vi "main4ChProspectiveStudyBK09172025.vi"() -> ()   [LabVIEW 2024]
doc: "Main VI for FLS imaging system."
uses:
  SubVI/DigitizerConfiguration/FLImDAQ.ctl
  <instrlib>/niScope/Controls/niScope trigger source.ctl
  SubVI/LabJack/LJ Pin Setting.ctl
  ConfigFiles/AimingBeamVideoConfig.ctl
  LaguerreDeconLib/DeconEngineClass/LaguerreDeconEngineClass.lvclass/LaguerreDeconEngineClass.ctl
  <vilib>/Utility/error.llb/DialogType.ctl
  LaguerreDeconLib/DeconEngineClass/LaguerreDeconEngineClass.lvclass
  <vilib>/event_ctls.llb/usereventprio.ctl
  <vilib>/Utility/miscctls.llb/LVMinMaxIncTypeDef.ctl
  SubVI/APD/APDClass.lvclass
  <vilib>/Analysis/baseanly.llb/Mean (DBL).vi
  SubVI/GlobalVariables.vi
  <vilib>/addons/control/pid/pid.llb/PID (DBL).vi
  <instrlib>/niScope/Acquire/Fetch/niScope Multi Fetch Binary 16.vi
  <vilib>/Instr/_visa.llb/VISA Configure Serial Port (Instr).vi
  <vilib>/Python/Open Anaconda Python Session.vi
  C:/Users/MarcuLab/Documents/GitHub/NetDeconForLV/Source/DotNETAssembly/output/build/LaguerreDeConNative.dll
  Documents/GitHub/NetDeconForLV/Source/DotNETAssembly/output/build/LaguerreDeConNative.dll
  <userlib>/_OpenG.lib/file/file.llb/openg_file.lvlib
  <userlib>/_OpenG.lib/time/time.llb/openg_time.lvlib
  <vilib>/Analysis/NI_AALBase.lvlib
  <vilib>/Utility/miscctls.llb/LVPointTypeDef.ctl
  <vilib>/addons/control/pid/NI_PID_pid.lvlib
panel:
  in  "CancerThreshold":dbl=0.15
  out "Decon Loop timing (ms)":dbl
  out "Ch3 Lifetime (ns)":dbl caption="Lifetime (ns)"
  out "Ch2 Lifetime (ns)":dbl caption="Lifetime (ns)"
  out "Ch1 Lifetime (ns)":dbl caption="Lifetime (ns)"
  out "Cancer Prob":dbl
  in  "Overlay selection":u16(ring)=2 items=["Gain", "Lifetime", "CancerProbability"]
  out "Record Backlog 2":i32
  in  "Auto gain ch4":bool=TRUE caption="Auto gain ch3"
  in  "V 4":dbl caption="Gain 3" min=0.0 max=4.67 step=0.1
  out "Gain4":dbl
  out "IntR4":dbl format="%#_2g"
  out "SNR4":dbl format="%#_3g"
  out "Channel 4":dbl[][](graph) caption="Channel 3"
  out "RunStartTime":u32
  out "Dig1 Temp":dbl
  out "Dig2 Temp":dbl
  out "Visualization PC video source":T1
  in  "V target(1.0)":dbl=1.0 caption="V target(1.5)" min=0.3 max=1.5 step=0.1 format="%#_4g"
  out "SNR3":dbl format="%#_3g"
  out "SNR2":dbl format="%#_3g"
  out "SNR1":dbl format="%#_3g"
  in  "Show BG removed?":bool=TRUE
  out "IntR3":dbl format="%#_2g"
  out "IntR2":dbl format="%#_2g"
  out "IntR1":dbl format="%#_2g"
  in  "Video Display":bool
  out "Gain3":dbl
  out "Gain2":dbl
  out "Gain1":dbl
  in  "Skip Data Save?":bool
  out "Aq Loop?":bool
  out "ML?":bool
  out "aquisition loop Error Out":errorcluster
  out "Laser f (Hz)":dbl
  out "Record Backlog":i32
  out "Fetch Record #":i32
  out "Sync Success?":bool
  out "Disclamer":picture
  out "Calibration #":i8
  out "BG #":i8
  in  "TCP Connect":bool
  out "Help":string
  in  "355nm Laser toggle":bool caption="355nm 460Hz"
  in  "Cali&iRF alignment":bool
  in  "Background":bool
  in  "Aiming beam toggle":bool caption="445nm 0Hz 30mA"
  in  "Auto gain ch3":bool=TRUE
  in  "Auto gain ch2":bool=TRUE
  in  "Auto gain ch1":bool=TRUE
  out "Run #":i8
  in  "StopButton":bool caption="Stop"
  out "Aquisition Status:":bool
  in  "StartButton":bool caption="Start"
  in  "V 3":dbl caption="Gain 3" min=0.0 max=4.65 step=0.1
  in  "V 2":dbl caption="Gain 2" min=0.0 max=4.59 step=0.1
  in  "V 1":dbl caption="Gain 1" min=0.0 max=4.63 step=0.1 format="%#_4g"
  in  "Video Source":enum32{"Camera", "FrameGrabber"}(radio)
  out "Case #":string
  out "System Hardware Connection Status":T2
  out "Channel 3":dbl[][](graph)
  out "Channel 2":dbl[][](graph)
  out "Channel 1":dbl[][](graph)
  in  "Tab Control":T3(tab)
  out "display loop timing(ms)":u32
  out "Aquisition loop timing(ms)":u32 format="%.2f"
  out "DisplayLoop":i32
  out "PID loop":i32 caption="processing loop"
  out "PID loop timing(ms)":u32 caption="processing loop timing(ms)"
  out "Communication loop(ms)":u32
  out "laser EM lamp V":dbl format="%0.6f"
  out "Auisition Loop idx":i32
  out "LJ process (ms)":u32
  out "LJ time(ms)":u32[](array[numeric])
  out "output variable":i32
  out "BG Graph":dbl[][](graph)
  out "Lifetime (ns)":cluster{dbl, dbl, dbl}(graph)
  out "DeCon Speed(ms)":dbl(graph)
  out "iRF Graph":dbl[][](graph)
  in  "Show BG":bool
  out "iRF length":i32
  out "BG length":i32
  out "data length":i32
  out "WarmupTime(ms)":u32
  out "BGAll":dbl[][](array[numeric])
  out "DeConOut":dbl[](array[numeric])
  in  "Ch1GainLim":dbl=350.0 format="%#_13g"
  in  "Ch2&3GainLim":dbl=1750.0 format="%#_13g"
  out "LJ Pinout":T4={"Ch1 Bias"="DAC0", "Ch2 Bias"="DAC1", "Ch3 Bias"="DAC2", "Ch4 Bias"="DAC0", "355 PWM"="FIO0", "AimingBeam PWM"="FIO2", "Laser Ready"="FIO3", "Interlock"="FIO1", "Laser Start/Stop"="FIO1", "Red LED"="FIO1", "Green LED"="DIO3", "Foot Pedal"="DIO15"}
  out "FLImDAQ":T5={"Digitizer 1"="", "Digitizer 2"="", "Channel"=enum."Channel 0", "trigger source"="VAL_EXTERNAL", "trigger level"=0.5, "trigger delay"=1.35e-07, "min sample rate"=12500000000.0, "min record length"=2500, "vertical range"=1.0, "vertical offset"=-0.25, "Waveform to Avg"=2000} caption="FLIm DAQ Configuration" {"trigger delay" format="%^#.4e"; "trigger level" min=0.0 max=3.5 step=0.5 format="%.2f"; "vertical offset" format="%.4f"; "vertical range" format="%.2f"; "min sample rate" format="%#.2p"}
  in  "Sys Reconfig":bool
  out "data out(communcation loop)":string
  out "PID loop error out":errorcluster caption="processing Error Out"
  out "decon error out":errorcluster
  out "Laser Rep Rate":dbl
  out "V4 Size":i32 caption="V3 Size"
  in  "Data Class":enum16{"Data", "BG", "Cali"}(ring)=enum."BG"
  out "V1 Size":i32
  out "V2 Size":i32
  out "V3 Size":i32
  out "data Size":i32[](array[numeric])
  out "State log":string
  out "SysConfigCluster":T7
  in  "Ch4 PID gains":T8={"proportional gain (Kc)"=30.0, "integral time (Ti, min)"=0.0003, "derivative time (Td, min)"=1e-05}
  in  "Ch3 PID gains":T8={"proportional gain (Kc)"=30.0, "integral time (Ti, min)"=0.0003, "derivative time (Td, min)"=1e-05}
  in  "Ch2 PID gains":T8={"proportional gain (Kc)"=30.0, "integral time (Ti, min)"=0.0003, "derivative time (Td, min)"=1e-05}
  in  "Ch1 PID gains":T8={"proportional gain (Kc)"=30.0, "integral time (Ti, min)"=0.0003, "derivative time (Td, min)"=1e-05}
  in  "module path":path=path "C:/Users/MarcuLab/Documents/GitHub/NetDeconForLV/Classifier/HNClassifier.py"
  in  "model path":path=path "C:/Users/MarcuLab/Documents/GitHub/NetDeconForLV/Classifier/20241127_dc/200.pkl"
  in  "Env name":string="HNClassifier"
  in  "Python version":string="3.10"
  out "Python session":refnum<k35>
  in  "Quit":bool
  in  "Radio Buttons":T9(radio)=enum."Ch2" caption="DeCon Chan"
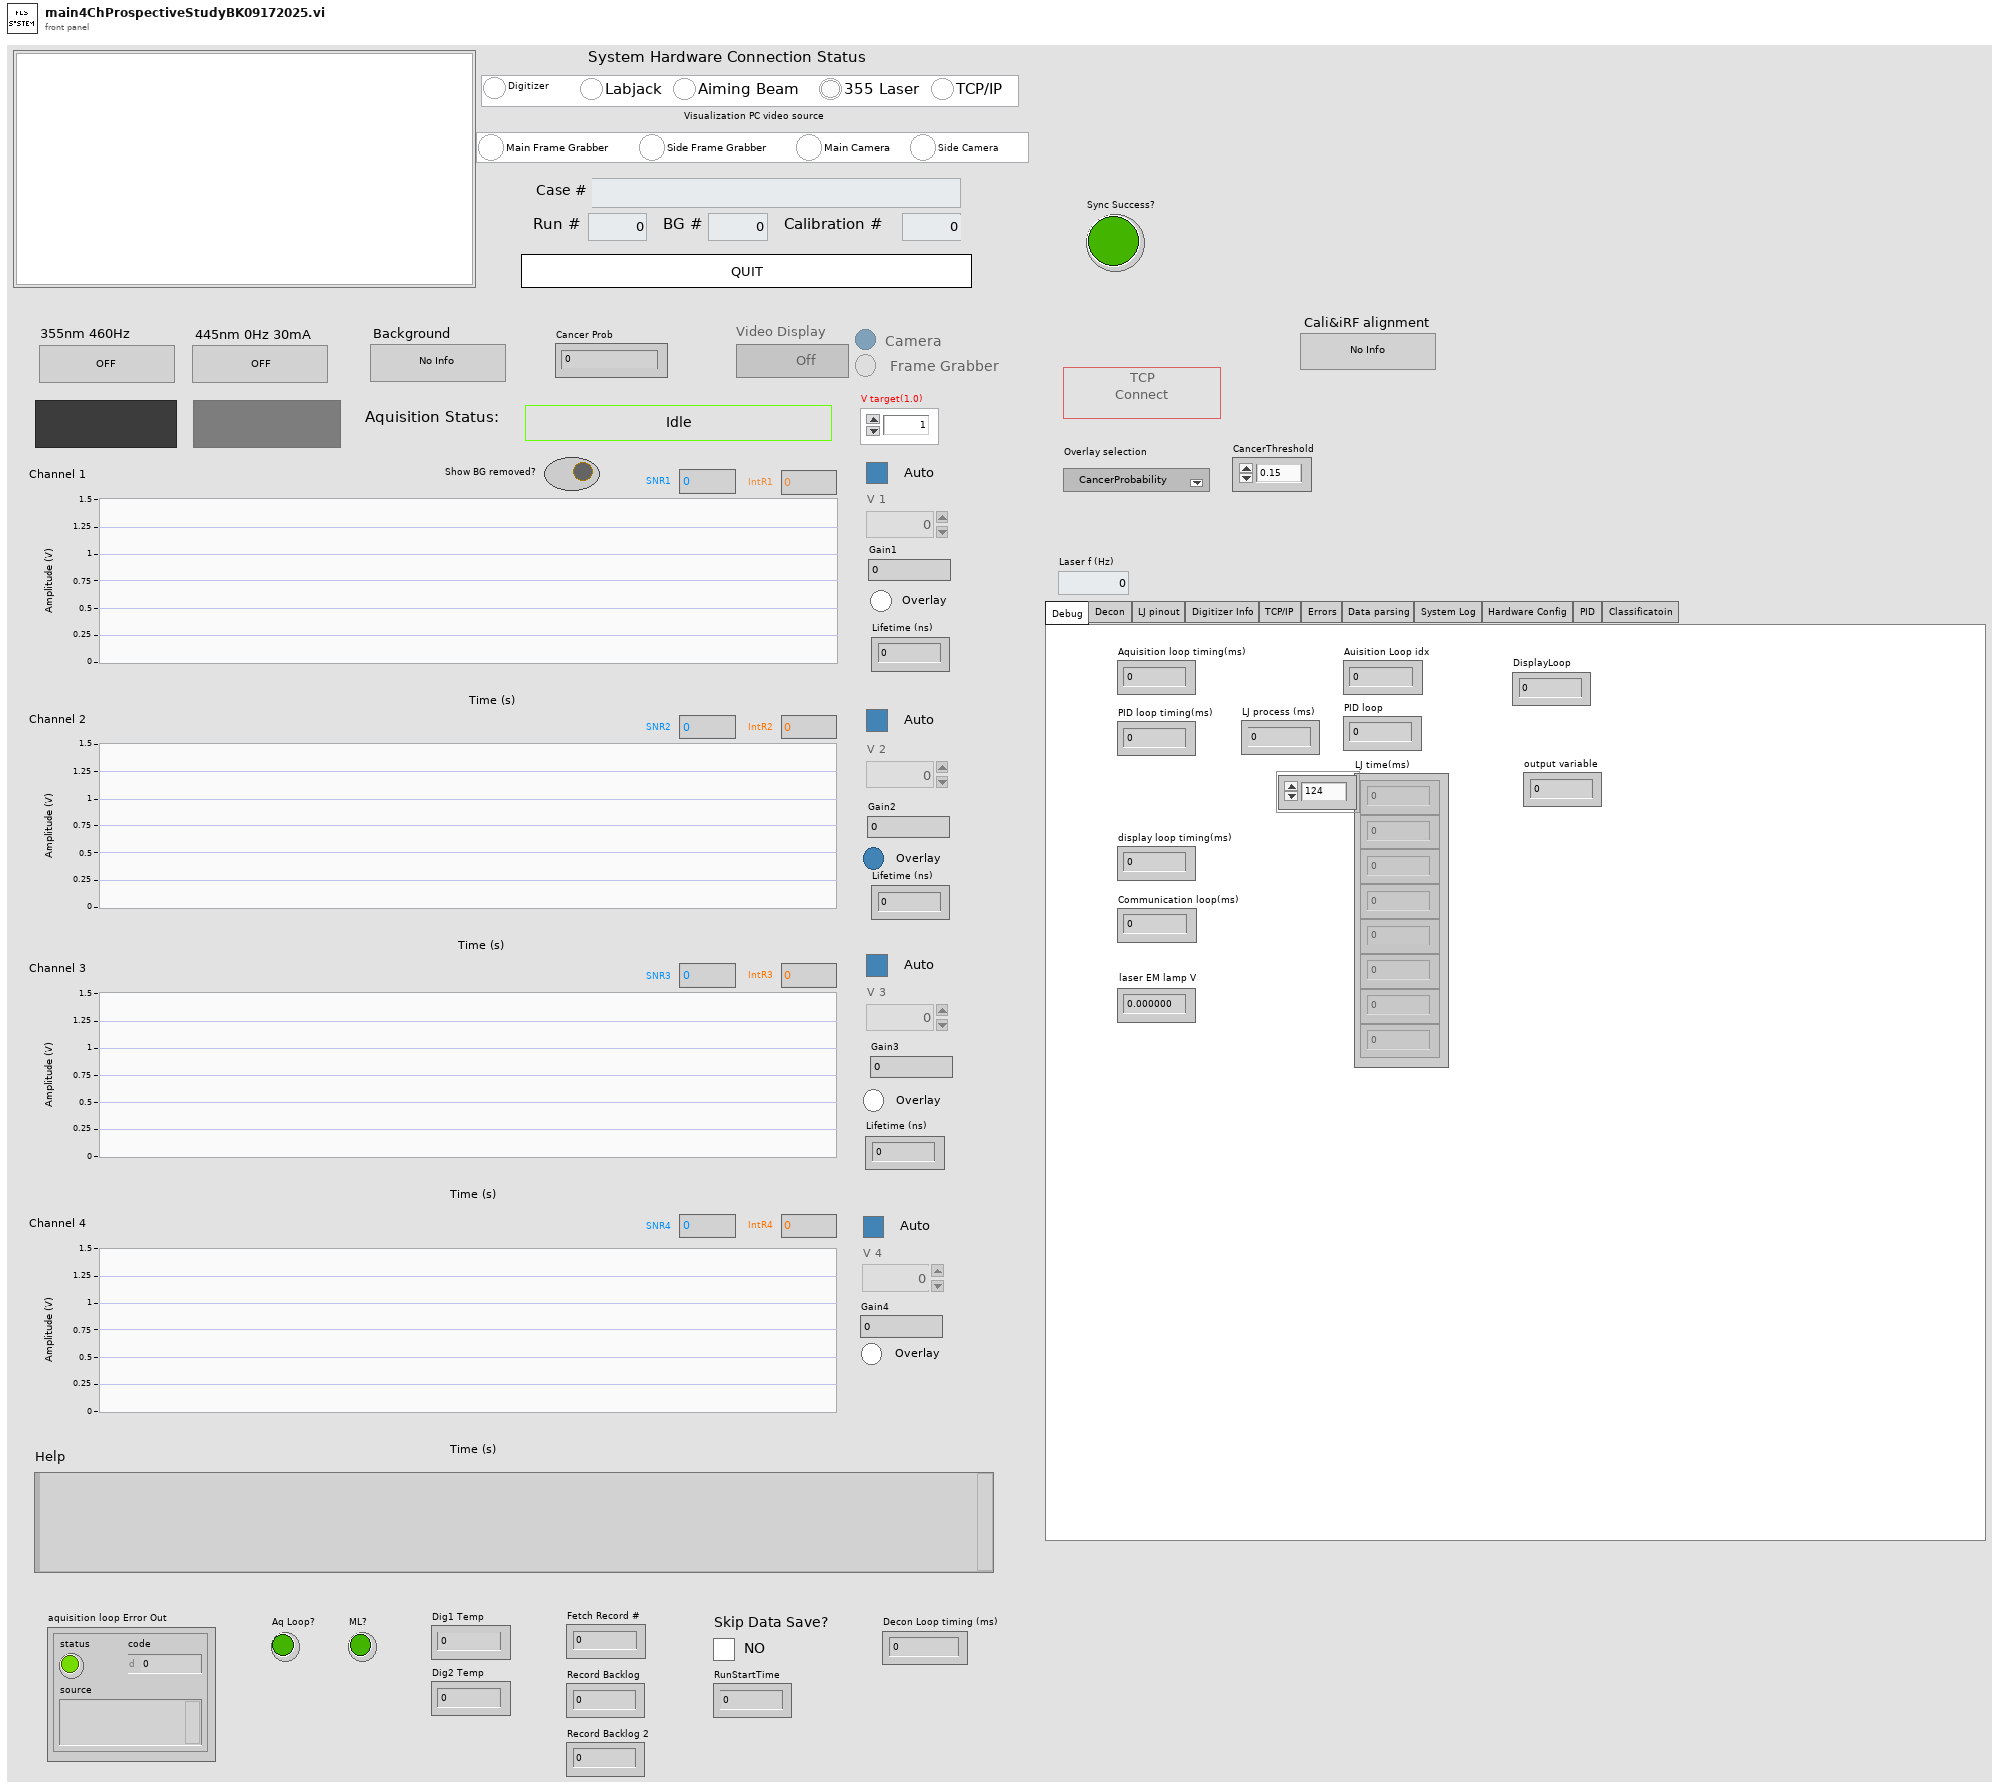
[diagram p1: front panel]
types:
  T1 = cluster{"Main Frame Grabber":bool, "Side Frame Grabber":bool, "Main Camera":bool, "Side Camera":bool}
  T2 = cluster{"Digitizer":bool, "Labjack":bool, "Aiming Beam":bool, "355 Laser":bool, "TCP/IP":bool}
  T3 = enum32{"Debug", "Decon", "LJ pinout", "Digitizer Info", "TCP/IP", "Errors", "Data parsing", "System Log", "Hardware Config", "PID", "Classificatoin"}
  T4 = typedef "LJ Pin Setting.ctl" = cluster{"Ch1 Bias":string, "Ch2 Bias":string, "Ch3 Bias":string, "Ch4 Bias":string, "355 PWM":string, "AimingBeam PWM":string, "Laser Ready":string, "Interlock":string, "Laser Start/Stop":string, "Red LED":string, "Green LED":string, "Foot Pedal":string}
  T5 = typedef "FLImDAQ.ctl" = cluster{"Digitizer 1":refnum<k15>, "Digitizer 2":refnum<k15>, "Channel":enum16{"Channel 0", "Channel 1", "Channel 0&1"}, "trigger source":T6, "trigger level":dbl, "trigger delay":dbl, "min sample rate":dbl, "min record length":i32, "vertical range":dbl, "vertical offset":dbl, "Waveform to Avg":i16}
  T6 = typedef "niScope trigger source.ctl" = string
  T7 = cluster{"Ch1Enable?":bool, "Ch2Enable?":bool, "Ch3Enable?":bool, "Ch1AutoGain?":bool, "Ch2AutoGain?":bool, "Ch3AutoGain?":bool, "AimingBeamEnable?":bool}
  T8 = cluster{"proportional gain (Kc)":dbl, "integral time (Ti, min)":dbl, "derivative time (Td, min)":dbl}
  T9 = enum32{"No Selection", "Ch1", "Ch2", "Ch3", "Ch4"}
  T10 = cluster{"remote start event":refnum<user-event>, "remote stop  event":refnum<user-event>}
  T11 = enum8{"Enabled", "Disabled", "Disabled and Grayed Out"}
  T12 = enum16{"open", "replace", "create", "open or create", "replace or create", "replace or create with confirmation"}
  T13 = cluster{"CH1":dbl[][], "CH2":dbl[][], "CH3":dbl[][], "CH4":dbl[][], "Gain cluster":cluster{"V1":dbl, "V2":dbl, "V3":dbl, "V4":dbl}}
  T14 = cluster{"idx":i32, "CH1&2":dbl[][], "CH3&4":dbl[][], "V cluster":cluster{"V1":dbl, "V2":dbl, "V3":dbl, "V4":dbl}}
  T15 = cluster{"Ch1 iRF":dbl[], "Ch2 iRF":dbl[], "Ch3 iRF":dbl[], "Ch4 iRF":dbl[]}
  T16 = enum16{"open", "open or create", "create or replace", "create", "open (read-only)"}
  T17 = enum32{"Invalid", "Standard", "Closed", "Hidden", "Minimized", "Maximized"}
  T18 = enum32{"invalid app kind", "Development System", "Run Time System", "Student Edition", "Embedded LabVIEW", "Evaluation", "Custom"}
  T19 = typedef "usereventprio.ctl" = enum32{"high priority", "normal priority"}
  T20 = enum32{"Bad", "Idle", "Run top level", "Running"}
  T21 = enum16{"Standard", "Buffered", "CRLF", "Immediate"}
  T22 = typedef "AimingBeamVideoConfig.ctl" = cluster{"DeCon Channel":enum16{"1", "2", "3"}, "Scale Bar":bool, "Scale Low":dbl, "Scale High":dbl, "ANSI":dbl, "Radius":dbl, "3D?":bool, "Firefly?":bool, "Pentero?":bool}
  T23 = cluster{"Core":cluster{"Current VI Reference":refnum<vi>, "Close Panel on Exit?":bool}, "SysConfigCluster":cluster{"Ch1Enable?":bool, "Ch2Enable?":bool, "Ch3Enable?":bool, "Ch1AutoGain?":bool, "Ch2AutoGain?":bool, "Ch3AutoGain?":bool, "AimingBeamEnable?":bool}, "System Status":cluster{"Digitizer":bool, "Labjack":bool, "Aiming Beam":bool, "355 Laser":bool, "TCP/IP":bool}, "IDs":cluster{"RunID":i8, "BG ID":i8, "Cali ID":i8}, "CaseID":string, "DefaultPath":path, "Pathes":cluster{"DataPath":path, "BG Path":path, "iRFPath":path, "CaliPath":path}, "FLImDAQ":cluster{"resource name":refnum<k15>, "resource name 2":refnum<k15>, "Channel":enum16{"Channel 0", "Channel 1", "Channel 0&1"}, "trigger source":T6, "trigger level":dbl, "trigger delay":dbl, "min sample rate":dbl, "min record length":i32, "vertical range":dbl, "vertical offset":dbl, "Waveform to Avg":i32}, "SysRunning?":bool, "AB Cluster":cluster{"Aiming Beam COM Port":refnum<visa-resource-name>, "Min Current":dbl, "Max Current":dbl, "Default Current":dbl, "Freq":i32}, "LJ Pinout":T4, "355 PWM setting":cluster{"DIO_EF_CLOCK1_DIVISOR":i16, "DIO_EF_CLOCK1_ROLL_VALUE":i32, "DIO#_EF_INDEX":i16, "DIO#_EF_OPTIONS":i16, "DIO#_EF_CONFIG_A":i32}, "AB PWM setting":cluster{"DIO_EF_CLOCK1_DIVISOR":i16, "DIO_EF_CLOCK1_ROLL_VALUE":i32, "DIO#_EF_INDEX":i16, "DIO#_EF_OPTIONS":i16, "DIO#_EF_CONFIG_A":i32}, "Last Trigger":u32, "niTClk sessions":refnum<k20>[], "Laser start tic":u32, "TCP attempt count":i32, "Ch1Data":dbl[][], "Ch2Data":dbl[][], "Ch3Data":dbl[][], "Ch4Data":dbl[][], "V1":dbl[], "V2":dbl[], "V3":dbl[], "V4":dbl[], "SlowTimer":u32, "FastTimer":u32, "listener ID":refnum<k5>, "TempPath":path, "CaliPath":path, "LED vi reference":refnum<vi>, "Aquisition Timer":u32, "APDSerialNum":cluster{"Ch1APDSerial#":string, "Ch2APDSerial#":string, "Ch3APDSerial#":string, "Ch4APDSerial#":string}, "VideoConfig":T22, "LED vi ref open?":bool, "video source":cluster{"Main Frame Grabber":bool, "Side Frame Grabber":bool, "Main Camera":bool, "Side Camera":bool}, "bothVidSourceAvail":bool}
  T24 = typedef "LVCursorListTypeDef.ctl" = cluster{"Name":string, "Color":u32, "Style":u8, "Point Style":u8, "Name Visible":bool, "Allow Drag":bool, "Cursor Mode":u32, "Plot":i32, "Index":i32, "Position":cluster{"X":dbl, "Y":dbl}, "X Scale":u32, "Y Scale":u32, "Watch Plots":i32[], "Watch All Plots":bool, "Plot Area":i32, "Label Offset":cluster{"X":dbl, "Y":dbl}}[]
  T25 = cluster{"Name":string, "Color":u32, "Style":u8, "Point Style":u8, "Name Visible":bool, "Allow Drag":bool, "Cursor Mode":u32, "Plot":i32, "Index":i32, "Position":cluster{"X":dbl, "Y":dbl}, "X Scale":u32, "Y Scale":u32, "Watch Plots":i32[], "Watch All Plots":bool, "Plot Area":i32, "Label Offset":cluster{"X":dbl, "Y":dbl}}
  T26 = cluster{"Ch1APDSerial#":string, "Ch2APDSerial#":string, "Ch3APDSerial#":string, "Ch4APDSerial#":string}
  T27 = cluster{"DataPath":path, "BG Path":path, "iRFPath":path, "CaliPath":path}
  T28 = cluster{"DIO_EF_CLOCK1_DIVISOR":i16, "DIO_EF_CLOCK1_ROLL_VALUE":i32, "DIO#_EF_INDEX":i16, "DIO#_EF_OPTIONS":i16, "DIO#_EF_CONFIG_A":i32}
  T29 = cluster{"Aiming Beam COM Port":refnum<visa-resource-name>, "Min Current":dbl, "Max Current":dbl, "Default Current":dbl, "Freq":i32}
  T30 = cluster{"resource name":refnum<k15>, "resource name 2":refnum<k15>, "Channel":enum16{"Channel 0", "Channel 1", "Channel 0&1"}, "trigger source":T6, "trigger level":dbl, "trigger delay":dbl, "min sample rate":dbl, "min record length":i32, "vertical range":dbl, "vertical offset":dbl, "Waveform to Avg":i32}
  T31 = cluster{"Current VI Reference":refnum<vi>, "Close Panel on Exit?":bool}
  T32 = cluster{"Channel 1":dbl[], "Channel 2":dbl[], "Channel 3":dbl[], "Channel 4":dbl[]}
  T33 = cluster{"V 1":dbl[], "V 2":dbl[], "V 3":dbl[], "V 4":dbl[]}
  T34 = cluster{"Ch1 WF":dbl[], "Ch2 WF":dbl[], "Ch3 WF":dbl[], "Ch4 WF":dbl[], "V1":dbl, "V2":dbl, "V3":dbl, "V4":dbl}
  T35 = typedef "iRFData.ctl" = cluster{"dt":dbl, "NumOfWFs":i32, "WFLength":i32, "iRFCtrlV":dbl[], "iRFWFsAvg":dbl[][], "iRFRaw":dbl[][]}
  T36 = cluster{"mean":dbl, "mean":dbl, "mean":dbl, "mean":dbl}
  T37 = cluster{"V1":dbl, "V2":dbl, "V3":dbl, "V4":dbl}[]
  T38 = cluster{"DataPath":path, "CaseID":string, "RunID":i16, "Ch1Data":dbl[][], "Ch2Data":dbl[][], "Ch3Data":dbl[][], "Ch4Data":dbl[][], "V1":dbl[], "V2":dbl[], "V3":dbl[], "V4":dbl[], "LaserRepRate":u16, "WFAverage":i16, "RunStartTime":u64}
  T39 = typedef "DialogType.ctl" = u16
  T40 = typedef "APD.ctl" = cluster{"gainV":dbl[], "gain":dbl[], "irfV":dbl[], "irfTNorm":dbl[][]}
  T41 = typedef "LJ PWM Setting.ctl" = cluster{"DIO_EF_CLOCK1_DIVISOR":i16, "DIO_EF_CLOCK1_ROLL_VALUE":i32, "DIO#_EF_INDEX":i16, "DIO#_EF_OPTIONS":i16, "DIO#_EF_CONFIG_A":i32}
  T42 = typedef "AimingBeam.ctl" = cluster{"Aiming Beam COM Port":refnum<visa-resource-name>, "Min Current":dbl, "Max Current":dbl, "Default Current":dbl, "Frequency(Hz)":u32}
  T43 = cluster{"DC1":i32, "DC2":i32, "BG1":i32, "BG2":i32}
  T44 = typedef "LVMinMaxIncTypeDef.ctl" = cluster{"Minimum":dbl, "Maximum":dbl, "Increment":dbl}
  T45 = typedef "LVBoundsTypeDef.ctl" = cluster{"Width":u32, "Height":u32}
  T46 = typedef "imagedata.ctl" = cluster{"image type":i32, "image depth":i32, "image":u8[], "mask":u8[], "colors":u32[], "Rectangle":cluster{"left":i16, "top":i16, "right":i16, "bottom":i16}}
  T47 = cluster{"DC Idx1":i32, "DC Idx2":i32, "BG Idx1":i32, "BG Idx2":i32}
  T48 = cluster{dbl[][], dbl[][], dbl[][], dbl[][], "V cluster":cluster{"V1":dbl, "V2":dbl, "V3":dbl, "V4":dbl}}
  T49 = cluster{"actualSamples":i32, "absoluteInitialX":dbl, "relativeInitialX":dbl, "xIncrement":dbl, "offset":dbl, "gain":dbl, "reserved1":dbl, "reserved2":dbl}[]
  T50 = cluster{"V1 out":dbl, "V2 out":dbl, "V3 out":dbl, "V3 out":dbl}
  T51 = cluster{i32, dbl[][], dbl[][], cluster{"V1 out":dbl, "V2 out":dbl, "V3 out":dbl, "V3 out":dbl}}
  T52 = typedef "LVPointTypeDef.ctl" = cluster{"Horizontal":i16, "Vertical":i16}
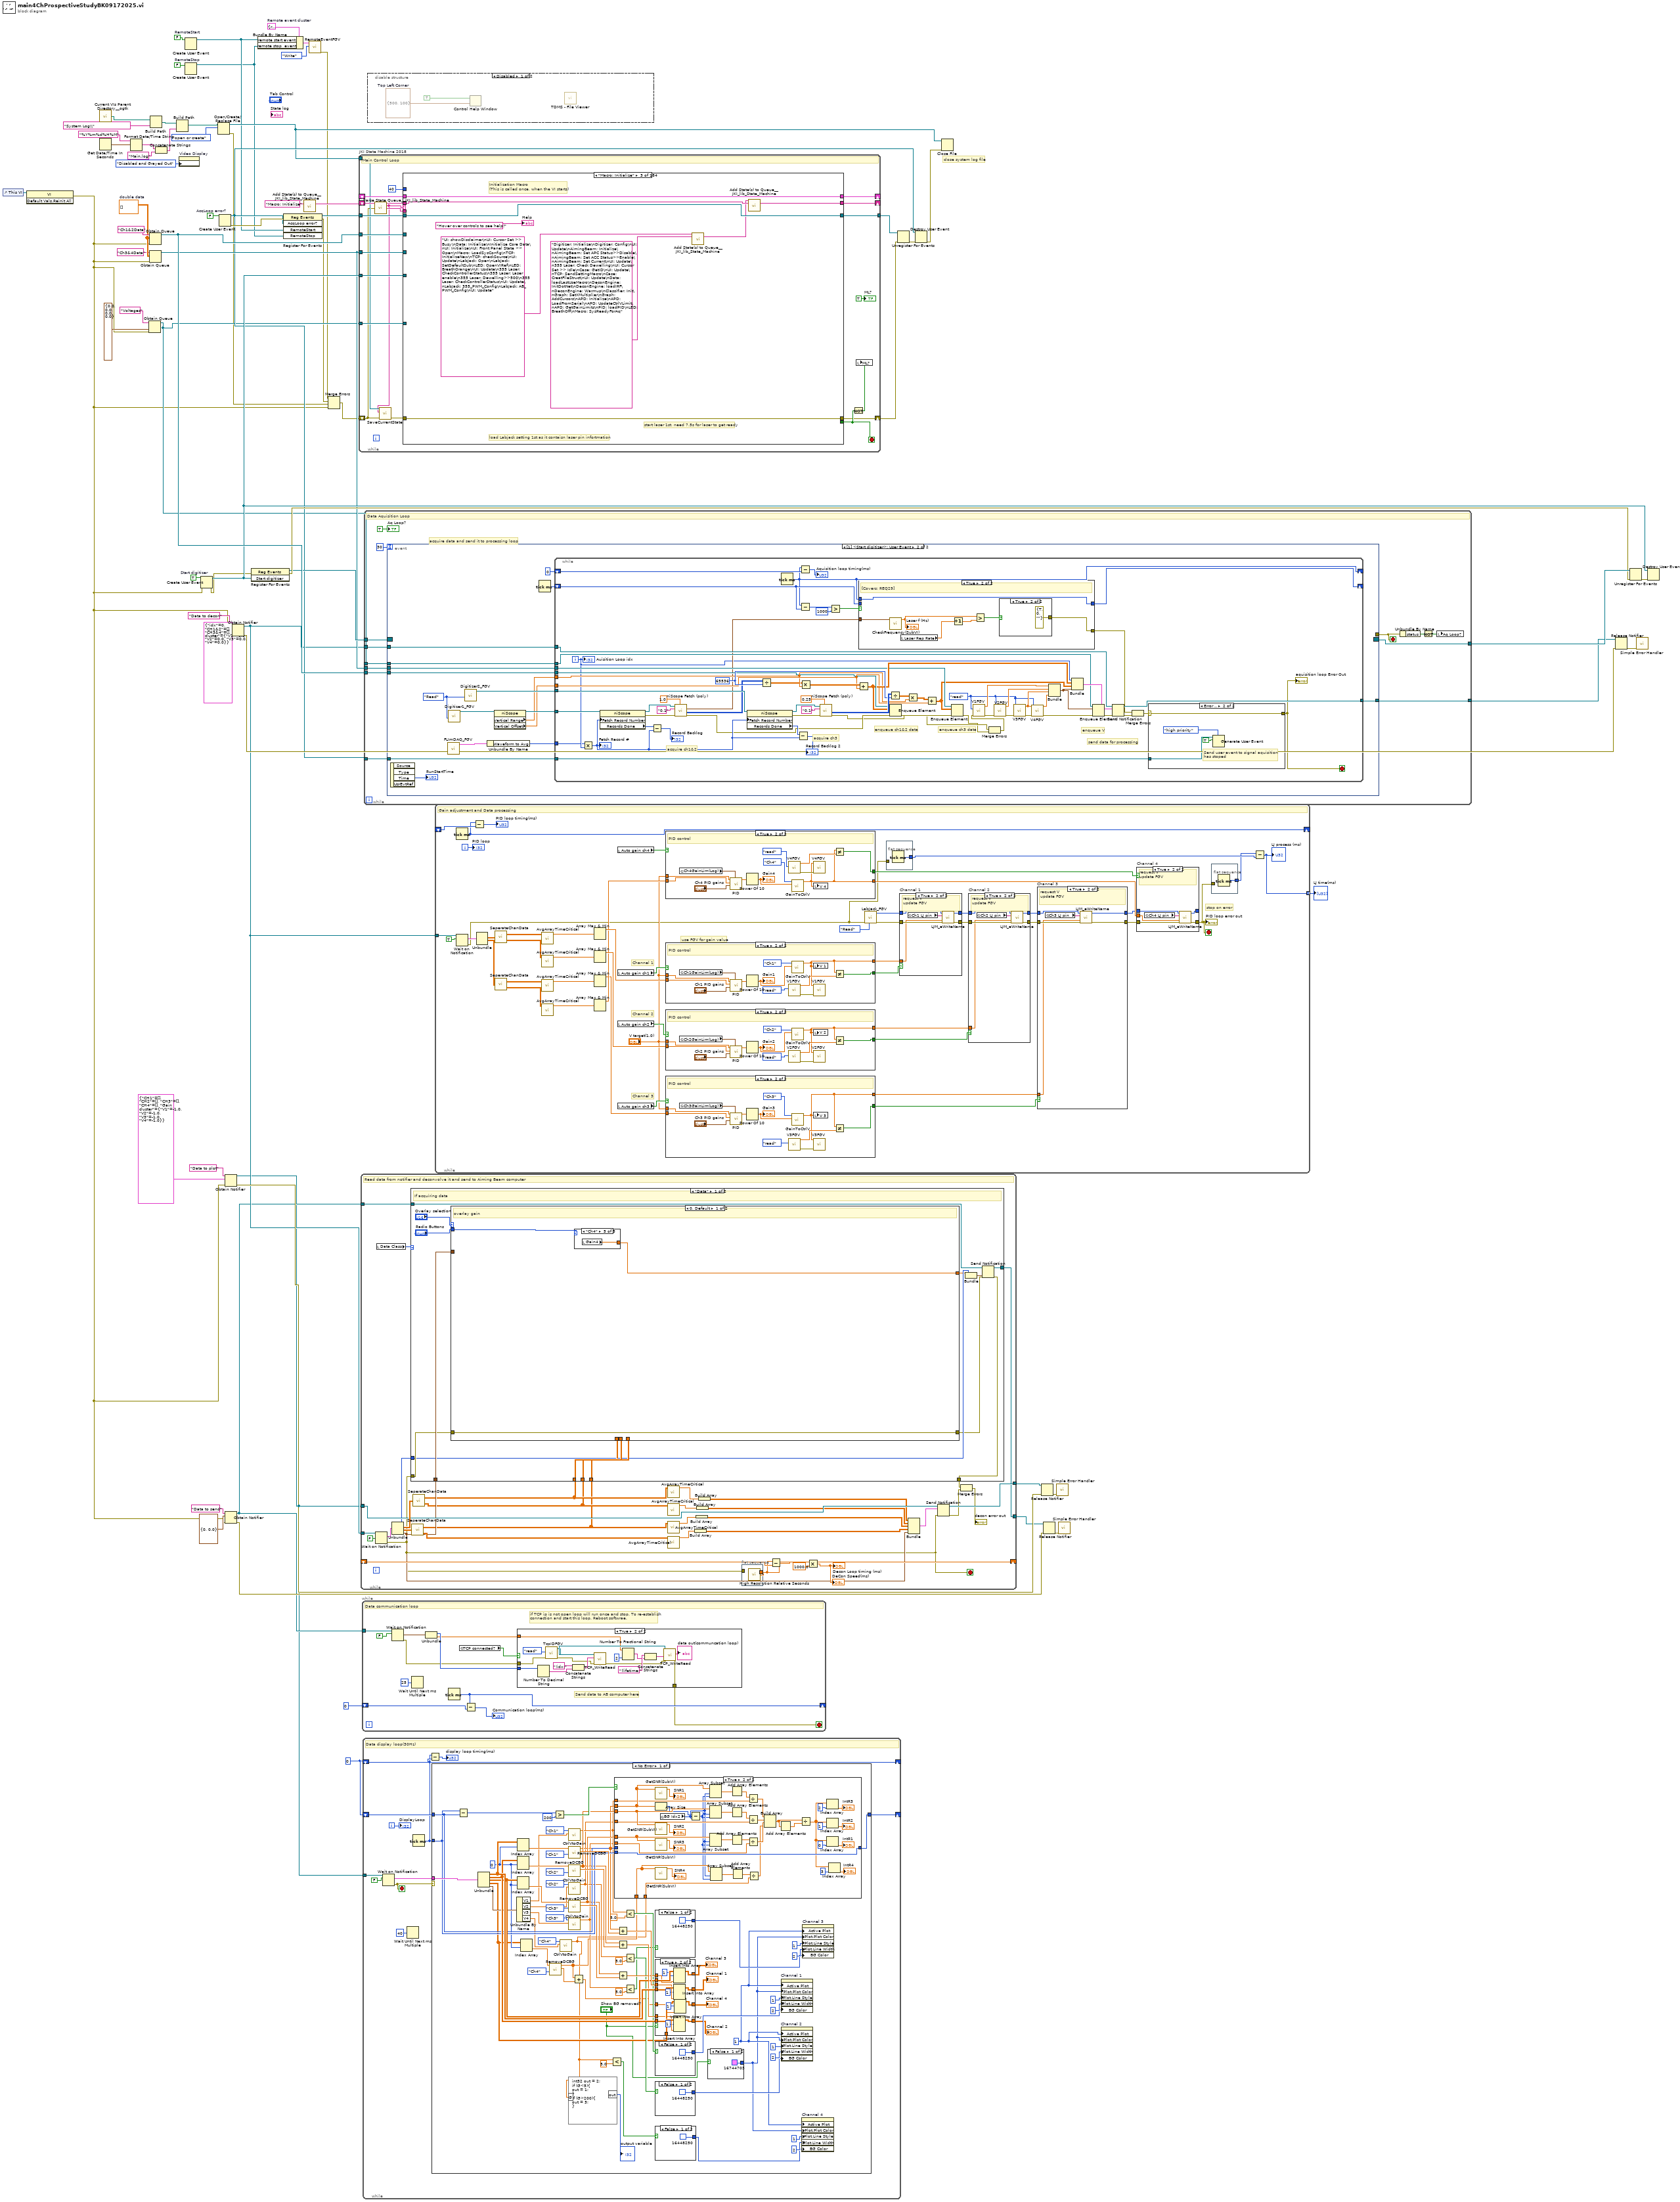
[diagram p0: block diagram]
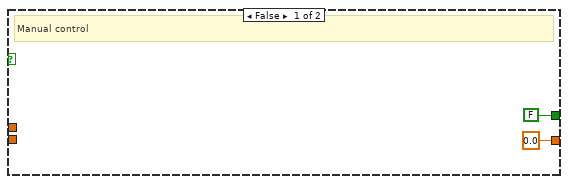
[diagram p6: hidden frame]
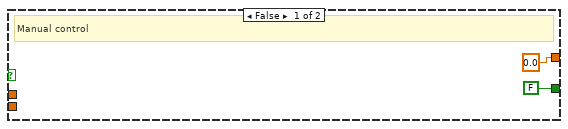
[diagram p7: hidden frame]
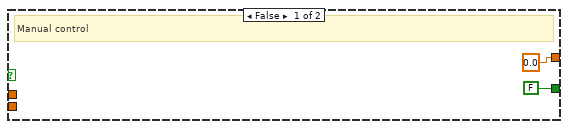
[diagram p8: hidden frame]
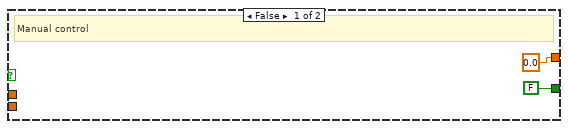
[diagram p9: hidden frame]
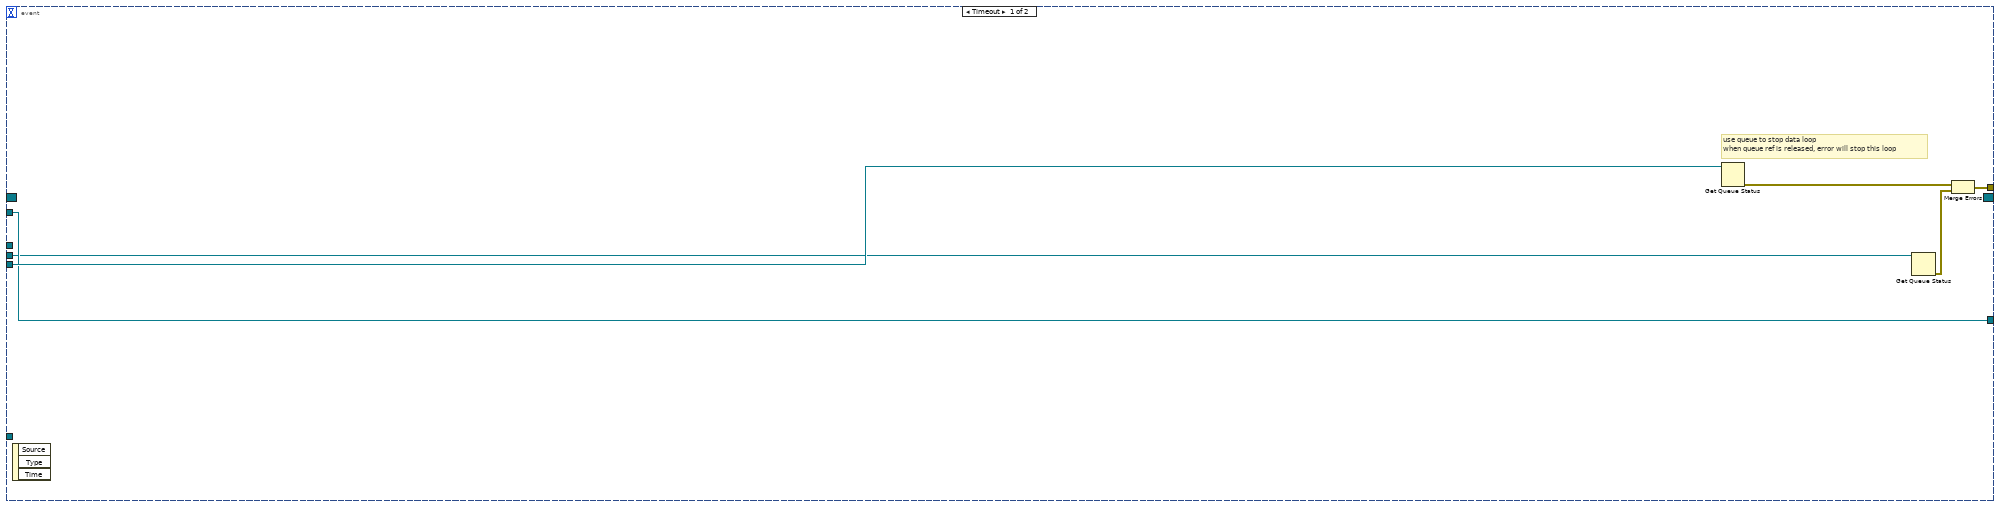
[diagram p10: hidden frame]
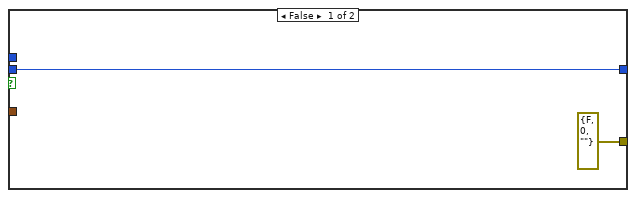
[diagram p11: hidden frame]
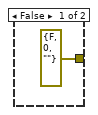
[diagram p12: hidden frame]
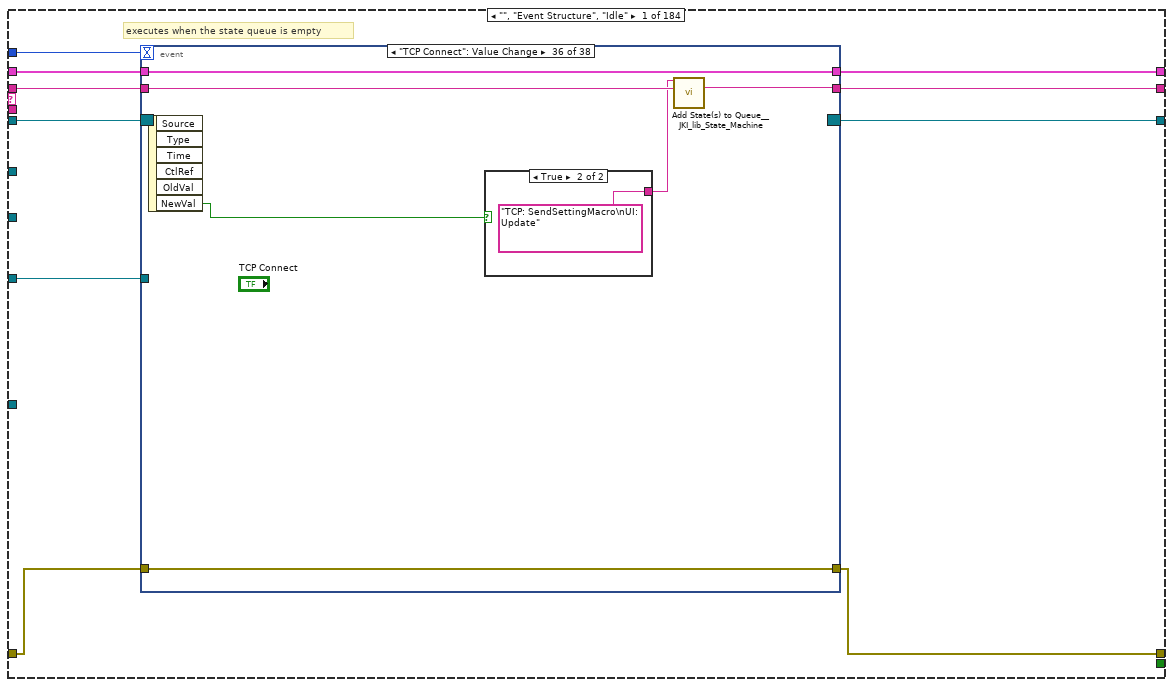
[diagram p14: hidden frame]
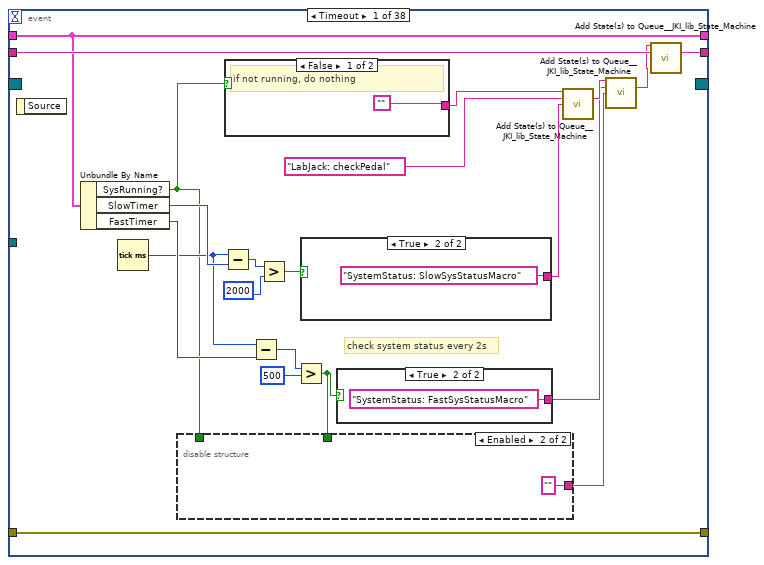
[diagram p15: hidden frame]
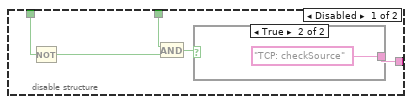
[diagram p16: hidden frame]
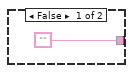
[diagram p17: hidden frame]
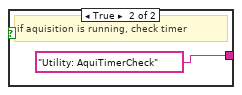
[diagram p18: hidden frame]
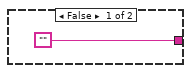
[diagram p19: hidden frame]
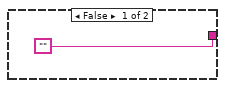
[diagram p20: hidden frame]
diagram:
  w8 = T10 {"remote start event"=refnum, "remote stop  event"=refnum}  # Remote event cluster
  w11 = FALSE  # RemoteStop
  w12 = FALSE  # RemoteStart
  w15 = u32 0 ("millisecond timer value")
  w54 = FALSE  # AcqLoop error?
  w64 = TRUE  # Start digitizer
  w67 = dbl[][] []  # double data
  # "close system log file"
  n1 = control-ref of="This VI"() -> (w69:refnum<vi>)
  n2 = invoke on="Invoke Node" class="VI" method="Default Vals.Reinit All"(reference=w69) -> (error out=w23:errorcluster)  [unwired: 2 in, 2 out]
  n3 = call <userlib>:"Current VIs Parent Directory__ogtk.vi"() -> ("Parent Directory (+ Relative)"=w34:path)  [unwired: 5 in]
  n4 = Get Date/Time In Seconds() -> (seconds since 1Jan1904=w32:timestamp)
  n5 = Format Date/Time String(time format string (%c)="%Y%m%d%H%M", seconds (now)=w32) -> (date/time string=w29:string)  [unwired: 1 in]
  n6 = Obtain Queue(name (unnamed)="Voltages", element data type=cluster{"V1":dbl, "V2":dbl, "V3":dbl, "V4":dbl} {"V1"=0.0, "V2"=0.0, "V3"=0.0, "V4"=0.0}, error in (no error)=w23) -> (queue out=w35:refnum<queue>)  [unwired: 2 in, 2 out]
  n7 = Obtain Queue(name (unnamed)="Ch3&4Data", element data type=w67, error in (no error)=w23) -> (queue out=w48:refnum<queue>)  [unwired: 2 in, 2 out]
  n8 = Obtain Queue(name (unnamed)="Ch1&2Data", element data type=w67, error in (no error)=w23) -> (queue out=w65:refnum<queue>)  [unwired: 2 in, 2 out]
  n9 = Build Path(base path=w34, name or relative path="System Log\\") -> (appended path=w25:path)
  n10 = Concatenate Strings(w29, "Main.log" ("string")) -> (w27:string)
  n11 = Build Path(base path=w25, name or relative path=w27) -> (appended path=w30:path)
  n12 = property on="Video Display" class="Bool (strict)"("DisabledEnum"=T11."Disabled and Grayed Out" ("Disabled")) -> ()  [unwired: 2 in, 2 out]
  n13 = Create User Event(user event datatype=w12) -> (user event=w10:refnum<user-event>)  [unwired: 1 in, 1 out]
  n14 = Create User Event(user event datatype=w11) -> (user event=w9:refnum<user-event>)  [unwired: 1 in, 1 out]
  n15 = Create User Event(user event datatype=w64, error in=w23) -> (user event=w53:refnum<user-event>, error out=w40:errorcluster)
  n16 = Open/Create/Replace File(file path (use dialog)=w30, operation (0:open)=T12."open or create") -> (refnum out=w21:refnum<file>, error out=w22:errorcluster)  [unwired: 4 in, 1 out]
  n17 = Create User Event(user event datatype=w54) -> (user event=w39:refnum<user-event>, error out=w41:errorcluster)  [unwired: 1 in]
  n18 = Obtain Notifier(name (unnamed)="Data to plot", notification data type=T13 {"CH1"=[], "CH2"=[], "CH3"=[], "CH4"=[], "Gain cluster"={"V1"=-1.0, "V2"=-1.0, "V3"=-1.0, "V4"=-1.0}}, error in (no error)=w23) -> (notifier out=w13:refnum<notifier>, error out=w49:errorcluster)  [unwired: 1 in, 1 out]
  n19 = Obtain Notifier(name (unnamed)="Data to send", notification data type=cluster{"idx":i32, "lifetime":dbl} {"idx"=0, "lifetime"=0.0}, error in (no error)=w23) -> (notifier out=w18:refnum<notifier>, error out=w38:errorcluster)  [unwired: 1 in, 1 out]
  n20 = Obtain Notifier(name (unnamed)="Data to decon", notification data type=T14 {"idx"=0, "CH1&2"=[], "CH3&4"=[], "V cluster"={"V1"=0.0, "V2"=0.0, "V3"=0.0, "V4"=0.0}}, error in (no error)=w23) -> (notifier out=w19:refnum<notifier>, error out=w58:errorcluster)  [unwired: 1 in, 1 out]
  n21 = register-events(error in=w40, w53) -> (reference out=w55:refnum<event-registration>, error out=w61:errorcluster)  [unwired: 1 in]
  n22 = Bundle By Name(cluster=w8, "remote start event"=w10, "remote stop  event"=w9) -> (w6:T10)
  n23 = register-events(error in=w41, w39, w10, w9) -> (reference out=w47:refnum<event-registration>, error out=w5:errorcluster)  [unwired: 1 in]
  n24 = call <vilib>:"Add State(s) to Queue__JKI_lib_State_Machine.vi"("State(s) in (\"\")"="Macro: Initialize") -> ("States Out"=w71:string)  [unwired: 14 in]
  n25 = call "RemoteEventFGV.vi"("Operation (Read)"=enum16{"Read", "Write"}."Write", "Remote Event in"=w6) -> ("Error Out"=w2:errorcluster)  [unwired: 8 in, 1 out]
  n26 = Merge Errors(w2, w5, w22, w23) -> (w24:errorcluster)
  n27 = while "JKI State Machine 2018" {
    shift-right: [w88] -> _
    shift-left: _ -> [w87]
    shift-right: [w72] -> w4
    shift-left: w24 -> [w74]
    shift-right: [w89] -> _
    shift-left: w71 -> [w90]
    tunnel: w65 -> [w85]
    tunnel: w48 -> [w84]
    tunnel: w53 -> [w83]
    tunnel: w47 -> [w82]
    tunnel: [w81] -> w46
    tunnel: w35 -> [w77]
    tunnel: w21 -> [w76]
    stop <- w80 stop-if-true
    # "Main Control Loop"
    n28 = call <vilib>:"Parse State Queue__JKI_lib_State_Machine.vi"("State Queue"=w90, "Error In (no error)"=w74) -> ("Remaining States"=w92:string, "Current State"=w75:string, "Arguments"=w91:string)  [unwired: 11 in]
    n29 = call "SaveCurrentState.vi"("error in (no error)"=w74, "Current State"=w75, "Byte Stream File in"=w76) -> ("error out"=w73:errorcluster)  [unwired: 8 in]
    n30 = case shown="\"Macro: Initialize\"" w75 {
      selector: w75 -> [_ _ _ _ _ _ _ _ _ _ _ _ _ _ _ _ _ _ _ _ _ _ _ _ w1091 _ _ _ _ _ _ _ _ _ _ _ _ _ _ _ _ _ _ _ _ _ _ _ _ _ _ _ _ _ _ _ _ _ _ _ _ _ _ _ _ _ _ _ _ _ _ _ _ _ _ _ _ _ _ _ _ _ _ _ _ _ _ _ _ _ _ _ _ _ _ _ _ _ _ _ _ _ _ _ _ _ _ _ _ _ _ _ _ _ _ _ _ _ _ _ _ _ _ _ _ _ _ _ _ _ _ _ _ _ _ _ _ _ _ _ _ _ _ _ _ _ _ _ _ _ _ _ _ _ _ _ _ _ _ _ _ _ _ _ _ _ _ _ _ _ _ _ _ _ _ _ _ _ _ _ _ _ _ _]
      tunnel: w92 -> [w102 w510 w519 w525 w531 w553 w566 w608 w614 w641 w660 w731 w746 w777 w804 w836 w867 w896 w910 w995 w1032 w1071 w1084 w1089 w1095 w1123 w1131 w1154 w1159 w1172 w1191 w1219 w1247 w1285 w1290 w1299 w1310 w1340 w1348 w1354 w1378 w1402 w1426 w1450 w1455 w1472 w1519 w1541 w1557 w1572 w1592 w1597 w1609 w1638 w1664 w1676 w1714 w1727 w1733 w1744 w1756 w1787 w1800 w1814 w1829 w1848 w1883 w1888 w1902 w1912 w1928 w1940 w1952 w1980 w1995 w2000 w2012 w2024 w2029 w2037 w2045 w2054 w2063 w2068 w2076 w2085 w2103 w2120 w2140 w2151 w2173 w2188 w2205 w2210 w2218 w2226 w2231 w2239 w2246 w2254 w2261 w2271 w2299 w2307 w2314 w2322 w2327 w2335 w2342 w2348 w2357 w2373 w2378 w2385 w2397 w2467 w2479 w2488 w2505 w2514 w2531 w2554 w2571 w2582 w2595 w2620 w2643 w2649 w2665 w2687 w2695 w2701 w2706 w2713 w2723 w2735 w2744 w2749 w2761 w2766 w2776 w2782 w2788 w2793 w2798 w2803 w2813 w2837 w2858 w2863 w2874 w2899 w2926 w2949 w2954 w2969 w3020 w3066 w3111 w3122 w3140 w3160 w3174 w3187 w3195 w3212 w3234 w3258 w3277 w3295 w3313 w3331 w3345 w3359 w3378 w3392 w3407 w3422 w3431 w3436 w3452 w3460 w3467 w3472]
      tunnel: w91 -> [_ _ _ _ _ _ _ _ _ _ _ _ _ _ _ _ _ _ _ _ _ _ _ _ _ _ _ _ _ _ _ _ _ _ _ _ _ _ _ _ _ _ _ _ _ _ _ _ _ _ _ _ _ _ _ _ _ _ _ _ w1754 _ _ _ _ _ _ _ _ _ _ _ _ _ _ _ _ _ _ _ _ _ _ _ _ _ _ _ _ _ _ _ _ _ _ _ _ _ _ _ _ w2262 _ _ _ _ _ _ _ _ _ _ _ w2380 w2391 _ _ _ _ w2511 w2528 _ _ _ _ _ w2639 _ _ _ _ _ _ w2708 _ _ _ _ _ _ w2772 _ _ _ _ _ _ _ _ _ _ _ _ _ _ _ _ _ _ _ _ _ _ _ _ _ _ _ _ _ _ _ _ _ _ _ _ _ _ _ _ _ _ _]
      tunnel: w87 -> [w100 w507 w515 w522 w528 w550 w563 _ w610 w637 w656 w728 w737 w774 w796 w827 w864 w893 w907 w956 w1024 w1059 w1079 w1086 w1093 w1116 w1128 w1152 w1156 w1160 w1181 w1211 w1239 w1281 w1287 w1297 w1308 w1338 w1346 w1351 w1359 w1383 w1408 w1432 w1452 w1465 w1509 w1538 w1542 w1569 w1589 w1594 w1598 w1627 w1654 w1669 w1697 w1725 w1730 w1737 w1752 w1770 w1795 w1806 w1824 w1841 w1866 w1885 w1898 w1906 w1925 w1937 w1949 w1968 w1984 w1997 w2010 w2022 w2026 w2031 w2038 w2050 w2059 w2065 w2072 w2082 w2090 w2107 w2135 w2141 w2170 w2181 w2203 w2207 w2211 w2219 w2228 w2237 w2243 w2251 w2258 w2268 w2296 w2304 w2311 w2319 w2324 w2329 w2340 w2345 w2351 w2370 w2375 w2383 w2393 w2464 w2469 w2482 w2503 w2512 w2529 w2544 w2568 w2579 w2589 w2613 w2640 w2646 w2658 w2683 w2692 w2698 w2703 w2710 w2717 w2731 w2741 w2746 w2758 w2763 w2769 w2779 w2785 w2790 w2795 w2800 w2810 w2835 w2856 w2860 w2872 w2897 w2924 w2947 w2951 w2962 w3014 w3062 w3108 w3118 w3135 w3155 w3169 w3183 w3189 w3207 w3229 w3253 w3272 w3290 w3308 w3326 w3340 w3354 w3373 w3387 w3402 w3419 w3429 w3433 w3450 w3458 w3464 w3469]
      tunnel: [w93 w508 w517 w523 w529 w551 w564 w606 w612 w633 w652 w705 w733 w775 w784 w816 w852 w884 w908 w932 w1021 w1058 w1080 w1087 w1097 w1120 errorcluster {"status"=FALSE, "code"=0, "source"=""} ("error out") w1151 w1157 w1170 w1189 w1203 w1226 w1283 w1288 w1292 w1303 w1313 w1342 w1352 w1360 w1384 w1409 w1433 w1453 w1456 w1501 w1532 w1546 w1570 w1580 w1595 w1601 w1625 w1653 w1668 w1684 w1719 w1731 w1742 w1746 w1761 w1790 w1802 w1820 w1840 w1857 w1886 w1890 w1908 w1923 w1935 w1947 w1970 w1985 w1998 w2002 w2019 w2027 w2035 w2043 w2047 w2056 w2066 w2069 w2078 w2093 w2115 w2134 w2145 w2163 w2185 w2201 w2208 w2216 w2224 w2229 w2236 w2244 w2252 w2259 w2269 w2297 w2305 w2312 w2320 w2325 w2333 w2339 w2346 w2354 w2371 w2376 w2381 w2394 w2465 w2473 w2485 w2495 w2508 w2525 w2545 w2569 w2578 w2591 w2615 w2641 w2647 w2655 w2677 w2693 w2699 w2704 w2711 w2721 w2733 w2742 w2747 w2759 w2764 w2774 w2780 w2786 w2791 w2796 w2801 w2811 w2825 w2849 w2861 w2865 w2884 w2916 w2941 w2952 w2956 w3015 w3063 w3109 w3117 w3137 w3157 w3171 w3185 w3191 w3209 w3231 w3255 w3274 w3292 w3310 w3328 w3342 w3356 w3375 w3389 w3403 w3420 w3427 w3434 w3440 w3453 w3465 w3470] -> w72
      tunnel: w73 -> [w99 w508 w517 w523 w529 w551 w564 w606 w612 w634 w650 w705 w732 w775 w785 w823 w853 w874 w908 w932 w1022 w1061 w1081 w1087 w1096 w1120 w1124 w1151 w1157 w1170 w1189 w1202 w1238 w1283 w1288 w1291 w1304 w1318 w1341 w1352 w1364 w1388 w1413 w1437 w1453 w1463 w1504 w1531 w1545 w1570 w1582 w1595 w1600 w1626 w1644 w1674 w1695 w1718 w1731 w1739 w1749 w1760 w1789 w1805 w1819 w1839 w1856 w1886 w1896 w1909 w1922 w1934 w1946 w1969 w1986 w1998 w2001 w2014 w2027 w2035 w2043 w2046 w2055 w2066 w2070 w2079 w2098 w2114 w2133 w2144 w2169 w2184 w2200 w2208 w2216 w2224 w2229 w2236 w2244 w2252 w2259 w2269 w2297 w2305 w2312 w2320 w2325 w2333 w2339 w2346 w2354 w2371 w2376 w2382 w2395 w2465 w2474 w2484 w2491 w2507 w2524 w2546 w2569 w2578 w2586 w2618 w2641 w2647 w2660 w2676 w2693 w2699 w2704 w2711 w2721 w2733 w2742 w2747 w2759 w2764 w2774 w2780 w2786 w2791 w2796 w2801 w2811 w2824 w2848 w2861 w2864 w2883 w2906 w2932 w2952 _ w3016 w3063 w3109 w3116 w3136 w3156 w3170 w3185 w3190 w3208 w3230 w3254 w3273 w3291 w3309 w3327 w3341 w3355 w3374 w3388 w3401 w3420 w3426 w3434 w3445 w3455 w3465 w3470]
      tunnel: [w101 w509 w518 w524 w530 w552 w565 w607 w613 w640 w659 w730 w745 w776 w803 w835 w866 w895 w909 w994 w1031 w1070 w1083 w1088 w1094 w1122 w1130 w1153 w1158 w1171 w1190 w1218 w1246 w1284 w1289 w1298 w1309 w1339 w1347 w1353 w1377 w1401 w1425 w1449 w1454 w1471 w1518 w1540 w1556 w1571 w1591 w1596 w1608 w1637 w1663 w1675 w1713 w1726 w1732 w1743 w1755 w1786 w1799 w1813 w1828 w1847 w1882 w1887 w1901 w1911 w1927 w1939 w1951 w1979 w1994 w1999 w2011 w2023 w2028 w2036 w2044 w2053 w2062 w2067 w2075 w2084 w2102 w2119 w2139 w2150 w2172 w2187 w2204 w2209 w2217 w2225 w2230 w2238 w2245 w2253 w2260 w2270 w2298 w2306 w2313 w2321 w2326 w2334 w2341 w2347 w2356 w2372 w2377 w2384 w2396 w2466 w2478 w2487 w2504 w2513 w2530 w2553 w2570 w2581 w2594 w2619 w2642 w2648 w2664 w2686 w2694 w2700 w2705 w2712 w2722 w2734 w2743 w2748 w2760 w2765 w2775 w2781 w2787 w2792 w2797 w2802 w2812 w2836 w2857 w2862 w2873 w2898 w2925 w2948 w2953 w2968 w3019 w3065 w3110 w3121 w3139 w3159 w3173 w3186 w3194 w3211 w3233 w3257 w3276 w3294 w3312 w3330 w3344 w3358 w3377 w3391 w3406 w3421 w3430 w3435 w3451 w3459 w3466 w3471] -> w89
      tunnel: [_ _ _ _ _ _ _ _ _ _ _ _ _ _ _ _ _ _ _ _ _ _ _ _ _ _ _ TRUE _ _ _ _ _ _ _ _ _ _ _ _ _ _ _ _ _ _ _ _ _ _ _ _ _ _ _ _ _ _ _ _ _ _ _ _ _ _ _ _ _ _ _ _ _ _ _ _ _ _ _ _ _ _ _ _ _ _ _ _ _ _ _ _ _ _ _ _ _ _ _ _ _ _ _ _ _ _ _ _ _ _ _ _ _ _ _ _ _ _ _ _ _ _ _ _ _ _ _ _ _ _ _ _ _ _ _ _ _ _ _ _ _ _ _ _ _ _ _ _ _ _ _ _ _ _ _ _ _ _ _ _ _ _ _ _ _ _ _ _ _ _ _ _ _ _ _ _ _ _ _ _ _ _ _ _] -> w80
      tunnel: [w98 w507 w515 w522 w528 w550 w563 w581 w610 w637 w656 w728 w737 w774 w796 w827 w864 w893 w907 w956 w1025 w1060 w1079 w1086 w1093 w1121 w1128 w1152 w1156 w1161 w1182 w1212 w1240 w1282 w1287 w1297 w1308 w1338 w1346 w1351 w1359 w1383 w1408 w1432 w1452 w1465 w1510 w1538 w1543 w1569 w1590 w1594 w1599 w1627 w1654 w1673 w1697 w1725 w1730 w1740 w1752 w1770 w1795 w1806 w1824 w1841 w1866 w1885 w1899 w1906 w1925 w1937 w1949 w1968 w1984 w1997 w2010 w2022 w2026 w2032 w2039 w2051 w2060 w2065 w2073 w2083 w2091 w2113 w2122 w2146 w2171 w2182 w2203 w2207 w2212 w2220 w2228 w2237 w2243 w2251 w2258 w2268 w2296 w2304 w2311 w2319 w2324 w2329 w2340 w2345 w2351 w2370 w2375 w2383 w2393 w2464 w2470 w2483 w2503 w2512 w2529 w2544 w2568 w2579 w2590 w2614 w2640 w2646 w2659 w2683 w2692 w2698 w2703 w2710 w2718 w2731 w2741 w2746 w2758 w2763 w2769 w2779 w2785 w2790 w2795 w2800 w2810 w2835 w2856 w2860 w2872 w2897 w2924 w2947 w2951 w2967 w3013 w3062 w3108 w3118 w3135 w3155 w3169 w3183 w3189 w3207 w3229 w3253 w3272 w3290 w3308 w3326 w3340 w3354 w3373 w3387 w3404 w3419 w3429 w3433 w3450 w3458 w3464 w3469] -> w88
      tunnel: 40 ("Timeout") -> [w97 _ _ _ _ _ _ _ _ _ _ _ _ _ _ _ _ _ _ _ _ _ _ _ _ _ _ _ _ _ _ _ _ _ _ _ _ _ _ _ _ _ _ _ _ _ _ _ _ _ _ _ _ _ _ _ _ _ _ _ _ _ _ _ _ _ _ _ _ _ _ _ _ _ _ _ _ _ _ _ _ _ _ _ _ _ _ _ _ _ _ _ _ _ _ _ _ _ _ _ _ _ _ _ _ _ _ _ _ _ _ _ _ _ _ _ _ _ _ _ _ _ _ _ _ _ _ _ _ _ _ _ _ _ _ _ _ _ _ _ _ _ _ _ _ _ _ _ _ _ _ _ _ _ _ _ _ _ _ _ _ _ _ _ _ _ _ _ _ _ _ _ _ _ _ _ _ _ _ _ _ _ _ _]
      tunnel: w85 -> [_ _ _ _ _ _ _ _ _ _ _ _ _ _ _ _ _ _ _ _ w1029 _ _ _ _ _ _ _ _ _ _ _ _ _ _ _ _ _ _ _ _ _ _ _ _ _ _ _ _ _ _ _ _ _ _ _ _ _ _ _ _ _ _ _ _ _ _ _ _ _ _ _ _ _ _ _ w2007 w2018 _ _ _ _ _ _ _ _ _ _ _ _ _ _ _ _ _ _ _ _ _ _ _ _ _ _ _ _ _ _ _ _ _ _ _ _ _ _ _ _ _ _ _ _ _ _ _ _ _ _ _ _ _ _ _ _ _ _ _ _ _ _ _ _ _ _ _ _ _ _ _ _ _ _ _ _ _ _ _ _ _ _ _ _ _ _ _ _ _ _ _ _ _ _ _ _ _ _ _ _ _ _ _ _ _ _]
      tunnel: w84 -> [_ _ _ _ _ _ _ _ _ _ _ _ _ _ _ _ _ _ _ _ w1028 _ _ _ _ _ _ _ _ _ _ _ _ _ _ _ _ _ _ _ _ _ _ _ _ _ _ _ _ _ _ _ _ _ _ _ _ _ _ _ _ _ _ _ _ _ _ _ _ _ _ _ _ _ _ _ w2008 w2017 _ _ _ _ _ _ _ _ _ _ _ _ _ _ _ _ _ _ _ _ _ _ _ _ _ _ _ _ _ _ _ _ _ _ _ _ _ _ _ _ _ _ _ _ _ _ _ _ _ _ _ _ _ _ _ _ _ _ _ _ _ _ _ _ _ _ _ _ _ _ _ _ _ _ _ _ _ _ _ _ _ _ _ _ _ _ _ _ _ _ _ _ _ _ _ _ _ _ _ _ _ _ _ _ _ _]
      tunnel: w83 -> [w96 _ _ _ _ _ _ _ _ _ _ _ _ _ _ _ _ _ _ _ _ _ _ _ _ _ _ _ _ _ _ _ _ _ _ _ _ _ _ _ _ _ _ _ _ _ _ w1534 _ _ _ _ _ _ _ _ _ _ _ _ _ _ _ _ _ _ _ _ _ _ _ _ _ _ _ _ _ _ _ _ _ _ _ _ _ _ _ _ _ _ _ _ _ _ _ _ _ _ _ _ _ _ _ _ _ _ _ _ _ _ _ _ _ _ _ _ _ _ _ _ _ _ _ _ _ _ _ _ _ _ _ _ _ _ _ _ _ _ _ _ _ _ _ _ _ _ _ _ _ _ _ _ _ _ _ _ _ _ _ _ _ _ _ _ _ _ _ _ _ _ _ _ _ _ _ _ _ _ _ _ _ _ _ _]
      tunnel: w82 -> [w95 w506 w516 w521 w527 w542 w562 w591 w611 w639 w658 w729 w744 w773 w802 w834 w865 w894 w906 w993 w1030 w1069 w1078 w1085 w1090 w1108 w1127 w1150 w1155 w1169 w1188 w1217 w1237 w1280 w1286 w1296 w1307 w1337 w1345 w1350 w1358 w1382 w1407 w1431 w1451 w1460 w1484 w1539 w1555 w1568 w1577 w1593 w1607 w1636 w1662 w1667 w1712 w1717 w1729 w1736 w1745 w1757 w1788 w1804 w1818 w1838 w1853 w1884 w1900 w1910 w1926 w1938 w1950 w1978 w1981 w1996 w2009 w2016 w2025 w2034 w2042 w2049 w2058 w2064 w2074 w2077 w2089 w2108 w2123 w2142 w2168 w2186 w2202 w2206 w2214 w2222 w2227 w2235 w2242 w2250 w2257 w2267 w2295 w2303 w2310 w2315 w2323 w2332 w2338 w2344 w2353 w2365 w2374 w2379 w2390 w2463 w2468 w2480 w2490 w2506 w2523 w2552 w2567 w2580 w2592 w2616 w2636 w2644 w2657 w2685 w2690 w2696 w2702 w2709 w2720 w2732 w2740 w2745 w2757 w2762 w2773 w2778 w2784 w2789 w2794 w2799 w2809 w2834 w2855 w2859 w2871 w2896 w2923 w2946 w2950 w2966 w3018 w3064 w3105 w3120 w3138 w3158 w3172 w3184 w3193 w3210 w3232 w3256 w3275 w3293 w3311 w3329 w3343 w3357 w3376 w3390 w3405 w3418 w3428 w3432 w3449 w3457 w3463 w3468]
      tunnel: [w94 w506 w516 w521 w527 w542 w562 w591 w611 w639 w658 w729 w744 w773 w802 w834 w865 w894 w906 w993 w1030 w1069 w1078 w1085 w1090 w1108 w1127 w1150 w1155 w1169 w1188 w1217 w1237 w1280 w1286 w1296 w1307 w1337 w1345 w1350 w1358 w1382 w1407 w1431 w1451 w1460 w1484 w1539 w1555 w1568 w1577 w1593 w1607 w1636 w1662 w1667 w1712 w1717 w1729 w1736 w1745 w1757 w1788 w1804 w1818 w1838 w1853 w1884 w1900 w1910 w1926 w1938 w1950 w1978 w1981 w1996 w2009 w2016 w2025 w2034 w2042 w2049 w2058 w2064 w2074 w2077 w2089 w2108 w2123 w2142 w2168 w2186 w2202 w2206 w2214 w2222 w2227 w2235 w2242 w2250 w2257 w2267 w2295 w2303 w2310 w2315 w2323 w2332 w2338 w2344 w2353 w2365 w2374 w2379 w2390 w2463 w2468 w2480 w2490 w2506 w2523 w2552 w2567 w2580 w2592 w2616 w2636 w2644 w2657 w2685 w2690 w2696 w2702 w2709 w2720 w2732 w2740 w2745 w2757 w2762 w2773 w2778 w2784 w2789 w2794 w2799 w2809 w2834 w2855 w2859 w2871 w2896 w2923 w2946 w2950 w2966 w3018 w3064 w3105 w3120 w3138 w3158 w3172 w3184 w3193 w3210 w3232 w3256 w3275 w3293 w3311 w3329 w3343 w3357 w3376 w3390 w3405 w3418 w3428 w3432 w3449 w3457 w3463 w3468] -> w81
      tunnel: w77 -> [_ _ _ _ _ _ _ _ _ _ _ _ _ _ _ _ _ _ _ _ w1023 _ _ _ _ _ _ _ _ _ _ _ _ _ _ _ _ _ _ _ _ _ _ _ _ _ _ _ _ _ _ _ _ _ _ _ _ _ _ _ _ _ _ _ _ _ _ _ _ _ _ _ _ _ _ _ w2006 w2015 _ _ _ _ _ _ _ _ _ _ _ _ _ _ _ _ _ _ _ _ _ _ _ _ _ _ _ _ _ _ _ _ _ _ _ _ _ _ _ _ _ _ _ _ _ _ _ _ _ _ _ _ _ _ _ _ _ _ _ _ _ _ _ _ _ _ _ _ _ _ _ _ _ _ _ _ _ _ _ _ _ _ _ _ _ _ _ _ _ _ _ _ _ _ _ _ _ _ _ _ _ _ _ _ _ _]
      frame "", "Event Structure", "Idle" {
        # "executes when the state queue is empty"
        n31 = event shown="[35] \"TCP Connect\": Value Change" {
          selector: w95 -> [_ _ _ _ _ _ _ _ _ _ _ _ _ _ _ _ _ _ _ _ _ _ _ _ _ _ _ _ _ _ _ _ _ _ _ _ _ _]
          dyn-events: [_ _ _ _ _ _ _ _ _ _ _ _ _ _ _ _ _ _ _ _ _ _ _ _ _ _ _ _ _ _ _ _ _ _ _ _ _ _] -> w94
          timeout: w97 -> [_ _ _ _ _ _ _ _ _ _ _ _ _ _ _ _ _ _ _ _ _ _ _ _ _ _ _ _ _ _ _ _ _ _ _ _ _ _]
          tunnel: w102 -> [w122 w141 w149 w153 w157 w165 w171 w179 w187 w197 w204 w233 w253 w273 w293 w297 w304 w327 w341 w355 w369 w374 w377 w383 w390 w397 w403 w409 w415 w422 w435 w446 w458 w465 w469 w473 w489 w505]
          tunnel: [w123 w141 w148 w153 w156 w165 w171 w179 w187 w197 w203 w233 w253 w273 w293 w297 w303 w327 w341 w355 w369 w373 w376 w383 w391 w398 w402 w408 w415 w423 w436 w446 w459 w465 w469 w472 w490 w504] -> w101
          tunnel: w100 -> [w106 w139 w143 w151 w158 w164 w172 w180 w188 w195 w199 w231 w251 w271 w291 w295 w299 w326 w340 w354 w368 w370 w378 w381 w386 w393 w405 w410 w413 w417 w430 w444 w454 w463 w467 w474 w487 w502]
          tunnel: [w121 w140 w144 w152 w159 w163 w170 w178 w186 w196 w205 w232 w252 w272 w292 w296 w305 w324 w328 w351 w366 w372 w379 w382 w387 w394 w406 w411 w414 w421 w434 w445 w455 w464 w468 w475 w491 w503] -> w93
          tunnel: w99 -> [w121 w140 w144 w152 w159 w163 w170 w178 w186 w196 w205 w232 w252 w272 w292 w296 w305 w321 w330 w342 w358 w372 w379 w382 w387 w394 w406 w411 w414 w421 w434 w445 w457 w464 w468 w475 w491 w503]
          tunnel: [w106 w139 w143 w151 w158 w164 w172 w180 w188 w195 w200 w231 w251 w271 w291 w295 w300 w326 w340 w354 w368 w370 w378 w381 w388 w395 w405 w410 w413 w418 w431 w444 w460 w463 w467 w474 w488 w502] -> w98
          tunnel: w96 -> [_ _ _ _ _ _ _ _ _ _ _ _ _ _ _ _ _ _ _ _ _ _ _ _ _ _ _ _ _ _ _ _ _ _ _ _ _ _]
          event Timeout {
            # "check system status every 2s"
            n32 = event-data() -> ()  [unwired: 1 in, 1 out]
            n33 = Unbundle By Name(w106) -> ("SysRunning?"=w104:bool, "SlowTimer"=w120:u32, "FastTimer"=w114:u32)
            n34 = Tick Count (ms)() -> (millisecond timer value=w107:u32)
            n35 = Subtract(x=w107, y=w120) -> (x-y=w117:u32)
            n36 = case shown="False" w104 {
              tunnel: ["" "Utility: AquiTimerCheck" ("State(s) in Front (\"\")")] -> w112
              frame False {
                # "if not running, do nothing"
              }
              frame True {
                # "if aquisition is running, check timer"
              }
            }
            n37 = Subtract(x=w107, y=w114) -> (x-y=w115:u32)
            n38 = Greater?(x=w117, y=u32 2000) -> (0:w118:bool)
            n39 = Greater?(x=w115, y=u32 500) -> (0:w105:bool)
            n40 = disable-structure shown="Enabled" {
              disable-tunnel: w105 -> [w128 _]
              disable-tunnel: w104 -> [w127 _]
              disable-tunnel: [w124 "" ("State(s) at Back (\"\")")] -> w103
              frame Disabled {
                n41 = Not(x=w127) -> (.not. x?=w126:bool)
                n42 = And(x=w128, y=w126) -> (x .and. y?=w125:bool)
                n43 = case shown="True" w125 {
                  tunnel: ["" ("Empty String Constant") "TCP: checkSource" ("State(s) in Front (\"\")")] -> w124
                  frame False {
                  }
                  frame True {
                  }
                }
              }
              frame Enabled {
              }
            }
            n44 = case shown="True" w118 {
              tunnel: ["" ("Empty String Constant") "SystemStatus: SlowSysStatusMacro" ("State(s) in Front (\"\")")] -> w110
              frame False {
              }
              frame True {
              }
            }
            n45 = case shown="True" w105 {
              tunnel: ["" ("Empty String Constant") "SystemStatus: FastSysStatusMacro" ("State(s) in Front (\"\")")] -> w108
              frame False {
              }
              frame True {
              }
            }
            n46 = call <vilib>:"Add State(s) to Queue__JKI_lib_State_Machine.vi"("State(s) in Front (\"\")"=w112, "State(s) in (\"\")"="LabJack: checkPedal" ("State(s) in Front (\"\")"), "State(s) at Back (\"\")"=w110) -> ("States Out"=w109:string)  [unwired: 12 in]
            n47 = call <vilib>:"Add State(s) to Queue__JKI_lib_State_Machine.vi"("State(s) in Front (\"\")"=w109, "State(s) in (\"\")"=w108, "State(s) at Back (\"\")"=w103) -> ("States Out"=w113:string)  [unwired: 12 in]
            n48 = call <vilib>:"Add State(s) to Queue__JKI_lib_State_Machine.vi"("State(s) in Front (\"\")"=w113, "State(s) in (\"\")"=w122) -> ("States Out"=w123:string)  [unwired: 13 in]
          }
          event "355nm Laser toggle": Mouse Enter {
            n49 = event-data() -> ()  [unwired: 1 in, 4 out]
            n50 = local write "Help"("Toggle 355nm laser." ("Help")) -> ()
          }
          event "355nm Laser toggle": Value Change {
            # "[Covers: REQ34]"
            n51 = event-data() -> ()  [unwired: 1 in, 6 out]
            n52 = Select(t="LabJack: 355_PWM_Start\nLabJack: AB_Start", s="355nm Laser toggle", f="LabJack: 355_PWM_Stop\nLabJack: AB_Stop") -> (s? t:f=w146:string)
            n53 = call <vilib>:"Add State(s) to Queue__JKI_lib_State_Machine.vi"("State(s) in Front (\"\")"=w146, "State(s) in (\"\")"=w149) -> ("States Out"=w148:string)  [unwired: 13 in]
          }
          event "Aiming beam toggle": Mouse Enter {
            n54 = event-data() -> ()  [unwired: 1 in, 4 out]
            n55 = local write "Help"("Toggle aiming beam laser." ("Help")) -> ()
          }
          event "Aiming beam toggle": Value Change {
            # "[Covers: REQ33]"
            n56 = event-data() -> ()  [unwired: 1 in, 6 out]
            n57 = case shown="True" "Aiming beam toggle" {
              tunnel: ["LabJack: AB_Stop" ("State(s) in Front (\"\")") "LabJack: AB_Start" ("State(s) in Front (\"\")")] -> w155
              frame False {
              }
              frame True {
              }
            }
            n58 = call <vilib>:"Add State(s) to Queue__JKI_lib_State_Machine.vi"("State(s) in Front (\"\")"=w155, "State(s) in (\"\")"=w157) -> ("States Out"=w156:string)  [unwired: 13 in]
          }
          event "Auto gain ch1": Value Change {
            n59 = event-data() -> ("NewVal"=w162:bool)  [unwired: 1 in, 5 out]
            n60 = case shown="True" w162 {
              frame False {
                n61 = local read "V 1"() -> (w166:dbl)
                n62 = call "V1FGV.vi"("action (write)"=enum16{"write", "read"}."write" ("action"), "V1 in"=w166) -> ()  [unwired: 8 in, 2 out]
                n63 = property on="V 1" class="DigNum (strict)"("DisabledEnum"=T11."Enabled" ("Disabled")) -> ()  [unwired: 2 in, 2 out]
              }
              frame True {
                n64 = property on="V 1" class="DigNum (strict)"("DisabledEnum"=T11."Disabled and Grayed Out" ("Disabled")) -> ()  [unwired: 2 in, 2 out]
              }
            }
          }
          event "Auto gain ch2": Value Change {
            n65 = event-data() -> ("NewVal"=w173:bool)  [unwired: 1 in, 5 out]
            n66 = case shown="False" w173 {
              frame False {
                n67 = local read "V 2"() -> (w174:dbl)
                n68 = property on="V 2" class="DigNum (strict)"("DisabledEnum"=T11."Enabled" ("Disabled")) -> ()  [unwired: 2 in, 2 out]
                n69 = call "V2FGV.vi"("action(write)"=enum16{"write", "read"}."write" ("action"), "V2 in"=w174) -> ()  [unwired: 8 in, 2 out]
              }
              frame True {
                n70 = property on="V 2" class="DigNum (strict)"("DisabledEnum"=T11."Disabled and Grayed Out" ("Disabled")) -> ()  [unwired: 2 in, 2 out]
              }
            }
          }
          event "Auto gain ch3": Value Change {
            n71 = event-data() -> ("NewVal"=w181:bool)  [unwired: 1 in, 5 out]
            n72 = case shown="False" w181 {
              frame False {
                n73 = local read "V 3"() -> (w182:dbl)
                n74 = property on="V 3" class="DigNum (strict)"("DisabledEnum"=T11."Enabled" ("Disabled")) -> ()  [unwired: 2 in, 2 out]
                n75 = call "V3FGV.vi"("action(write)"=enum16{"write", "read"}."write" ("action"), "V3 in"=w182) -> ()  [unwired: 8 in, 2 out]
              }
              frame True {
                n76 = property on="V 3" class="DigNum (strict)"("DisabledEnum"=T11."Disabled and Grayed Out" ("Disabled")) -> ()  [unwired: 2 in, 2 out]
              }
            }
          }
          event "Auto gain ch4": Value Change {
            n77 = event-data() -> ("NewVal"=w189:bool)  [unwired: 1 in, 5 out]
            n78 = case shown="False" w189 {
              frame False {
                n79 = local read "V 4"() -> (w190:dbl)
                n80 = property on="V 4" class="DigNum (strict)"("DisabledEnum"=T11."Enabled" ("Disabled")) -> ()  [unwired: 2 in, 2 out]
                n81 = call "V4FGV.vi"("action(write)"=enum16{"write", "read"}."write" ("action"), "V3 in"=w190) -> ()  [unwired: 8 in, 2 out]
              }
              frame True {
                n82 = property on="V 4" class="DigNum (strict)"("DisabledEnum"=T11."Disabled and Grayed Out" ("Disabled")) -> ()  [unwired: 2 in, 2 out]
              }
            }
          }
          event "Background": Mouse Enter {
            n83 = event-data() -> ()  [unwired: 1 in, 4 out]
            n84 = local write "Help"("Click to record a background." ("Help")) -> ()
          }
          event "Background": Value Change {
            n85 = event-data() -> ("NewVal"=w201:bool)  [unwired: 1 in, 5 out]
            n86 = case shown="True" w201 {
              tunnel: ["Utility: SetAllChanManualGain\nQueue: Flash\nUtility: Dewelling >> 2500\nLabJack: 355_PWM_Stop\nLabJack: AB_Stop" "Utility: SetDataClass >> Bg\nUI: Update\nLabJack: 355_PWM_Start\nLabJack: AB_Start\nUtility: SaveDeconChan\nUtility: Dewelling >> 50\nLabJack: SetV\nDigitizer: Start\nUtility: AquiTimerReset\nLED: BreathGreen\nUI: duringBGAcquire"] -> w202
              tunnel: [FALSE TRUE] -> w198
              frame False {
                n87 = local read "Skip Data Save?"() -> (w206:bool)
                n88 = case shown="False" w206 {
                  frame False {
                    n89 = property on="Background" class="Bool (strict)"("BoolText.Text"="Done!" ("Boolean Text.Text")) -> ()  [unwired: 2 in, 2 out]
                  }
                  frame True {
                  }
                }
              }
              frame True {
                # "[Covers: REQ6]"
                n90 = property on="Background" class="Bool (strict)"("BoolText.Text"="Running" ("Boolean Text.Text"), "Colors [4]"=cluster{u32, u32}[] [{6618880, 6618880}, {16711680, 16711680}]) -> ()  [unwired: 2 in, 2 out]
              }
            }
            n91 = Bundle By Name(cluster=w199, "SysRunning?"=w198) -> (w200:T23)
            n92 = call <vilib>:"Add State(s) to Queue__JKI_lib_State_Machine.vi"("State(s) in Front (\"\")"=w202, "State(s) in (\"\")"=w204) -> ("States Out"=w203:string)  [unwired: 13 in]
          }
          event "Channel 1": Cursor Move {
            n93 = event-data() -> ("CursIdx"=w217:i32, "CursLoc"=w229:cluster{"X":dbl, "Y":dbl})  [unwired: 1 in, 7 out]
            n94 = property on="Channel 3" class="WFGraph (strict)"() -> ("CrsrList"=w224:T24)  [unwired: 2 in, 2 out]
            n95 = property on="Channel 4" class="WFGraph (strict)"() -> ("CrsrList"=w216:T24)  [unwired: 2 in, 2 out]
            n96 = property on="Channel 2" class="WFGraph (strict)"() -> ("CrsrList"=w227:T24)  [unwired: 2 in, 2 out]
            n97 = Index Array(array=w224, index=w217) -> (element=w228:T25)
            n98 = Index Array(array=w216, index=w217) -> (element=w219:T25)
            n99 = Unbundle By Name(w229) -> ("X"=w218:dbl)
            n100 = Index Array(array=w227, index=w217) -> (element=w230:T25)
            n101 = Bundle By Name(cluster=w228, "Position.X"=w218) -> (w223:T25)
            n102 = Bundle By Name(cluster=w219, "Position.X"=w218) -> (w215:T25)
            n103 = Bundle By Name(cluster=w230, "Position.X"=w218) -> (w226:T25)
            n104 = control-ref of="Channel 1"() -> (w220:refnum<vi>)
            n105 = Replace Array Subset(array=w224, new element=w223, index=w217) -> (w222:T24)
            n106 = Replace Array Subset(array=w216, new element=w215, index=w217) -> (w214:T24)
            n107 = Replace Array Subset(array=w227, new element=w226, index=w217) -> (w225:T24)
            n108 = property on="Channel 3" class="WFGraph (strict)"("CrsrList"=w222) -> (error out=w221:errorcluster)  [unwired: 2 in, 1 out]
            n109 = property on="Channel 4" class="WFGraph (strict)"("CrsrList"=w214) -> ()  [unwired: 2 in, 2 out]
            n110 = property on="Channel 2" class="WFGraph (strict)"("CrsrList"=w225) -> ()  [unwired: 2 in, 2 out]
            n111 = call "UpdateCurserIdx(SubVI).vi"("error in (no error)"=w221, "WaveformGraph in"=w220) -> ()  [unwired: 9 in, 1 out]
          }
          event "Channel 2": Cursor Move {
            n112 = event-data() -> ("CursIdx"=w236:i32, "CursLoc"=w250:cluster{"X":dbl, "Y":dbl})  [unwired: 1 in, 7 out]
            n113 = Unbundle By Name(w250) -> ("X"=w238:dbl)
            n114 = property on="Channel 1" class="WFGraph (strict)"() -> ("CrsrList"=w244:T24)  [unwired: 2 in, 2 out]
            n115 = property on="Channel 3" class="WFGraph (strict)"() -> ("CrsrList"=w246:T24)  [unwired: 2 in, 2 out]
            n116 = property on="Channel 4" class="WFGraph (strict)"() -> ("CrsrList"=w237:T24)  [unwired: 2 in, 2 out]
            n117 = Index Array(array=w244, index=w236) -> (element=w249:T25)
            n118 = Index Array(array=w246, index=w236) -> (element=w248:T25)
            n119 = Index Array(array=w237, index=w236) -> (element=w239:T25)
            n120 = Bundle By Name(cluster=w239, "Position.X"=w238) -> (w235:T25)
            n121 = Bundle By Name(cluster=w249, "Position.X"=w238) -> (w247:T25)
            n122 = Bundle By Name(cluster=w248, "Position.X"=w238) -> (w245:T25)
            n123 = Replace Array Subset(array=w244, new element=w247, index=w236) -> (w243:T24)
            n124 = Replace Array Subset(array=w246, new element=w245, index=w236) -> (w242:T24)
            n125 = Replace Array Subset(array=w237, new element=w235, index=w236) -> (w234:T24)
            n126 = control-ref of="Channel 1"() -> (w241:refnum<vi>)
            n127 = property on="Channel 1" class="WFGraph (strict)"("CrsrList"=w243) -> ()  [unwired: 2 in, 2 out]
            n128 = property on="Channel 3" class="WFGraph (strict)"("CrsrList"=w242) -> (error out=w240:errorcluster)  [unwired: 2 in, 1 out]
            n129 = property on="Channel 4" class="WFGraph (strict)"("CrsrList"=w234) -> ()  [unwired: 2 in, 2 out]
            n130 = call "UpdateCurserIdx(SubVI).vi"("error in (no error)"=w240, "WaveformGraph in"=w241) -> ()  [unwired: 9 in, 1 out]
          }
          event "Channel 3": Cursor Move {
            n131 = event-data() -> ("CursIdx"=w256:i32, "CursLoc"=w270:cluster{"X":dbl, "Y":dbl})  [unwired: 1 in, 7 out]
            n132 = Unbundle By Name(w270) -> ("X"=w258:dbl)
            n133 = property on="Channel 4" class="WFGraph (strict)"() -> ("CrsrList"=w257:T24)  [unwired: 2 in, 2 out]
            n134 = property on="Channel 1" class="WFGraph (strict)"() -> ("CrsrList"=w267:T24)  [unwired: 2 in, 2 out]
            n135 = property on="Channel 2" class="WFGraph (strict)"() -> ("CrsrList"=w265:T24)  [unwired: 2 in, 2 out]
            n136 = Index Array(array=w257, index=w256) -> (element=w259:T25)
            n137 = Index Array(array=w267, index=w256) -> (element=w269:T25)
            n138 = Index Array(array=w265, index=w256) -> (element=w268:T25)
            n139 = Bundle By Name(cluster=w259, "Position.X"=w258) -> (w255:T25)
            n140 = Bundle By Name(cluster=w269, "Position.X"=w258) -> (w266:T25)
            n141 = Bundle By Name(cluster=w268, "Position.X"=w258) -> (w264:T25)
            n142 = Replace Array Subset(array=w257, new element=w255, index=w256) -> (w254:T24)
            n143 = Replace Array Subset(array=w267, new element=w266, index=w256) -> (w263:T24)
            n144 = Replace Array Subset(array=w265, new element=w264, index=w256) -> (w262:T24)
            n145 = control-ref of="Channel 1"() -> (w260:refnum<vi>)
            n146 = property on="Channel 4" class="WFGraph (strict)"("CrsrList"=w254) -> ()  [unwired: 2 in, 2 out]
            n147 = property on="Channel 1" class="WFGraph (strict)"("CrsrList"=w263) -> ()  [unwired: 2 in, 2 out]
            n148 = property on="Channel 2" class="WFGraph (strict)"("CrsrList"=w262) -> (error out=w261:errorcluster)  [unwired: 2 in, 1 out]
            n149 = call "UpdateCurserIdx(SubVI).vi"("error in (no error)"=w261, "WaveformGraph in"=w260) -> ()  [unwired: 9 in, 1 out]
          }
          event "Channel 4": Cursor Move {
            n150 = event-data() -> ("CursIdx"=w278:i32, "CursLoc"=w290:cluster{"X":dbl, "Y":dbl})  [unwired: 1 in, 7 out]
            n151 = Unbundle By Name(w290) -> ("X"=w276:dbl)
            n152 = property on="Channel 1" class="WFGraph (strict)"() -> ("CrsrList"=w288:T24)  [unwired: 2 in, 2 out]
            n153 = property on="Channel 2" class="WFGraph (strict)"() -> ("CrsrList"=w284:T24)  [unwired: 2 in, 2 out]
            n154 = property on="Channel 3" class="WFGraph (strict)"() -> ("CrsrList"=w279:T24)  [unwired: 2 in, 2 out]
            n155 = Index Array(array=w288, index=w278) -> (element=w289:T25)
            n156 = Index Array(array=w284, index=w278) -> (element=w285:T25)
            n157 = Index Array(array=w279, index=w278) -> (element=w281:T25)
            n158 = Bundle By Name(cluster=w289, "Position.X"=w276) -> (w287:T25)
            n159 = Bundle By Name(cluster=w285, "Position.X"=w276) -> (w283:T25)
            n160 = Bundle By Name(cluster=w281, "Position.X"=w276) -> (w280:T25)
            n161 = Replace Array Subset(array=w288, new element=w287, index=w278) -> (w286:T24)
            n162 = Replace Array Subset(array=w284, new element=w283, index=w278) -> (w282:T24)
            n163 = Replace Array Subset(array=w279, new element=w280, index=w278) -> (w277:T24)
            n164 = control-ref of="Channel 1"() -> (w274:refnum<vi>)
            n165 = call "UpdateCurserIdx(SubVI).vi"() -> ()  [unwired: 11 in, 1 out]
            n166 = call "UpdateCurserIdx(SubVI).vi"() -> ()  [unwired: 11 in, 1 out]
            n167 = property on="Channel 1" class="WFGraph (strict)"("CrsrList"=w286) -> ()  [unwired: 2 in, 2 out]
            n168 = property on="Channel 2" class="WFGraph (strict)"("CrsrList"=w282) -> ()  [unwired: 2 in, 2 out]
            n169 = property on="Channel 3" class="WFGraph (strict)"("CrsrList"=w277) -> (error out=w275:errorcluster)  [unwired: 2 in, 1 out]
            n170 = call "UpdateCurserIdx(SubVI).vi"("error in (no error)"=w275, "WaveformGraph in"=w274) -> ()  [unwired: 9 in, 1 out]
          }
          event "Cali&iRF alignment": Mouse Enter {
            n171 = event-data() -> ()  [unwired: 1 in, 4 out]
            n172 = local write "Help"("Click to run system intensity calibration and irf alignment" ("Help")) -> ()
          }
          event "Cali&iRF alignment": Value Change {
            n173 = event-data() -> ("NewVal"=w301:bool)  [unwired: 1 in, 5 out]
            n174 = case shown="False" w301 {
              tunnel: ["Utility: SetAllChanManualGain\nQueue: Flash\nUtility: Dewelling >> 2500\nLabJack: 355_PWM_Stop\nLabJack: AB_Stop" "Utility: SetDataClass >> Cali\nUI: Update\nUtility: SaveDeconChan\nLabJack: 355_PWM_Start\nLabJack: AB_Start\nLabJack: SetV\nDigitizer: Start\nUtility: AquiTimerReset\nLED: BreathGreen\nUI: duringIRFAlign"] -> w302
              tunnel: [FALSE TRUE] -> w298
              frame False {
                n175 = local read "Skip Data Save?"() -> (w306:bool)
                n176 = case shown="False" w306 {
                  frame False {
                    n177 = property on="Cali&iRF alignment" class="Bool (strict)"("BoolText.Text"="Done!" ("Boolean Text.Text")) -> ()  [unwired: 2 in, 2 out]
                  }
                  frame True {
                  }
                }
              }
              frame True {
                n178 = property on="Cali&iRF alignment" class="Bool (strict)"("BoolText.Text"="Running" ("Boolean Text.Text"), "Colors [4]"=cluster{u32, u32}[] [{6618880, 6618880}, {16711680, 16711680}]) -> ()  [unwired: 2 in, 2 out]
              }
            }
            n179 = Bundle By Name(cluster=w299, "SysRunning?"=w298) -> (w300:T23)
            n180 = call <vilib>:"Add State(s) to Queue__JKI_lib_State_Machine.vi"("State(s) in Front (\"\")"=w302, "State(s) in (\"\")"=w304) -> ("States Out"=w303:string)  [unwired: 13 in]
          }
          event "V 1": Value Change {
            n181 = event-data() -> ()  [unwired: 1 in, 6 out]
            n182 = call "LabJack_FGV.vi"("Operation(Read)"=enum16{"Write", "Read"}."Read" ("Operation"), "error in (no error)"=w321) -> ("error out"=w318:errorcluster, "Read data"=w319:i32)  [unwired: 8 in]
            n183 = global read "GlobalVariables.vi" "Ch1 LJ pin"() -> (w317:string)
            n184 = call "LJM_eWriteName.vi"("Handle In"=w319, "Name"=w317, "Value"="V 1", "error in"=w318) -> ("error out"=w315:errorcluster)  [unwired: 10 in, 1 out]
            n185 = call "V1FGV.vi"("Error In"=w315, "action (write)"=enum16{"write", "read"}."write" ("action"), "V1 in"="V 1") -> ("Error Out"=w314:errorcluster)  [unwired: 7 in, 1 out]
            n186 = call "CtrlVtoGain.vi"("error in (no error)"=w314, "CtrlV(V)"="V 1", "Channel"=enum16{"Ch1", "Ch2", "Ch3"}."Ch1" ("Enum")) -> ("error out"=w324:errorcluster, "Gain"=w323:dbl)  [unwired: 7 in]
            n187 = local write "Gain1"(w323) -> ()
          }
          event "V 2": Value Change {
            n188 = event-data() -> ()  [unwired: 1 in, 6 out]
            n189 = call "LabJack_FGV.vi"("Operation(Read)"=enum16{"Write", "Read"}."Read" ("Operation"), "error in (no error)"=w330) -> ("error out"=w335:errorcluster, "Read data"=w336:i32)  [unwired: 8 in]
            n190 = global read "GlobalVariables.vi" "Ch2 LJ pin"() -> (w334:string)
            n191 = call "LJM_eWriteName.vi"("Handle In"=w336, "Name"=w334, "Value"="V 2", "error in"=w335) -> ("error out"=w333:errorcluster)  [unwired: 10 in, 1 out]
            n192 = call "V2FGV.vi"("Error In"=w333, "action(write)"=enum16{"write", "read"}."write" ("action"), "V2 in"="V 2") -> ("Error Out"=w332:errorcluster)  [unwired: 7 in, 1 out]
            n193 = call "CtrlVtoGain.vi"("error in (no error)"=w332, "CtrlV(V)"="V 2", "Channel"=enum16{"Ch1", "Ch2", "Ch3"}."Ch2" ("Enum")) -> ("error out"=w328:errorcluster, "Gain"=w329:dbl)  [unwired: 7 in]
            n194 = local write "Gain2"(w329) -> ()
          }
          event "V 3": Value Change {
            n195 = event-data() -> ()  [unwired: 1 in, 6 out]
            n196 = call "LabJack_FGV.vi"("Operation(Read)"=enum16{"Write", "Read"}."Read" ("Operation"), "error in (no error)"=w342) -> ("error out"=w347:errorcluster, "Read data"=w348:i32)  [unwired: 8 in]
            n197 = global read "GlobalVariables.vi" "Ch3 LJ pin"() -> (w346:string)
            n198 = call "LJM_eWriteName.vi"("Handle In"=w348, "Name"=w346, "Value"="V 3", "error in"=w347) -> ("error out"=w344:errorcluster)  [unwired: 10 in, 1 out]
            n199 = call "V3FGV.vi"("Error In"=w344, "action(write)"=enum16{"write", "read"}."write" ("action"), "V3 in"="V 3") -> ("Error Out"=w343:errorcluster)  [unwired: 7 in, 1 out]
            n200 = call "CtrlVtoGain.vi"("error in (no error)"=w343, "CtrlV(V)"="V 3", "Channel"=enum16{"Ch1", "Ch2", "Ch3"}."Ch3" ("Enum")) -> ("error out"=w351:errorcluster, "Gain"=w350:dbl)  [unwired: 7 in]
            n201 = local write "Gain3"(w350) -> ()
          }
          event "V 4": Value Change {
            n202 = event-data() -> ()  [unwired: 1 in, 6 out]
            n203 = call "LabJack_FGV.vi"("Operation(Read)"=enum16{"Write", "Read"}."Read" ("Operation"), "error in (no error)"=w358) -> ("error out"=w362:errorcluster, "Read data"=w363:i32)  [unwired: 8 in]
            n204 = global read "GlobalVariables.vi" "Ch4 LJ pin"() -> (w361:string)
            n205 = call "LJM_eWriteName.vi"("Handle In"=w363, "Name"=w361, "Value"="V 4", "error in"=w362) -> ("error out"=w360:errorcluster)  [unwired: 10 in, 1 out]
            n206 = call "V4FGV.vi"("Error In"=w360, "action(write)"=enum16{"write", "read"}."write" ("action"), "V3 in"="V 4") -> ("Error Out"=w359:errorcluster)  [unwired: 7 in, 1 out]
            n207 = call "CtrlVtoGain.vi"("error in (no error)"=w359, "CtrlV(V)"="V 4", "Channel"=enum16{"Ch1", "Ch2", "Ch3", "Ch4"}."Ch4") -> ("error out"=w366:errorcluster, "Gain"=w365:dbl)  [unwired: 7 in]
            n208 = local write "Gain4"(w365) -> ()
          }
          event "Quit": Value Change {
            # "Exit Button Value Change (pressed) Event\n(when pressed.  quite)"
            n209 = event-data() -> ()  [unwired: 1 in, 1 out]
            n210 = call <vilib>:"Add State(s) to Queue__JKI_lib_State_Machine.vi"("State(s) in Front (\"\")"="LED: Off\nMacro: Exit", "State(s) in (\"\")"=w374) -> ("States Out"=w373:string)  [unwired: 13 in]
          }
          event "Show BG": Value Change {
            n211 = event-data() -> ()  [unwired: 1 in, 6 out]
            n212 = call <vilib>:"Add State(s) to Queue__JKI_lib_State_Machine.vi"("State(s) in Front (\"\")"="Data: showBG" ("State(s) in Front (\"\")"), "State(s) in (\"\")"=w377) -> ("States Out"=w376:string)  [unwired: 13 in]
          }
          event "StartButton": Mouse Enter {
            n213 = event-data() -> ()  [unwired: 1 in, 4 out]
            n214 = local write "Help"("Press to start aquisition." ("Help")) -> ()
          }
          event "StartButton": Value Change {
            # "[Covers: REQ32]"
            # "start PWM before acquisition"
            # "Initialize both digitizer aquisition and\n send user event to trigger aquisition loop"
            n215 = event-data() -> ()  [unwired: 1 in, 6 out]
            n216 = local write "StartButton"(FALSE ("StartButton")) -> ()
            n217 = Bundle By Name(cluster=w386, "SysRunning?"=TRUE) -> (w388:T23)
            n218 = call <vilib>:"Add State(s) to Queue__JKI_lib_State_Machine.vi"("State(s) in Front (\"\")"="TCP: stopCam\nUtility: SetDataClass >> Data\nQueue: Flash\nUI: Update\nUtility: StartBeep\nLabJack: 355_PWM_Start\nLabJack: AB_Start\nLabJack: SetV\nDigitizer: Start\nUtility: AquiTimerReset\nUI: DuringAquisition\nLED: BreathGreen\nTCP: sendRunNum\nTCP: sendVideoSource\nTCP: sendChannel\nTCP: startRun", "State(s) in (\"\")"=w390) -> ("States Out"=w391:string)  [unwired: 13 in]
          }
          event User Event {
            # "[Covers: REQ32]"
            # "start PWM before acquisition"
            # "Initialize both digitizer aquisition and\n send user event to trigger aquisition loop"
            n219 = event-data() -> ()  [unwired: 1 in, 5 out]
            n220 = Bundle By Name(cluster=w393, "SysRunning?"=TRUE) -> (w395:T23)
            n221 = call <vilib>:"Add State(s) to Queue__JKI_lib_State_Machine.vi"("State(s) in Front (\"\")"="TCP: stopCam\nUtility: SetDataClass >> Data\nQueue: Flash\nUI: Update\nUtility: StartBeep\nLabJack: 355_PWM_Start\nLabJack: AB_Start\nLabJack: SetV\nDigitizer: Start\nUtility: AquiTimerReset\nUI: DuringAquisition\nLED: BreathGreen\nTCP: sendRunNum\nTCP: sendVideoSource\nTCP: sendChannel\nTCP: startRun", "State(s) in (\"\")"=w397) -> ("States Out"=w398:string)  [unwired: 13 in]
          }
          event "Video Display": Value Change {
            n222 = event-data() -> ("NewVal"=w404:bool)  [unwired: 1 in, 5 out]
            n223 = Select(t="TCP: startCam", s=w404, f="TCP: stopCam") -> (s? t:f=w401:string)
            n224 = call <vilib>:"Add State(s) to Queue__JKI_lib_State_Machine.vi"("State(s) in (\"\")"=w403, "State(s) at Back (\"\")"=w401) -> ("States Out"=w402:string)  [unwired: 13 in]
          }
          event "Video Source": Value Change {
            n225 = event-data() -> ()  [unwired: 1 in, 6 out]
            n226 = call <vilib>:"Add State(s) to Queue__JKI_lib_State_Machine.vi"("State(s) in Front (\"\")"="TCP: sendVideoSource" ("State(s) in Front (\"\")"), "State(s) in (\"\")"=w409) -> ("States Out"=w408:string)  [unwired: 13 in]
          }
          event "StopButton": Mouse Enter {
            n227 = event-data() -> ()  [unwired: 1 in, 4 out]
            n228 = local write "Help"("Press to stop data aquisition." ("Help")) -> ()
          }
          event "StopButton": Value Change {
            # "if system is running, send stop command, if not do nothing."
            # "stop aquisition\nupdate UI"
            n229 = event-data() -> ()  [unwired: 1 in, 6 out]
            n230 = Unbundle By Name(w417) -> ("SysRunning?"=w419:bool)
            n231 = case shown="True" w419 {
              tunnel: ["" ("Empty String Constant") "LabJack: AB_Stop\nLabJack: 355_PWM_Stop\n/*Digitizer: Abort"] -> w420
              tunnel: w417 -> [w424 w428]
              tunnel: [w424 w427] -> w418
              frame False {
              }
              frame True {
                n232 = Bundle By Name(cluster=w428, "SysRunning?"=FALSE) -> (w427:T23)
              }
            }
            n233 = call <vilib>:"Add State(s) to Queue__JKI_lib_State_Machine.vi"("State(s) in Front (\"\")"=w420, "State(s) in (\"\")"=w422) -> ("States Out"=w423:string)  [unwired: 13 in]
            n234 = local write "StopButton"(FALSE ("StopButton")) -> ()
          }
          event User Event {
            # "if system is running, send stop command, if not do nothing."
            # "stop aquisition\nupdate UI"
            n235 = event-data() -> ()  [unwired: 1 in, 5 out]
            n236 = Unbundle By Name(w430) -> ("SysRunning?"=w432:bool)
            n237 = case shown="True" w432 {
              tunnel: ["" ("Empty String Constant") "LabJack: AB_Stop\nLabJack: 355_PWM_Stop\n/*Digitizer: Abort"] -> w433
              tunnel: w430 -> [w437 w441]
              tunnel: [w437 w440] -> w431
              frame False {
              }
              frame True {
                n238 = Bundle By Name(cluster=w441, "SysRunning?"=FALSE) -> (w440:T23)
              }
            }
            n239 = call <vilib>:"Add State(s) to Queue__JKI_lib_State_Machine.vi"("State(s) in Front (\"\")"=w433, "State(s) in (\"\")"=w435) -> ("States Out"=w436:string)  [unwired: 13 in]
          }
          event "Sys Reconfig": Mouse Enter {
            n240 = event-data() -> ()  [unwired: 1 in, 4 out]
            n241 = local write "Help"("Click to reconfig digitizer settings." ("Help")) -> ()
          }
          event "Sys Reconfig": Value Change {
            # "everytime the user change data aquisition setting, need to reinitilize decon engine and realign iRF.\ncheck whether data length has changed, if changed, reinitialize Decon engine\nreset BG ready, need a new BG"
            # "update DAQ FGV"
            n242 = event-data() -> ()  [unwired: 1 in, 6 out]
            n243 = call "SystemConfigEditorV6.vi"("error in"=w457) -> ("error out"=w456:errorcluster, "FLImDAQ out"=w451:T5)  [unwired: 1 in]
            n244 = Unbundle By Name(w454) -> ("FLImDAQ.min record length"=w453:i32)
            n245 = Unbundle By Name(w451) -> ("min record length"=w452:i32)
            n246 = call "FLImDAQ_FGV.vi"("error in (no error)"=w456, "Operation (Read)"=enum16{"Write", "Read"}."Write" ("Operation"), "Write data"=w451) -> ("error out"=w455:errorcluster, "Read data"=w450:T5)  [unwired: 7 in]
            n247 = Equal?(x=w453, y=w452) -> (x = y?=w449:bool)
            n248 = case shown="False" w449 {
              tunnel: ["UI: Cursor Set >> Busy\nDigitizer: Config\nDeconEngine: InitializeCh1\nDeconEngine: InitializeCh2\nDeconEngine: InitializeCh3\nUI: CaliAndiRFNotReady\n/*UI iRF not ready\nUI: Update\nUI: Cursor Set >> Idle" "UI: Cursor Set >> Busy\nDigitizer: Config\nUI: Update\nUI: Cursor Set >> Idle"] -> w448
              frame False {
              }
              frame True {
              }
            }
            n249 = Bundle By Name(cluster=w454, "FLImDAQ"=w450) -> (w460:T23)
            n250 = call <vilib>:"Add State(s) to Queue__JKI_lib_State_Machine.vi"("State(s) in Front (\"\")"=w448, "State(s) in (\"\")"=w458) -> ("States Out"=w459:string)  [unwired: 13 in]
          }
          event "System Hardware Connection Status", "StartButton", "StopButton", "355nm Laser toggle", "Aiming beam toggle", "Cali&iRF alignment", "Background", "Sys Reconfig": Mouse Leave {
            n251 = event-data() -> ()  [unwired: 1 in, 4 out]
            n252 = invoke on="Help" class="Str" method="Reinit To Default"() -> ()  [unwired: 3 in, 3 out]
          }
          event "System Hardware Connection Status.Digitizer": Mouse Enter {
            n253 = event-data() -> ()  [unwired: 1 in, 4 out]
            n254 = local write "Help"("Status of hardware connections. TCP/IP is optional." ("Help")) -> ()
          }
          event "TCP Connect": Value Change {
            n255 = event-data() -> ("NewVal"=w470:bool)  [unwired: 1 in, 5 out]
            n256 = case shown="True" w470 {
              tunnel: ["TCP: Close\nUI: Update" ("State(s) in Front (\"\")") "TCP: SendSettingMacro\nUI: Update" ("State(s) in Front (\"\")")] -> w471
              frame False {
              }
              frame True {
              }
            }
            n257 = call <vilib>:"Add State(s) to Queue__JKI_lib_State_Machine.vi"("State(s) in Front (\"\")"=w471, "State(s) in (\"\")"=w473) -> ("States Out"=w472:string)  [unwired: 13 in]
          }
          event User Event {
            # "if aquisition loop is error out. Stop digitizer, update front panel indicator, stop both laser and \nOption 1: parse and save data\nOption 2: Flash queue if scout run. [Covers: REQ23]"
            n258 = event-data() -> ()  [unwired: 1 in, 5 out]
            n259 = case shown="\"Data\", Default" "Data Class" {
              tunnel: [w495 "UI: Cursor Set >> Busy\nUtility: SetAllChanAutoGain\nUtility: RestoreDeConChan\nData: parseRunData\nData: irfAlignment\nUI: Cursor Set >> Idle" "UI: Cursor Set >> Busy\nUtility: SetAllChanAutoGain\nUtility: RestoreDeConChan\nData: parseRunData\nData: saveBGtoFGV\nData: saveBGtoFile\nUI: Cursor Set >> Idle\nData: showBG\nRun: BGIncrement"] -> w485
              frame "Data", Default {
                n260 = local read "Video Display"() -> (w497:bool)
                n261 = Select(t="TCP: startCam", s=w497, f="") -> (s? t:f=w493:string)
                n262 = call <vilib>:"Add State(s) to Queue__JKI_lib_State_Machine.vi"("State(s) in Front (\"\")"="UI: Cursor Set >> Busy\nData: parseRunData\nData: saveRunData\nUI: Cursor Set>>Idle" ("State(s) in Front (\"\")"), "State(s) in (\"\")"=w493) -> ("States Out"=w495:string)  [unwired: 13 in]
              }
              frame "Cali" {
              }
              frame "BG" {
              }
            }
            n263 = Bundle By Name(cluster=w487, "SysRunning?"=FALSE) -> (w488:T23)
            n264 = Select(t="" ("State(s) in Front (\"\")"), s="Skip Data Save?", f=w485) -> (s? t:f=w482:string)
            n265 = call <vilib>:"Add State(s) to Queue__JKI_lib_State_Machine.vi"("State(s) in Front (\"\")"="TCP: stopRun\nUI: Update\nLabJack: AB_Stop\nLabJack: 355_PWM_Stop\nDigitizer: Abort\nLabJack: ZeroV\nUtility: EndBeep\nLED: BreathOff" ("State(s) in Front (\"\")"), "State(s) in (\"\")"=w482, "State(s) at Back (\"\")"="Macro: SysReadyForAq\nUI: Update" ("State(s) in Front (\"\")")) -> ("States Out"=w480:string)  [unwired: 12 in]
            n266 = call <vilib>:"Add State(s) to Queue__JKI_lib_State_Machine.vi"("State(s) in Front (\"\")"=w480, "State(s) in (\"\")"=w489) -> ("States Out"=w490:string)  [unwired: 13 in]
          }
          event Panel Close? {
            # "Discard the event because we'll close the front panel ourselves in Macro: Exit"
            # "Close Panel button (pressed) Event\n(this executes Macro: Exit to terminate the VI)"
            n267 = event-data() -> ()  [unwired: 1 in, 1 out]
            n268 = event-data ("Event Filter Node")("Discard?"=TRUE) -> ()  [unwired: 1 in, 1 out]
            n269 = call <vilib>:"Add State(s) to Queue__JKI_lib_State_Machine.vi"("State(s) in Front (\"\")"="Macro: Exit", "State(s) in (\"\")"=w505) -> ("States Out"=w504:string)  [unwired: 13 in]
          }
        }
      }
      frame "---------- Macro ----------" {
        # "Do not put any code in this frame.\n(It is a separator no-op. You can make a copy of this frame to create a new Macro frame)"
        n270 = call <vilib>:"Add State(s) to Queue__JKI_lib_State_Machine.vi"("State(s) in (\"\")"=w510) -> ("States Out"=w509:string)  [unwired: 14 in]
      }
      frame "Macro: Initialize" {
        # "load Labjack setting 1st as it contaisn laser pin infortmation"
        # "start laser 1st, need 7.5s for laser to get ready"
        # "Initialization Macro\n(This is called once, when the VI starts)"
        n271 = call <vilib>:"Add State(s) to Queue__JKI_lib_State_Machine.vi"("State(s) in Front (\"\")"="UI: showDisclaimer\nUI: Cursor Set >> Busy\nData: Initialize\nInitialize Core Data\nUI: Initialize\nUI: Front Panel State >> Open\nMacro: LoadSysConfig\nTCP: InitializeNew\nTCP: checkSource\nUI: Update\nLabJack: Open\nLabJack: SetDefaultSub\nLED: OpenVIRef\nLED: BreathOrange\nUI: Update\n355 Laser: CheckControllerStatus\n355 Laser: Laser enable\n355 Laser: Dewelling>>500\n355 Laser: CheckControllerStatus\nUI: Update\nLabJack: 355_PWM_Config\nLabJack: AB_PWM_Config\nUI: Update", "State(s) in (\"\")"="Digitizer: Initialize\nDigitizer: Config\nUI: Update\nAimingBeam: Initialize\nAimingBeam: Set APC Status>>Disable\nAimingBeam: Set ACC Status>>Enable\nAimingBeam: Set Current\nUI: Update\n355 Laser: Check Dewelling\nUI: Cursor Set >> Idle\nCase: GetID\nUI: Update\nTCP: SendSettingMacro\nCase: CreatFileStruct\nUI: Update\nData: loadLastUseMacro\nDeconEngine: InitDotNet\nDeconEngine: loadIRF\nDeconEngine: Warmup\nClassifier: Init\nGraph: SetXMultiplier\nGraph: AddCursors\nAPD: Initialize\nAPD: LoadFromSerial\nAPD: UpdateCtrlVLimit\nAPD: GetGainLimits\nPID: loadPID\nLED: BreathOff\nMacro: SysReadyForAq") -> ("States Out"=w511:string)  [unwired: 13 in]
        n272 = call <vilib>:"Add State(s) to Queue__JKI_lib_State_Machine.vi"("State(s) in Front (\"\")"=w511, "State(s) in (\"\")"=w519) -> ("States Out"=w518:string)  [unwired: 13 in]
        "Help" <- "Hover over controls to see help!" ("Help")
      }
      frame "Macro: LoadSysConfig" {
        # "System configuration Macro. [Covers: REQ15]\n(Load configurations for different component of the system)"
        n273 = call <vilib>:"Add State(s) to Queue__JKI_lib_State_Machine.vi"("State(s) in Front (\"\")"="SysConfig: Load Sys Config\nSysConfig: Load Digitizer Setting\nSysConfig: Load AB setting\nSysConfig: Load LJ Pinout\nSysConfig: Load 355 PWM\nSysConfig: LoadAPDSerialNumber\nSysConfig: LoadABVideoSetting\nSysConfig: LoadCursorLocation", "State(s) in (\"\")"=w525) -> ("States Out"=w524:string)  [unwired: 13 in]
      }
      frame "Macro: SysReadyForAq" {
        # "Macro for system ready\n(It is a separator no-op. You can make a copy of this frame to create a new Macro frame)"
        n274 = call <vilib>:"Add State(s) to Queue__JKI_lib_State_Machine.vi"("State(s) in Front (\"\")"="UI: ReadyForAquisition\nLED: Green" ("State(s) in Front (\"\")"), "State(s) in (\"\")"=w531) -> ("States Out"=w530:string)  [unwired: 13 in]
      }
      frame "Macro: Exit" {
        # "close LJ last"
        # "check whether hardware is initilized, if so close, if not do nothing"
        # "Exit Macro, close all hardware\n(This is called once, when the VI exits)"
        n275 = Unbundle By Name(w550) -> ("System Status.Digitizer"=w546:bool, "System Status.Aiming Beam"=w545:bool, "System Status.355 Laser"=w544:bool, "System Status.Labjack"=w535:bool, "Core.Close Panel on Exit?"=w539:bool)
        n276 = case shown="True" w546 {
          tunnel: ["" ("Empty String Constant") "Digitizer: Close"] -> w541
          frame False {
          }
          frame True {
          }
        }
        n277 = case shown="True" w535 {
          tunnel: ["" ("Empty String Constant") "LabJack: SetDefaultAndClose"] -> w532
          frame False {
          }
          frame True {
          }
        }
        n278 = case shown="True" w545 {
          tunnel: ["" ("Empty String Constant") "AimingBeam: Set ACC Status >> Disable\nAimingBeam: Close"] -> w534
          frame False {
          }
          frame True {
          }
        }
        n279 = case shown="True" w544 {
          tunnel: ["" ("Empty String Constant") "355 Laser: Close\n355 Laser: CheckControllerStatus"] -> w533
          frame False {
          }
          frame True {
          }
        }
        n280 = Select(t="UI: Front Panel State >> Close", s=w539, f="" ("Empty String Constant")) -> (s? t:f=w536:string)
        n281 = call <vilib>:"Add State(s) to Queue__JKI_lib_State_Machine.vi"("State(s) in Front (\"\")"="TCP: Close\nDeconEngine: CloseNetRef\nClassifier: Close", "State(s) in (\"\")"=w541, "State(s) at Back (\"\")"=w534) -> ("States Out"=w543:string)  [unwired: 12 in]
        n282 = call <vilib>:"Add State(s) to Queue__JKI_lib_State_Machine.vi"("State(s) in Front (\"\")"=w543, "State(s) in (\"\")"=w533, "State(s) at Back (\"\")"=w532) -> ("States Out"=w538:string)  [unwired: 12 in]
        n283 = call <vilib>:"Add State(s) to Queue__JKI_lib_State_Machine.vi"("State(s) in Front (\"\")"=w538, "State(s) in (\"\")"="UI: Update\nUI: Reset\nGraph: SaveCursorLoc\nLED: CloseVIRef\nQueue: Destory\nData: Cleanup\nExit", "State(s) at Back (\"\")"=w536) -> ("States Out"=w547:string)  [unwired: 12 in]
        n284 = call <vilib>:"Add State(s) to Queue__JKI_lib_State_Machine.vi"("State(s) in Front (\"\")"=w547, "State(s) in (\"\")"=w553) -> ("States Out"=w552:string)  [unwired: 13 in]
      }
      frame "---------- Data ----------" {
        # "Do not put any code in this frame.\n(It is a separator no-op. You can make a copy of this frame to create a new Data frame)"
        n285 = call <vilib>:"Add State(s) to Queue__JKI_lib_State_Machine.vi"("State(s) in (\"\")"=w566) -> ("States Out"=w565:string)  [unwired: 14 in]
      }
      frame "Data: Initialize" {
        w567 = path ""  # CaliPath
        w568 = dbl[] []  # V4
        w569 = dbl[][] []  # Ch4Data
        w570 = FALSE  # bothVidSourceAvail
        w571 = T1 {"Main Frame Grabber"=FALSE, "Side Frame Grabber"=FALSE, "Main Camera"=FALSE, "Side Camera"=FALSE}  # video source
        w572 = FALSE  # LED vi ref open?
        w574 = T22 {"DeCon Channel"=enum."1", "Scale Bar"=FALSE, "Scale Low"=3.0, "Scale High"=8.0, "ANSI"=20.0, "Radius"=1.0, "3D?"=FALSE, "Firefly?"=FALSE, "Pentero?"=FALSE}  # VideoConfig
        w575 = T26 {"Ch1APDSerial#"="", "Ch2APDSerial#"="", "Ch3APDSerial#"="", "Ch4APDSerial#"=""}  # APDSerialNum
        w576 = u32 0  # Aquisition Timer
        w577 = cluster{"RunID":i8, "BG ID":i8, "Cali ID":i8} {"RunID"=1, "BG ID"=1, "Cali ID"=1}  # IDs
        w578 = refnum<vi> refnum  # LED vi reference
        w579 = path ""  # TempPath
        w580 = T27 {"DataPath"=path "", "BG Path"=path "", "iRFPath"=path "", "CaliPath"=path ""}  # Pathes
        w582 = dbl[] []  # V3
        w583 = dbl[] []  # V2
        w584 = dbl[] []  # V1
        w586 = u32 0  # FastTimer
        w587 = u32 0  # SlowTimer
        w588 = dbl[][] []  # Ch3Data
        w589 = dbl[][] []  # Ch2Data
        w573 = dbl[][] []  # Ch1Data
        w592 = T2 {"Digitizer"=FALSE, "Labjack"=FALSE, "Aiming Beam"=FALSE, "355 Laser"=FALSE, "TCP/IP"=FALSE}  # System Status
        w593 = T28 {"DIO_EF_CLOCK1_DIVISOR"=16, "DIO_EF_CLOCK1_ROLL_VALUE"=25000, "DIO#_EF_INDEX"=0, "DIO#_EF_OPTIONS"=1, "DIO#_EF_CONFIG_A"=6250}  # AB PWM setting
        w594 = T4 {"Ch1 Bias"="TDA11", "Ch2 Bias"="DAC10", "Ch3 Bias"="DAC0", "Ch4 Bias"="DAC0", "355 PWM"="FIO0", "AimingBeam PWM"="FIO2", "Laser Ready"="FIO3", "Interlock"="FIO1", "Laser Start/Stop"="FIO1", "Red LED"="FIO1", "Green LED"="FIO1", "Foot Pedal"="DIO15"}  # LJ Pinout
        w595 = 0  # TCP attempt count
        w596 = u32 0  # Laser start tic
        w597 = refnum<k20>[] []  # niTClk sessions
        w598 = u32 0  # Last Trigger
        w599 = T28 {"DIO_EF_CLOCK1_DIVISOR"=16, "DIO_EF_CLOCK1_ROLL_VALUE"=25000, "DIO#_EF_INDEX"=0, "DIO#_EF_OPTIONS"=1, "DIO#_EF_CONFIG_A"=6250}  # 355 PWM setting
        w600 = T29 {"Aiming Beam COM Port"="COM3", "Min Current"=0.0, "Max Current"=63.0, "Default Current"=20.0, "Freq"=0}  # AB Cluster
        w601 = T30 {"resource name"="", "resource name 2"="", "Channel"=enum."Channel 0", "trigger source"="VAL_EXTERNAL", "trigger level"=0.5, "trigger delay"=1.35e-07, "min sample rate"=12500000000.0, "min record length"=2500, "vertical range"=1.0, "vertical offset"=-0.25, "Waveform to Avg"=2000}  # FLImDAQ
        w602 = FALSE  # SysRunning?
        w590 = path ""  # DefaultPath
        w603 = ""  # CaseID
        w604 = T7 {"Ch1Enable?"=FALSE, "Ch2Enable?"=FALSE, "Ch3Enable?"=FALSE, "Ch1AutoGain?"=FALSE, "Ch2AutoGain?"=FALSE, "Ch3AutoGain?"=FALSE, "AimingBeamEnable?"=FALSE}  # SysConfigCluster
        w605 = T31 {"Current VI Reference"=refnum, "Close Panel on Exit?"=FALSE}  # Core
        # "Initialize the shift-register data, here.\n(data names are defined by what you wire into the bundle function)"
        n286 = Bundle("Core"=w605, "SysConfigCluster"=w604, "System Status"=w592, "IDs"=w577, "CaseID"=w603, "DefaultPath"=w590, "Pathes"=w580, "FLImDAQ"=w601, "SysRunning?"=w602, "AB Cluster"=w600, "LJ Pinout"=w594, "355 PWM setting"=w599, "AB PWM setting"=w593, "Last Trigger"=w598, "niTClk sessions"=w597, "Laser start tic"=w596, "TCP attempt count"=w595, "Ch1Data"=w573, "Ch2Data"=w589, "Ch3Data"=w588, "Ch4Data"=w569, "V1"=w584, "V2"=w583, "V3"=w582, "V4"=w568, "SlowTimer"=w587, "FastTimer"=w586, "listener ID"=refnum<k5> refnum, "TempPath"=w579, "CaliPath"=w567, "LED vi reference"=w578, "Aquisition Timer"=w576, "APDSerialNum"=w575, "VideoConfig"=w574, "LED vi ref open?"=w572, "video source"=w571, "bothVidSourceAvail"=w570) -> (w581:T23)  [unwired: 1 in]
        n287 = call <vilib>:"Add State(s) to Queue__JKI_lib_State_Machine.vi"("State(s) in (\"\")"=w608) -> ("States Out"=w607:string)  [unwired: 14 in]
      }
      frame "Data: loadLastUseMacro" {
        # "Load last use BG and Cali and iRF.\n(It is a separator no-op. You can make a copy of this frame to create a new Data frame)"
        n288 = call <vilib>:"Add State(s) to Queue__JKI_lib_State_Machine.vi"("State(s) in Front (\"\")"="Data: loadLastUseBG\nData: loadSystemCali\nData: loadLastUseiRF\n/*Data: LoadiRFFromAPDFile\nUI: CaliAndiRFLoaded\nData: ShowiRF" ("State(s) in Front (\"\")"), "State(s) in (\"\")"=w614) -> ("States Out"=w613:string)  [unwired: 13 in]
      }
      frame "Data: loadLastUseBG" {
        w618 = enum16{"write", "read"}."write" ("action")
        # "Load last use BG.\n()"
        n289 = Unbundle By Name(w637) -> ("TempPath"=w636:path)
        n290 = call "FLImDAQ_FGV.vi"() -> ("Read data"=w632:T5)  [unwired: 10 in, 1 out]
        n291 = Build Path(base path=w636, name or relative path="Background.tdms") -> (appended path=w635:path)
        n292 = call "ReadBGorCali (SubVI).vi"("DataType"=enum16{"BG", "Cali"}."BG", "error in (no error)"=w634, "file path in"=w635) -> ("error out"=w633:errorcluster, "AvgDataCluster"=w628:T32)  [unwired: 6 in, 1 out]
        n293 = Unbundle By Name(w628) -> ("Channel 1"=w615:dbl[], "Channel 2"=w627:dbl[], "Channel 3"=w620:dbl[], "Channel 4"=w617:dbl[])
        n294 = Unbundle By Name(w632) -> ("min record length"=w624:i32)
        n295 = Array Size(array=w615) -> (size(s)=w626:i32)
        "BG length" <- w626
        n296 = Equal?(x=w626, y=w624) -> (x = y?=w625:bool)
        n297 = Select(t="UI: BGLoaded" ("State(s) in Front (\"\")"), s=w625, f="UI: BGSizeError" ("State(s) in Front (\"\")")) -> (s? t:f=w629:string)
        n298 = case shown="True" w625 {
          tunnel: w615 -> [_ w648]
          tunnel: w627 -> [_ w647]
          tunnel: w620 -> [_ w646]
          tunnel: w624 -> [w643 _]
          tunnel: [w642 w648] -> w623
          tunnel: [w642 w647] -> w622
          tunnel: [w642 w646] -> w621
          tunnel: w617 -> [_ w645]
          tunnel: [w642 w645] -> w616
          frame False {
            # "If error set BG all 0, update UI"
            n299 = for {
              N: w643 -> [_]
              tunnel: [0.0] -> w642 mode=indexing
            }
          }
          frame True {
            # "If no error, check size match"
          }
        }
        n300 = call "BG4FGV.vi"("action"=w618, "BG4 in"=w616) -> ()  [unwired: 8 in, 2 out]
        n301 = call "BG3FGV.vi"("action"=w618, "BG3 in"=w621) -> ()  [unwired: 8 in, 2 out]
        n302 = call "BG1FGV.vi"("action"=w618, "BG1 in"=w623) -> ()  [unwired: 8 in, 2 out]
        n303 = call "BG2FGV.vi"("action"=w618, "BG2 in"=w622) -> ()  [unwired: 8 in, 2 out]
        n304 = call <vilib>:"Add State(s) to Queue__JKI_lib_State_Machine.vi"("State(s) in Front (\"\")"=w629, "State(s) in (\"\")"=w641) -> ("States Out"=w640:string)  [unwired: 13 in]
      }
      frame "Data: loadSystemCali" {
        # "Load last use calibration.\n()"
        n305 = Unbundle By Name(w656) -> ("CaliPath"=w655:path)
        n306 = Build Path(base path=w655, name or relative path="Calibration.tdms") -> (appended path=w651:path)
        n307 = call "ReadBGorCali (SubVI).vi"("DataType"=enum16{"BG", "Cali"}."Cali", "error in (no error)"=w650, "file path in"=w651) -> ("error out"=w652:errorcluster, "CtrlVCluster"=w654:T33, "AvgDataCluster"=w653:T32)  [unwired: 6 in]
        n308 = case shown="No Error" w652 {
          tunnel: w654 -> [w675 _]
          tunnel: w653 -> [w674 _]
          frame No Error {
            w665 = T34 {"Ch1 WF"=[], "Ch2 WF"=[], "Ch3 WF"=[], "Ch4 WF"=[], "V1"=0.0, "V2"=0.0, "V3"=0.0, "V4"=0.0}  # SysCaliData
            n309 = Unbundle By Name(w674) -> ("Channel 1"=w673:dbl[], "Channel 2"=w672:dbl[], "Channel 3"=w671:dbl[], "Channel 4"=w664:dbl[])
            n310 = Unbundle By Name(w675) -> ("V 1"=w670:dbl[], "V 2"=w669:dbl[], "V 3"=w663:dbl[], "V 4"=w661:dbl[])
            n311 = Index Array(array=w670) -> (element=w668:dbl)  [unwired: 1 in]
            n312 = Index Array(array=w669) -> (element=w667:dbl)  [unwired: 1 in]
            n313 = Index Array(array=w663) -> (element=w666:dbl)  [unwired: 1 in]
            n314 = Index Array(array=w661) -> (element=w662:dbl)  [unwired: 1 in]
            n315 = Bundle By Name(cluster=w665, "Ch1 WF"=w673, "Ch2 WF"=w672, "Ch3 WF"=w671, "Ch4 WF"=w664, "V1"=w668, "V2"=w667, "V3"=w666, "V4"=w662) -> (w676:T34)
            n316 = global write "GlobalVariables.vi" "SysCaliData"(w676) -> ()
          }
          frame Error {
          }
        }
        n317 = call <vilib>:"Add State(s) to Queue__JKI_lib_State_Machine.vi"("State(s) in (\"\")"=w660) -> ("States Out"=w659:string)  [unwired: 14 in]
      }
      frame "Data: LoadiRFFromAPDFile" {
        w706 = T15 {"Ch1 iRF"=[], "Ch2 iRF"=[], "Ch3 iRF"=[], "Ch4 iRF"=[]}  # LastUseiRF
        # "only load the last 5th  iRF for the moment"
        # "Load APD detector data\n(It is a separator no-op. You can make a copy of this frame to create a new Data frame)"
        n318 = Unbundle By Name(w728) -> ("APDSerialNum.Ch1APDSerial#"=w727:string, "APDSerialNum.Ch2APDSerial#"=w708:string, "APDSerialNum.Ch3APDSerial#"=w707:string, "APDSerialNum.Ch4APDSerial#"=w704:string)
        n319 = call "CreatFromSerialNumNoRaw.vi"("error in (no error)"=w705, "APD Serial #"=w727) -> ("error out"=w725:errorcluster, "APDClass out"=w726:refnum<class "APDClass.lvclass">)  [unwired: 8 in]
        n320 = call "CreatFromSerialNumNoRaw.vi"("error in (no error)"=w705, "APD Serial #"=w708) -> ("error out"=w716:errorcluster, "APDClass out"=w717:refnum<class "APDClass.lvclass">)  [unwired: 8 in]
        n321 = call "CreatFromSerialNumNoRaw.vi"("error in (no error)"=w705, "APD Serial #"=w707) -> ("error out"=w710:errorcluster, "APDClass out"=w711:refnum<class "APDClass.lvclass">)  [unwired: 8 in]
        n322 = call "CreatFromSerialNumNoRaw.vi"("error in (no error)"=w705, "APD Serial #"=w704) -> ("error out"=w702:errorcluster, "APDClass out"=w703:refnum<class "APDClass.lvclass">)  [unwired: 8 in]
        n323 = call-dynamic "Read iRFData.vi"("error in (no error)"=w725, "APDClass in"=w726) -> ("iRFData"=w724:T35)  [unwired: 7 in, 2 out]
        n324 = call-dynamic "Read iRFData.vi"("error in (no error)"=w716, "APDClass in"=w717) -> ("iRFData"=w720:T35)  [unwired: 7 in, 2 out]
        n325 = call-dynamic "Read iRFData.vi"("error in (no error)"=w710, "APDClass in"=w711) -> ("iRFData"=w714:T35)  [unwired: 7 in, 2 out]
        n326 = call-dynamic "Read iRFData.vi"("error in (no error)"=w702, "APDClass in"=w703) -> ("iRFData"=w701:T35)  [unwired: 7 in, 2 out]
        n327 = Unbundle By Name(w724) -> ("iRFWFsAvg"=w723:dbl[][])
        n328 = Unbundle By Name(w720) -> ("iRFWFsAvg"=w719:dbl[][])
        n329 = Unbundle By Name(w714) -> ("iRFWFsAvg"=w713:dbl[][])
        n330 = Unbundle By Name(w701) -> ("iRFWFsAvg"=w698:dbl[][])
        n331 = Array Size(array=w723) -> (size(s)=w722:i32[])
        n332 = Array Size(array=w719) -> (size(s)=w715:i32[])
        n333 = Array Size(array=w713) -> (size(s)=w709:i32[])
        n334 = Array Size(array=w698) -> (size(s)=w699:i32[])
        n335 = Index Array(array=w722, index=0) -> (element=w697:i32)
        n336 = Index Array(array=w715, index=0) -> (element=w693:i32)
        n337 = Index Array(array=w709, index=0) -> (element=w690:i32)
        n338 = Index Array(array=w699, index=0) -> (element=w687:i32)
        n339 = Subtract(x=w697, y=5) -> (x-y=w695:i32)
        n340 = Subtract(x=w693, y=5) -> (x-y=w692:i32)
        n341 = Subtract(x=w690, y=5) -> (x-y=w689:i32)
        n342 = Subtract(x=w687, y=5) -> (x-y=w686:i32)
        n343 = Index Array(array=w723, index (row)=w695) -> (element=w685:dbl[])  [unwired: 1 in]
        n344 = Index Array(array=w719, index (row)=w692) -> (element=w684:dbl[])  [unwired: 1 in]
        n345 = Index Array(array=w713, index (row)=w689) -> (element=w683:dbl[])  [unwired: 1 in]
        n346 = Index Array(array=w698, index (row)=w686) -> (element=w682:dbl[])  [unwired: 1 in]
        n347 = call "DownSampleAndShiftiRF (SubVI).vi"("ArrayIn"=w685) -> ("ArrayOut"=w681:dbl[])  [unwired: 10 in]
        n348 = call "DownSampleAndShiftiRF (SubVI).vi"("ArrayIn"=w684) -> ("ArrayOut"=w677:dbl[])  [unwired: 10 in]
        n349 = call "DownSampleAndShiftiRF (SubVI).vi"("ArrayIn"=w683) -> ("ArrayOut"=w678:dbl[])  [unwired: 10 in]
        n350 = call "DownSampleAndShiftiRF (SubVI).vi"("ArrayIn"=w682) -> ("ArrayOut"=w680:dbl[])  [unwired: 10 in]
        n351 = call <vilib>:"Add State(s) to Queue__JKI_lib_State_Machine.vi"("State(s) in (\"\")"=w731) -> ("States Out"=w730:string)  [unwired: 14 in]
        n352 = Bundle(cluster=w706, "Ch1 iRF"=w681, "Ch2 iRF"=w677, "Ch3 iRF"=w678, "Ch4 iRF"=w680) -> (w679:T15)
        n353 = global write "GlobalVariables.vi" "LastUseiRF"(w679) -> ()
      }
      frame "Data: loadLastUseiRF" {
        # "Load last use iRF.\n()"
        n354 = Unbundle By Name(w737) -> ("TempPath"=w736:path)
        n355 = Build Path(base path=w736, name or relative path="iRF.tdms") -> (appended path=w742:path)
        n356 = TDMS Open(8:w732, 11:w742) -> (0:w740:errorcluster, 3:w741:refnum<k34>)  [unwired: 5 in]
        n357 = TDMS Read(0:w741, 11:w740, 12:dbl[][] []) -> (4:w735:refnum<k34>, 10:w738:dbl[][], 15:w734:errorcluster)  [unwired: 5 in, 3 out]
        n358 = TDMS Close(8:w734, 11:w735) -> (0:w733:errorcluster)  [unwired: 1 out]
        n359 = case shown="No Error" w734 {
          tunnel: w738 -> [w752 _]
          frame No Error {
            w755 = T15 {"Ch1 iRF"=[], "Ch2 iRF"=[], "Ch3 iRF"=[], "Ch4 iRF"=[]}  # LastUseiRF
            n360 = Index Array(array=w752, index (row)=0) -> (element=w747:dbl[])  [unwired: 1 in]
            n361 = Index Array(array=w752, index (row)=1) -> (element=w748:dbl[])  [unwired: 1 in]
            n362 = Index Array(array=w752, index (row)=2) -> (element=w749:dbl[])  [unwired: 1 in]
            n363 = Index Array(array=w752, index (row)=3) -> (element=w750:dbl[])  [unwired: 1 in]
            n364 = Add Array Elements(numeric array=w747) -> (sum=w761:dbl)
            n365 = Add Array Elements(numeric array=w748) -> (sum=w759:dbl)
            n366 = Add Array Elements(numeric array=w749) -> (sum=w757:dbl)
            n367 = Add Array Elements(numeric array=w750) -> (sum=w753:dbl)
            n368 = Divide(x=w747, y=w761) -> (x/y=w760:dbl[])
            n369 = Divide(x=w748, y=w759) -> (x/y=w758:dbl[])
            n370 = Divide(x=w749, y=w757) -> (x/y=w756:dbl[])
            n371 = Divide(x=w750, y=w753) -> (x/y=w751:dbl[])
            n372 = Bundle(cluster=w755, "Ch1 iRF"=w760, "Ch2 iRF"=w758, "Ch3 iRF"=w756, "Ch4 iRF"=w751) -> (w763:T15)
            n373 = Array Size(array=w747) -> (size(s)=→"iRF length":i32)
            n374 = global write "GlobalVariables.vi" "LastUseiRF"(w763) -> ()
          }
          frame Error {
          }
        }
        n375 = call <vilib>:"Add State(s) to Queue__JKI_lib_State_Machine.vi"("State(s) in (\"\")"=w746) -> ("States Out"=w745:string)  [unwired: 14 in]
      }
      frame "Data: ShowiRF" {
        # "Show loaded iRF.\n(It is a separator no-op. You can make a copy of this frame to create a new Data frame)"
        n376 = global read "GlobalVariables.vi" "LastUseiRF"() -> (w772:T15)
        n377 = Unbundle By Name(w772) -> ("Ch1 iRF"=w771:dbl[], "Ch2 iRF"=w770:dbl[], "Ch3 iRF"=w769:dbl[], "Ch4 iRF"=w768:dbl[])
        n378 = Build Array(w771, w770, w769, w768) -> (→"iRF Graph":dbl[][])
        n379 = call <vilib>:"Add State(s) to Queue__JKI_lib_State_Machine.vi"("State(s) in (\"\")"=w777) -> ("States Out"=w776:string)  [unwired: 14 in]
      }
      frame "Data: saveCalibration" {
        # "Average data and save calibration file. [Covers: REQ11]\n(It is a separator no-op. You can make a copy of this frame to create a new Data frame)"
        n380 = Unbundle By Name(w796) -> ("Ch1Data"=w795:dbl[][], "V1"=w794:dbl[], "Ch2Data"=w793:dbl[][], "V2"=w792:dbl[], "Ch3Data"=w791:dbl[][], "V3"=w790:dbl[], "Ch4Data"=w781:dbl[][], "V4"=w780:dbl[], "Pathes.CaliPath"=w799:path, "IDs.Cali ID"=w798:i8)
        n381 = Increment(x=w798) -> (x+1=w782:i8)
        n382 = Bundle("Ch1Data"=w795, "V1"=w794) -> (w789:cluster{"Ch1Data":dbl[][], "V1":dbl[]})  [unwired: 1 in]
        n383 = Bundle("Ch4Data"=w781, "V4"=w780) -> (w779:cluster{"Ch4Data":dbl[][], "V4":dbl[]})  [unwired: 1 in]
        n384 = Bundle("Ch2Data"=w793, "V2"=w792) -> (w788:cluster{"Ch2Data":dbl[][], "V2":dbl[]})  [unwired: 1 in]
        n385 = Bundle("Ch3Data"=w791, "V3"=w790) -> (w787:cluster{"Ch3Data":dbl[][], "V3":dbl[]})  [unwired: 1 in]
        n386 = Format Value(string ("")="Calibration" ("default name"), format string="%02d", value (0)=w782) -> (output string=w801:string)
        n387 = Build Path(base path=w799, name or relative path=w801) -> (appended path=w786:path)
        n388 = call "SaveBGorCali(SubVI).vi"("Channel1"=w789, "BG path"=w786, "DataType"=enum16{"BG", "Cali"}."Cali", "Channel 2"=w788, "Channel 3"=w787, "Channel 4"=w779, "error in (no error)"=w785, "SytemID"="UCDVetMed") -> ("error out"=w784:errorcluster)  [unwired: 7 in]
        n389 = call <vilib>:"Add State(s) to Queue__JKI_lib_State_Machine.vi"("State(s) in (\"\")"=w804) -> ("States Out"=w803:string)  [unwired: 14 in]
      }
      frame "Data: saveiRF" {
        w810 = enum16{"write", "read"}."read" ("action")
        # "Get iRF from decon stracture and save it on disk.\n(It is a separator no-op. You can make a copy of this frame to create a new Data frame)"
        n390 = Unbundle By Name(w827) -> ("TempPath"=w826:path)
        n391 = call "Ch1DeconEngineFGV.vi"("action(read)"=w810) -> ("Error Out"=w832:errorcluster, "Ch1DeconEngine out"=w833:refnum<class "LaguerreDeconEngineClass.lvclass">)  [unwired: 9 in]
        n392 = call "Ch2DeconEngineFGV.vi"("action(read)"=w810) -> ("Error Out"=w830:errorcluster, "Ch2DeconEngine out"=w831:refnum<class "LaguerreDeconEngineClass.lvclass">)  [unwired: 9 in]
        n393 = call "Ch3DeconEngineFGV.vi"("action(read)"=w810) -> ("Error Out"=w828:errorcluster, "Ch3DeconEngine out"=w829:refnum<class "LaguerreDeconEngineClass.lvclass">)  [unwired: 9 in]
        n394 = call "Ch4DeconEngineFGV.vi"("action(read)"=w810) -> ("Error Out"=w809:errorcluster, "Ch3DeconEngine out"=w808:refnum<class "LaguerreDeconEngineClass.lvclass">)  [unwired: 9 in]
        n395 = Build Path(base path=w826, name or relative path="iRF" ("default name")) -> (appended path=w824:path)
        n396 = call "getIRF.vi"("error in (no error)"=w809, "LaguerreDeconEngineClass in"=w808) -> ("iRF"=w807:dbl[])  [unwired: 7 in, 2 out]
        n397 = call "getIRF.vi"("error in (no error)"=w832, "LaguerreDeconEngineClass in"=w833) -> ("iRF"=w815:dbl[])  [unwired: 7 in, 2 out]
        n398 = call "getIRF.vi"("error in (no error)"=w830, "LaguerreDeconEngineClass in"=w831) -> ("iRF"=w814:dbl[])  [unwired: 7 in, 2 out]
        n399 = call "getIRF.vi"("error in (no error)"=w828, "LaguerreDeconEngineClass in"=w829) -> ("iRF"=w813:dbl[])  [unwired: 7 in, 2 out]
        n400 = TDMS Open(8:w823, 10:T16."create or replace" ("operation (0:open)"), 11:w824) -> (0:w820:errorcluster, 3:w821:refnum<k34>)  [unwired: 4 in]
        n401 = Bundle(cluster=T15 {"Ch1 iRF"=[], "Ch2 iRF"=[], "Ch3 iRF"=[], "Ch4 iRF"=[]} ("LastUseiRF"), "Ch1 iRF"=w815, "Ch2 iRF"=w814, "Ch3 iRF"=w813, "Ch4 iRF"=w807) -> (w811:T15)
        n402 = Build Array(w815, w814, w813, w807) -> (w819:dbl[][])
        n403 = global write "GlobalVariables.vi" "LastUseiRF"(w811) -> ()
        n404 = TDMS Write(0:w821, 5:"iRF" ("group name in (Untitled)"), 7:string[] ["Ch1", "Ch2", "Ch3", "Ch4"] ("channel name(s) in (Untitled)"), 9:w819, 11:w820) -> (4:w818:refnum<k34>, 15:w817:errorcluster)  [unwired: 1 in, 2 out]
        n405 = TDMS Close(8:w817, 11:w818) -> (0:w816:errorcluster)  [unwired: 1 out]
        n406 = call <vilib>:"Add State(s) to Queue__JKI_lib_State_Machine.vi"("State(s) in (\"\")"=w836) -> ("States Out"=w835:string)  [unwired: 14 in]
      }
      frame "Data: saveBGtoFGV" {
        w863 = enum16{"write", "read"}."write" ("action")
        # "Save BG and pass it to FGV.\n(save BG to disk and set it to FGV)"
        n407 = call "DotNetFGV.vi"("Error In"=w853) -> ("Error Out"=w858:errorcluster, "reference out"=w859:refnum<k24>)  [unwired: 9 in]
        n408 = Unbundle By Name(w864) -> ("Ch1Data"=w848:dbl[][], "Ch2Data"=w846:dbl[][], "Ch3Data"=w844:dbl[][], "Ch4Data"=w842:dbl[][])
        n409 = Transpose 2D Array(2D array=w848) -> (transposed array=w862:dbl[][])
        n410 = Transpose 2D Array(2D array=w846) -> (transposed array=w861:dbl[][])
        n411 = Transpose 2D Array(2D array=w844) -> (transposed array=w860:dbl[][])
        n412 = call "AvgArrayTimeCritical.vi"("2D array"=w846) -> ("1D Avg"=w845:dbl[])  [unwired: 10 in]
        n413 = call "AvgArrayTimeCritical.vi"("2D array"=w844) -> ("1D Avg"=w843:dbl[])  [unwired: 10 in]
        n414 = call "WaveformTUA(SubVI).vi"("error in (no error)"=w858, "WF in"=w862, "new reference"=w859) -> ("error out"=w840:errorcluster, "WF out"=w849:dbl[])  [unwired: 6 in, 1 out]
        n415 = call "WaveformTUA(SubVI).vi"("error in (no error)"=w858, "WF in"=w861, "new reference"=w859) -> ("error out"=w839:errorcluster, "WF out"=w851:dbl[])  [unwired: 6 in, 1 out]
        n416 = call "WaveformTUA(SubVI).vi"("error in (no error)"=w858, "WF in"=w860, "new reference"=w859) -> ("error out"=w838:errorcluster, "WF out"=w850:dbl[])  [unwired: 6 in, 1 out]
        n417 = call "AvgArrayTimeCritical.vi"("2D array"=w848) -> ("1D Avg"=w847:dbl[])  [unwired: 10 in]
        n418 = call "AvgArrayTimeCritical.vi"("2D array"=w842) -> ("1D Avg"=w841:dbl[])  [unwired: 10 in]
        n419 = call "BG1FGV.vi"("Error In"=w840, "action"=w863, "BG1 in"=w847) -> ("Error Out"=w857:errorcluster)  [unwired: 7 in, 1 out]
        n420 = call "BG2FGV.vi"("Error In"=w839, "action"=w863, "BG2 in"=w845) -> ("Error Out"=w856:errorcluster)  [unwired: 7 in, 1 out]
        n421 = call "BG3FGV.vi"("Error In"=w838, "action"=w863, "BG3 in"=w843) -> ("Error Out"=w855:errorcluster)  [unwired: 7 in, 1 out]
        n422 = call "BG4FGV.vi"("action"=w863, "BG4 in"=w841) -> ("Error Out"=w854:errorcluster)  [unwired: 8 in, 1 out]
        n423 = Build Array(w849, w851, w850) -> (→"BGAll" →"BG Graph":dbl[][])
        n424 = Merge Errors(w857, w856, w855, w854) -> (w852:errorcluster)
        n425 = call <vilib>:"Add State(s) to Queue__JKI_lib_State_Machine.vi"("State(s) in (\"\")"=w867) -> ("States Out"=w866:string)  [unwired: 14 in]
      }
      frame "Data: saveBGtoFile" {
        w889 = "Background" ("name or relative path")
        # "Save BG to file.\n(save BG to disk both data folder and temp folder)"
        n426 = Unbundle By Name(w893) -> ("Pathes.BG Path"=w886:path, "IDs.BG ID"=w885:i8, "Ch1Data"=w883:dbl[][], "V1"=w882:dbl[], "Ch2Data"=w881:dbl[][], "V2"=w880:dbl[], "Ch3Data"=w879:dbl[][], "V3"=w878:dbl[], "Ch4Data"=w870:dbl[][], "V4"=w869:dbl[], "TempPath"=w891:path)
        n427 = Increment(x=w885) -> (x+1=w890:i8)
        n428 = Format Value(string ("")=w889, format string="%02d", value (0)=w890) -> (output string=w888:string)
        n429 = Build Path(base path=w891, name or relative path=w889) -> (appended path=w872:path)
        n430 = call "File Dialog2"("start path"=w886, "prompt"="Please select BG name, DO NOT CANCEL!", "default name"=w888) -> ("selected path"=w873:path)  [unwired: 9 in, 3 out]
        n431 = Bundle("Ch1Data"=w883, "V1"=w882) -> (w877:cluster{"Ch1Data":dbl[][], "V1":dbl[]})  [unwired: 1 in]
        n432 = Bundle("Ch4Data"=w870, "V4"=w869) -> (w868:cluster{"Ch4Data":dbl[][], "V4":dbl[]})  [unwired: 1 in]
        n433 = Bundle("Ch2Data"=w881, "V2"=w880) -> (w876:cluster{"Ch2Data":dbl[][], "V2":dbl[]})  [unwired: 1 in]
        n434 = Bundle("Ch3Data"=w879, "V3"=w878) -> (w875:cluster{"Ch3Data":dbl[][], "V3":dbl[]})  [unwired: 1 in]
        n435 = Build Array(w873, w872) -> (w871:path[])
        n436 = for {
          tunnel: w877 -> [w904]
          tunnel: w876 -> [w903]
          tunnel: w875 -> [w902]
          shift-right: [w905] -> w884
          shift-left: w874 -> [w901]
          tunnel: w871 -> [w900] mode=indexing
          tunnel: w868 -> [w898]
          n437 = call "SaveBGorCali(SubVI).vi"("Channel1"=w904, "BG path"=w900, "DataType"=enum16{"BG", "Cali"}."BG", "Channel 2"=w903, "Channel 3"=w902, "Channel 4"=w898, "error in (no error)"=w901, "SytemID"="UCDVetMed") -> ("error out"=w905:errorcluster)  [unwired: 7 in]
        }
        n438 = call <vilib>:"Add State(s) to Queue__JKI_lib_State_Machine.vi"("State(s) in (\"\")"=w896) -> ("States Out"=w895:string)  [unwired: 14 in]
      }
      frame "Data: showBG" {
        # "Show BG in seperate window.\n()"
        n439 = call "showBG.vi"() -> ()  [unwired: 12 in]
        n440 = call <vilib>:"Add State(s) to Queue__JKI_lib_State_Machine.vi"("State(s) in (\"\")"=w910) -> ("States Out"=w909:string)  [unwired: 14 in]
      }
      frame "Data: irfAlignment" {
        w911 = enum16{"write", "read"}."write" ("action")
        # "do iRF alignment in this state\n(It is a separator no-op. You can make a copy of this frame to create a new Data frame)"
        n441 = Unbundle By Name(w956) -> ("Ch1Data"=w992:dbl[][], "Ch2Data"=w991:dbl[][], "Ch3Data"=w990:dbl[][], "Ch4Data"=w933:dbl[][])
        n442 = call "Ch1DeconEngineFGV.vi"("Error In"=w932) -> ("Error Out"=w988:errorcluster, "Ch1DeconEngine out"=w989:refnum<class "LaguerreDeconEngineClass.lvclass">)  [unwired: 9 in]
        n443 = call "Ch2DeconEngineFGV.vi"("Error In"=w932) -> ("Error Out"=w986:errorcluster, "Ch2DeconEngine out"=w987:refnum<class "LaguerreDeconEngineClass.lvclass">)  [unwired: 9 in]
        n444 = call "Ch3DeconEngineFGV.vi"("Error In"=w932) -> ("Error Out"=w984:errorcluster, "Ch3DeconEngine out"=w985:refnum<class "LaguerreDeconEngineClass.lvclass">)  [unwired: 9 in]
        n445 = call "Ch4DeconEngineFGV.vi"("Error In"=w932) -> ("Error Out"=w923:errorcluster, "Ch3DeconEngine out"=w922:refnum<class "LaguerreDeconEngineClass.lvclass">)  [unwired: 9 in]
        n446 = call "AvgArray.vi"("2D array in"=w991) -> ("1D Avg out"=w938:dbl[])  [unwired: 10 in]
        n447 = call "AvgArray.vi"("2D array in"=w990) -> ("1D Avg out"=w937:dbl[])  [unwired: 10 in]
        n448 = call "AvgArray.vi"("2D array in"=w933) -> ("1D Avg out"=w912:dbl[])  [unwired: 10 in]
        n449 = call "AvgArray.vi"("2D array in"=w992) -> ("1D Avg out"=w939:dbl[])  [unwired: 10 in]
        n450 = call "RemoveDCBG.vi"("WF in"=w939) -> ("DC"=w946:dbl, "WF out"=w936:dbl[])  [unwired: 8 in, 1 out]
        n451 = call "RemoveDCBG.vi"("WF in"=w938) -> ("DC"=w943:dbl, "WF out"=w949:dbl[])  [unwired: 8 in, 1 out]
        n452 = call "RemoveDCBG.vi"("WF in"=w937) -> ("DC"=w941:dbl, "WF out"=w948:dbl[])  [unwired: 8 in, 1 out]
        n453 = call "RemoveDCBG.vi"("WF in"=w912) -> ("DC"=w916:dbl, "WF out"=w914:dbl[])  [unwired: 8 in, 1 out]
        n454 = call "computeIRFAlignment.vi"("error in (no error)"=w988, "fIRF temp"=w936, "LaguerreDeconEngineClass in"=w989) -> ("error out"=w980:errorcluster, "LaguerreDeconEngineClass out"=w981:refnum<class "LaguerreDeconEngineClass.lvclass">)  [unwired: 6 in, 1 out]
        n455 = call "computeIRFAlignment.vi"("error in (no error)"=w986, "fIRF temp"=w949, "LaguerreDeconEngineClass in"=w987) -> ("error out"=w978:errorcluster, "LaguerreDeconEngineClass out"=w979:refnum<class "LaguerreDeconEngineClass.lvclass">)  [unwired: 6 in, 1 out]
        n456 = call "computeIRFAlignment.vi"("error in (no error)"=w984, "fIRF temp"=w948, "LaguerreDeconEngineClass in"=w985) -> ("error out"=w982:errorcluster, "LaguerreDeconEngineClass out"=w983:refnum<class "LaguerreDeconEngineClass.lvclass">)  [unwired: 6 in, 1 out]
        n457 = call "computeIRFAlignment.vi"("error in (no error)"=w923, "fIRF temp"=w914, "LaguerreDeconEngineClass in"=w922) -> ("error out"=w930:errorcluster, "LaguerreDeconEngineClass out"=w931:refnum<class "LaguerreDeconEngineClass.lvclass">)  [unwired: 6 in, 1 out]
        n458 = call "Ch1DeconEngineFGV.vi"("Error In"=w980, "action(read)"=w911, "Ch1DeconEngine in"=w981) -> ("Error Out"=w976:errorcluster, "Ch1DeconEngine out"=w977:refnum<class "LaguerreDeconEngineClass.lvclass">)  [unwired: 7 in]
        n459 = call "Ch2DeconEngineFGV.vi"("Error In"=w978, "action(read)"=w911, "Ch2DeconEngine in"=w979) -> ("Error Out"=w966:errorcluster, "Ch2DeconEngine out"=w967:refnum<class "LaguerreDeconEngineClass.lvclass">)  [unwired: 7 in]
        n460 = call "Ch3DeconEngineFGV.vi"("Error In"=w982, "action(read)"=w911, "Ch3DeconEngine in"=w983) -> ("Error Out"=w960:errorcluster, "Ch3DeconEngine out"=w961:refnum<class "LaguerreDeconEngineClass.lvclass">)  [unwired: 7 in]
        n461 = call "Ch4DeconEngineFGV.vi"("Error In"=w930, "action(read)"=w911, "Ch3DeconEngine in"=w931) -> ("Error Out"=w924:errorcluster, "Ch3DeconEngine out"=w925:refnum<class "LaguerreDeconEngineClass.lvclass">)  [unwired: 7 in]
        n462 = call "setfIRF.vi"("error in (no error)"=w960, "fIRF"=w948, "LaguerreDeconEngineClass in"=w961) -> ("error out"=w964:errorcluster, "LaguerreDeconEngineClass out"=w965:refnum<class "LaguerreDeconEngineClass.lvclass">)  [unwired: 7 in]
        n463 = call "setfIRF.vi"("error in (no error)"=w924, "fIRF"=w914, "LaguerreDeconEngineClass in"=w925) -> ("error out"=w928:errorcluster, "LaguerreDeconEngineClass out"=w929:refnum<class "LaguerreDeconEngineClass.lvclass">)  [unwired: 7 in]
        n464 = call "setfIRF.vi"("error in (no error)"=w966, "fIRF"=w949, "LaguerreDeconEngineClass in"=w967) -> ("error out"=w970:errorcluster, "LaguerreDeconEngineClass out"=w971:refnum<class "LaguerreDeconEngineClass.lvclass">)  [unwired: 7 in]
        n465 = call "setfIRF.vi"("error in (no error)"=w976, "fIRF"=w936, "LaguerreDeconEngineClass in"=w977) -> ("error out"=w974:errorcluster, "LaguerreDeconEngineClass out"=w975:refnum<class "LaguerreDeconEngineClass.lvclass">)  [unwired: 7 in]
        n466 = Unbundle By Name(w956) -> ("V1"=w935:dbl[], "V2"=w955:dbl[], "V3"=w954:dbl[], "V4"=w921:dbl[])
        n467 = call "computeLCs.vi"("error in (no error)"=w974, "LaguerreDeconClass in"=w975) -> ("error out"=w972:errorcluster, "LaguerreDeconClass out"=w973:refnum<class "LaguerreDeconEngineClass.lvclass">)  [unwired: 8 in]
        n468 = call "computeLCs.vi"("error in (no error)"=w970, "LaguerreDeconClass in"=w971) -> ("error out"=w968:errorcluster, "LaguerreDeconClass out"=w969:refnum<class "LaguerreDeconEngineClass.lvclass">)  [unwired: 8 in]
        n469 = call "computeLCs.vi"("error in (no error)"=w964, "LaguerreDeconClass in"=w965) -> ("error out"=w962:errorcluster, "LaguerreDeconClass out"=w963:refnum<class "LaguerreDeconEngineClass.lvclass">)  [unwired: 8 in]
        n470 = call "computeLCs.vi"("error in (no error)"=w928, "LaguerreDeconClass in"=w929) -> ("error out"=w926:errorcluster, "LaguerreDeconClass out"=w927:refnum<class "LaguerreDeconEngineClass.lvclass">)  [unwired: 8 in]
        n471 = call-poly <vilib>:"Mean.vi"("X"=w935) -> ("mean"=w934:dbl)  [unwired: 1 out]
        n472 = call-poly <vilib>:"Mean.vi"("X"=w921) -> ("mean"=w920:dbl)  [unwired: 1 out]
        n473 = call-poly <vilib>:"Mean.vi"("X"=w955) -> ("mean"=w953:dbl)  [unwired: 1 out]
        n474 = call "getFitting.vi"("error in (no error)"=w972, "LaguerreDeconEngineClass in"=w973) -> ("Fitting"=w945:dbl[])  [unwired: 7 in, 2 out]
        n475 = call "getFitting.vi"("error in (no error)"=w968, "LaguerreDeconEngineClass in"=w969) -> ("Fitting"=w942:dbl[])  [unwired: 7 in, 2 out]
        n476 = call "getFitting.vi"("error in (no error)"=w962, "LaguerreDeconEngineClass in"=w963) -> ("Fitting"=w918:dbl[])  [unwired: 7 in, 2 out]
        n477 = call "getFitting.vi"("error in (no error)"=w926, "LaguerreDeconEngineClass in"=w927) -> ("Fitting"=w917:dbl[])  [unwired: 7 in, 2 out]
        n478 = Add(x=w946, y=w945) -> (x+y=w947:dbl[])
        n479 = Add(x=w943, y=w942) -> (x+y=w944:dbl[])
        n480 = call-poly <vilib>:"Mean.vi"("X"=w954) -> ("mean"=w952:dbl)  [unwired: 1 out]
        n481 = Add(x=w941, y=w918) -> (x+y=w940:dbl[])
        n482 = Build Array(w939, w947) -> (w959:dbl[][])
        n483 = Build Array(w938, w944) -> (w958:dbl[][])
        n484 = Build Array(w937, w940) -> (w957:dbl[][])
        n485 = Add(x=w916, y=w917) -> (x+y=w915:dbl[])
        n486 = Bundle("mean"=w934, "mean"=w953, "mean"=w952, "mean"=w920) -> (w919:T36)  [unwired: 1 in]
        n487 = Build Array(w912, w915) -> (w913:dbl[][])
        n488 = call "Calib_and_iRFAlign_confirm.vi"("Current V"=w919, "Ch4 Data"=w913, "Ch3 Data"=w957, "Ch2 Data"=w958, "Ch1 Data"=w959) -> ("Save?"=w951:bool)  [unwired: 6 in]
        n489 = case shown="True" w951 {
          tunnel: ["" ("Empty String Constant") "Data: saveCalibration\nData: saveiRF\nRun: CaliIncrement"] -> w950
          frame False {
          }
          frame True {
            # "[Covers: REQ2]"
          }
        }
        n490 = call <vilib>:"Add State(s) to Queue__JKI_lib_State_Machine.vi"("State(s) in Front (\"\")"=w950, "State(s) in (\"\")"=w995) -> ("States Out"=w994:string)  [unwired: 13 in]
      }
      frame "Data: parseRunData" {
        # "All APD bias"
        # "flash queue"
        # "Ch3&4"
        # "Ch1&2"
        # "Flash data from queue and save it in structure\n()"
        n491 = Flush Queue(queue=w1023, error in (no error)=w1022) -> (remaining elements=w1017:T37, error out=w1018:errorcluster)  [unwired: 1 out]
        n492 = Flush Queue(queue=w1028, error in (no error)=w1022) -> (remaining elements=w1026:cluster{"double data":dbl[][]}[], error out=w1019:errorcluster)  [unwired: 1 out]
        n493 = Flush Queue(queue=w1029, error in (no error)=w1022) -> (remaining elements=w1027:cluster{"double data":dbl[][]}[], error out=w1020:errorcluster)  [unwired: 1 out]
        n494 = for {
          tunnel: w1027 -> [w1045] mode=indexing
          tunnel: [w1043] -> w1012 mode=concatenating
          tunnel: [w1042] -> w1013 mode=concatenating
          n495 = Unbundle By Name(w1045) -> ("double data"=w1044:dbl[][])
          n496 = call "SeperateChanData.vi"("Input (Ch1&2)"=w1044) -> ("Ch1"=w1043:dbl[][], "Ch2"=w1042:dbl[][])
        }
        n497 = for {
          tunnel: w1026 -> [w1041] mode=indexing
          tunnel: [w1040] -> w1002 mode=concatenating
          tunnel: [w1038] -> w1003 mode=concatenating
          n498 = Unbundle By Name(w1041) -> ("double data"=w1039:dbl[][])
          n499 = call "SeperateChanData.vi"("Input (Ch1&2)"=w1039) -> ("Ch1"=w1040:dbl[][], "Ch2"=w1038:dbl[][])
        }
        n500 = call "FLImDAQ_FGV.vi"() -> ("Read data"=w1010:T5)  [unwired: 10 in, 1 out]
        n501 = Unbundle By Name(w1010) -> ("Waveform to Avg"=w1000:i16)
        n502 = for {
          tunnel: w1017 -> [w1037] mode=indexing
          tunnel: [w1036] -> w1009 mode=indexing
          tunnel: [w1035] -> w1007 mode=indexing
          tunnel: [w1034] -> w1005 mode=indexing
          tunnel: [w1033] -> w1001 mode=indexing
          n503 = Unbundle By Name(w1037) -> ("V1"=w1036:dbl, "V2"=w1035:dbl, "V3"=w1034:dbl, "V4"=w1033:dbl)
        }
        n504 = call "DuplicateV(SubVI).vi"("Averaging"=w1000, "V in"=w1009) -> ("V out"=w1008:dbl[])  [unwired: 9 in]
        n505 = Array Size(array=w1002) -> (size(s)=→"data Size":i32[])
        n506 = call "DuplicateV(SubVI).vi"("Averaging"=w1000, "V in"=w1007) -> ("V out"=w1006:dbl[])  [unwired: 9 in]
        n507 = call "DuplicateV(SubVI).vi"("Averaging"=w1000, "V in"=w1005) -> ("V out"=w1004:dbl[])  [unwired: 9 in]
        n508 = call "DuplicateV(SubVI).vi"("Averaging"=w1000, "V in"=w1001) -> ("V out"=w998:dbl[])  [unwired: 9 in]
        n509 = Bundle By Name(cluster=w1024, "Ch1Data"=w1012, "Ch2Data"=w1013, "Ch3Data"=w1002, "Ch4Data"=w1003, "V1"=w1008, "V2"=w1006, "V3"=w1004, "V4"=w998) -> (w1025:T23)
        n510 = Merge Errors(w1020, w1019, w1018) -> (w1021:errorcluster)
        n511 = Array Size(array=w1008) -> (size(s)=→"V1 Size":i32)
        n512 = Array Size(array=w1006) -> (size(s)=→"V2 Size":i32)
        n513 = Array Size(array=w1004) -> (size(s)=→"V3 Size":i32)
        n514 = Array Size(array=w998) -> (size(s)=→"V4 Size":i32)
        n515 = call <vilib>:"Add State(s) to Queue__JKI_lib_State_Machine.vi"("State(s) in (\"\")"=w1032) -> ("States Out"=w1031:string)  [unwired: 14 in]
      }
      frame "Data: saveRunData" {
        w1048 = T38 {"DataPath"=path "", "CaseID"="", "RunID"=0, "Ch1Data"=[], "Ch2Data"=[], "Ch3Data"=[], "Ch4Data"=[], "V1"=[], "V2"=[], "V3"=[], "V4"=[], "LaserRepRate"=0, "WFAverage"=0, "RunStartTime"=0}  # Data cluster
        # "Save FLIm data to disk.\n(Save to LV tdms file format)"
        n516 = Unbundle By Name(w1059) -> ("Pathes.DataPath"=w1055:path, "CaseID"=w1067:string, "IDs.RunID"=w1057:i8, "Ch1Data"=w1066:dbl[][], "Ch2Data"=w1065:dbl[][], "Ch3Data"=w1054:dbl[][], "Ch4Data"=w1047:dbl[][], "V1"=w1049:dbl[], "V2"=w1064:dbl[], "V3"=w1063:dbl[], "V4"=w1046:dbl[])
        n517 = call "FLImDAQ_FGV.vi"() -> ("Read data"=w1052:T5)  [unwired: 10 in, 1 out]
        n518 = Unbundle By Name(w1052) -> ("Waveform to Avg"=w1051:i16)
        n519 = local read "RunStartTime"() -> (w1050:u32)
        n520 = local read "Laser Rep Rate"() -> (w1053:dbl)
        n521 = Increment(x=w1057) -> (x+1=w1056:i8)
        n522 = Bundle By Name(cluster=w1048, "DataPath"=w1055, "CaseID"=w1067, "RunID"=w1056, "Ch1Data"=w1066, "Ch2Data"=w1065, "Ch3Data"=w1054, "Ch4Data"=w1047, "V1"=w1049, "V2"=w1064, "V3"=w1063, "V4"=w1046, "LaserRepRate"=w1053, "WFAverage"=w1051, "RunStartTime"=w1050) -> (w1062:T38)
        n523 = call "SaveRunData(SubVI).vi"("Data cluster"=w1062, "error in (no error)"=w1061) -> ("error out"=w1058:errorcluster)  [unwired: 13 in]
        n524 = flat-sequence {
          tunnel: w1059 -> [w1075]
          tunnel: [w1074] -> w1060
          tunnel: w1058 -> [_]
          frame #0 {
            w1072 = dbl[][] [] ("Ch1Data")
            w1073 = dbl[] [] ("V1")
            # "reset local data"
            n525 = Bundle By Name(cluster=w1075, "Ch1Data"=w1072, "Ch2Data"=w1072, "Ch3Data"=w1072, "Ch4Data"=w1072, "V1"=w1073, "V2"=w1073, "V3"=w1073, "V4"=w1073) -> (w1074:T23)
          }
        }
        n526 = case shown="No Error" w1058 {
          tunnel: ["Run: Increment" "" ("Empty String Constant")] -> w1068
          frame No Error {
          }
          frame Error {
          }
        }
        n527 = call <vilib>:"Add State(s) to Queue__JKI_lib_State_Machine.vi"("State(s) in Front (\"\")"=w1068, "State(s) in (\"\")"=w1071) -> ("States Out"=w1070:string)  [unwired: 13 in]
      }
      frame "Data: Cleanup" {
        # "Cleanup any data and references, here.\n(this is called automatically, by the Macro: Exit)"
        n528 = Unbundle By Name(w1079) -> ("Core.Current VI Reference"=w1082:refnum<vi>)
        n529 = Close Reference(reference=w1082, error in (no error)=w1081) -> (error out=w1080:errorcluster)
        n530 = call <vilib>:"Add State(s) to Queue__JKI_lib_State_Machine.vi"("State(s) in (\"\")"=w1084) -> ("States Out"=w1083:string)  [unwired: 14 in]
      }
      frame "---------- Core ----------" {
        # "Do not put any code in this frame.\n(it is a separator no-op)"
        n531 = call <vilib>:"Add State(s) to Queue__JKI_lib_State_Machine.vi"("State(s) in (\"\")"=w1089) -> ("States Out"=w1088:string)  [unwired: 14 in]
      }
      frame Default {
        w1100 = 42 items=["No error", "Argument error", "Memory is full", "Out of zone", "End of file", "File already open", "Generic file I/O error", "File not found", "File permission error", "Disk is full", "Duplicate path", "Too many files open", "System feature not enabled", "Resource file not found", "Cannot add resource", "Resource not found", "Image not found", "Image memory error", "Pen does not exist", "Config type invalid", "Config token not found", "Config parse error", "Config memory error", "Bad external code format", "Bad external code offset", "External code not present", "Null window", "Destroy window error", "Null menu", "Print aborted", "Bad print record", "Print driver error", "Windows error during printing", "Memory error during printing", "Print dialog error", "Generic print error", "Invalid device refnum", "Device not found", "Device parameter error", "Device unit error", "Cannot open device", "Device call aborted", "Generic error", "Cancelled by user", "Object ID too low", "Object ID too high", "Object not in heap", "Unknown heap", "Unknown object (invalid DefProc)", "Unknown object (DefProc not in table)", "Message out of range", "Invalid (null) method", "Unknown message", "Manager call not supported", "Bad address", "Network operation in progress", "Network operation timed out", "Connection is busy", "Network attribute not supported", "Network error", "Address in use", "System out of memory", "Connection aborted", "Connection refused", "Not connected", "Already connected", "Connection closed", "Initialization error (interapplication manager)", "Bad occurrence", "Wait on unbound occurrence handler", "Occurrence queue overflow", "Datalog type conflict", "Unused", "Unrecognized type (interapplication manager)", "Memory corrupt", "Failed to make temporary DLL", "Old CIN version", "Drag socket not found", "Failed to load drop-object", "Failed to register OLE object", "Failed to release OLE object", "Format specifier type mismatch", "Unknown format specifier", "Too few format specifiers", "Too many format specifiers", "Scan failed", "Newer CIN version", "Error converting to variant", "Runtime menu error", "Password tampered", "Variant attribute not found", "Incompatible variant data type", "Event data is not available", "Event Store is not present", "Occurrence is not found", "Event Queue is not created", "Event info is not available", "Refnum passed is NULL", "Error retrieving Class GUID", "Error retrieving CoClass GUID", "Error retrieving TypeLib GUID.", "Bad built application magic bytes.", "Specific driver is different from the specific driver associated with the Logical Name.", "There is no session opened to the class driver.", "Max Error", "MAX - Error with config objects", "MAX - Error loading configuration", "MAX - Group not supported"]
        # "Current State"
        # "Do not delete, rename, or modify this frame.\n(this is used to capture unhandled states and typos)"
        # "Handle mistyped state name (developer tool)"
        n532 = Format Into String(format string="Software Exception: Unhandled State \"%s\"." ("message"), error in=w1096, w1091) -> (resulting string=w1099:string, error out=w1098:errorcluster)  [unwired: 1 in]
        n533 = call <vilib>:"Error Cluster From Error Code.vi"("show call chain? (False)"=TRUE, "error in (no error)"=w1098, "error message (\"\")"=w1099, "error code (0)"=w1100) -> ("error out"=w1097:errorcluster)  [unwired: 5 in]
        n534 = call <vilib>:"Add State(s) to Queue__JKI_lib_State_Machine.vi"("State(s) in (\"\")"=w1095) -> ("States Out"=w1094:string)  [unwired: 14 in]
      }
      frame "Initialize Core Data" {
        # "Build default path based on the location of project"
        # "Do not delete, rename, or modify this frame.\n(this is used to determine panel behavior on exit)"
        # "originally closed?"
        # "exe?"
        # "If panel starts closed or is an EXE, then close it when we exit"
        n535 = call <vilib>:"Application Directory.vi"() -> ("Application Directory"=w1103:path)
        n536 = property on="Property Node" class="App"() -> ("App.Kind"=w1119:T18)  [unwired: 2 in, 2 out]
        n537 = property on="Property Node" class="VI"() -> ("FP.State"=w1113:T17)  [unwired: 2 in, 2 out]
        n538 = control-ref of="Current VI Reference"() -> (w1114:refnum<vi>)
        n539 = Equal?(x=w1113, y=T17."Closed" ("Front Panel Window:State")) -> (x = y?=w1111:bool)
        n540 = Strip Path(path=w1103) -> (stripped path=w1102:path)  [unwired: 1 out]
        n541 = Equal?(x=w1119, y=T18."Run Time System" ("Application:Kind")) -> (x = y?=w1117:bool)
        n542 = Build Path(base path=w1102, name or relative path="Data") -> (appended path=w1109:path)
        n543 = Build Path(base path=w1103, name or relative path="SystemTemp") -> (appended path=w1106:path)
        n544 = Build Path(base path=w1103, name or relative path="SystemCalibrationFile") -> (appended path=w1104:path)
        n545 = Or(x=w1111, y=w1117) -> (x .or. y?=w1115:bool)
        n546 = Bundle By Name(cluster=w1116, "Core.Current VI Reference"=w1114, "Core.Close Panel on Exit?"=w1115, "DefaultPath"=w1109, "TempPath"=w1106, "CaliPath"=w1104) -> (w1121:T23)
        n547 = call <vilib>:"Add State(s) to Queue__JKI_lib_State_Machine.vi"("State(s) in (\"\")"=w1123) -> ("States Out"=w1122:string)  [unwired: 14 in]
      }
      frame "Error Handler" {
        # "Unhandled Error -- Display it"
        # "Handle any errors here.\nYou can also output any states to clean-up after errors occur"
        # "Clear error"
        n548 = Unbundle By Name(w1124) -> ("code"=w1126:i32)
        n549 = case shown="Default" w1126 {
          tunnel: ["Macro: Exit" w1136 w1142] -> w1125
          tunnel: w1124 -> [w1132 _ _]
          frame Default {
            w1134 = T39 1 items=["no dialog", "OK message", "continue or stop message", "OK message + warnings", "continue/stop + warnings"] ("type of dialog (OK msg:1)")
            n550 = call <vilib>:"General Error Handler.vi"("type of dialog (OK msg:1)"=w1134, "error in (no error)"=w1132) -> ()  [unwired: 9 in, 5 out]
          }
          frame 5002 {
            n551 = Two Button Dialog(message="Laser interlock open! Please close interlock and try again! ", 1:"Safely Shutdown" ("F button name (\"Cancel\")"), 2:"OK" ("T button name (\"OK\")")) -> (T button?=w1137:bool)
            n552 = case shown="True" w1137 {
              tunnel: ["Macro: Exit" "355 Laser: CheckControllerStatus"] -> w1136
              frame False {
              }
              frame True {
              }
            }
          }
          frame 5001 {
            n553 = Two Button Dialog(message="Unable to connect to imaging computer, do you want to run data aquisiton alone? ", 1:"No" ("F button name (\"Cancel\")"), 2:"Yes" ("T button name (\"OK\")")) -> (T button?=w1143:bool)
            n554 = case shown="False" w1143 {
              tunnel: ["Macro: Exit" "" ("Empty String Constant")] -> w1142
              frame False {
              }
              frame True {
              }
            }
          }
        }
        n555 = call <vilib>:"Add State(s) to Queue__JKI_lib_State_Machine.vi"("State(s) in Front (\"\")"=w1125, "State(s) in (\"\")"=w1131) -> ("States Out"=w1130:string)  [unwired: 13 in]
      }
      frame "Exit" {
        # "Do not put any code in this frame.\n(No errors that occur here will be handled.)"
        n556 = call <vilib>:"Add State(s) to Queue__JKI_lib_State_Machine.vi"("State(s) in (\"\")"=w1154) -> ("States Out"=w1153:string)  [unwired: 14 in]
      }
      frame "---------- Case ----------" {
        # "Template Separator\n(You can make a copy of, or modify, this frame)"
        n557 = call <vilib>:"Add State(s) to Queue__JKI_lib_State_Machine.vi"("State(s) in (\"\")"=w1159) -> ("States Out"=w1158:string)  [unwired: 14 in]
      }
      frame "Case: getCaliID" {
        # "Get Calibration file #\n(You can make a copy of, or modify, this frame)"
        n558 = Unbundle By Name(w1160) -> ("Pathes.CaliPath"=w1163:path)
        n559 = call <vilib>:"Recursive File List.vi"("pattern"="*.tdms", "Treat LLBs as Folders?"=FALSE, "Folder Path"=w1163) -> ("All Files in Dir"=w1168:path[])  [unwired: 4 in, 4 out]
        n560 = for {
          tunnel: w1168 -> [w1178] mode=indexing
          tunnel: [w1177] -> w1167 mode=indexing
          tunnel: "Calibration" -> [w1174]
          n561 = Strip Path(path=w1178) -> (name=w1175:string)  [unwired: 1 out]
          n562 = Search and Replace String(input string=w1175, search string=w1174) -> (result string=w1173:string)  [unwired: 6 in, 3 out]
          n563 = Scan From String(format string="%d" ("string"), input string=w1173) -> (output 1=w1177:i32)  [unwired: 3 in, 3 out]
        }
        n564 = Array Max & Min(array=w1167) -> (max value=w1166:i32)  [unwired: 3 out]
        n565 = Bundle By Name(cluster=w1160, "IDs.Cali ID"=w1166) -> (w1161:T23)
        n566 = call <vilib>:"Add State(s) to Queue__JKI_lib_State_Machine.vi"("State(s) in (\"\")"=w1172) -> ("States Out"=w1171:string)  [unwired: 14 in]
      }
      frame "Case: getBGID" {
        # "Get background #\n(You can make a copy of, or modify, this frame)"
        n567 = Unbundle By Name(w1181) -> ("Pathes.BG Path"=w1186:path)
        n568 = call <vilib>:"Recursive File List.vi"("pattern"="*.tdms", "Treat LLBs as Folders?"=FALSE, "Folder Path"=w1186) -> ("All Files in Dir"=w1184:path[])  [unwired: 4 in, 4 out]
        n569 = for {
          tunnel: w1184 -> [w1201] mode=indexing
          tunnel: "Background" ("name or relative path") -> [w1199]
          shift-right: [w1192] -> w1179
          shift-left: 0 -> [w1196]
          n570 = Strip Path(path=w1201) -> (name=w1200:string)  [unwired: 1 out]
          n571 = Search and Replace String(input string=w1200, search string=w1199) -> (number of replacements=w1198:i32)  [unwired: 6 in, 3 out]
          n572 = Greater Than 0?(x=w1198) -> (x > 0?=w1197:bool)
          n573 = Select(t=1, s=w1197, f=0) -> (s? t:f=w1195:i32)
          n574 = Add(x=w1195, y=w1196) -> (x+y=w1192:i32)
        }
        n575 = Bundle By Name(cluster=w1181, "IDs.BG ID"=w1179) -> (w1182:T23)
        n576 = call <vilib>:"Add State(s) to Queue__JKI_lib_State_Machine.vi"("State(s) in (\"\")"=w1191) -> ("States Out"=w1190:string)  [unwired: 14 in]
      }
      frame "Case: getRunID" {
        # "Check folder for run ID\n(You can make a copy of, or modify, this frame)"
        n577 = Unbundle By Name(w1211) -> ("Pathes.DataPath"=w1210:path, "CaseID"=w1206:string)
        n578 = Build Array("Background" ("name or relative path"), "Calibration", "3DScanData" ("element")) -> (w1216:string[])
        n579 = call <vilib>:"Recursive File List.vi"("Folders to Exclude"=w1216, "pattern"="*.tdms", "Treat LLBs as Folders?"=FALSE, "Folder Path"=w1210) -> ("All Files in Dir"=w1207:path[])  [unwired: 3 in, 4 out]
        n580 = for {
          tunnel: w1207 -> [w1225] mode=indexing
          tunnel: [w1224] -> w1213 mode=indexing
          tunnel: w1206 -> [w1221]
          n581 = Strip Path(path=w1225) -> (name=w1222:string)  [unwired: 1 out]
          n582 = Search and Replace String(input string=w1222, search string=w1221) -> (result string=w1220:string)  [unwired: 6 in, 3 out]
          n583 = Scan From String(format string="_%d" ("string"), input string=w1220) -> (output 1=w1224:i32)  [unwired: 3 in, 3 out]
        }
        n584 = Array Max & Min(array=w1213) -> (max value=w1204:i32)  [unwired: 3 out]
        n585 = Bundle By Name(cluster=w1211, "IDs.RunID"=w1204) -> (w1212:T23)
        n586 = call "RunIDFGV.vi"("Error In"=w1202, "RunID in"=w1204) -> ("Error Out"=w1203:errorcluster)  [unwired: 8 in, 1 out]
        n587 = call <vilib>:"Add State(s) to Queue__JKI_lib_State_Machine.vi"("State(s) in (\"\")"=w1219) -> ("States Out"=w1218:string)  [unwired: 14 in]
      }
      frame "Case: CreatFileStruct" {
        # "Creat case file structure"
        n588 = Unbundle By Name(w1239) -> ("DefaultPath"=w1245:path, "CaseID"=w1232:string)
        n589 = Build Path(base path=w1245, name or relative path=w1232) -> (appended path=w1244:path)
        n590 = call <vilib>:"Check if File or Folder Exists.vi"("error in (no error)"=w1238, "path"=w1244) -> ("error out"=w1241:errorcluster, "file or folder exists?"=w1243:bool, "dup path"=w1242:path)  [unwired: 7 in]
        n591 = case shown="True" w1243 {
          tunnel: w1242 -> [w1262 w1270]
          tunnel: w1241 -> [w1260 w1265]
          tunnel: [w1254 w1270] -> w1230
          tunnel: [w1258 w1272] -> w1229
          tunnel: [u32 0 u32 0] -> w1228
          tunnel: [w1256 w1275] -> w1236
          tunnel: "Background" ("name or relative path") -> [w1255 w1267]
          tunnel: "Calibration" -> [w1253 w1266]
          tunnel: [w1249 w1268] -> w1233
          tunnel: w1232 -> [_ _]
          tunnel: ["" ("Empty String Constant") "Case: getRunID\nCase: getBGID\nCase: getCaliID\nUI: Update"] -> w1231
          frame False {
            # "Folder not exist. Creat folders."
            n592 = Create Folder(path (use dialog)=w1262, error in=w1260) -> (created path=w1254:path, error out=w1251:errorcluster)  [unwired: 1 in, 1 out]
            n593 = Build Path(base path=w1254, name or relative path=w1253) -> (appended path=w1252:path)
            n594 = Build Path(base path=w1254, name or relative path=w1255) -> (appended path=w1261:path)
            n595 = Create Folder(path (use dialog)=w1261, error in=w1251) -> (created path=w1256:path, error out=w1257:errorcluster)  [unwired: 1 in, 1 out]
            n596 = Create Folder(path (use dialog)=w1252, error in=w1251) -> (created path=w1249:path, error out=w1250:errorcluster)  [unwired: 1 in, 1 out]
            n597 = Merge Errors(w1257, w1250) -> (w1258:errorcluster)
          }
          frame True {
            # "Folder exsit, check file #"
            n598 = Build Path(base path=w1270, name or relative path=w1266) -> (appended path=w1271:path)
            n599 = Build Path(base path=w1270, name or relative path=w1267) -> (appended path=w1276:path)
            n600 = call <vilib>:"Check if File or Folder Exists.vi"("path"=w1271) -> ("file or folder exists?"=w1269:bool, "dup path"=w1268:path)  [unwired: 8 in, 1 out]
            n601 = call <vilib>:"Check if File or Folder Exists.vi"("path"=w1276) -> ("file or folder exists?"=w1274:bool, "dup path"=w1275:path)  [unwired: 8 in, 1 out]
            n602 = And(x=w1274, y=w1269) -> (x .and. y?=w1273:bool)
            n603 = case shown="False" w1273 {
              tunnel: w1265 -> [_ w1278]
              tunnel: [errorcluster {"status"=TRUE, "code"=5003, "source"="File structure error."} ("error out") w1278] -> w1272
              frame False {
              }
              frame True {
              }
            }
          }
        }
        n604 = Bundle By Name(cluster=w1239, "Pathes.DataPath"=w1230, "Pathes.BG Path"=w1236, "Pathes.CaliPath"=w1233, "IDs.RunID"=w1228, "IDs.BG ID"=w1228, "IDs.Cali ID"=w1228) -> (w1240:T23)
        n605 = call "DataRootPathFGV.vi"("Error In"=w1229, "PathIn"=w1230) -> ("Error Out"=w1227:errorcluster)  [unwired: 8 in, 1 out]
        n606 = call "RunIDFGV.vi"("Error In"=w1227, "RunID in"=w1228) -> ("Error Out"=w1226:errorcluster)  [unwired: 8 in, 1 out]
        n607 = call <vilib>:"Add State(s) to Queue__JKI_lib_State_Machine.vi"("State(s) in Front (\"\")"=w1231, "State(s) in (\"\")"=w1247) -> ("States Out"=w1246:string)  [unwired: 13 in]
      }
      frame "Case: GetID" {
        # "Template Separator\n(You can make a copy of, or modify, this frame)"
        n608 = call "set_subjectID.vi"() -> ("subject_id"=w1279:string)  [unwired: 10 in]
        n609 = Bundle By Name(cluster=w1281, "CaseID"=w1279) -> (w1282:T23)
        n610 = call <vilib>:"Add State(s) to Queue__JKI_lib_State_Machine.vi"("State(s) in (\"\")"=w1285) -> ("States Out"=w1284:string)  [unwired: 14 in]
      }
      frame "---------- DeconEngine ----------" {
        # "start data aquisition and then set irfAligh to ture and decon channel to 1,2 and 3."
        # "Template Separator\n(You can make a copy of, or modify, this frame)"
        n611 = call <vilib>:"Add State(s) to Queue__JKI_lib_State_Machine.vi"("State(s) in (\"\")"=w1290) -> ("States Out"=w1289:string)  [unwired: 14 in]
      }
      frame "DeconEngine: InitDotNet" {
        # "Initialize Dot Net Decon and save the FGV"
        # "Initilize Dot Net \n(You can make a copy of, or modify, this frame)"
        n612 = constructor on="Constructor Node" class="LaguerreDeCon"(error in=w1291) -> (reference out=w1294:refnum<k24>, error out=w1293:errorcluster)  [unwired: 2 in, 1 out]
        n613 = call "DotNetFGV.vi"("Error In"=w1293, "Operation (Read)"=enum16{"Read", "Write"}."Write", "reference in"=w1294) -> ("Error Out"=w1292:errorcluster)  [unwired: 7 in, 1 out]
        n614 = call <vilib>:"Add State(s) to Queue__JKI_lib_State_Machine.vi"("State(s) in (\"\")"=w1299) -> ("States Out"=w1298:string)  [unwired: 14 in]
      }
      frame "DeconEngine: Warmup" {
        # "Warm up parpool\n(You can make a copy of, or modify, this frame)"
        n615 = call "DotNetFGV.vi"("Error In"=w1304) -> ("Error Out"=w1305:errorcluster, "reference out"=w1306:refnum<k24>)  [unwired: 9 in]
        n616 = flat-sequence {
          tunnel: w1304 -> [_]
          tunnel: [w1312] -> w1301
          frame #0 {
            n617 = Tick Count (ms)() -> (millisecond timer value=w1312:u32)
          }
        }
        n618 = invoke class="LaguerreDeCon" method="init_parpool"(reference=w1306, error in=w1305) -> (error out=w1303:errorcluster)  [unwired: 1 in, 2 out]
        n619 = flat-sequence {
          tunnel: w1303 -> [_]
          tunnel: [w1311] -> w1302
          frame #0 {
            n620 = Tick Count (ms)() -> (millisecond timer value=w1311:u32)
          }
        }
        n621 = Subtract(x=w1302, y=w1301) -> (x-y=→"WarmupTime(ms)":u32)
        n622 = call <vilib>:"Add State(s) to Queue__JKI_lib_State_Machine.vi"("State(s) in (\"\")"=w1310) -> ("States Out"=w1309:string)  [unwired: 14 in]
      }
      frame "DeconEngine: loadIRF" {
        # "Load IRF for decon and save to FGV\n(You can make a copy of, or modify, this frame)"
        n623 = Current VI's Path() -> (path=w1330:path)
        n624 = Strip Path(path=w1330) -> (stripped path=w1329:path)  [unwired: 1 out]
        n625 = Build Path(base path=w1329, name or relative path="DotNetDecon") -> (appended path=w1317:path)
        n626 = Build Path(base path=w1317, name or relative path="Channel1.tdms") -> (appended path=w1334:path)
        n627 = Build Path(base path=w1317, name or relative path="Channel3.tdms") -> (appended path=w1319:path)
        n628 = Build Path(base path=w1317, name or relative path="Channel2.tdms") -> (appended path=w1320:path)
        n629 = call "LoadIRF.vi"("error in (no error)"=w1318, "file path"=w1334) -> ("error out"=w1332:errorcluster, "APD"=w1333:T40)  [unwired: 8 in]
        n630 = call "LoadIRF.vi"("error in (no error)"=w1318, "file path"=w1320) -> ("error out"=w1325:errorcluster, "APD"=w1326:T40)  [unwired: 8 in]
        n631 = call "LoadIRF.vi"("error in (no error)"=w1318, "file path"=w1319) -> ("error out"=w1322:errorcluster, "APD"=w1323:T40)  [unwired: 8 in]
        n632 = call "DeConAPD1FGV.vi"("Error In"=w1332, "Operation (Read)"=enum16{"Read", "Write"}."Write", "APDClass in"=w1333) -> ("Error Out"=w1316:errorcluster)  [unwired: 7 in, 1 out]
        n633 = call "DeConAPD2FGV.vi"("Error In"=w1325, "Operation (Read)"=enum16{"Read", "Write"}."Write", "APDClass in"=w1326) -> ("Error Out"=w1315:errorcluster)  [unwired: 7 in, 1 out]
        n634 = call "DeConAPD3FGV.vi"("Error In"=w1322, "Operation (Read)"=enum16{"Read", "Write"}."Write", "APDClass in"=w1323) -> ("Error Out"=w1314:errorcluster)  [unwired: 7 in, 1 out]
        n635 = Merge Errors(w1316, w1315, w1314) -> (w1313:errorcluster)
        n636 = call <vilib>:"Add State(s) to Queue__JKI_lib_State_Machine.vi"("State(s) in (\"\")"=w1340) -> ("States Out"=w1339:string)  [unwired: 14 in]
      }
      frame "DeconEngine: CloseNetRef" {
        # "Template Separator\n(You can make a copy of, or modify, this frame)"
        n637 = call "DotNetFGV.vi"("Error In"=w1341) -> ("Error Out"=w1343:errorcluster, "reference out"=w1344:refnum<k24>)  [unwired: 9 in]
        n638 = Close Reference(reference=w1344, error in (no error)=w1343) -> (error out=w1342:errorcluster)
        n639 = call <vilib>:"Add State(s) to Queue__JKI_lib_State_Machine.vi"("State(s) in (\"\")"=w1348) -> ("States Out"=w1347:string)  [unwired: 14 in]
      }
      frame "DeconEngine: InitilizeMacro" {
        # "start data aquisition and then set irfAligh to ture and decon channel to 1,2 and 3."
        # "Initilize Decon Engine for all channel\n(You can make a copy of, or modify, this frame)"
        n640 = call <vilib>:"Add State(s) to Queue__JKI_lib_State_Machine.vi"("State(s) in Front (\"\")"="DeconEngine: InitializeCh1\nDeconEngine: InitializeCh2\nDeconEngine: InitializeCh3\nDeconEngine: InitializeCh4" ("State(s) in Front (\"\")"), "State(s) in (\"\")"=w1354) -> ("States Out"=w1353:string)  [unwired: 13 in]
      }
      frame "DeconEngine: InitializeCh1" {
        w1376 = refnum<class "LaguerreDeconEngineClass.lvclass"> refnum  # Ch1DeconObj
        # "Initilize Laguerre Deconvolution engine Object\n(You can make a copy of, or modify, this frame)"
        n641 = global read "GlobalVariables.vi" "LastUseiRF"() -> (w1357:T15)
        n642 = call "setLaguerreOrder.vi"("error in (no error)"=w1364, "LaguerreOrder"=u32 12, "LaguerreDeconClass in"=w1376) -> ("error out"=w1373:errorcluster, "LaguerreDeconClass out"=w1374:refnum<class "LaguerreDeconEngineClass.lvclass">)  [unwired: 7 in]
        n643 = Unbundle By Name(w1357) -> ("Ch1 iRF"=w1356:dbl[])
        n644 = call "setDataLength.vi"("error in (no error)"=w1373, "dataLength"=u32 600, "LaguerreDeconClass in"=w1374) -> ("error out"=w1372:errorcluster, "LaguerreDeconClass out"=w1371:refnum<class "LaguerreDeconEngineClass.lvclass">)  [unwired: 7 in]
        n645 = call "setIRF.vi"("error in (no error)"=w1372, "iRF"=w1356, "LaguerreDeconClass in"=w1371) -> ("error out"=w1369:errorcluster, "LaguerreDeconClass out"=w1370:refnum<class "LaguerreDeconEngineClass.lvclass">)  [unwired: 7 in]
        n646 = call "computeAlpha.vi"("error in (no error)"=w1369, "LaguerreDeconClass in"=w1370) -> ("error out"=w1367:errorcluster, "LaguerreDeconClass out"=w1368:refnum<class "LaguerreDeconEngineClass.lvclass">)  [unwired: 8 in]
        n647 = call "dataInitilize.vi"("error in (no error)"=w1367, "LaguerreDeconClass in"=w1368) -> ("error out"=w1365:errorcluster, "LaguerreDeconClass out"=w1366:refnum<class "LaguerreDeconEngineClass.lvclass">)  [unwired: 8 in]
        n648 = call "computeDeconMatrix.vi"("error in (no error)"=w1365, "LaguerreDeconClass in"=w1366) -> ("error out"=w1361:errorcluster, "LaguerreDeconClass out"=w1363:refnum<class "LaguerreDeconEngineClass.lvclass">)  [unwired: 8 in]
        n649 = call "Ch1DeconEngineFGV.vi"("Error In"=w1361, "action(read)"=enum16{"write", "read"}."write" ("action"), "Ch1DeconEngine in"=w1363) -> ("Error Out"=w1360:errorcluster)  [unwired: 7 in, 1 out]
        n650 = call <vilib>:"Add State(s) to Queue__JKI_lib_State_Machine.vi"("State(s) in (\"\")"=w1378) -> ("States Out"=w1377:string)  [unwired: 14 in]
      }
      frame "DeconEngine: InitializeCh2" {
        w1400 = refnum<class "LaguerreDeconEngineClass.lvclass"> refnum  # Ch2DeconObj
        # "Initilize Laguerre Deconvolution engine Object\n(You can make a copy of, or modify, this frame)"
        n651 = global read "GlobalVariables.vi" "LastUseiRF"() -> (w1381:T15)
        n652 = call "setLaguerreOrder.vi"("error in (no error)"=w1388, "LaguerreOrder"=u32 12, "LaguerreDeconClass in"=w1400) -> ("error out"=w1397:errorcluster, "LaguerreDeconClass out"=w1398:refnum<class "LaguerreDeconEngineClass.lvclass">)  [unwired: 7 in]
        n653 = Unbundle By Name(w1381) -> ("Ch2 iRF"=w1380:dbl[])
        n654 = call "setDataLength.vi"("error in (no error)"=w1397, "dataLength"=u32 600, "LaguerreDeconClass in"=w1398) -> ("error out"=w1396:errorcluster, "LaguerreDeconClass out"=w1395:refnum<class "LaguerreDeconEngineClass.lvclass">)  [unwired: 7 in]
        n655 = call "setIRF.vi"("error in (no error)"=w1396, "iRF"=w1380, "LaguerreDeconClass in"=w1395) -> ("error out"=w1393:errorcluster, "LaguerreDeconClass out"=w1394:refnum<class "LaguerreDeconEngineClass.lvclass">)  [unwired: 7 in]
        n656 = call "computeAlpha.vi"("error in (no error)"=w1393, "LaguerreDeconClass in"=w1394) -> ("error out"=w1391:errorcluster, "LaguerreDeconClass out"=w1392:refnum<class "LaguerreDeconEngineClass.lvclass">)  [unwired: 8 in]
        n657 = call "dataInitilize.vi"("error in (no error)"=w1391, "LaguerreDeconClass in"=w1392) -> ("error out"=w1389:errorcluster, "LaguerreDeconClass out"=w1390:refnum<class "LaguerreDeconEngineClass.lvclass">)  [unwired: 8 in]
        n658 = call "computeDeconMatrix.vi"("error in (no error)"=w1389, "LaguerreDeconClass in"=w1390) -> ("error out"=w1385:errorcluster, "LaguerreDeconClass out"=w1387:refnum<class "LaguerreDeconEngineClass.lvclass">)  [unwired: 8 in]
        n659 = call "Ch2DeconEngineFGV.vi"("Error In"=w1385, "action(read)"=enum16{"write", "read"}."write" ("action"), "Ch2DeconEngine in"=w1387) -> ("Error Out"=w1384:errorcluster)  [unwired: 7 in, 1 out]
        n660 = call <vilib>:"Add State(s) to Queue__JKI_lib_State_Machine.vi"("State(s) in (\"\")"=w1402) -> ("States Out"=w1401:string)  [unwired: 14 in]
      }
      frame "DeconEngine: InitializeCh3" {
        w1404 = refnum<class "LaguerreDeconEngineClass.lvclass"> refnum  # Ch3DeconObj
        # "Initilize Laguerre Deconvolution engine Object\n(You can make a copy of, or modify, this frame)"
        n661 = global read "GlobalVariables.vi" "LastUseiRF"() -> (w1406:T15)
        n662 = call "setLaguerreOrder.vi"("error in (no error)"=w1413, "LaguerreOrder"=u32 12, "LaguerreDeconClass in"=w1404) -> ("error out"=w1422:errorcluster, "LaguerreDeconClass out"=w1423:refnum<class "LaguerreDeconEngineClass.lvclass">)  [unwired: 7 in]
        n663 = Unbundle By Name(w1406) -> ("Ch3 iRF"=w1405:dbl[])
        n664 = call "setDataLength.vi"("error in (no error)"=w1422, "dataLength"=600, "LaguerreDeconClass in"=w1423) -> ("error out"=w1421:errorcluster, "LaguerreDeconClass out"=w1420:refnum<class "LaguerreDeconEngineClass.lvclass">)  [unwired: 7 in]
        n665 = call "setIRF.vi"("error in (no error)"=w1421, "iRF"=w1405, "LaguerreDeconClass in"=w1420) -> ("error out"=w1418:errorcluster, "LaguerreDeconClass out"=w1419:refnum<class "LaguerreDeconEngineClass.lvclass">)  [unwired: 7 in]
        n666 = call "computeAlpha.vi"("error in (no error)"=w1418, "LaguerreDeconClass in"=w1419) -> ("error out"=w1416:errorcluster, "LaguerreDeconClass out"=w1417:refnum<class "LaguerreDeconEngineClass.lvclass">)  [unwired: 8 in]
        n667 = call "dataInitilize.vi"("error in (no error)"=w1416, "LaguerreDeconClass in"=w1417) -> ("error out"=w1414:errorcluster, "LaguerreDeconClass out"=w1415:refnum<class "LaguerreDeconEngineClass.lvclass">)  [unwired: 8 in]
        n668 = call "computeDeconMatrix.vi"("error in (no error)"=w1414, "LaguerreDeconClass in"=w1415) -> ("error out"=w1410:errorcluster, "LaguerreDeconClass out"=w1412:refnum<class "LaguerreDeconEngineClass.lvclass">)  [unwired: 8 in]
        n669 = call "Ch3DeconEngineFGV.vi"("Error In"=w1410, "action(read)"=enum16{"write", "read"}."write" ("action"), "Ch3DeconEngine in"=w1412) -> ("Error Out"=w1409:errorcluster)  [unwired: 7 in, 1 out]
        n670 = call <vilib>:"Add State(s) to Queue__JKI_lib_State_Machine.vi"("State(s) in (\"\")"=w1426) -> ("States Out"=w1425:string)  [unwired: 14 in]
      }
      frame "DeconEngine: InitializeCh4" {
        w1428 = refnum<class "LaguerreDeconEngineClass.lvclass"> refnum  # Ch3DeconObj
        # "Initilize Laguerre Deconvolution engine Object\n(You can make a copy of, or modify, this frame)"
        n671 = global read "GlobalVariables.vi" "LastUseiRF"() -> (w1430:T15)
        n672 = call "setLaguerreOrder.vi"("error in (no error)"=w1437, "LaguerreOrder"=u32 12, "LaguerreDeconClass in"=w1428) -> ("error out"=w1446:errorcluster, "LaguerreDeconClass out"=w1447:refnum<class "LaguerreDeconEngineClass.lvclass">)  [unwired: 7 in]
        n673 = Unbundle By Name(w1430) -> ("Ch4 iRF"=w1429:dbl[])
        n674 = call "setDataLength.vi"("error in (no error)"=w1446, "dataLength"=u32 600, "LaguerreDeconClass in"=w1447) -> ("error out"=w1445:errorcluster, "LaguerreDeconClass out"=w1444:refnum<class "LaguerreDeconEngineClass.lvclass">)  [unwired: 7 in]
        n675 = call "setIRF.vi"("error in (no error)"=w1445, "iRF"=w1429, "LaguerreDeconClass in"=w1444) -> ("error out"=w1442:errorcluster, "LaguerreDeconClass out"=w1443:refnum<class "LaguerreDeconEngineClass.lvclass">)  [unwired: 7 in]
        n676 = call "computeAlpha.vi"("error in (no error)"=w1442, "LaguerreDeconClass in"=w1443) -> ("error out"=w1440:errorcluster, "LaguerreDeconClass out"=w1441:refnum<class "LaguerreDeconEngineClass.lvclass">)  [unwired: 8 in]
        n677 = call "dataInitilize.vi"("error in (no error)"=w1440, "LaguerreDeconClass in"=w1441) -> ("error out"=w1438:errorcluster, "LaguerreDeconClass out"=w1439:refnum<class "LaguerreDeconEngineClass.lvclass">)  [unwired: 8 in]
        n678 = call "computeDeconMatrix.vi"("error in (no error)"=w1438, "LaguerreDeconClass in"=w1439) -> ("error out"=w1434:errorcluster, "LaguerreDeconClass out"=w1436:refnum<class "LaguerreDeconEngineClass.lvclass">)  [unwired: 8 in]
        n679 = call "Ch4DeconEngineFGV.vi"("Error In"=w1434, "action(read)"=enum16{"write", "read"}."write" ("action"), "Ch3DeconEngine in"=w1436) -> ("Error Out"=w1433:errorcluster)  [unwired: 7 in, 1 out]
        n680 = call <vilib>:"Add State(s) to Queue__JKI_lib_State_Machine.vi"("State(s) in (\"\")"=w1450) -> ("States Out"=w1449:string)  [unwired: 14 in]
      }
      frame "---------- Digitizer ----------" {
        # "Template Separator\n(You can make a copy of, or modify, this frame)"
        n681 = call <vilib>:"Add State(s) to Queue__JKI_lib_State_Machine.vi"("State(s) in (\"\")"=w1455) -> ("States Out"=w1454:string)  [unwired: 14 in]
      }
      frame "Digitizer: Initialize" {
        # "reset digitizer to everytime the system runs"
        # "reset digitizer to everytime the system runs"
        # "Initialize digitizer.\nInitialize both digitizer and update status."
        n682 = call "FLImDAQ_FGV.vi"("error in (no error)"=w1463) -> ("error out"=w1457:errorcluster, "Read data"=w1462:T5)  [unwired: 9 in]
        n683 = Unbundle By Name(w1465) -> ("SysConfigCluster.Ch1Enable?"=w1470:bool, "SysConfigCluster.Ch2Enable?"=w1469:bool, "SysConfigCluster.Ch3Enable?"=w1467:bool)
        n684 = Unbundle By Name(w1462) -> ("Digitizer 1"=w1458:refnum<k15>, "Digitizer 2"=w1461:refnum<k15>)
        n685 = property on="Digitizer" class="Bool (strict)"("Blinking"=TRUE) -> ()  [unwired: 2 in, 2 out]
        n686 = Or(x=w1470, y=w1469) -> (x .or. y?=w1468:bool)
        n687 = case shown="True" w1468 {
          tunnel: w1457 -> [w1478 w1481]
          tunnel: [w1478 w1480] -> w1459
          tunnel: w1458 -> [_ w1482]
          frame False {
          }
          frame True {
            n688 = call <instrlib>:"niScope Initialize.vi"("resource name"=w1482, "reset device"=TRUE, "error in"=w1481) -> ("error out"=w1480:errorcluster)  [unwired: 11 in, 1 out]
          }
        }
        n689 = case shown="True" w1467 {
          tunnel: w1457 -> [w1473 w1475]
          tunnel: [w1473 w1477] -> w1464
          tunnel: w1461 -> [_ w1476]
          frame False {
          }
          frame True {
            n690 = call <instrlib>:"niScope Initialize.vi"("resource name"=w1476, "reset device"=TRUE, "error in"=w1475) -> ("error out"=w1477:errorcluster)  [unwired: 11 in, 1 out]
          }
        }
        n691 = Merge Errors(w1459, w1464) -> (w1456:errorcluster)
        n692 = call <vilib>:"Add State(s) to Queue__JKI_lib_State_Machine.vi"("State(s) in (\"\")"=w1472) -> ("States Out"=w1471:string)  [unwired: 14 in]
      }
      frame "Digitizer: Config" {
        # "Synchronize is taking time ~3s."
        # "Config  digitizer\nCall subVi to config digitizer"
        n693 = call "FLImDAQ_FGV.vi"() -> ("Read data"=w1500:T5)  [unwired: 10 in, 1 out]
        n694 = Unbundle By Name(w1509) -> ("SysConfigCluster.Ch1Enable?"=w1517:bool, "SysConfigCluster.Ch2Enable?"=w1516:bool, "SysConfigCluster.Ch3Enable?"=w1514:bool, "FLImDAQ"=w1511:T30)
        n695 = Unbundle By Name(w1500) -> ("Digitizer 1"=w1503:refnum<k15>, "Digitizer 2"=w1502:refnum<k15>)
        n696 = property on="Digitizer" class="Bool (strict)"(error in=w1504, "Blinking"=TRUE) -> (error out=w1505:errorcluster)  [unwired: 1 in, 1 out]
        n697 = Or(x=w1517, y=w1516) -> (x .or. y?=w1515:bool)
        n698 = case shown="True" w1515 {
          tunnel: w1511 -> [_ w1530]
          tunnel: w1505 -> [w1526 w1529]
          tunnel: [w1526 w1528] -> w1512
          tunnel: w1503 -> [_ w1527]
          frame False {
          }
          frame True {
            n699 = call "DigitizerConfig.vi"("error in (no error)"=w1529, "FLImDAQ"=w1530, "IVI Refnum in"=w1527) -> ("error out"=w1528:errorcluster)  [unwired: 7 in, 1 out]
          }
        }
        n700 = case shown="True" w1514 {
          tunnel: w1511 -> [_ w1525]
          tunnel: w1512 -> [w1520 w1524]
          tunnel: [w1520 w1523] -> w1488
          tunnel: w1502 -> [_ w1521]
          frame False {
          }
          frame True {
            n701 = call "DigitizerConfig.vi"("Config Trigger? (T)"=FALSE ("Config Trigge(T)r:"), "error in (no error)"=w1524, "FLImDAQ"=w1525, "IVI Refnum in"=w1521) -> ("error out"=w1523:errorcluster)  [unwired: 6 in, 1 out]
          }
        }
        n702 = call "Digitizer1_FGV.vi"("error in (no error)"=w1488) -> ("error out"=w1498:errorcluster, "Read data"=w1499:refnum<k15>)  [unwired: 9 in]
        n703 = call <instrlib>:"niScope Get Session Reference.vi"("instrument handle"=w1499, "error in"=w1498) -> ("session reference"=w1492:refnum<k20>, "error out"=w1490:errorcluster)  [unwired: 11 in, 1 out]
        n704 = call "Digitizer2_FGV.vi"("error in (no error)"=w1490) -> ("error out"=w1496:errorcluster, "Read data"=w1497:refnum<k15>)  [unwired: 9 in]
        n705 = call <instrlib>:"niScope Get Session Reference.vi"("instrument handle"=w1497, "error in"=w1496) -> ("session reference"=w1491:refnum<k20>, "error out"=w1489:errorcluster)  [unwired: 11 in, 1 out]
        n706 = Build Array(w1492, w1491) -> (w1495:refnum<k20>[])
        n707 = call <instrlib>:"niTClk Configure For Homogeneous Triggers.vi"("error in (no error)"=w1489, "sessions"=w1495) -> ("error out"=w1494:errorcluster, "sessions out"=w1493:refnum<k20>[])  [unwired: 8 in]
        n708 = call <instrlib>:"niTClk Synchronize.vi"("error in (no error)"=w1494, "sessions"=w1493) -> ("error out"=w1487:errorcluster, "sessions out"=w1485:refnum<k20>[])  [unwired: 8 in]
        n709 = call <userlib>:"Wait (ms)__ogtk.vi"("error in (no error)"=w1487, "milliseconds to wait"=u32 1500) -> ("error out"=w1483:errorcluster)  [unwired: 8 in, 1 out]
        n710 = Unbundle By Name(w1483) -> ("status"=w1508:bool)
        n711 = Not(x=w1508) -> (.not. x?=w1507:bool)
        n712 = Bundle By Name(cluster=w1509, "System Status.Digitizer"=w1507, "niTClk sessions"=w1485) -> (w1510:T23)
        n713 = property on="Digitizer" class="Bool (strict)"(error in=w1483, "Blinking"=FALSE) -> (error out=w1501:errorcluster)  [unwired: 1 in, 1 out]
        n714 = call <vilib>:"Add State(s) to Queue__JKI_lib_State_Machine.vi"("State(s) in (\"\")"=w1519) -> ("States Out"=w1518:string)  [unwired: 14 in]
      }
      frame "Digitizer: Start" {
        # "send trigger to start acquisition loop"
        # "initilize aquisition"
        # "Start Digitizer\n(TClk start)"
        n715 = Unbundle By Name(w1538) -> ("niTClk sessions"=w1537:refnum<k20>[])
        n716 = call <instrlib>:"niTClk Initiate.vi"("error in (no error)"=w1531, "sessions"=w1537) -> ("error out"=w1533:errorcluster)  [unwired: 8 in, 1 out]
        n717 = Generate User Event(priority (normal)=usereventprio."high priority", user event=w1534, event data cluster=TRUE ("event data"), error in=w1533) -> (error out=w1532:errorcluster)  [unwired: 1 out]
        n718 = call <vilib>:"Add State(s) to Queue__JKI_lib_State_Machine.vi"("State(s) in (\"\")"=w1541) -> ("States Out"=w1540:string)  [unwired: 14 in]
      }
      frame "Digitizer: Abort" {
        # "Template Separator\n(You can make a copy of, or modify, this frame)"
        n719 = call "Digitizer1_FGV.vi"("error in (no error)"=w1545, "Operation (Read)"=enum16{"Write", "Read"}."Read" ("Operation")) -> ("error out"=w1552:errorcluster, "Read data"=w1549:refnum<k15>)  [unwired: 8 in]
        n720 = call "Digitizer2_FGV.vi"("error in (no error)"=w1545, "Operation (Read)"=enum16{"Write", "Read"}."Read" ("Operation")) -> ("error out"=w1548:errorcluster, "Read data"=w1550:refnum<k15>)  [unwired: 8 in]
        n721 = Bundle By Name(cluster=w1542, "SysRunning?"=FALSE ("System Status")) -> (w1543:T23)
        n722 = call <instrlib>:"niScope Abort.vi"("instrument handle"=w1549, "error in"=w1552) -> ("error out"=w1554:errorcluster)  [unwired: 12 in, 1 out]
        n723 = call <instrlib>:"niScope Abort.vi"("instrument handle"=w1550, "error in"=w1548) -> ("error out"=w1553:errorcluster)  [unwired: 12 in, 1 out]
        n724 = Merge Errors(w1554, w1553) -> (w1546:errorcluster)
        n725 = call <vilib>:"Add State(s) to Queue__JKI_lib_State_Machine.vi"("State(s) in (\"\")"=w1557) -> ("States Out"=w1556:string)  [unwired: 14 in]
      }
      frame "Digitizer: checkTemp" {
        w1560 = 65.0 ("y")
        w1565 = enum16{"Write", "Read"}."Read" ("Operation")
        # "Template Separator\n(You can make a copy of, or modify, this frame)"
        n726 = call "Digitizer1_FGV.vi"("Operation (Read)"=w1565) -> ("error out"=w1566:errorcluster, "Read data"=w1567:refnum<k15>)  [unwired: 9 in]
        n727 = call "Digitizer2_FGV.vi"("Operation (Read)"=w1565) -> ("error out"=w1563:errorcluster, "Read data"=w1564:refnum<k15>)  [unwired: 9 in]
        n728 = property on="Property Node" class="niScope"(reference=w1564, error in=w1563) -> ("Device Temperature"=w1561:dbl)  [unwired: 2 out]
        "Dig2 Temp" <- w1561
        n729 = property on="Property Node" class="niScope"(reference=w1567, error in=w1566) -> ("Device Temperature"=w1562:dbl)  [unwired: 2 out]
        "Dig1 Temp" <- w1562
        n730 = Greater?(x=w1562, y=w1560) -> (0:w1559:bool)
        n731 = Greater?(x=w1561, y=w1560) -> (0:w1558:bool)
        n732 = case shown="True" w1559 {
          frame False {
          }
          frame True {
            n733 = One Button Dialog(message="Digitizer 1 over heating!", button name ("OK")="OK") -> ()  [unwired: 1 out]
          }
        }
        n734 = case shown="True" w1558 {
          frame False {
          }
          frame True {
            n735 = One Button Dialog(message="Digitizer 2 over heating!", button name ("OK")="OK") -> ()  [unwired: 1 out]
          }
        }
        n736 = call <vilib>:"Add State(s) to Queue__JKI_lib_State_Machine.vi"("State(s) in (\"\")"=w1572) -> ("States Out"=w1571:string)  [unwired: 14 in]
      }
      frame "Digitizer: Close" {
        # "Close Digitizer"
        n737 = call "Digitizer1_FGV.vi"("error in (no error)"=w1582, "Operation (Read)"=enum16{"Write", "Read"}."Read" ("Operation")) -> ("error out"=w1584:errorcluster, "Read data"=w1588:refnum<k15>)  [unwired: 8 in]
        n738 = call "Digitizer2_FGV.vi"("error in (no error)"=w1582, "Operation (Read)"=enum16{"Write", "Read"}."Read" ("Operation")) -> ("error out"=w1583:errorcluster, "Read data"=w1586:refnum<k15>)  [unwired: 8 in]
        n739 = call <instrlib>:"niScope Close.vi"("instrument handle"=w1588, "error in"=w1584) -> ("error out"=w1581:errorcluster)  [unwired: 13 in]
        n740 = call <instrlib>:"niScope Close.vi"("instrument handle"=w1586, "error in"=w1583) -> ("error out"=w1580:errorcluster)  [unwired: 13 in]
        n741 = Merge Errors(w1581, w1580) -> (w1579:errorcluster)
        n742 = Unbundle By Name(w1579) -> ("status"=w1578:bool)
        n743 = Bundle By Name(cluster=w1589, "System Status.Digitizer"=w1578) -> (w1590:T23)
        n744 = call <vilib>:"Add State(s) to Queue__JKI_lib_State_Machine.vi"("State(s) in (\"\")"=w1592) -> ("States Out"=w1591:string)  [unwired: 14 in]
      }
      frame "---------- LabJack ----------" {
        # "Template Separator\n(You can make a copy of, or modify, this frame)"
        n745 = call <vilib>:"Add State(s) to Queue__JKI_lib_State_Machine.vi"("State(s) in (\"\")"=w1597) -> ("States Out"=w1596:string)  [unwired: 14 in]
      }
      frame "LabJack: checkPedal" {
        # "Template Separator\n(You can make a copy of, or modify, this frame)"
        n746 = Unbundle By Name(w1598) -> ("LJ Pinout.Foot Pedal"=w1602:string)
        n747 = call "LabJack_FGV.vi"("Operation(Read)"=enum16{"Write", "Read"}."Read" ("Operation"), "error in (no error)"=w1600) -> ("error out"=w1604:errorcluster, "Read data"=w1605:i32)  [unwired: 8 in]
        n748 = call "LJM_eReadName.vi"("Handle In"=w1605, "Name"=w1602, "error in"=w1604) -> ("Value"=w1603:dbl, "error out"=w1601:errorcluster)  [unwired: 10 in, 1 out]
        n749 = case shown="1" w1603 {
          tunnel: w1598 -> [w1610 w1613]
          tunnel: [w1610 w1611] -> w1599
          frame 0, Default {
          }
          frame 1 {
            # "If Pedal pressed"
            n750 = Tick Count (ms)() -> (millisecond timer value=w1617:u32)
            n751 = Unbundle By Name(w1613) -> ("Last Trigger"=w1612:u32)
            n752 = Subtract(x=w1617, y=w1612) -> (x-y=w1616:u32)
            n753 = Greater Or Equal?(x=w1616, y=u32 2000) -> (x >= y?=w1614:bool)
            n754 = case shown="True" w1614 {
              tunnel: w1613 -> [w1618 w1619]
              tunnel: w1612 -> [_ _]
              tunnel: [w1618 w1620] -> w1611
              frame False {
              }
              frame True {
                n755 = Tick Count (ms)() -> (millisecond timer value=w1621:u32)
                n756 = Unbundle By Name(w1619) -> ("SysRunning?"=w1622:bool)
                n757 = case shown="False" w1622 {
                  frame False {
                    n758 = property on="StartButton" class="Bool (strict)"("Val(Sgnl)"=TRUE ("Value (Signaling)")) -> ()  [unwired: 2 in, 2 out]
                  }
                  frame True {
                    n759 = property on="StopButton" class="Bool (strict)"("Val(Sgnl)"=TRUE ("Value (Signaling)")) -> ()  [unwired: 2 in, 2 out]
                  }
                }
                n760 = Bundle By Name(cluster=w1619, "Last Trigger"=w1621) -> (w1620:T23)
              }
            }
          }
        }
        n761 = call <vilib>:"Add State(s) to Queue__JKI_lib_State_Machine.vi"("State(s) in (\"\")"=w1609) -> ("States Out"=w1608:string)  [unwired: 14 in]
      }
      frame "LabJack: ZeroV" {
        # "Just Zero V\nDO not update FGV and front panel\nWIll resume from last V"
        # "set bias to 0"
        # "Zero APD bias\n(You can make a copy of, or modify, this frame)"
        n762 = Unbundle By Name(w1627) -> ("LJ Pinout.Ch1 Bias"=w1632:string, "LJ Pinout.Ch2 Bias"=w1631:string, "LJ Pinout.Ch3 Bias"=w1630:string)
        n763 = Build Array(w1632, w1631, w1630) -> (w1629:string[])
        n764 = call "LabJack_FGV.vi"("Operation(Read)"=enum16{"Write", "Read"}."Read" ("Operation"), "error in (no error)"=w1626) -> ("error out"=w1633:errorcluster, "Read data"=w1634:i32)  [unwired: 8 in]
        n765 = call "LJM_eWriteNames.vi"("Handle In"=w1634, "aNames"=w1629, "aValuesIn"=dbl[] [0.0, 0.0, 0.0], "error in"=w1633) -> ("error out"=w1625:errorcluster)  [unwired: 9 in, 2 out]
        n766 = call <vilib>:"Add State(s) to Queue__JKI_lib_State_Machine.vi"("State(s) in (\"\")"=w1638) -> ("States Out"=w1637:string)  [unwired: 14 in]
      }
      frame "LabJack: SetV" {
        w1645 = enum16{"write", "read"}."read" ("action (write)")
        # "set bias to user specifid"
        # "Set APD bias\n(You can make a copy of, or modify, this frame)"
        n767 = Unbundle By Name(w1654) -> ("LJ Pinout.Ch1 Bias"=w1658:string, "LJ Pinout.Ch2 Bias"=w1657:string, "LJ Pinout.Ch3 Bias"=w1656:string, "LJ Pinout.Ch4 Bias"=w1648:string)
        n768 = call "V2FGV.vi"("Error In"=w1644, "action(write)"=w1645) -> ("Error Out"=w1642:errorcluster, "V2 out"=w1650:dbl)  [unwired: 8 in]
        n769 = call "V4FGV.vi"("Error In"=w1644, "action(write)"=w1645) -> ("Error Out"=w1640:errorcluster, "V3 out"=w1646:dbl)  [unwired: 8 in]
        n770 = call "V1FGV.vi"("Error In"=w1644, "action (write)"=w1645) -> ("Error Out"=w1643:errorcluster, "V1 out"=w1647:dbl)  [unwired: 8 in]
        n771 = call "V3FGV.vi"("Error In"=w1644, "action(write)"=w1645) -> ("Error Out"=w1641:errorcluster, "V3 out"=w1649:dbl)  [unwired: 8 in]
        n772 = local write "V 3"(w1649) -> ()
        n773 = local write "V 2"(w1650) -> ()
        n774 = local write "V 4"(w1646) -> ()
        n775 = local write "V 1"(w1647) -> ()
        n776 = Build Array(w1658, w1657, w1656, w1648) -> (w1655:string[])
        n777 = call "LabJack_FGV.vi"("Operation(Read)"=enum16{"Write", "Read"}."Read" ("Operation"), "error in (no error)"=w1644) -> ("error out"=w1659:errorcluster, "Read data"=w1660:i32)  [unwired: 8 in]
        n778 = Build Array(w1647, w1650, w1649, w1646) -> (w1651:dbl[])
        n779 = call "LJM_eWriteNames.vi"("Handle In"=w1660, "aNames"=w1655, "aValuesIn"=w1651, "error in"=w1659) -> ("error out"=w1652:errorcluster)  [unwired: 9 in, 2 out]
        n780 = Merge Errors(w1643, w1642, w1641, w1640) -> (w1639:errorcluster)
        n781 = call <vilib>:"Add State(s) to Queue__JKI_lib_State_Machine.vi"("State(s) in (\"\")"=w1664) -> ("States Out"=w1663:string)  [unwired: 14 in]
        n782 = Merge Errors(w1639, w1652) -> (w1653:errorcluster)
      }
      frame "LabJack: Open" {
        # "Initialize LabJack T7\nEstablish connection and initialize pins"
        n783 = call "LJ_Open.vi"("error in"=w1674, "DeviceType"="LJM_dtT7") -> ("error out"=w1671:errorcluster, "Success?"=w1672:bool, "Handle Out"=w1666:i32)  [unwired: 7 in]
        n784 = call "LabJack_FGV.vi"("Operation(Read)"=enum16{"Write", "Read"}."Write" ("Operation"), "error in (no error)"=w1671, "Write data"=w1666) -> ("error out"=w1668:errorcluster)  [unwired: 7 in, 1 out]
        n785 = Bundle By Name(cluster=w1669, "System Status.Labjack"=w1672) -> (w1673:T23)
        n786 = call <vilib>:"Add State(s) to Queue__JKI_lib_State_Machine.vi"("State(s) in (\"\")"=w1676) -> ("States Out"=w1675:string)  [unwired: 14 in]
      }
      frame "LabJack: SetDefaultSub" {
        w1686 = enum16{"write", "read"}."write" ("action")
        w1687 = 0.0 ("V1 in")
        w1700 = "_EF_ENABLE" ("string")
        # "1. Disable PWM\n2. Set all V to 0\n3. Set 355 relay to open\n4. Set LED to off"
        # "read once to set DIO to input"
        # "set all initila V to 0. Set footpedal to input. Set PWM to low. Set laser relay to open. Set LEDs to yellow."
        # "Set Labjack to correct input and output state and initial values"
        n787 = disable-structure shown="Disabled" {
          frame Disabled {
            (unwired) dbl[] [0.0, 0.0, 0.0, 0.0, 0.0, 0.0, 0.0, 0.0, 0.0] ("aValuesIn")
          }
          frame Enabled {
          }
        }
        n788 = Unbundle By Name(w1697) -> ("LJ Pinout.355 PWM"=w1702:string, "LJ Pinout.AimingBeam PWM"=w1701:string, "LJ Pinout.Ch1 Bias"=w1707:string, "LJ Pinout.Ch2 Bias"=w1677:string, "LJ Pinout.Ch3 Bias"=w1711:string, "LJ Pinout.Ch4 Bias"=w1691:string, "LJ Pinout.Laser Start/Stop"=w1710:string, "LJ Pinout.Red LED"=w1709:string, "LJ Pinout.Green LED"=w1708:string)
        n789 = call "V1FGV.vi"("Error In"=w1695, "action (write)"=w1686, "V1 in"=w1687) -> ("Error Out"=w1690:errorcluster, "V1 out"=w1694:dbl)  [unwired: 7 in]
        n790 = local write "V 1"(w1694) -> ()
        n791 = call "V2FGV.vi"("Error In"=w1690, "action(write)"=w1686, "V2 in"=w1687) -> ("Error Out"=w1689:errorcluster, "V2 out"=w1693:dbl)  [unwired: 7 in]
        n792 = call "LabJack_FGV.vi"("Operation(Read)"=enum16{"Write", "Read"}."Read" ("Operation"), "error in (no error)"=w1695) -> ("error out"=w1683:errorcluster, "Read data"=w1705:i32)  [unwired: 8 in]
        n793 = Concatenate Strings(w1702, w1700) -> (w1699:string)
        n794 = Concatenate Strings(w1701, w1700) -> (w1698:string)
        n795 = local write "V 2"(w1693) -> ()
        n796 = call "V3FGV.vi"("Error In"=w1689, "action(write)"=w1686, "V3 in"=w1687) -> ("Error Out"=w1688:errorcluster, "V3 out"=w1692:dbl)  [unwired: 7 in]
        n797 = Build Array(w1699, w1698, w1707, w1677, w1711, w1691, w1710, w1709, w1708) -> (w1681:string[])
        n798 = local write "V 3"(w1692) -> ()
        n799 = call "V4FGV.vi"("Error In"=w1688, "action(write)"=w1686, "V3 in"=w1687) -> ("Error Out"=w1684:errorcluster, "V3 out"=w1685:dbl)  [unwired: 7 in]
        n800 = Array Size(array=w1681) -> (size(s)=w1680:i32)
        n801 = local write "V 4"(w1685) -> ()
        n802 = Initialize Array(0.0 ("element"), w1680) -> (w1678:dbl[])
        n803 = Unbundle By Name(w1697) -> ("LJ Pinout.Foot Pedal"=w1696:string)
        n804 = call "LJM_eWriteNames.vi"("Handle In"=w1705, "aNames"=w1681, "aValuesIn"=w1678, "error in"=w1683) -> ("Handle Out"=w1704:i32, "error out"=w1703:errorcluster)  [unwired: 9 in, 1 out]
        n805 = call "LJM_eReadName.vi"("Handle In"=w1704, "Name"=w1696, "error in"=w1703) -> ("error out"=w1682:errorcluster)  [unwired: 10 in, 2 out]
        n806 = case shown="Error .." w1682 {
          frame No Error {
            # "no error"
          }
          frame Error {
            # "handle error"
            n807 = One Button Dialog(message="Labjack error! The pin assignment is likely wrong. Please check pin setting of Labjack. Program will terminate.", button name ("OK")="OK") -> ()  [unwired: 1 out]
          }
        }
        n808 = call <vilib>:"Add State(s) to Queue__JKI_lib_State_Machine.vi"("State(s) in (\"\")"=w1714) -> ("States Out"=w1713:string)  [unwired: 14 in]
      }
      frame "LabJack: FootPedalConfig" {
        # "Setup footPedal\n(You can make a copy of, or modify, this frame)"
        n809 = call "LabJack_FGV.vi"("Operation(Read)"=enum16{"Write", "Read"}."Read" ("Operation"), "error in (no error)"=w1718) -> ("error out"=w1722:errorcluster, "Read data"=w1723:i32)  [unwired: 8 in]
        n810 = call "LJM_eWriteName.vi"("Handle In"=w1723, "Name"="DIO15", "Value"=1.0, "error in"=w1722) -> ("error out"=w1719:errorcluster)  [unwired: 10 in, 1 out]
        n811 = call <vilib>:"Add State(s) to Queue__JKI_lib_State_Machine.vi"("State(s) in (\"\")"=w1727) -> ("States Out"=w1726:string)  [unwired: 14 in]
      }
      frame "LabJack: SetDefaultAndClose" {
        # "Template Separator\n(You can make a copy of, or modify, this frame)"
        n812 = call <vilib>:"Add State(s) to Queue__JKI_lib_State_Machine.vi"("State(s) in Front (\"\")"="LabJack: SetDefaultSub\nLabJack: Close" ("State(s) in Front (\"\")"), "State(s) in (\"\")"=w1733) -> ("States Out"=w1732:string)  [unwired: 13 in]
      }
      frame "LabJack: Close" {
        # "Close LabJack Refnum"
        n813 = call "LabJack_FGV.vi"("Operation(Read)"=enum16{"Write", "Read"}."Read" ("Operation"), "error in (no error)"=w1739) -> ("error out"=w1734:errorcluster, "Read data"=w1735:i32)  [unwired: 8 in]
        n814 = Bundle By Name(cluster=w1737, "System Status.Labjack"=FALSE ("System Status.Gain Control")) -> (w1740:T23)
        n815 = call "LJM_Close.vi"("error in"=w1734, "Handle"=w1735) -> ("error out"=w1742:errorcluster)  [unwired: 9 in]
        n816 = call <vilib>:"Add State(s) to Queue__JKI_lib_State_Machine.vi"("State(s) in (\"\")"=w1744) -> ("States Out"=w1743:string)  [unwired: 14 in]
      }
      frame "LabJack: Interlock enable/disable" {
        w1753 = i8 0  # int8
        # "[Covers: REQ8]"
        # "Interlock enable/disable\n(Usage: \"LabJack: Interlock enable/disable >> 1|0\")"
        n817 = Fract/Exp String To Number(string=w1754, default (0 dbl)=w1753) -> (number=w1750:i8)  [unwired: 2 in, 1 out]
        n818 = Unbundle By Name(w1752) -> ("LJ Pinout.Interlock"=w1751:string)
        n819 = call "LabJack_FGV.vi"("Operation(Read)"=enum16{"Write", "Read"}."Read" ("Operation")) -> ("Read data"=w1748:i32)  [unwired: 9 in, 1 out]
        n820 = call "LJM_eWriteName.vi"("Handle In"=w1748, "Name"=w1751, "Value"=w1750, "error in"=w1749) -> ("error out"=w1746:errorcluster)  [unwired: 10 in, 1 out]
        n821 = call <vilib>:"Add State(s) to Queue__JKI_lib_State_Machine.vi"("State(s) in (\"\")"=w1756) -> ("States Out"=w1755:string)  [unwired: 14 in]
      }
      frame "LabJack: 355_PWM_Config" {
        w1758 = 0.0 ("element")
        w1778 = "DIO_EF_CLOCK1_ENABLE"
        # "Config PWM frequency"
        n822 = Unbundle By Name(w1770) -> ("LJ Pinout.355 PWM"=w1777:string)
        n823 = Unbundle By Name(w1770) -> ("355 PWM setting.DIO_EF_CLOCK1_DIVISOR"=w1769:i16, "355 PWM setting.DIO_EF_CLOCK1_ROLL_VALUE"=w1768:i32, "355 PWM setting.DIO#_EF_INDEX"=w1765:i16, "355 PWM setting.DIO#_EF_OPTIONS"=w1764:i16, "355 PWM setting.DIO#_EF_CONFIG_A"=w1763:i32)
        n824 = Concatenate Strings(w1777, "_EF_ENABLE" ("string")) -> (w1773:string)
        n825 = Concatenate Strings(w1777, "_EF_INDEX") -> (w1776:string)
        n826 = Concatenate Strings(w1777, "_EF_OPTIONS") -> (w1775:string)
        n827 = Concatenate Strings(w1777, "_EF_CONFIG_A") -> (w1774:string)
        n828 = call "LabJack_FGV.vi"("Operation(Read)"=enum16{"Write", "Read"}."Read" ("Operation")) -> ("Read data"=w1771:i32)  [unwired: 9 in, 1 out]
        n829 = Build Array(w1758, w1758, w1769, w1768, 1.0 ("element"), 0.0 ("element"), w1765, w1764, w1763) -> (w1762:dbl[])
        n830 = Build Array("DIO_EF_CLOCK0_ENABLE", w1778, "DIO_EF_CLOCK1_DIVISOR", "DIO_EF_CLOCK1_ROLL_VALUE", w1778, w1773, w1776, w1775, w1774) -> (w1772:string[])
        n831 = call "LJM_eWriteNames.vi"("Handle In"=w1771, "aNames"=w1772, "aValuesIn"=w1762, "error in"=w1760) -> ("error out"=w1761:errorcluster)  [unwired: 9 in, 2 out]
        n832 = call <vilib>:"Add State(s) to Queue__JKI_lib_State_Machine.vi"("State(s) in (\"\")"=w1787) -> ("States Out"=w1786:string)  [unwired: 14 in]
      }
      frame "LabJack: 355_PWM_Start" {
        # "Template Separator\n(You can make a copy of, or modify, this frame)"
        n833 = Unbundle By Name(w1795) -> ("LJ Pinout.355 PWM"=w1794:string)
        n834 = call "LabJack_FGV.vi"("Operation(Read)"=enum16{"Write", "Read"}."Read" ("Operation"), "error in (no error)"=w1789) -> ("error out"=w1796:errorcluster, "Read data"=w1797:i32)  [unwired: 8 in]
        n835 = Concatenate Strings(w1794, "_EF_ENABLE" ("string")) -> (w1792:string)
        n836 = call "LJM_eWriteName.vi"("Handle In"=w1797, "Name"=w1792, "Value"=1.0, "error in"=w1796) -> ("error out"=w1790:errorcluster)  [unwired: 10 in, 1 out]
        n837 = call <vilib>:"Add State(s) to Queue__JKI_lib_State_Machine.vi"("State(s) in (\"\")"=w1800) -> ("States Out"=w1799:string)  [unwired: 14 in]
      }
      frame "LabJack: 355_PWM_Stop" {
        # "Template Separator\n(You can make a copy of, or modify, this frame)"
        n838 = Unbundle By Name(w1806) -> ("LJ Pinout.355 PWM"=w1810:string)
        n839 = call "LabJack_FGV.vi"("Operation(Read)"=enum16{"Write", "Read"}."Read" ("Operation"), "error in (no error)"=w1805) -> ("error out"=w1811:errorcluster, "Read data"=w1803:i32)  [unwired: 8 in]
        n840 = Concatenate Strings(w1810, "_EF_ENABLE" ("string")) -> (w1808:string)
        n841 = call "LJM_eWriteName.vi"("Handle In"=w1803, "Name"=w1808, "Value"=0.0, "error in"=w1811) -> ("error out"=w1802:errorcluster)  [unwired: 10 in, 1 out]
        n842 = local write "355nm Laser toggle"(FALSE ("355nm Laser toggle")) -> ()
        n843 = call <vilib>:"Add State(s) to Queue__JKI_lib_State_Machine.vi"("State(s) in (\"\")"=w1814) -> ("States Out"=w1813:string)  [unwired: 14 in]
      }
      frame "LabJack: AB_Start" {
        # "Aiming Beam Start\n(Based on aimging beam frequency, set LabJack pin)"
        n844 = Unbundle By Name(w1824) -> ("AB Cluster.Freq"=w1816:i32, "LJ Pinout.AimingBeam PWM"=w1823:string)
        n845 = Greater Than 0?(x=w1816) -> (x > 0?=w1815:bool)
        n846 = case shown="False" w1815 {
          tunnel: w1823 -> [w1830 w1833]
          tunnel: [w1830 w1831] -> w1822
          frame False {
            # "if 0 freq, set PWM pin"
          }
          frame True {
            # "if non zero freq, set PWM enable"
            n847 = Concatenate Strings(w1833, "_EF_ENABLE" ("string")) -> (w1831:string)
          }
        }
        n848 = call "LabJack_FGV.vi"("Operation(Read)"=enum16{"Write", "Read"}."Read" ("Operation"), "error in (no error)"=w1819) -> ("error out"=w1825:errorcluster, "Read data"=w1826:i32)  [unwired: 8 in]
        n849 = call "LJM_eWriteName.vi"("Handle In"=w1826, "Name"=w1822, "Value"=1.0, "error in"=w1825) -> ("error out"=w1820:errorcluster)  [unwired: 10 in, 1 out]
        n850 = local write "Aiming beam toggle"(TRUE ("Aiming beam toggle")) -> ()
        n851 = call <vilib>:"Add State(s) to Queue__JKI_lib_State_Machine.vi"("State(s) in (\"\")"=w1829) -> ("States Out"=w1828:string)  [unwired: 14 in]
      }
      frame "LabJack: AB_Stop" {
        # "Aiming Beam Stop\n(Based on aiming beam frequency, set LabJack pin low)"
        n852 = Unbundle By Name(w1841) -> ("AB Cluster.Freq"=w1836:i32, "LJ Pinout.AimingBeam PWM"=w1843:string)
        n853 = Greater Than 0?(x=w1836) -> (x > 0?=w1835:bool)
        n854 = case shown="False" w1835 {
          tunnel: w1843 -> [w1849 w1852]
          tunnel: [w1849 w1850] -> w1834
          frame False {
          }
          frame True {
            n855 = Concatenate Strings(w1852, "_EF_ENABLE" ("string")) -> (w1850:string)
          }
        }
        n856 = call "LabJack_FGV.vi"("Operation(Read)"=enum16{"Write", "Read"}."Read" ("Operation"), "error in (no error)"=w1839) -> ("error out"=w1844:errorcluster, "Read data"=w1845:i32)  [unwired: 8 in]
        n857 = call "LJM_eWriteName.vi"("Handle In"=w1845, "Name"=w1834, "Value"=0.0, "error in"=w1844) -> ("error out"=w1840:errorcluster)  [unwired: 10 in, 1 out]
        n858 = local write "Aiming beam toggle"(FALSE ("Aiming beam toggle")) -> ()
        n859 = call <vilib>:"Add State(s) to Queue__JKI_lib_State_Machine.vi"("State(s) in (\"\")"=w1848) -> ("States Out"=w1847:string)  [unwired: 14 in]
      }
      frame "LabJack: AB_PWM_Config" {
        w1854 = 0.0 ("element")
        w1874 = "DIO_EF_CLOCK2_ENABLE"
        # "Config PWM frequency"
        n860 = Unbundle By Name(w1866) -> ("LJ Pinout.AimingBeam PWM"=w1873:string)
        n861 = Unbundle By Name(w1866) -> ("AB PWM setting.DIO_EF_CLOCK1_DIVISOR"=w1865:i16, "AB PWM setting.DIO_EF_CLOCK1_ROLL_VALUE"=w1864:i32, "AB PWM setting.DIO#_EF_INDEX"=w1861:i16, "AB PWM setting.DIO#_EF_OPTIONS"=w1860:i16, "AB PWM setting.DIO#_EF_CONFIG_A"=w1859:i32)
        n862 = Concatenate Strings(w1873, "_EF_ENABLE" ("string")) -> (w1869:string)
        n863 = Concatenate Strings(w1873, "_EF_INDEX") -> (w1872:string)
        n864 = Concatenate Strings(w1873, "_EF_OPTIONS") -> (w1871:string)
        n865 = Concatenate Strings(w1873, "_EF_CONFIG_A") -> (w1870:string)
        n866 = call "LabJack_FGV.vi"("Operation(Read)"=enum16{"Write", "Read"}."Read" ("Operation")) -> ("Read data"=w1867:i32)  [unwired: 9 in, 1 out]
        n867 = Build Array(w1854, w1854, w1865, w1864, 1.0 ("element"), 0.0 ("element"), w1861, w1860, w1859) -> (w1858:dbl[])
        n868 = Build Array("DIO_EF_CLOCK0_ENABLE", w1874, "DIO_EF_CLOCK2_DIVISOR", "DIO_EF_CLOCK2_ROLL_VALUE", w1874, w1869, w1872, w1871, w1870) -> (w1868:string[])
        n869 = call "LJM_eWriteNames.vi"("Handle In"=w1867, "aNames"=w1868, "aValuesIn"=w1858, "error in"=w1856) -> ("error out"=w1857:errorcluster)  [unwired: 9 in, 2 out]
        n870 = call <vilib>:"Add State(s) to Queue__JKI_lib_State_Machine.vi"("State(s) in (\"\")"=w1883) -> ("States Out"=w1882:string)  [unwired: 14 in]
      }
      frame "---------- LED ----------" {
        # "Template Separator\n(You can make a copy of, or modify, this frame)"
        n871 = call <vilib>:"Add State(s) to Queue__JKI_lib_State_Machine.vi"("State(s) in (\"\")"=w1888) -> ("States Out"=w1887:string)  [unwired: 14 in]
      }
      frame "LED: OpenVIRef" {
        # "Template Separator\n(You can make a copy of, or modify, this frame)"
        n872 = call <vilib>:"Application Directory.vi"() -> ("Application Directory"=w1895:path)
        n873 = Build Path(base path=w1895, name or relative path="SubVI") -> (appended path=w1893:path)
        n874 = Build Path(base path=w1893, name or relative path="LEDBreath.vi") -> (appended path=w1891:path)
        n875 = Open VI Reference(vi path=w1891, error in (no error)=w1896) -> (vi reference=w1897:refnum<vi>, error out=w1890:errorcluster)  [unwired: 4 in]
        n876 = case shown="Error .." w1890 {
          tunnel: [TRUE FALSE] -> w1889
          frame No Error {
          }
          frame Error {
          }
        }
        n877 = Bundle By Name(cluster=w1898, "LED vi reference"=w1897, "LED vi ref open?"=w1889) -> (w1899:T23)
        n878 = call <vilib>:"Add State(s) to Queue__JKI_lib_State_Machine.vi"("State(s) in (\"\")"=w1902) -> ("States Out"=w1901:string)  [unwired: 14 in]
      }
      frame "LED: CloseVIRef" {
        # "Template Separator\n(You can make a copy of, or modify, this frame)"
        n879 = Unbundle By Name(w1906) -> ("LED vi reference"=w1907:refnum<vi>, "LED vi ref open?"=w1905:bool)
        n880 = case shown="True" w1905 {
          tunnel: w1909 -> [w1913 w1916]
          tunnel: [w1913 w1915] -> w1908
          tunnel: w1907 -> [_ w1914]
          frame False {
          }
          frame True {
            n881 = Close Reference(reference=w1914, error in (no error)=w1916) -> (error out=w1915:errorcluster)
          }
        }
        n882 = call <vilib>:"Add State(s) to Queue__JKI_lib_State_Machine.vi"("State(s) in (\"\")"=w1912) -> ("States Out"=w1911:string)  [unwired: 14 in]
      }
      frame "LED: BreathGreen" {
        w1917 = FALSE ("Wait Until Done")
        # "Breath system LED\n(LED: Breath >> True/False)"
        n883 = Unbundle By Name(w1925) -> ("LED vi reference"=w1924:refnum<vi>)
        n884 = invoke class="VI" method="Ctrl Val.Set"(reference=w1924, error in=w1922, "Control Name"="Color", "Value"=0) -> (reference out=w1921:refnum<vi>, error out=w1920:errorcluster)  [unwired: 1 in, 3 out]
        n885 = invoke on="Invoke Node" class="VI" method="Run VI"(reference=w1921, error in=w1920, "Wait until done"=w1917, "Auto Dispose Ref"=w1917) -> (error out=w1923:errorcluster)  [unwired: 1 in, 4 out]
        n886 = call <vilib>:"Add State(s) to Queue__JKI_lib_State_Machine.vi"("State(s) in (\"\")"=w1928) -> ("States Out"=w1927:string)  [unwired: 14 in]
      }
      frame "LED: BreathOrange" {
        w1929 = FALSE ("Wait Until Done")
        # "Breath system LED\n(LED: Breath >> True/False)"
        n887 = Unbundle By Name(w1937) -> ("LED vi reference"=w1936:refnum<vi>)
        n888 = invoke class="VI" method="Ctrl Val.Set"(reference=w1936, error in=w1934, "Control Name"="Color", "Value"=1) -> (reference out=w1933:refnum<vi>, error out=w1932:errorcluster)  [unwired: 1 in, 3 out]
        n889 = invoke on="Invoke Node" class="VI" method="Run VI"(reference=w1933, error in=w1932, "Wait until done"=w1929, "Auto Dispose Ref"=w1929) -> (error out=w1935:errorcluster)  [unwired: 1 in, 4 out]
        n890 = call <vilib>:"Add State(s) to Queue__JKI_lib_State_Machine.vi"("State(s) in (\"\")"=w1940) -> ("States Out"=w1939:string)  [unwired: 14 in]
      }
      frame "LED: BreathOff" {
        # "System LED Breath Off\n(Breath off, check VI status to make sure it is off)"
        n891 = Unbundle By Name(w1949) -> ("LED vi reference"=w1948:refnum<vi>)
        n892 = invoke on="Invoke Node" class="VI" method="Ctrl Val.Set"(reference=w1948, error in=w1946, "Control Name"="Stop", "Value"=TRUE) -> (reference out=w1941:refnum<vi>, error out=w1942:errorcluster)  [unwired: 1 in, 3 out]
        n893 = case shown="No Error" w1942 {
          selector: w1942 -> [w1954 _]
          tunnel: [w1953 errorcluster {"status"=FALSE, "code"=0, "source"=""} ("error IO")] -> w1947
          tunnel: ["" ("State(s) in Front (\"\")") "LED: BreathOff" ("State(s) in Front (\"\")")] -> w1945
          tunnel: w1941 -> [w1955 _]
          frame No Error {
            # "No error, wait for VI to stop"
            n894 = while {
              tunnel: w1955 -> [w1963]
              shift-right: [w1957] -> w1953
              shift-left: w1954 -> [w1962]
              stop <- w1959 stop-if-true
              # "continue check whether vi is running"
              n895 = property class="VI"(reference=w1963, error in=w1962) -> (error out=w1957:errorcluster, "Exec.State"=w1961:T20)  [unwired: 1 out]
              n896 = Wait (ms)(milliseconds to wait=u32 50) -> ()  [unwired: 1 out]
              n897 = Equal?(x=w1961, y=T20."Idle") -> (x = y?=w1959:bool)
            }
          }
          frame Error {
            # "try again when error"
          }
        }
        n898 = call <vilib>:"Add State(s) to Queue__JKI_lib_State_Machine.vi"("State(s) in Front (\"\")"=w1945, "State(s) in (\"\")"=w1952) -> ("States Out"=w1951:string)  [unwired: 13 in]
      }
      frame "LED: Off" {
        # "set LED to red"
        # "Template Separator\n(You can make a copy of, or modify, this frame)"
        n899 = Unbundle By Name(w1968) -> ("LJ Pinout.Red LED"=w1967:string, "LJ Pinout.Green LED"=w1966:string)
        n900 = call "LabJack_FGV.vi"("Operation(Read)"=enum16{"Write", "Read"}."Read" ("Operation"), "error in (no error)"=w1969) -> ("error out"=w1976:errorcluster, "Read data"=w1975:i32)  [unwired: 8 in]
        n901 = call "LJM_eWriteName.vi"("Handle In"=w1975, "Name"=w1967, "Value"=0.0, "error in"=w1976) -> ("Handle Out"=w1973:i32, "error out"=w1972:errorcluster)  [unwired: 10 in]
        n902 = call "LJM_eWriteName.vi"("Handle In"=w1973, "Name"=w1966, "Value"=0.0, "error in"=w1972) -> ("error out"=w1970:errorcluster)  [unwired: 10 in, 1 out]
        n903 = call <vilib>:"Add State(s) to Queue__JKI_lib_State_Machine.vi"("State(s) in (\"\")"=w1980) -> ("States Out"=w1979:string)  [unwired: 14 in]
      }
      frame "LED: Green" {
        # "set LED to green"
        # "Template Separator\n(You can make a copy of, or modify, this frame)"
        n904 = Unbundle By Name(w1984) -> ("LJ Pinout.Red LED"=w1982:string, "LJ Pinout.Green LED"=w1983:string)
        n905 = call "LabJack_FGV.vi"("Operation(Read)"=enum16{"Write", "Read"}."Read" ("Operation"), "error in (no error)"=w1986) -> ("error out"=w1992:errorcluster, "Read data"=w1991:i32)  [unwired: 8 in]
        n906 = call "LJM_eWriteName.vi"("Handle In"=w1991, "Name"=w1982, "Value"=0.0, "error in"=w1992) -> ("Handle Out"=w1989:i32, "error out"=w1988:errorcluster)  [unwired: 10 in]
        n907 = call "LJM_eWriteName.vi"("Handle In"=w1989, "Name"=w1983, "Value"=9.0, "error in"=w1988) -> ("error out"=w1985:errorcluster)  [unwired: 10 in, 1 out]
        n908 = call <vilib>:"Add State(s) to Queue__JKI_lib_State_Machine.vi"("State(s) in (\"\")"=w1995) -> ("States Out"=w1994:string)  [unwired: 14 in]
      }
      frame "---------- Queue ----------" {
        # "Template Separator\n(You can make a copy of, or modify, this frame)"
        n909 = call <vilib>:"Add State(s) to Queue__JKI_lib_State_Machine.vi"("State(s) in (\"\")"=w2000) -> ("States Out"=w1999:string)  [unwired: 14 in]
      }
      frame "Queue: Flash" {
        # "Clear queue contnet\n(clear queue content by flash it)"
        n910 = Flush Queue(queue=w2007, error in (no error)=w2001) -> (error out=w2005:errorcluster)  [unwired: 2 out]
        n911 = Flush Queue(queue=w2008, error in (no error)=w2001) -> (error out=w2004:errorcluster)  [unwired: 2 out]
        n912 = Flush Queue(queue=w2006, error in (no error)=w2001) -> (error out=w2003:errorcluster)  [unwired: 2 out]
        n913 = Merge Errors(w2005, w2004, w2003) -> (w2002:errorcluster)
        n914 = call <vilib>:"Add State(s) to Queue__JKI_lib_State_Machine.vi"("State(s) in (\"\")"=w2012) -> ("States Out"=w2011:string)  [unwired: 14 in]
      }
      frame "Queue: Destory" {
        # "Destory Data Queue\nDistory data queue ref so the aquisition loop stop"
        n915 = Release Queue(queue=w2018, error in (no error)=w2014) -> (error out=w2021:errorcluster)  [unwired: 1 in, 2 out]
        n916 = Release Queue(queue=w2017, error in (no error)=w2014) -> (error out=w2020:errorcluster)  [unwired: 1 in, 2 out]
        n917 = Release Queue(queue=w2015, error in (no error)=w2014) -> (error out=w2013:errorcluster)  [unwired: 1 in, 2 out]
        n918 = Merge Errors(w2021, w2020, w2013) -> (w2019:errorcluster)
        n919 = call <vilib>:"Simple Error Handler.vi"("error in (no error)"=w2019) -> ()  [unwired: 4 in, 5 out]
        n920 = call <vilib>:"Add State(s) to Queue__JKI_lib_State_Machine.vi"("State(s) in (\"\")"=w2024) -> ("States Out"=w2023:string)  [unwired: 14 in]
      }
      frame "---------- Run ----------" {
        # "Template Separator\n(You can make a copy of, or modify, this frame)"
        n921 = call <vilib>:"Add State(s) to Queue__JKI_lib_State_Machine.vi"("State(s) in (\"\")"=w2029) -> ("States Out"=w2028:string)  [unwired: 14 in]
      }
      frame "Run: CaliIncrement" {
        # "Increment Calibration #\n(You can make a copy of, or modify, this frame)"
        n922 = Unbundle By Name(w2031) -> ("IDs.Cali ID"=w2033:i8)
        n923 = Increment(x=w2033) -> (x+1=w2030:i8)
        n924 = Bundle By Name(cluster=w2031, "IDs.Cali ID"=w2030) -> (w2032:T23)
        n925 = call <vilib>:"Add State(s) to Queue__JKI_lib_State_Machine.vi"("State(s) in (\"\")"=w2037) -> ("States Out"=w2036:string)  [unwired: 14 in]
      }
      frame "Run: BGIncrement" {
        # "Increment BG #\n(You can make a copy of, or modify, this frame)"
        n926 = Unbundle By Name(w2038) -> ("IDs.BG ID"=w2041:i8)
        n927 = Increment(x=w2041) -> (x+1=w2040:i8)
        n928 = Bundle By Name(cluster=w2038, "IDs.BG ID"=w2040) -> (w2039:T23)
        n929 = call <vilib>:"Add State(s) to Queue__JKI_lib_State_Machine.vi"("State(s) in (\"\")"=w2045) -> ("States Out"=w2044:string)  [unwired: 14 in]
      }
      frame "Run: Increment" {
        # "Increase Run# by 1"
        n930 = Unbundle By Name(w2050) -> ("IDs.RunID"=w2052:i8)
        n931 = Increment(x=w2052) -> (x+1=w2048:i8)
        n932 = Bundle By Name(cluster=w2050, "IDs.RunID"=w2048) -> (w2051:T23)
        n933 = call "RunIDFGV.vi"("Error In"=w2046, "RunID in"=w2048) -> ("Error Out"=w2047:errorcluster)  [unwired: 8 in, 1 out]
        n934 = call <vilib>:"Add State(s) to Queue__JKI_lib_State_Machine.vi"("State(s) in (\"\")"=w2054) -> ("States Out"=w2053:string)  [unwired: 14 in]
      }
      frame "Run: Decrement" {
        # "Increase Run# by 1"
        n935 = Unbundle By Name(w2059) -> ("IDs.RunID"=w2061:i8)
        n936 = Decrement(x=w2061) -> (x-1=w2057:i8)
        n937 = Bundle By Name(cluster=w2059, "IDs.RunID"=w2057) -> (w2060:T23)
        n938 = call "RunIDFGV.vi"("Error In"=w2055, "RunID in"=w2057) -> ("Error Out"=w2056:errorcluster)  [unwired: 8 in, 1 out]
        n939 = call <vilib>:"Add State(s) to Queue__JKI_lib_State_Machine.vi"("State(s) in (\"\")"=w2063) -> ("States Out"=w2062:string)  [unwired: 14 in]
      }
      frame "---------- SysConfig ----------" {
        # "Template Separator\n(You can make a copy of, or modify, this frame)"
        n940 = call <vilib>:"Add State(s) to Queue__JKI_lib_State_Machine.vi"("State(s) in (\"\")"=w2068) -> ("States Out"=w2067:string)  [unwired: 14 in]
      }
      frame "SysConfig: LoadAPDSerialNumber" {
        # "Template Separator\n(You can make a copy of, or modify, this frame)"
        n941 = call "readAPDSerial.vi"("Error In"=w2070) -> ("Error Out"=w2069:errorcluster, "output cluster"=w2071:T26)  [unwired: 9 in]
        n942 = Bundle By Name(cluster=w2072, "APDSerialNum"=w2071) -> (w2073:T23)
        n943 = call <vilib>:"Add State(s) to Queue__JKI_lib_State_Machine.vi"("State(s) in (\"\")"=w2076) -> ("States Out"=w2075:string)  [unwired: 14 in]
      }
      frame "SysConfig: Load Sys Config" {
        # "[Covers: REQ5]"
        # "Load System config"
        # "Load system configuration\n(Load both hardware and DAQ config)"
        n944 = call "LoadSysConfig.vi"("Error In"=w2079, "Enum"=enum16{"LastUse", "Default"}."LastUse") -> ("Error Out"=w2078:errorcluster, "SysConfigCluster"=w2081:T7)  [unwired: 8 in]
        "SysConfigCluster" <- w2081
        n945 = Bundle By Name(cluster=w2082, "SysConfigCluster"=w2081) -> (w2083:T23)
        n946 = call <vilib>:"Add State(s) to Queue__JKI_lib_State_Machine.vi"("State(s) in (\"\")"=w2085) -> ("States Out"=w2084:string)  [unwired: 14 in]
      }
      frame "SysConfig: Load Digitizer Setting" {
        w2086 = enum16{"Write", "Read"}."Write" ("Operation")
        # "Load DAQ config\nSave to FGV"
        # "Template Separator\n(You can make a copy of, or modify, this frame)"
        n947 = call <userlib>:"Current VIs Parent Directory__ogtk.vi"() -> ("Parent Directory (+ Relative)"=w2100:path)  [unwired: 5 in]
        n948 = Build Path(base path=w2100, name or relative path="SubVI\\DigitizerConfiguration\\V6_Scope_last_use.config") -> (appended path=w2101:path)
        n949 = call "ReadDigitizerConfig(SubVI).vi"("error in (no error)"=w2098, "appended path"=w2101) -> ("error out"=w2094:errorcluster, "FLImDAQ"=w2092:T5)  [unwired: 8 in]
        n950 = call "FLImDAQ_FGV.vi"("error in (no error)"=w2094, "Operation (Read)"=w2086, "Write data"=w2092) -> ("error out"=w2096:errorcluster)  [unwired: 7 in, 1 out]
        n951 = Unbundle By Name(w2092) -> ("min record length"=→"data length":i32, "Digitizer 1"=w2088:refnum<k15>, "Digitizer 2"=w2095:refnum<k15>)
        n952 = Bundle By Name(cluster=w2090, "FLImDAQ"=w2092) -> (w2091:T23)
        n953 = call "Digitizer1_FGV.vi"("error in (no error)"=w2096, "Operation (Read)"=w2086, "Write data"=w2088) -> ("error out"=w2097:errorcluster)  [unwired: 7 in, 1 out]
        n954 = call "Digitizer2_FGV.vi"("error in (no error)"=w2097, "Operation (Read)"=w2086, "Write data"=w2095) -> ("error out"=w2093:errorcluster)  [unwired: 7 in, 1 out]
        n955 = call <vilib>:"Add State(s) to Queue__JKI_lib_State_Machine.vi"("State(s) in (\"\")"=w2103) -> ("States Out"=w2102:string)  [unwired: 14 in]
      }
      frame "SysConfig: Load LJ Pinout" {
        # "Template Separator\n(You can make a copy of, or modify, this frame)"
        n956 = call <userlib>:"Current VIs Parent Directory__ogtk.vi"() -> ("Parent Directory (+ Relative)"=w2118:path)  [unwired: 5 in]
        n957 = Build Path(base path=w2118, name or relative path="SubVI\\LabJack\\LJ_pin_setting.config") -> (appended path=w2116:path)
        n958 = call "ReadLabjackConfig(SubVI).vi"("error in (no error)"=w2114, "appended path"=w2116) -> ("error out"=w2115:errorcluster, "Utility"=w2112:T4)  [unwired: 8 in]
        n959 = Unbundle By Name(w2112) -> ("Ch1 Bias"=w2111:string, "Ch2 Bias"=w2110:string, "Ch3 Bias"=w2109:string, "Ch4 Bias"=w2104:string, "Red LED"=w2106:string, "Green LED"=w2105:string)
        n960 = global write "GlobalVariables.vi" "LED Green pin"(w2105) -> ()
        n961 = global write "GlobalVariables.vi" "Ch1 LJ pin"(w2111) -> ()
        n962 = global write "GlobalVariables.vi" "Ch2 LJ pin"(w2110) -> ()
        n963 = global write "GlobalVariables.vi" "Ch3 LJ pin"(w2109) -> ()
        n964 = global write "GlobalVariables.vi" "Ch4 LJ pin"(w2104) -> ()
        n965 = global write "GlobalVariables.vi" "LED Red pin"(w2106) -> ()
        n966 = Bundle By Name(cluster=w2107, "LJ Pinout"=w2112) -> (w2113:T23)
        n967 = call <vilib>:"Add State(s) to Queue__JKI_lib_State_Machine.vi"("State(s) in (\"\")"=w2120) -> ("States Out"=w2119:string)  [unwired: 14 in]
      }
      frame "SysConfig: Load 355 PWM" {
        # "Template Separator\n(You can make a copy of, or modify, this frame)"
        n968 = call <userlib>:"Current VIs Parent Directory__ogtk.vi"() -> ("Parent Directory (+ Relative)"=w2138:path)  [unwired: 5 in]
        n969 = Build Path(base path=w2138, name or relative path="SubVI\\LabJack\\PWM_setting_355.config") -> (appended path=w2136:path)
        n970 = call "ReadPWMConfig(SubVI).vi"("error in (no error)"=w2133, "appended path"=w2136) -> ("error out"=w2134:errorcluster, "PWM Setting"=w2132:T41)  [unwired: 8 in]
        n971 = Unbundle By Name(w2132) -> ("DIO_EF_CLOCK1_DIVISOR"=w2129:i16, "DIO_EF_CLOCK1_ROLL_VALUE"=w2128:i32)
        n972 = Multiply(x=w2129, y=w2128) -> (x*y=w2130:i32)
        n973 = Bundle By Name(cluster=w2135, "355 PWM setting"=w2132) -> (w2122:T23)
        n974 = Divide(x=80000000.0, y=w2130) -> (x/y=w2127:dbl)
        "Laser Rep Rate" <- w2127
        n975 = Number To Decimal String(number=w2127) -> (decimal integer string=w2126:string)  [unwired: 1 in]
        n976 = Concatenate Strings("355nm " ("string"), w2126, "Hz" ("string")) -> (w2124:string)
        n977 = property on="355nm Laser toggle" class="Bool (strict)"("Caption.Text"=w2124) -> ()  [unwired: 2 in, 2 out]
        n978 = call <vilib>:"Add State(s) to Queue__JKI_lib_State_Machine.vi"("State(s) in (\"\")"=w2140) -> ("States Out"=w2139:string)  [unwired: 14 in]
      }
      frame "SysConfig: Load AB PWM" {
        # "Template Separator\n(You can make a copy of, or modify, this frame)"
        n979 = call <userlib>:"Current VIs Parent Directory__ogtk.vi"() -> ("Parent Directory (+ Relative)"=w2149:path)  [unwired: 5 in]
        n980 = Build Path(base path=w2149, name or relative path="SubVI\\LabJack\\PWM_setting_AB.config") -> (appended path=w2147:path)
        n981 = call "ReadPWMConfig(SubVI).vi"("error in (no error)"=w2144, "appended path"=w2147) -> ("error out"=w2145:errorcluster, "PWM Setting"=w2143:T41)  [unwired: 8 in]
        n982 = Bundle By Name(cluster=w2141, "AB PWM setting"=w2143) -> (w2146:T23)
        n983 = call <vilib>:"Add State(s) to Queue__JKI_lib_State_Machine.vi"("State(s) in (\"\")"=w2151) -> ("States Out"=w2150:string)  [unwired: 14 in]
      }
      frame "SysConfig: Load AB setting" {
        # "load aming beam setting\n(check frequency, if 0 do nothing, if not zero, config PWM)"
        n984 = call "readAimingBeamSetting.vi"("error in (no error)"=w2169) -> ("error out"=w2164:errorcluster, "Aiming Beam Setting"=w2156:T42)  [unwired: 9 in]
        n985 = Unbundle By Name(w2156) -> ("Default Current"=w2155:dbl)
        n986 = Unbundle By Name(w2156) -> ("Frequency(Hz)"=w2152:u32)
        n987 = Equal To 0?(x=w2152) -> (x = 0?=w2162:bool)
        n988 = Select(t="", s=w2162, f="SysConfig: Load AB PWM" ("State(s) in Front (\"\")")) -> (s? t:f=w2165:string)
        n989 = Number To Decimal String(number=w2152) -> (decimal integer string=w2161:string)  [unwired: 1 in]
        n990 = Number To Decimal String(number=w2155, width (-)=i16 2) -> (decimal integer string=w2154:string)
        n991 = Concatenate Strings("445nm " ("string"), w2161, "Hz " ("string"), w2154, "mA" ("string")) -> (w2160:string)
        n992 = property on="Aiming beam toggle" class="Bool (strict)"("Caption.Text"=w2160) -> ()  [unwired: 2 in, 2 out]
        n993 = case shown="False" w2162 {
          tunnel: w2164 -> [w2177 w2180]
          tunnel: [w2176 w2180] -> w2163
          tunnel: w2152 -> [w2175 _]
          frame False {
            n994 = call "LJ_calculate_PWM_parameters.vi"("Duty Cycle (%)"=u32 10, "Error In"=w2177, "Show Confirmation"=FALSE, "Laser Rep Rate (Hz)"=w2175, "Laser"=enum16{"355nm", "AimingBeam"}."AimingBeam") -> ("Error Out"=w2176:errorcluster)  [unwired: 5 in, 1 out]
          }
          frame True {
          }
        }
        n995 = Bundle By Name(cluster=w2170, "AB Cluster"=w2156) -> (w2171:T23)
        n996 = call <vilib>:"Add State(s) to Queue__JKI_lib_State_Machine.vi"("State(s) in Front (\"\")"=w2165, "State(s) in (\"\")"=w2173) -> ("States Out"=w2172:string)  [unwired: 13 in]
      }
      frame "SysConfig: LoadABVideoSetting" {
        # "Load AB video setting form ini file\n()"
        n997 = call "readVideoConfig.vi"("error in (no error)"=w2184) -> ("error out"=w2185:errorcluster, "Aiming Beam Config"=w2183:T22)  [unwired: 8 in, 1 out]
        n998 = Bundle By Name(cluster=w2181, "VideoConfig"=w2183) -> (w2182:T23)
        n999 = call <vilib>:"Add State(s) to Queue__JKI_lib_State_Machine.vi"("State(s) in (\"\")"=w2188) -> ("States Out"=w2187:string)  [unwired: 14 in]
      }
      frame "SysConfig: LoadCursorLocation" {
        # "Load cursor location from ini file\n(load cursor from system setting ini file)"
        n1000 = call "readCursorConfigMain.vi"("error in (no error)"=w2200) -> ("error out"=w2201:errorcluster, "Cursor Locations"=w2199:T43)  [unwired: 9 in]
        n1001 = Unbundle By Name(w2199) -> ("DC1"=w2198:i32, "DC2"=w2197:i32, "BG1"=w2192:i32, "BG2"=w2191:i32)
        n1002 = Build Array(w2198, w2197) -> (w2196:i32[])
        n1003 = Build Array(w2192, w2191) -> (w2193:i32[])
        n1004 = Array Max & Min(array=w2196) -> (max value=w2195:i32, min value=w2194:i32)  [unwired: 2 out]
        n1005 = Array Max & Min(array=w2193) -> (max value=w2190:i32, min value=w2189:i32)  [unwired: 2 out]
        n1006 = global write "GlobalVariables.vi" "DC Idx2"(w2195) -> ()
        n1007 = global write "GlobalVariables.vi" "DC Idx1"(w2194) -> ()
        n1008 = global write "GlobalVariables.vi" "BG Idx2"(w2190) -> ()
        n1009 = global write "GlobalVariables.vi" "BG Idx1"(w2189) -> ()
        n1010 = call <vilib>:"Add State(s) to Queue__JKI_lib_State_Machine.vi"("State(s) in (\"\")"=w2205) -> ("States Out"=w2204:string)  [unwired: 14 in]
      }
      frame "---------- SystemStatus ----------" {
        # "Template Separator\n(You can make a copy of, or modify, this frame)"
        n1011 = call <vilib>:"Add State(s) to Queue__JKI_lib_State_Machine.vi"("State(s) in (\"\")"=w2210) -> ("States Out"=w2209:string)  [unwired: 14 in]
      }
      frame "SystemStatus: SlowSysStatusMacro" {
        # "store system check time"
        # "Template Separator\n(You can make a copy of, or modify, this frame)"
        n1012 = Tick Count (ms)() -> (millisecond timer value=w2213:u32)
        n1013 = Bundle By Name(cluster=w2211, "SlowTimer"=w2213) -> (w2212:T23)
        n1014 = call <vilib>:"Add State(s) to Queue__JKI_lib_State_Machine.vi"("State(s) in Front (\"\")"="Digitizer: checkTemp\nTCP: CheckConnection" ("State(s) in Front (\"\")"), "State(s) in (\"\")"=w2218) -> ("States Out"=w2217:string)  [unwired: 13 in]
      }
      frame "SystemStatus: FastSysStatusMacro" {
        # "store system check time"
        # "Template Separator\n(You can make a copy of, or modify, this frame)"
        n1015 = Tick Count (ms)() -> (millisecond timer value=w2221:u32)
        n1016 = Bundle By Name(cluster=w2219, "FastTimer"=w2221) -> (w2220:T23)
        n1017 = call <vilib>:"Add State(s) to Queue__JKI_lib_State_Machine.vi"("State(s) in Front (\"\")"="355 Laser: CheckPWMStatus\nAimingBeam: GetPWMStatus\n/*355 Laser: CheckControllerStatus" ("State(s) in Front (\"\")"), "State(s) in (\"\")"=w2226) -> ("States Out"=w2225:string)  [unwired: 13 in]
      }
      frame "---------- UI ----------" {
        # "Do not put any code in this frame.\n(It is a separator no-op. You can make a copy of this frame to create a new UI frame)"
        n1018 = call <vilib>:"Add State(s) to Queue__JKI_lib_State_Machine.vi"("State(s) in (\"\")"=w2231) -> ("States Out"=w2230:string)  [unwired: 14 in]
      }
      frame "UI: Initialize" {
        w2233 = T44 {"Minimum"=0.0, "Maximum"=4.6, "Increment"=0.1} ("Data Entry Limits")
        w2232 = T11."Disabled and Grayed Out" ("Disabled")
        # "Disable all button on startup"
        # "Initialize the User Interface, here.\n(this is called automatically, by the Macro: Init)"
        n1019 = property on="V 1" class="DigNum (strict)"("DisabledEnum"=w2232) -> ()  [unwired: 2 in, 2 out]
        n1020 = property on="V 2" class="DigNum (strict)"("DisabledEnum"=w2232) -> ()  [unwired: 2 in, 2 out]
        n1021 = property on="StopButton" class="Bool (strict)"("DisabledEnum"=w2232) -> ()  [unwired: 2 in, 2 out]
        n1022 = property on="Sys Reconfig" class="Bool"("DisabledEnum"=w2232) -> ()  [unwired: 2 in, 2 out]
        n1023 = property on="StartButton" class="Bool (strict)"("DisabledEnum"=w2232) -> ()  [unwired: 2 in, 2 out]
        n1024 = property on="355nm Laser toggle" class="Bool (strict)"("DisabledEnum"=w2232) -> ()  [unwired: 2 in, 2 out]
        n1025 = property on="Aiming beam toggle" class="Bool (strict)"("DisabledEnum"=w2232) -> ()  [unwired: 2 in, 2 out]
        n1026 = property on="Background" class="Bool (strict)"("DisabledEnum"=w2232) -> ()  [unwired: 2 in, 2 out]
        n1027 = property on="Cali&iRF alignment" class="Bool (strict)"("DisabledEnum"=w2232) -> ()  [unwired: 2 in, 2 out]
        n1028 = property on="V 3" class="DigNum (strict)"("DisabledEnum"=w2232) -> ()  [unwired: 2 in, 2 out]
        n1029 = property on="Video Source" class="RadioBtnsControl (strict)"("DisabledEnum"=w2232) -> ()  [unwired: 2 in, 2 out]
        n1030 = property on="V 1" class="DigNum (strict)"("Data Range"=w2233) -> ()  [unwired: 2 in, 2 out]
        n1031 = property on="V 2" class="DigNum (strict)"("Data Range"=w2233) -> ()  [unwired: 2 in, 2 out]
        n1032 = property on="V 3" class="DigNum (strict)"("Data Range"=w2233) -> ()  [unwired: 2 in, 2 out]
        n1033 = call <vilib>:"Add State(s) to Queue__JKI_lib_State_Machine.vi"("State(s) in Front (\"\")"="UI: CaliAndiRFNotReady" ("State(s) in Front (\"\")"), "State(s) in (\"\")"=w2239) -> ("States Out"=w2238:string)  [unwired: 13 in]
      }
      frame "UI: BGLoaded" {
        # "[Covers: REQ24]"
        # "Do not put any code in this frame.\n(It is a separator no-op. You can make a copy of this frame to create a new UI frame)"
        n1034 = property on="Background" class="Bool (strict)"("BoolText.Text"="Loaded!" ("Boolean Text.Text"), "Colors [4]"=cluster{u32, u32}[] [{15764023, 15764023}, {16711680, 16711680}]) -> ()  [unwired: 2 in, 2 out]
        n1035 = call <vilib>:"Add State(s) to Queue__JKI_lib_State_Machine.vi"("State(s) in (\"\")"=w2246) -> ("States Out"=w2245:string)  [unwired: 14 in]
      }
      frame "UI: BGSizeError" {
        # "[Covers: REQ24]"
        # "Do not put any code in this frame.\n(It is a separator no-op. You can make a copy of this frame to create a new UI frame)"
        n1036 = property on="Background" class="Bool (strict)"("BoolText.Text"="Loaded!" ("Boolean Text.Text"), "Colors [4]"=cluster{u32, u32}[] [{7171459, 7171459}, {16711680, 16711680}]) -> ()  [unwired: 2 in, 2 out]
        n1037 = One Button Dialog(message="Background waveform length and current digitizer setting mismatch! Please take a new background before any aquisition!") -> ()  [unwired: 1 in, 1 out]
        n1038 = call <vilib>:"Add State(s) to Queue__JKI_lib_State_Machine.vi"("State(s) in (\"\")"=w2254) -> ("States Out"=w2253:string)  [unwired: 14 in]
      }
      frame "UI: CaliAndiRFLoaded" {
        # "[Covers: REQ24]"
        # "Do not put any code in this frame.\n(It is a separator no-op. You can make a copy of this frame to create a new UI frame)"
        n1039 = property on="Cali&iRF alignment" class="Bool (strict)"("BoolText.Text"="Loaded!" ("Boolean Text.Text"), "Colors [4]"=cluster{u32, u32}[] [{15764023, 15764023}, {16711680, 16711680}]) -> ()  [unwired: 2 in, 2 out]
        n1040 = call <vilib>:"Add State(s) to Queue__JKI_lib_State_Machine.vi"("State(s) in (\"\")"=w2261) -> ("States Out"=w2260:string)  [unwired: 14 in]
      }
      frame "UI: WFAutoScale" {
        # "Set graph auto scale.\n(UI: WFAutoScale >> T/F)"
        n1041 = Equal?(x=w2262, y="F") -> (x = y?=w2263:bool)
        n1042 = Equal?(x=w2262, y="T") -> (x = y?=w2265:bool)
        n1043 = case shown="True" w2265 {
          frame False {
          }
          frame True {
            w2281 = u8 2 ("Y Scale.Scale Fit")
            n1044 = property on="Channel 1" class="WFGraph (strict)"("YScale.ScaleFit"=w2281) -> ()  [unwired: 2 in, 2 out]
            n1045 = property on="Channel 2" class="WFGraph (strict)"("YScale.ScaleFit"=w2281) -> ()  [unwired: 2 in, 2 out]
            n1046 = property on="Channel 3" class="WFGraph (strict)"("YScale.ScaleFit"=w2281) -> ()  [unwired: 2 in, 2 out]
          }
        }
        n1047 = case shown="True" w2263 {
          frame False {
          }
          frame True {
            w2278 = 0.0 ("Y Scale.Range:Maximum")
            w2279 = 2.0 ("Y Scale.Range:Maximum")
            w2280 = u8 0 ("Y Scale.Scale Fit")
            n1048 = property on="Channel 1" class="WFGraph (strict)"("YScale.ScaleFit"=w2280) -> (error out=w2277:errorcluster)  [unwired: 2 in, 1 out]
            n1049 = property on="Channel 2" class="WFGraph (strict)"("YScale.ScaleFit"=w2280) -> (error out=w2276:errorcluster)  [unwired: 2 in, 1 out]
            n1050 = property on="Channel 3" class="WFGraph (strict)"("YScale.ScaleFit"=w2280) -> (error out=w2275:errorcluster)  [unwired: 2 in, 1 out]
            n1051 = property on="Channel 1" class="WFGraph (strict)"(error in=w2277, "YScale.Maximum"=w2279) -> (error out=w2274:errorcluster)  [unwired: 1 in, 1 out]
            n1052 = property on="Channel 2" class="WFGraph (strict)"(error in=w2276, "YScale.Maximum"=w2279) -> (error out=w2273:errorcluster)  [unwired: 1 in, 1 out]
            n1053 = property on="Channel 3" class="WFGraph (strict)"(error in=w2275, "YScale.Maximum"=w2279) -> (error out=w2272:errorcluster)  [unwired: 1 in, 1 out]
            n1054 = property on="Channel 1" class="WFGraph (strict)"(error in=w2274, "YScale.Minimum"=w2278) -> ()  [unwired: 1 in, 2 out]
            n1055 = property on="Channel 2" class="WFGraph (strict)"(error in=w2273, "YScale.Minimum"=w2278) -> ()  [unwired: 1 in, 2 out]
            n1056 = property on="Channel 3" class="WFGraph (strict)"(error in=w2272, "YScale.Minimum"=w2278) -> ()  [unwired: 1 in, 2 out]
          }
        }
        n1057 = call <vilib>:"Add State(s) to Queue__JKI_lib_State_Machine.vi"("State(s) in (\"\")"=w2271) -> ("States Out"=w2270:string)  [unwired: 14 in]
      }
      frame "UI: showDisclaimer" {
        # "Show disclamer window.\n(It is a separator no-op. You can make a copy of this frame to create a new UI frame)"
        n1058 = call <vilib>:"Application Directory.vi"() -> ("Application Directory"=w2294:path)
        n1059 = Build Path(base path=w2294, name or relative path="Disclamer.png") -> (appended path=w2292:path)
        n1060 = property on="Disclamer" class="Pict"() -> ("Draw Area Size"=w2290:T45)  [unwired: 2 in, 2 out]
        n1061 = disable-structure "Diagram Disable Structure" shown="Disabled" {
          frame Disabled {
            n1062 = flat-sequence {
              frame #0 {
                n1063 = call "disclaimer.vi"() -> ()  [unwired: 12 in]
              }
              frame #1 {
                n1064 = Wait (ms)(milliseconds to wait=u32 250) -> ()  [unwired: 1 out]
              }
              frame #2 {
                n1065 = call "SoftwareNote.vi"() -> ()  [unwired: 12 in]
              }
            }
          }
          frame Enabled {
          }
        }
        n1066 = call <vilib>:"Read PNG File.vi"("path to PNG file"=w2292) -> ("image data"=w2289:T46)  [unwired: 8 in, 2 out]
        n1067 = Unbundle By Name(w2289) -> ("Rectangle.right"=w2287:i16, "Rectangle.bottom"=w2285:i16)
        n1068 = Unbundle By Name(w2290) -> ("Width"=w2288:u32, "Height"=w2286:u32)
        n1069 = call <vilib>:"Draw Flattened Pixmap.vi"("image data"=w2289) -> ("new picture"=→"Disclamer":picture)  [unwired: 8 in]
        n1070 = Divide(x=w2288, y=w2287) -> (x/y=w2284:dbl)
        n1071 = Divide(x=w2286, y=w2285) -> (x/y=w2283:dbl)
        n1072 = Max & Min(x=w2284, y=w2283) -> (min(x,y)=w2282:dbl)  [unwired: 1 out]
        n1073 = property on="Disclamer" class="Pict"("ZoomFactor"=w2282) -> ()  [unwired: 2 in, 2 out]
        n1074 = call <vilib>:"Add State(s) to Queue__JKI_lib_State_Machine.vi"("State(s) in (\"\")"=w2299) -> ("States Out"=w2298:string)  [unwired: 14 in]
      }
      frame "UI: CaliAndiRFNotReady" {
        # "Do not put any code in this frame.\n(It is a separator no-op. You can make a copy of this frame to create a new UI frame)"
        n1075 = property on="Cali&iRF alignment" class="Bool (strict)"("BoolText.Text"="No Info" ("Boolean Text.Text"), "Colors [4]"=cluster{u32, u32}[] [{13816530, 13816530}, {16711680, 16711680}]) -> ()  [unwired: 2 in, 2 out]
        n1076 = call <vilib>:"Add State(s) to Queue__JKI_lib_State_Machine.vi"("State(s) in (\"\")"=w2307) -> ("States Out"=w2306:string)  [unwired: 14 in]
      }
      frame "UI: BGnotReady" {
        # "Do not put any code in this frame.\n(It is a separator no-op. You can make a copy of this frame to create a new UI frame)"
        n1077 = property on="Background" class="Bool (strict)"("BoolText.Text"="No Info" ("Boolean Text.Text"), "Colors [4]"=cluster{u32, u32}[] [{13816530, 13816530}, {16711680, 16711680}]) -> ()  [unwired: 2 in, 2 out]
        n1078 = call <vilib>:"Add State(s) to Queue__JKI_lib_State_Machine.vi"("State(s) in (\"\")"=w2314) -> ("States Out"=w2313:string)  [unwired: 14 in]
      }
      frame "UI: Reset" {
        w2316 = cluster{u32, u32}[] [{13816530, 13816530}, {13816530, 13816530}] ("Colors [4]")
        # "Do not put any code in this frame.\n(It is a separator no-op. You can make a copy of this frame to create a new UI frame)"
        n1079 = property on="Cali&iRF alignment" class="Bool (strict)"("BoolText.Text"="No Info" ("Boolean Text.Text"), "Colors [4]"=w2316) -> ()  [unwired: 2 in, 2 out]
        n1080 = property on="Background" class="Bool (strict)"("BoolText.Text"="No Info" ("Boolean Text.Text"), "Colors [4]"=w2316) -> ()  [unwired: 2 in, 2 out]
        n1081 = call <vilib>:"Add State(s) to Queue__JKI_lib_State_Machine.vi"("State(s) in (\"\")"=w2322) -> ("States Out"=w2321:string)  [unwired: 14 in]
      }
      frame "UI: SetButtonText" {
        # "Set button text of 355nm laser and aiming beam."
        n1082 = call <vilib>:"Add State(s) to Queue__JKI_lib_State_Machine.vi"("State(s) in (\"\")"=w2327) -> ("States Out"=w2326:string)  [unwired: 14 in]
      }
      frame "UI: DuringAquisition" {
        w2330 = T11."Disabled and Grayed Out" ("Disabled")
        # "Do not put any code in this frame.\n(It is a separator no-op. You can make a copy of this frame to create a new UI frame)"
        n1083 = Unbundle By Name(w2329) -> ("bothVidSourceAvail"=w2328:bool)
        n1084 = case shown="True" w2328 {
          tunnel: w2330 -> [_ w2336]
          frame False {
          }
          frame True {
            n1085 = property on="Video Source" class="RadioBtnsControl (strict)"("DisabledEnum"=w2336) -> ()  [unwired: 2 in, 2 out]
          }
        }
        n1086 = property on="StartButton" class="Bool (strict)"("DisabledEnum"=w2330) -> ()  [unwired: 2 in, 2 out]
        n1087 = property on="Sys Reconfig" class="Bool"("DisabledEnum"=w2330) -> ()  [unwired: 2 in, 2 out]
        n1088 = property on="355nm Laser toggle" class="Bool (strict)"("DisabledEnum"=w2330) -> ()  [unwired: 2 in, 2 out]
        n1089 = property on="Aiming beam toggle" class="Bool (strict)"("DisabledEnum"=w2330) -> ()  [unwired: 2 in, 2 out]
        n1090 = property on="Background" class="Bool (strict)"("DisabledEnum"=w2330) -> ()  [unwired: 2 in, 2 out]
        n1091 = property on="Radio Buttons" class="RadioBtnsControl (strict)"("DisabledEnum"=w2330) -> ()  [unwired: 2 in, 2 out]
        n1092 = property on="Cali&iRF alignment" class="Bool (strict)"("DisabledEnum"=w2330) -> ()  [unwired: 2 in, 2 out]
        n1093 = property on="Quit" class="Bool"("DisabledEnum"=w2330) -> ()  [unwired: 2 in, 2 out]
        n1094 = property on="Skip Data Save?" class="Bool (strict)"("DisabledEnum"=w2330) -> ()  [unwired: 2 in, 2 out]
        n1095 = property on="Video Display" class="Bool (strict)"("DisabledEnum"=w2330) -> ()  [unwired: 2 in, 2 out]
        n1096 = property on="StopButton" class="Bool (strict)"("DisabledEnum"=T11."Enabled" ("Disabled")) -> ()  [unwired: 2 in, 2 out]
        n1097 = call <vilib>:"Add State(s) to Queue__JKI_lib_State_Machine.vi"("State(s) in (\"\")"=w2335) -> ("States Out"=w2334:string)  [unwired: 14 in]
      }
      frame "UI: duringIRFAlign" {
        w2337 = T11."Disabled and Grayed Out" ("Disabled")
        # "Set UI to during iRF alignment\n(It is a separator no-op. You can make a copy of this frame to create a new UI frame)"
        n1098 = property on="StartButton" class="Bool (strict)"("DisabledEnum"=w2337) -> ()  [unwired: 2 in, 2 out]
        n1099 = property on="Sys Reconfig" class="Bool"("DisabledEnum"=w2337) -> ()  [unwired: 2 in, 2 out]
        n1100 = property on="355nm Laser toggle" class="Bool (strict)"("DisabledEnum"=w2337) -> ()  [unwired: 2 in, 2 out]
        n1101 = property on="Aiming beam toggle" class="Bool (strict)"("DisabledEnum"=w2337) -> ()  [unwired: 2 in, 2 out]
        n1102 = property on="Background" class="Bool (strict)"("DisabledEnum"=w2337) -> ()  [unwired: 2 in, 2 out]
        n1103 = property on="StopButton" class="Bool (strict)"("DisabledEnum"=w2337) -> ()  [unwired: 2 in, 2 out]
        n1104 = call <vilib>:"Add State(s) to Queue__JKI_lib_State_Machine.vi"("State(s) in (\"\")"=w2342) -> ("States Out"=w2341:string)  [unwired: 14 in]
      }
      frame "UI: duringBGAcquire" {
        w2343 = T11."Disabled and Grayed Out" ("Disabled")
        # "Do not put any code in this frame.\n(It is a separator no-op. You can make a copy of this frame to create a new UI frame)"
        n1105 = property on="StartButton" class="Bool (strict)"("DisabledEnum"=w2343) -> ()  [unwired: 2 in, 2 out]
        n1106 = property on="StopButton" class="Bool (strict)"("DisabledEnum"=w2343) -> ()  [unwired: 2 in, 2 out]
        n1107 = property on="Sys Reconfig" class="Bool"("DisabledEnum"=w2343) -> ()  [unwired: 2 in, 2 out]
        n1108 = property on="355nm Laser toggle" class="Bool (strict)"("DisabledEnum"=w2343) -> ()  [unwired: 2 in, 2 out]
        n1109 = property on="Aiming beam toggle" class="Bool (strict)"("DisabledEnum"=w2343) -> ()  [unwired: 2 in, 2 out]
        n1110 = property on="Cali&iRF alignment" class="Bool (strict)"("DisabledEnum"=w2343) -> ()  [unwired: 2 in, 2 out]
        n1111 = call <vilib>:"Add State(s) to Queue__JKI_lib_State_Machine.vi"("State(s) in (\"\")"=w2348) -> ("States Out"=w2347:string)  [unwired: 14 in]
      }
      frame "UI: ReadyForAquisition" {
        w2352 = T11."Enabled" ("Disabled")
        # "Do not put any code in this frame.\n(It is a separator no-op. You can make a copy of this frame to create a new UI frame)"
        n1112 = Unbundle By Name(w2351) -> ("System Status.TCP/IP"=w2350:bool, "bothVidSourceAvail"=w2349:bool)
        n1113 = property on="StartButton" class="Bool (strict)"("DisabledEnum"=w2352) -> ()  [unwired: 2 in, 2 out]
        n1114 = property on="Sys Reconfig" class="Bool"("DisabledEnum"=w2352) -> ()  [unwired: 2 in, 2 out]
        n1115 = property on="355nm Laser toggle" class="Bool (strict)"("DisabledEnum"=w2352) -> ()  [unwired: 2 in, 2 out]
        n1116 = property on="Aiming beam toggle" class="Bool (strict)"("DisabledEnum"=w2352) -> ()  [unwired: 2 in, 2 out]
        n1117 = property on="Cali&iRF alignment" class="Bool (strict)"("DisabledEnum"=w2352) -> ()  [unwired: 2 in, 2 out]
        n1118 = property on="Background" class="Bool (strict)"("DisabledEnum"=w2352) -> ()  [unwired: 2 in, 2 out]
        n1119 = property on="Quit" class="Bool"("DisabledEnum"=w2352) -> ()  [unwired: 2 in, 2 out]
        n1120 = property on="Radio Buttons" class="RadioBtnsControl (strict)"("DisabledEnum"=w2352) -> ()  [unwired: 2 in, 2 out]
        n1121 = case shown="True" w2349 {
          tunnel: w2352 -> [_ w2358]
          frame False {
          }
          frame True {
            n1122 = property on="Video Source" class="RadioBtnsControl (strict)"("DisabledEnum"=w2358) -> ()  [unwired: 2 in, 2 out]
          }
        }
        n1123 = property on="Skip Data Save?" class="Bool (strict)"("DisabledEnum"=w2352) -> ()  [unwired: 2 in, 2 out]
        n1124 = case shown="True" w2350 {
          tunnel: w2352 -> [_ w2359]
          frame False {
          }
          frame True {
            n1125 = property on="Video Display" class="Bool (strict)"("DisabledEnum"=w2359) -> ()  [unwired: 2 in, 2 out]
          }
        }
        n1126 = property on="StopButton" class="Bool (strict)"("DisabledEnum"=T11."Disabled and Grayed Out" ("Disabled")) -> ()  [unwired: 2 in, 2 out]
        n1127 = call <vilib>:"Add State(s) to Queue__JKI_lib_State_Machine.vi"("State(s) in (\"\")"=w2357) -> ("States Out"=w2356:string)  [unwired: 14 in]
      }
      frame "UI: Update" {
        # "Do not put any code in this frame.\n(It is a separator no-op. You can make a copy of this frame to create a new UI frame)"
        n1128 = Unbundle By Name(w2370) -> ("System Status"=→"System Hardware Connection Status":T2, "IDs.RunID"=→"Run #":i8, "CaseID"=→"Case #":string, "FLImDAQ"=→"FLImDAQ":T30, "SysRunning?"=→"Aquisition Status:":bool, "LJ Pinout"=→"LJ Pinout":T4, "IDs.BG ID"=→"BG #":i8, "IDs.Cali ID"=→"Calibration #":i8, "video source"=→"Visualization PC video source":T1)
        n1129 = call <vilib>:"Add State(s) to Queue__JKI_lib_State_Machine.vi"("State(s) in (\"\")"=w2373) -> ("States Out"=w2372:string)  [unwired: 14 in]
      }
      frame "UI: updateVideoToggle" {
        # "Set video toggle based on visualization PC video source.\n(take )"
        n1130 = call <vilib>:"Add State(s) to Queue__JKI_lib_State_Machine.vi"("State(s) in (\"\")"=w2378) -> ("States Out"=w2377:string)  [unwired: 14 in]
      }
      frame "UI: Cursor Set" {
        # "Argument"
        # "Set and Unset Cursor Busy.\n(Usage: \"UI: Cursor Set >> Busy|Idle\")"
        n1131 = case shown="\"Idle\", Default" w2380 {
          tunnel: w2382 -> [w2387 w2389]
          tunnel: [w2386 w2388] -> w2381
          frame "Idle", Default {
            n1132 = call <vilib>:"Unset Busy.vi"("error in (no error)"=w2387) -> ("error out"=w2386:errorcluster)  [unwired: 10 in]
          }
          frame "Busy" {
            n1133 = call <vilib>:"Set Busy.vi"("error in (no error)"=w2389) -> ("error out"=w2388:errorcluster)  [unwired: 9 in, 1 out]
          }
        }
        n1134 = call <vilib>:"Add State(s) to Queue__JKI_lib_State_Machine.vi"("State(s) in (\"\")"=w2385) -> ("States Out"=w2384:string)  [unwired: 14 in]
      }
      frame "UI: Front Panel State" {
        # "Argument"
        # "Set Front Panel Open or Closed\n(Usage: \"UI: Front Panel State >> Open|Close\")"
        n1135 = Unbundle By Name(w2393) -> ("Core.Current VI Reference"=w2392:refnum<vi>)
        n1136 = case shown="\"Open\", \"Standard\", Default" w2391 {
          tunnel: w2395 -> [w2403 w2418 w2429 w2442 w2455]
          tunnel: [w2405 w2419 w2431 w2444 w2457] -> w2394
          tunnel: w2392 -> [w2404 w2416 w2430 w2443 w2456]
          frame "Open", "Standard", Default {
            w2398 = T17."Standard" ("State")
            n1137 = property on="Property Node" class="VI"(reference=w2404, error in=w2403) -> (reference out=w2401:refnum<vi>, error out=w2402:errorcluster, "FP.State"=w2400:T17)
            n1138 = Not Equal?(x=w2400, y=w2398) -> (x != y?=w2399:bool)
            n1139 = case shown="True" w2399 {
              tunnel: [w2409 w2411] -> w2405
              tunnel: w2402 -> [w2408 w2411]
              tunnel: w2401 -> [w2407 _]
              tunnel: w2398 -> [w2406 _]
              frame True {
                n1140 = invoke on="Invoke Node" class="VI" method="FP.Open"(reference=w2407, error in=w2408, "Activate"=TRUE, "State"=w2406) -> (error out=w2409:errorcluster)  [unwired: 1 in, 4 out]
              }
              frame False {
              }
            }
          }
          frame "Close", "Closed" {
            n1141 = property on="Property Node" class="VI"(reference=w2416, error in=w2418) -> (reference out=w2415:refnum<vi>, error out=w2417:errorcluster, "FP.State"=w2413:T17)
            n1142 = Not Equal?(x=w2413, y=T17."Closed" ("Front Panel Window:State")) -> (x != y?=w2412:bool)
            n1143 = case shown="True" w2412 {
              tunnel: [w2420 w2423] -> w2419
              tunnel: w2417 -> [w2420 w2422]
              tunnel: w2415 -> [_ w2421]
              frame False {
              }
              frame True {
                n1144 = invoke on="Invoke Node" class="VI" method="FP.Close"(reference=w2421, error in=w2422) -> (error out=w2423:errorcluster)  [unwired: 1 in, 2 out]
              }
            }
          }
          frame "Hidden", "Hide" {
            w2424 = T17."Hidden" ("State")
            n1145 = property on="Property Node" class="VI"(reference=w2430, error in=w2429) -> (reference out=w2427:refnum<vi>, error out=w2428:errorcluster, "FP.State"=w2426:T17)
            n1146 = Not Equal?(x=w2426, y=w2424) -> (x != y?=w2425:bool)
            n1147 = case shown="True" w2425 {
              tunnel: [w2435 w2436] -> w2431
              tunnel: w2428 -> [w2434 w2436]
              tunnel: w2427 -> [w2433 _]
              tunnel: w2424 -> [w2432 _]
              frame True {
                n1148 = invoke on="Invoke Node" class="VI" method="FP.Open"(reference=w2433, error in=w2434, "State"=w2432) -> (error out=w2435:errorcluster)  [unwired: 2 in, 4 out]
              }
              frame False {
              }
            }
          }
          frame "Minimize", "Minimized" {
            w2437 = T17."Minimized" ("State")
            n1149 = property on="Property Node" class="VI"(reference=w2443, error in=w2442) -> (reference out=w2440:refnum<vi>, error out=w2441:errorcluster, "FP.State"=w2439:T17)
            n1150 = Not Equal?(x=w2439, y=w2437) -> (x != y?=w2438:bool)
            n1151 = case shown="True" w2438 {
              tunnel: [w2448 w2449] -> w2444
              tunnel: w2441 -> [w2447 w2449]
              tunnel: w2440 -> [w2446 _]
              tunnel: w2437 -> [w2445 _]
              frame True {
                n1152 = invoke on="Invoke Node" class="VI" method="FP.Open"(reference=w2446, error in=w2447, "State"=w2445) -> (error out=w2448:errorcluster)  [unwired: 2 in, 4 out]
              }
              frame False {
              }
            }
          }
          frame "Maximize", "Maximized" {
            w2450 = T17."Maximized" ("State")
            n1153 = property on="Property Node" class="VI"(reference=w2456, error in=w2455) -> (reference out=w2453:refnum<vi>, error out=w2454:errorcluster, "FP.State"=w2452:T17)
            n1154 = Not Equal?(x=w2452, y=w2450) -> (x != y?=w2451:bool)
            n1155 = case shown="True" w2451 {
              tunnel: [w2461 w2462] -> w2457
              tunnel: w2454 -> [w2460 w2462]
              tunnel: w2453 -> [w2459 _]
              tunnel: w2450 -> [w2458 _]
              frame True {
                n1156 = invoke on="Invoke Node" class="VI" method="FP.Open"(reference=w2459, error in=w2460, "State"=w2458) -> (error out=w2461:errorcluster)  [unwired: 2 in, 4 out]
              }
              frame False {
              }
            }
          }
        }
        n1157 = call <vilib>:"Add State(s) to Queue__JKI_lib_State_Machine.vi"("State(s) in (\"\")"=w2397) -> ("States Out"=w2396:string)  [unwired: 14 in]
      }
      frame "---------- AimingBeam ----------" {
        # "Template Separator\n(You can make a copy of, or modify, this frame)"
        n1158 = call <vilib>:"Add State(s) to Queue__JKI_lib_State_Machine.vi"("State(s) in (\"\")"=w2467) -> ("States Out"=w2466:string)  [unwired: 14 in]
      }
      frame "AimingBeam: Initialize" {
        # "set aiming beam button color"
        # "Open COM port for Aiming Beam\n(Require USB connection)"
        n1159 = Unbundle By Name(w2469) -> ("AB Cluster.Aiming Beam COM Port"=w2477:refnum<visa-resource-name>)
        n1160 = call-poly "VISA Configure Serial Port"("VISA resource name"=w2477, "Enable Termination\nChar (T)"=TRUE ("Enable Termination\nChar (T)"), "baud rate (9600)"=u32 9600, "error in (no error)"=w2474) -> ("error out"=w2473:errorcluster)  [unwired: 10 in, 1 out]
        n1161 = Unbundle By Name(w2473) -> ("status"=w2472:bool)
        n1162 = Not(x=w2472) -> (.not. x?=w2471:bool)
        n1163 = Bundle By Name(cluster=w2469, "System Status.Aiming Beam"=w2471) -> (w2470:T23)
        n1164 = call <vilib>:"Add State(s) to Queue__JKI_lib_State_Machine.vi"("State(s) in (\"\")"=w2479) -> ("States Out"=w2478:string)  [unwired: 14 in]
      }
      frame "AimingBeam: Close" {
        # "Close Aiming Beam COM port\n(Require USB connection to Aiming Beam Laser)"
        n1165 = Unbundle By Name(w2482) -> ("AB Cluster.Aiming Beam COM Port"=w2486:refnum<visa-resource-name>)
        n1166 = VISA Close(VISA resource name=w2486, error in (no error)=w2484) -> (error out=w2485:errorcluster)
        n1167 = Bundle By Name(cluster=w2482, "System Status.Aiming Beam"=FALSE) -> (w2483:T23)
        n1168 = call <vilib>:"Add State(s) to Queue__JKI_lib_State_Machine.vi"("State(s) in (\"\")"=w2488) -> ("States Out"=w2487:string)  [unwired: 14 in]
      }
      frame "AimingBeam: Set Current" {
        # "Set Aiming Beam Current\n(You can make a copy of, or modify, this frame)"
        n1169 = Unbundle By Name(w2503) -> ("AB Cluster.Aiming Beam COM Port"=w2496:refnum<visa-resource-name>, "AB Cluster.Max Current"=w2492:dbl, "AB Cluster.Default Current"=w2494:dbl, "AB Cluster.Min Current"=w2493:dbl)
        n1170 = In Range and Coerce(upper limit=w2492, x=w2494, lower limit=w2493) -> (coerced(x)=w2489:dbl)  [unwired: 1 out]
        n1171 = Number To Fractional String(number=w2489, precision (6)=i16 2) -> (F-format string=w2497:string)  [unwired: 2 in]
        n1172 = Concatenate Strings("slc:", w2497, "\r" ("Carriage Return Constant"), "\n" ("Line Feed Constant")) -> (w2500:string)
        n1173 = VISA Write(VISA resource name=w2496, write buffer=w2500, error in (no error)=w2491) -> (error out=w2495:errorcluster)  [unwired: 2 out]
        n1174 = call <vilib>:"Add State(s) to Queue__JKI_lib_State_Machine.vi"("State(s) in (\"\")"=w2505) -> ("States Out"=w2504:string)  [unwired: 14 in]
      }
      frame "AimingBeam: Set ACC Status" {
        # "Enable Aiming Beam\n(Usage: \"AimingBeam: Set >> Enable|Disable\")"
        n1175 = Unbundle By Name(w2512) -> ("AB Cluster.Aiming Beam COM Port"=w2509:refnum<visa-resource-name>)
        n1176 = case shown="\"Enable\"" w2511 {
          tunnel: [w2515 w2519] -> w2510
          frame "Disable", Default {
            n1177 = Concatenate Strings("cof", "\r" ("Carriage Return Constant"), "\n" ("Line Feed Constant")) -> (w2515:string)
          }
          frame "Enable" {
            n1178 = Concatenate Strings("con", "\r" ("Carriage Return Constant"), "\n" ("Line Feed Constant")) -> (w2519:string)
          }
        }
        n1179 = VISA Write(VISA resource name=w2509, write buffer=w2510, error in (no error)=w2507) -> (error out=w2508:errorcluster)  [unwired: 2 out]
        n1180 = call <vilib>:"Add State(s) to Queue__JKI_lib_State_Machine.vi"("State(s) in (\"\")"=w2514) -> ("States Out"=w2513:string)  [unwired: 14 in]
      }
      frame "AimingBeam: Set APC Status" {
        # "Enable Aiming Beam\n(Usage: \"AimingBeam: Set >> Enable|Disable\")"
        n1181 = Unbundle By Name(w2529) -> ("AB Cluster.Aiming Beam COM Port"=w2526:refnum<visa-resource-name>)
        n1182 = case shown="\"Disable\", Default" w2528 {
          tunnel: [w2532 w2536] -> w2527
          frame "Disable", Default {
            n1183 = Concatenate Strings("lof", "\r" ("Carriage Return Constant"), "\n" ("Line Feed Constant")) -> (w2532:string)
          }
          frame "Enable" {
            n1184 = Concatenate Strings("lon", "\r" ("Carriage Return Constant"), "\n" ("Line Feed Constant")) -> (w2536:string)
          }
        }
        n1185 = VISA Write(VISA resource name=w2526, write buffer=w2527, error in (no error)=w2524) -> (error out=w2525:errorcluster)  [unwired: 2 out]
        n1186 = call <vilib>:"Add State(s) to Queue__JKI_lib_State_Machine.vi"("State(s) in (\"\")"=w2531) -> ("States Out"=w2530:string)  [unwired: 14 in]
      }
      frame "AimingBeam: GetPWMStatus" {
        # "Get aiming beam PWM status\n()"
        n1187 = Unbundle By Name(w2544) -> ("AB Cluster.Freq"=w2543:i32, "LJ Pinout.AimingBeam PWM"=w2550:string)
        n1188 = Equal To 0?(x=w2543) -> (x = 0?=w2542:bool)
        n1189 = call "LabJack_FGV.vi"("Operation(Read)"=enum16{"Write", "Read"}."Read" ("Operation"), "error in (no error)"=w2546) -> ("error out"=w2548:errorcluster, "Read data"=w2549:i32)  [unwired: 8 in]
        n1190 = case shown="True" w2542 {
          tunnel: w2550 -> [w2563 _]
          tunnel: [w2561 "DIO_STATE"] -> w2547
          frame False {
            n1191 = Concatenate Strings(w2563, "_EF_ENABLE" ("string")) -> (w2561:string)
          }
          frame True {
          }
        }
        n1192 = call "LJM_eReadName.vi"("Handle In"=w2549, "Name"=w2547, "error in"=w2548) -> ("Value"=w2541:dbl, "error out"=w2545:errorcluster)  [unwired: 10 in, 1 out]
        n1193 = case shown="True" w2542 {
          tunnel: w2541 -> [w2556 w2560]
          tunnel: [w2555 w2557] -> w2540
          frame False {
            n1194 = Greater Than 0?(x=w2556) -> (x > 0?=w2555:bool)
          }
          frame True {
            n1195 = Number To Boolean Array(number=w2560) -> (Boolean array=w2559:bool[])
            n1196 = Index Array(array=w2559, index=3) -> (element=w2557:bool)
          }
        }
        n1197 = case shown="False" w2540 {
          frame False {
            # "PWM is off\nset color to dark green"
            n1198 = local write "Aiming beam toggle"(FALSE ("Aimging beam")) -> ()
          }
          frame True {
            # "PWM is on\nset color to light green"
            n1199 = local write "Aiming beam toggle"(TRUE ("Aimging beam")) -> ()
          }
        }
        n1200 = call <vilib>:"Add State(s) to Queue__JKI_lib_State_Machine.vi"("State(s) in (\"\")"=w2554) -> ("States Out"=w2553:string)  [unwired: 14 in]
      }
      frame "---------- 355 Laser ----------" {
        # "Template Separator\n(You can make a copy of, or modify, this frame)"
        n1201 = call <vilib>:"Add State(s) to Queue__JKI_lib_State_Machine.vi"("State(s) in (\"\")"=w2571) -> ("States Out"=w2570:string)  [unwired: 14 in]
      }
      frame "355 Laser: Check Dewelling" {
        # "if time laser start time is less than 7.5s before, wait 250ms then check again."
        # "Template Separator\n(You can make a copy of, or modify, this frame)"
        n1202 = Unbundle By Name(w2579) -> ("Laser start tic"=w2576:u32)
        n1203 = Tick Count (ms)() -> (millisecond timer value=w2577:u32)
        n1204 = Subtract(x=w2577, y=w2576) -> (x-y=w2575:u32)
        n1205 = Greater?(x=w2575, y=u32 5000) -> (0:w2573:bool)
        n1206 = case shown="False" w2573 {
          tunnel: ["355 Laser: Check Dewelling" ""] -> w2572
          frame False {
            n1207 = Wait (ms)(milliseconds to wait=u32 250) -> ()  [unwired: 1 out]
          }
          frame True {
          }
        }
        n1208 = call <vilib>:"Add State(s) to Queue__JKI_lib_State_Machine.vi"("State(s) in Front (\"\")"=w2572, "State(s) in (\"\")"=w2582) -> ("States Out"=w2581:string)  [unwired: 13 in]
      }
      frame "355 Laser: Laser enable" {
        # "Laser enable/disable\n(Usage: \"LabJack: Laser enable/disable >> 1|0\")"
        n1209 = Unbundle By Name(w2589) -> ("LJ Pinout.Laser Start/Stop"=w2593:string, "System Status.355 Laser"=w2587:bool)
        n1210 = case shown="False" w2587 {
          tunnel: w2586 -> [w2608 w2609]
          tunnel: w2593 -> [w2602 _]
          tunnel: [w2597 w2609] -> w2591
          tunnel: [w2596 u32 0 ("millisecond timer value")] -> w2588
          frame False {
            n1211 = call "LabJack_FGV.vi"("Operation(Read)"=enum16{"Write", "Read"}."Read" ("Operation")) -> ("Read data"=w2604:i32)  [unwired: 9 in, 1 out]
            n1212 = call "LJM_eWriteName.vi"("Handle In"=w2604, "Name"=w2602, "Value"=1.0, "error in"=w2608) -> ("Handle Out"=w2603:i32, "error out"=w2601:errorcluster)  [unwired: 10 in]
            n1213 = call <userlib>:"Wait (ms)__ogtk.vi"("error in (no error)"=w2601, "milliseconds to wait"=u32 250) -> ("error out"=w2600:errorcluster)  [unwired: 8 in, 1 out]
            n1214 = call "LJM_eWriteName.vi"("Handle In"=w2603, "Name"=w2602, "Value"=0.0, "error in"=w2600) -> ("error out"=w2598:errorcluster)  [unwired: 10 in, 1 out]
            n1215 = call <userlib>:"Tick Count (ms)__ogtk.vi"("error in (no error)"=w2598) -> ("error out"=w2597:errorcluster, "millisecond timer value"=w2596:u32)  [unwired: 9 in]
          }
          frame True {
          }
        }
        n1216 = Bundle By Name(cluster=w2589, "Laser start tic"=w2588) -> (w2590:T23)
        n1217 = call <vilib>:"Add State(s) to Queue__JKI_lib_State_Machine.vi"("State(s) in (\"\")"=w2595) -> ("States Out"=w2594:string)  [unwired: 14 in]
      }
      frame "355 Laser: Laser disable" {
        # "Laser enable/disable\n(Usage: \"LabJack: Laser enable/disable >> 1|0\")"
        n1218 = Unbundle By Name(w2613) -> ("LJ Pinout.Laser Start/Stop"=w2617:string, "System Status.355 Laser"=w2611:bool)
        n1219 = case shown="True" w2611 {
          tunnel: w2618 -> [w2621 w2635]
          tunnel: w2617 -> [_ w2629]
          tunnel: [w2621 w2624] -> w2615
          tunnel: [u32 0 ("millisecond timer value") w2623] -> w2612
          frame False {
          }
          frame True {
            n1220 = call "LabJack_FGV.vi"("Operation(Read)"=enum16{"Write", "Read"}."Read" ("Operation")) -> ("Read data"=w2631:i32)  [unwired: 9 in, 1 out]
            n1221 = call "LJM_eWriteName.vi"("Handle In"=w2631, "Name"=w2629, "Value"=1.0, "error in"=w2635) -> ("Handle Out"=w2630:i32, "error out"=w2628:errorcluster)  [unwired: 10 in]
            n1222 = call <userlib>:"Wait (ms)__ogtk.vi"("error in (no error)"=w2628, "milliseconds to wait"=u32 250) -> ("error out"=w2627:errorcluster)  [unwired: 8 in, 1 out]
            n1223 = call "LJM_eWriteName.vi"("Handle In"=w2630, "Name"=w2629, "Value"=0.0, "error in"=w2627) -> ("error out"=w2625:errorcluster)  [unwired: 10 in, 1 out]
            n1224 = call <userlib>:"Tick Count (ms)__ogtk.vi"("error in (no error)"=w2625) -> ("error out"=w2624:errorcluster, "millisecond timer value"=w2623:u32)  [unwired: 9 in]
          }
        }
        n1225 = Bundle By Name(cluster=w2613, "Laser start tic"=w2612) -> (w2614:T23)
        n1226 = call <vilib>:"Add State(s) to Queue__JKI_lib_State_Machine.vi"("State(s) in (\"\")"=w2620) -> ("States Out"=w2619:string)  [unwired: 14 in]
      }
      frame "355 Laser: Dewelling" {
        # "Wait some time (ms)\n(355 Laser: Dewelling >> #)"
        n1227 = Fract/Exp String To Number(string=w2639, default (0 dbl)=0) -> (number=w2637:i32)  [unwired: 2 in, 1 out]
        n1228 = Wait (ms)(milliseconds to wait=w2637) -> ()  [unwired: 1 out]
        n1229 = call <vilib>:"Add State(s) to Queue__JKI_lib_State_Machine.vi"("State(s) in (\"\")"=w2643) -> ("States Out"=w2642:string)  [unwired: 14 in]
      }
      frame "355 Laser: Close" {
        # "Template Separator\n(You can make a copy of, or modify, this frame)"
        n1230 = call <vilib>:"Add State(s) to Queue__JKI_lib_State_Machine.vi"("State(s) in Front (\"\")"="355 Laser: CheckControllerStatus\n355 Laser: Laser disable\n355 Laser: Dewelling >>1000", "State(s) in (\"\")"=w2649) -> ("States Out"=w2648:string)  [unwired: 13 in]
      }
      frame "355 Laser: CheckControllerStatus" {
        # "if average < 2, laser no power\nif average 2 < average < 9.3, laser on\nif 9.3<average<10, interlock open, blink indicator\nif average > 10, laser off\n[Covers: REQ30]"
        # "take 10 measuremt and look at average"
        # "Check 355 laser controller status\nBy probing Emisison Lamp negative terminal voltage"
        n1231 = Unbundle By Name(w2658) -> ("LJ Pinout.Laser Ready"=w2661:string)
        n1232 = call "LabJack_FGV.vi"("Operation(Read)"=enum16{"Write", "Read"}."Read" ("Operation")) -> ("Read data"=w2662:i32)  [unwired: 9 in, 1 out]
        n1233 = for {
          N: 20 -> [_]
          tunnel: w2662 -> [w2673]
          tunnel: w2661 -> [w2672]
          shift-right: [w2671] -> w2654
          shift-left: w2660 -> [w2670]
          tunnel: [w2668] -> w2653 mode=indexing
          n1234 = call "LJM_eReadName.vi"("Handle In"=w2673, "Name"=w2672, "error in"=w2670) -> ("Value"=w2668:dbl, "error out"=w2671:errorcluster)  [unwired: 10 in, 1 out]
          n1235 = Wait (ms)(milliseconds to wait=u32 25) -> ()  [unwired: 1 out]
        }
        n1236 = call "checkLaserStatus.vi"("error in (no error)"=w2654, "Laser LED voltage"=w2653) -> ("error out"=w2655:errorcluster, "Interlock open?"=w2650:bool, "Laser on?"=w2652:bool, "Mean voltage"=→"laser EM lamp V":dbl)  [unwired: 6 in]
        n1237 = Bundle By Name(cluster=w2658, "System Status.355 Laser"=w2652) -> (w2659:T23)
        n1238 = case shown="True" w2650 {
          frame False {
            n1239 = property on="355 Laser" class="Bool (strict)"("Blinking"=FALSE) -> ()  [unwired: 2 in, 2 out]
          }
          frame True {
            n1240 = property on="355 Laser" class="Bool (strict)"("Blinking"=TRUE) -> ()  [unwired: 2 in, 2 out]
          }
        }
        n1241 = call <vilib>:"Add State(s) to Queue__JKI_lib_State_Machine.vi"("State(s) in (\"\")"=w2665) -> ("States Out"=w2664:string)  [unwired: 14 in]
      }
      frame "355 Laser: CheckPWMStatus" {
        # "Check 355 laser PWM status\n(Read LJ DIO#EF_ENABLE register to determine PWM status)"
        n1242 = Unbundle By Name(w2683) -> ("LJ Pinout.355 PWM"=w2682:string)
        n1243 = call "LabJack_FGV.vi"("Operation(Read)"=enum16{"Write", "Read"}."Read" ("Operation"), "error in (no error)"=w2676) -> ("error out"=w2679:errorcluster, "Read data"=w2680:i32)  [unwired: 8 in]
        n1244 = Concatenate Strings(w2682, "_EF_ENABLE" ("string")) -> (w2678:string)
        n1245 = call "LJM_eReadName.vi"("Handle In"=w2680, "Name"=w2678, "error in"=w2679) -> ("Value"=w2675:dbl, "error out"=w2677:errorcluster)  [unwired: 10 in, 1 out]
        n1246 = Greater Than 0?(x=w2675) -> (x > 0?=w2674:bool)
        n1247 = case shown="False" w2674 {
          frame False {
            # "PWM is off\nset color to gray"
            n1248 = local write "355nm Laser toggle"(FALSE ("355nm Laser")) -> ()
          }
          frame True {
            # "PWM is on\nset color to light green"
            n1249 = local write "355nm Laser toggle"(TRUE ("355nm Laser")) -> ()
          }
        }
        n1250 = call <vilib>:"Add State(s) to Queue__JKI_lib_State_Machine.vi"("State(s) in (\"\")"=w2687) -> ("States Out"=w2686:string)  [unwired: 14 in]
      }
      frame "355 Laser: Start" {
        # "Template Separator\n(You can make a copy of, or modify, this frame)"
        n1251 = call <vilib>:"Add State(s) to Queue__JKI_lib_State_Machine.vi"("State(s) in Front (\"\")"="LabJack: 355_PWM_Start", "State(s) in (\"\")"=w2695) -> ("States Out"=w2694:string)  [unwired: 13 in]
      }
      frame "355 Laser: Stop" {
        # "Template Separator\n(You can make a copy of, or modify, this frame)"
        n1252 = call <vilib>:"Add State(s) to Queue__JKI_lib_State_Machine.vi"("State(s) in Front (\"\")"="LabJack: 355_PWM_Stop", "State(s) in (\"\")"=w2701) -> ("States Out"=w2700:string)  [unwired: 13 in]
      }
      frame "---------- Utility ----------" {
        # "Template Separator\n(You can make a copy of, or modify, this frame)"
        n1253 = call <vilib>:"Add State(s) to Queue__JKI_lib_State_Machine.vi"("State(s) in (\"\")"=w2706) -> ("States Out"=w2705:string)  [unwired: 14 in]
      }
      frame "Utility: SetDataClass" {
        # "Set Data Class in Queues\n(Set data class to either Data, Bg or Cali)"
        n1254 = case shown="\"Cali\"" w2708 {
          tunnel: [enum16{"Data", "BG", "Cali"}."Data" ("Data Class") enum16{"Data", "BG", "Cali"}."BG" ("Data Class") enum16{"Data", "BG", "Cali"}."Cali" ("Data Class")] -> w2707
          frame "Data", Default {
          }
          frame "Bg" {
          }
          frame "Cali" {
          }
        }
        n1255 = local write "Data Class"(w2707) -> ()
        n1256 = call <vilib>:"Add State(s) to Queue__JKI_lib_State_Machine.vi"("State(s) in (\"\")"=w2713) -> ("States Out"=w2712:string)  [unwired: 14 in]
      }
      frame "Utility: AquiTimerReset" {
        # "Set Aquisition Timer\n(You can make a copy of, or modify, this frame)"
        n1257 = Tick Count (ms)() -> (millisecond timer value=w2719:u32)
        n1258 = Bundle By Name(cluster=w2717, "Aquisition Timer"=w2719) -> (w2718:T23)
        n1259 = call <vilib>:"Add State(s) to Queue__JKI_lib_State_Machine.vi"("State(s) in (\"\")"=w2723) -> ("States Out"=w2722:string)  [unwired: 14 in]
      }
      frame "Utility: AquiTimerCheck" {
        # "5min to ms"
        # "Set Aquisition Timer\n([Covers: REQ35])"
        n1260 = Unbundle By Name(w2731) -> ("Aquisition Timer"=w2729:u32)
        n1261 = Tick Count (ms)() -> (millisecond timer value=w2730:u32)
        n1262 = Subtract(x=w2730, y=w2729) -> (x-y=w2728:u32)
        n1263 = Multiply(x=1000, y=300) -> (x*y=w2725:i32)
        n1264 = Greater Or Equal?(x=w2728, y=w2725) -> (x >= y?=w2724:bool)
        n1265 = case shown="True" w2724 {
          frame False {
            # "do nothing"
          }
          frame True {
            # "if timed out, stop aquisition"
            n1266 = property on="StopButton" class="Bool (strict)"("Val(Sgnl)"=TRUE ("Value (Signaling)")) -> ()  [unwired: 2 in, 2 out]
          }
        }
        n1267 = call <vilib>:"Add State(s) to Queue__JKI_lib_State_Machine.vi"("State(s) in (\"\")"=w2735) -> ("States Out"=w2734:string)  [unwired: 14 in]
      }
      frame "Utility: StartBeep" {
        # "Beep\n([Covers: REQ18])"
        n1268 = call <vilib>:"Beep.vi"("use system alert? (T)"=FALSE, "duration (msec)"=u32 1000, "frequency (Hz)"=u32 2000) -> ()  [unwired: 9 in]
        n1269 = call <vilib>:"Add State(s) to Queue__JKI_lib_State_Machine.vi"("State(s) in (\"\")"=w2744) -> ("States Out"=w2743:string)  [unwired: 14 in]
      }
      frame "Utility: EndBeep" {
        # "Beep\n([Covers: REQ18])"
        n1270 = flat-sequence {
          frame #0 {
            n1271 = call <vilib>:"Beep.vi"("use system alert? (T)"=FALSE, "duration (msec)"=u32 500, "frequency (Hz)"=u32 2000) -> ()  [unwired: 9 in]
          }
          frame #1 {
            n1272 = call <vilib>:"Beep.vi"("use system alert? (T)"=FALSE, "duration (msec)"=u32 500, "frequency (Hz)"=u32 2000) -> ()  [unwired: 9 in]
          }
        }
        n1273 = call <vilib>:"Add State(s) to Queue__JKI_lib_State_Machine.vi"("State(s) in (\"\")"=w2749) -> ("States Out"=w2748:string)  [unwired: 14 in]
      }
      frame "Utility: RestoreDeConChan" {
        # "Template Separator\n(You can make a copy of, or modify, this frame)"
        n1274 = global read "GlobalVariables.vi" "DeconChan Temp"() -> (w2756:T9)
        n1275 = local write "Radio Buttons"(w2756) -> ()
        n1276 = call <vilib>:"Add State(s) to Queue__JKI_lib_State_Machine.vi"("State(s) in (\"\")"=w2761) -> ("States Out"=w2760:string)  [unwired: 14 in]
      }
      frame "Utility: SaveDeconChan" {
        # "Save Decon Channel to global temp\n(You can make a copy of, or modify, this frame)"
        n1277 = flat-sequence {
          frame #0 {
            n1278 = local read "Radio Buttons"() -> (w2767:T9)
            n1279 = global write "GlobalVariables.vi" "DeconChan Temp"(w2767) -> ()
          }
          frame #1 {
            n1280 = local write "Radio Buttons"(T9."No Selection" ("Radio Buttons")) -> ()
          }
        }
        n1281 = flat-sequence {
          frame #0 {
          }
          frame #1 {
            (unwired) enum32{"No Selection", "Ch1", "Ch2", "Ch3"}."No Selection" ("Radio Buttons")
          }
        }
        n1282 = call <vilib>:"Add State(s) to Queue__JKI_lib_State_Machine.vi"("State(s) in (\"\")"=w2766) -> ("States Out"=w2765:string)  [unwired: 14 in]
      }
      frame "Utility: Dewelling" {
        # "Main loop dewell\n(Dewelling >> #)"
        n1283 = Fract/Exp String To Number(string=w2772, default (0 dbl)=0) -> (number=w2770:i32)  [unwired: 2 in, 1 out]
        n1284 = Wait (ms)(milliseconds to wait=w2770) -> ()  [unwired: 1 out]
        n1285 = call <vilib>:"Add State(s) to Queue__JKI_lib_State_Machine.vi"("State(s) in (\"\")"=w2776) -> ("States Out"=w2775:string)  [unwired: 14 in]
      }
      frame "Utility: SetAllChanManualGain" {
        w2777 = FALSE ("Value (Signaling)")
        # "Set all channel to manual gain\n(You can make a copy of, or modify, this frame)"
        n1286 = property on="Auto gain ch1" class="Bool (strict)"("Val(Sgnl)"=w2777) -> ()  [unwired: 2 in, 2 out]
        n1287 = property on="Auto gain ch2" class="Bool (strict)"("Val(Sgnl)"=w2777) -> ()  [unwired: 2 in, 2 out]
        n1288 = property on="Auto gain ch3" class="Bool (strict)"("Val(Sgnl)"=w2777) -> ()  [unwired: 2 in, 2 out]
        n1289 = property on="Auto gain ch4" class="Bool (strict)"("Val(Sgnl)"=w2777) -> ()  [unwired: 2 in, 2 out]
        n1290 = call <vilib>:"Add State(s) to Queue__JKI_lib_State_Machine.vi"("State(s) in (\"\")"=w2782) -> ("States Out"=w2781:string)  [unwired: 14 in]
      }
      frame "Utility: SetAllChanAutoGain" {
        w2783 = TRUE ("Value (Signaling)")
        # "Set all channels to auto gain\n(You can make a copy of, or modify, this frame)"
        n1291 = property on="Auto gain ch1" class="Bool (strict)"("Val(Sgnl)"=w2783) -> ()  [unwired: 2 in, 2 out]
        n1292 = property on="Auto gain ch2" class="Bool (strict)"("Val(Sgnl)"=w2783) -> ()  [unwired: 2 in, 2 out]
        n1293 = property on="Auto gain ch3" class="Bool (strict)"("Val(Sgnl)"=w2783) -> ()  [unwired: 2 in, 2 out]
        n1294 = property on="Auto gain ch4" class="Bool (strict)"("Val(Sgnl)"=w2783) -> ()  [unwired: 2 in, 2 out]
        n1295 = call <vilib>:"Add State(s) to Queue__JKI_lib_State_Machine.vi"("State(s) in (\"\")"=w2788) -> ("States Out"=w2787:string)  [unwired: 14 in]
      }
      frame "---------- SysLog ----------" {
        # "Template Separator\n(You can make a copy of, or modify, this frame)"
        n1296 = call <vilib>:"Add State(s) to Queue__JKI_lib_State_Machine.vi"("State(s) in (\"\")"=w2793) -> ("States Out"=w2792:string)  [unwired: 14 in]
      }
      frame "SysLog: OpenLogFile" {
        # "Template Separator\n(You can make a copy of, or modify, this frame)"
        n1297 = call <vilib>:"Add State(s) to Queue__JKI_lib_State_Machine.vi"("State(s) in (\"\")"=w2798) -> ("States Out"=w2797:string)  [unwired: 14 in]
      }
      frame "---------- Graph ----------" {
        # "Template Separator\n(You can make a copy of, or modify, this frame)"
        n1298 = call <vilib>:"Add State(s) to Queue__JKI_lib_State_Machine.vi"("State(s) in (\"\")"=w2803) -> ("States Out"=w2802:string)  [unwired: 14 in]
      }
      frame "Graph: SetXMultiplier" {
        # "Set X multiplier of WF graphs\n(You can make a copy of, or modify, this frame)"
        n1299 = call "Digitizer1_FGV.vi"() -> ("error out"=w2807:errorcluster, "Read data"=w2808:refnum<k15>)  [unwired: 10 in]
        n1300 = property class="niScope"(reference=w2808, error in=w2807) -> ("Min Sample Rate"=w2806:dbl)  [unwired: 2 out]
        n1301 = Divide(x=1.0, y=w2806) -> (x/y=w2804:dbl)
        n1302 = property on="Channel 1" class="WFGraph (strict)"("XScale.Multiplier"=w2804) -> ()  [unwired: 2 in, 2 out]
        n1303 = property on="Channel 2" class="WFGraph (strict)"("XScale.Multiplier"=w2804) -> ()  [unwired: 2 in, 2 out]
        n1304 = property on="Channel 3" class="WFGraph (strict)"("XScale.Multiplier"=w2804) -> ()  [unwired: 2 in, 2 out]
        n1305 = property on="Channel 4" class="WFGraph (strict)"("XScale.Multiplier"=w2804) -> ()  [unwired: 2 in, 2 out]
        n1306 = call <vilib>:"Add State(s) to Queue__JKI_lib_State_Machine.vi"("State(s) in (\"\")"=w2813) -> ("States Out"=w2812:string)  [unwired: 14 in]
      }
      frame "Graph: AddCursors" {
        # "Add BG and DC cursor to all graphs\n(You can make a copy of, or modify, this frame)"
        n1307 = property on="Channel 1" class="WFGraph (strict)"() -> ("XScale.Multiplier"=w2822:dbl)  [unwired: 2 in, 2 out]
        n1308 = global read "GlobalVariables.vi" "DC Idx1"() -> (w2821:i32)
        n1309 = global read "GlobalVariables.vi" "DC Idx2"() -> (w2820:i32)
        n1310 = global read "GlobalVariables.vi" "BG Idx1"() -> (w2819:i32)
        n1311 = global read "GlobalVariables.vi" "BG Idx2"() -> (w2818:i32)
        n1312 = property on="Channel 1" class="WFGraph (strict)"(error in=w2824) -> ("CrsrList"=w2833:T24)  [unwired: 1 in, 2 out]
        n1313 = property on="Channel 2" class="WFGraph (strict)"() -> ("CrsrList"=w2830:T24)  [unwired: 2 in, 2 out]
        n1314 = property on="Channel 3" class="WFGraph (strict)"() -> ("CrsrList"=w2829:T24)  [unwired: 2 in, 2 out]
        n1315 = property on="Channel 4" class="WFGraph (strict)"() -> ("CrsrList"=w2815:T24)  [unwired: 2 in, 2 out]
        n1316 = Build Array(w2821, w2820, w2819, w2818) -> (w2817:i32[])
        n1317 = Multiply(x=w2817, y=w2822) -> (x*y=w2816:dbl[])
        n1318 = for {
          tunnel: w2833 -> [w2847] mode=indexing
          tunnel: w2816 -> [w2840] mode=indexing
          tunnel: [w2846] -> w2832 mode=indexing
          tunnel: u32[] [6618880, 6618880, 16711680, 16711680] -> [w2839] mode=indexing
          tunnel: w2830 -> [w2845] mode=indexing
          tunnel: w2829 -> [w2844] mode=indexing
          tunnel: [w2843] -> w2828 mode=indexing
          tunnel: [w2842] -> w2827 mode=indexing
          tunnel: w2815 -> [w2841] mode=indexing
          tunnel: [w2838] -> w2814 mode=indexing
          n1319 = Bundle By Name(cluster=w2847, "Position.X"=w2840, "Color"=w2839) -> (w2846:T25)
          n1320 = Bundle By Name(cluster=w2845, "Position.X"=w2840, "Color"=w2839) -> (w2843:T25)
          n1321 = Bundle By Name(cluster=w2844, "Position.X"=w2840, "Color"=w2839) -> (w2842:T25)
          n1322 = Bundle By Name(cluster=w2841, "Position.X"=w2840, "Color"=w2839) -> (w2838:T25)
        }
        n1323 = property on="Channel 1" class="WFGraph (strict)"("CrsrList"=w2832) -> (error out=w2823:errorcluster)  [unwired: 2 in, 1 out]
        n1324 = property on="Channel 2" class="WFGraph (strict)"("CrsrList"=w2828) -> ()  [unwired: 2 in, 2 out]
        n1325 = property on="Channel 3" class="WFGraph (strict)"("CrsrList"=w2827) -> ()  [unwired: 2 in, 2 out]
        n1326 = property on="Channel 4" class="WFGraph (strict)"("CrsrList"=w2814) -> ()  [unwired: 2 in, 2 out]
        n1327 = control-ref of="Channel 1"() -> (w2826:refnum<vi>)
        n1328 = call <vilib>:"Add State(s) to Queue__JKI_lib_State_Machine.vi"("State(s) in (\"\")"=w2837) -> ("States Out"=w2836:string)  [unwired: 14 in]
        n1329 = call "UpdateCurserIdx(SubVI).vi"("error in (no error)"=w2823, "WaveformGraph in"=w2826) -> ("error out"=w2825:errorcluster)  [unwired: 9 in]
      }
      frame "Graph: SaveCursorLoc" {
        # "Save cursor location to ini file\n(Save cursor location to system setting ini file)"
        n1330 = global read "GlobalVariables.vi" "DC Idx1"() -> (w2854:i32)
        n1331 = global read "GlobalVariables.vi" "DC Idx2"() -> (w2853:i32)
        n1332 = global read "GlobalVariables.vi" "BG Idx1"() -> (w2852:i32)
        n1333 = global read "GlobalVariables.vi" "BG Idx2"() -> (w2851:i32)
        n1334 = Bundle("DC Idx1"=w2854, "DC Idx2"=w2853, "BG Idx1"=w2852, "BG Idx2"=w2851) -> (w2850:T47)  [unwired: 1 in]
        n1335 = call "writeCursorConfigMain.vi"("error in (no error)"=w2848, "Cursor Locations"=w2850) -> ("error out"=w2849:errorcluster)  [unwired: 9 in]
        n1336 = call <vilib>:"Add State(s) to Queue__JKI_lib_State_Machine.vi"("State(s) in (\"\")"=w2858) -> ("States Out"=w2857:string)  [unwired: 14 in]
      }
      frame "---------- APD ----------" {
        # "Template Separator\n(You can make a copy of, or modify, this frame)"
        n1337 = call <vilib>:"Add State(s) to Queue__JKI_lib_State_Machine.vi"("State(s) in (\"\")"=w2863) -> ("States Out"=w2862:string)  [unwired: 14 in]
      }
      frame "APD: Initialize" {
        w2870 = enum16{"Read", "Write"}."Write" ("Operation (Read)")
        w2869 = refnum<class "APDClass.lvclass"> refnum  # APDClass.lvclass
        # "Initialize APD FGV\n(Initialized APD FGV for holding data)"
        n1338 = call "APD1FGV.vi"("Error In"=w2864, "Operation (Read)"=w2870, "APDClass in"=w2869) -> ("Error Out"=w2868:errorcluster)  [unwired: 7 in, 1 out]
        n1339 = call "APD2FGV.vi"("Error In"=w2864, "Operation (Read)"=w2870, "APDClass in"=w2869) -> ("Error Out"=w2867:errorcluster)  [unwired: 7 in, 1 out]
        n1340 = call "APD3FGV.vi"("Error In"=w2864, "Operation (Read)"=w2870, "APDClass in"=w2869) -> ("Error Out"=w2866:errorcluster)  [unwired: 7 in, 1 out]
        n1341 = Merge Errors(w2868, w2867, w2866) -> (w2865:errorcluster)
        n1342 = call <vilib>:"Add State(s) to Queue__JKI_lib_State_Machine.vi"("State(s) in (\"\")"=w2874) -> ("States Out"=w2873:string)  [unwired: 14 in]
      }
      frame "APD: LoadFromSerial" {
        w2876 = enum16{"Read", "Write"}."Write" ("Operation (Read)")
        # "Load APD data from tdms file\n(load and update FGV)"
        n1343 = call "readAPDSerial.vi"("Error In"=w2883) -> ("Error Out"=w2879:errorcluster, "output cluster"=w2882:T26)  [unwired: 9 in]
        n1344 = Unbundle By Name(w2882) -> ("Ch1APDSerial#"=w2895:string, "Ch2APDSerial#"=w2881:string, "Ch3APDSerial#"=w2894:string, "Ch4APDSerial#"=w2880:string)
        n1345 = call "CreatFromSerialNumNoRaw.vi"("error in (no error)"=w2879, "APD Serial #"=w2895) -> ("error out"=w2892:errorcluster, "APDClass out"=w2893:refnum<class "APDClass.lvclass">)  [unwired: 8 in]
        n1346 = call "CreatFromSerialNumNoRaw.vi"("error in (no error)"=w2879, "APD Serial #"=w2881) -> ("error out"=w2890:errorcluster, "APDClass out"=w2891:refnum<class "APDClass.lvclass">)  [unwired: 8 in]
        n1347 = call "CreatFromSerialNumNoRaw.vi"("error in (no error)"=w2879, "APD Serial #"=w2894) -> ("error out"=w2888:errorcluster, "APDClass out"=w2889:refnum<class "APDClass.lvclass">)  [unwired: 8 in]
        n1348 = call "CreatFromSerialNumNoRaw.vi"("error in (no error)"=w2879, "APD Serial #"=w2880) -> ("error out"=w2877:errorcluster, "APDClass out"=w2878:refnum<class "APDClass.lvclass">)  [unwired: 8 in]
        n1349 = call "APD1FGV.vi"("Error In"=w2892, "Operation (Read)"=w2876, "APDClass in"=w2893) -> ("Error Out"=w2887:errorcluster)  [unwired: 7 in, 1 out]
        n1350 = call "APD2FGV.vi"("Error In"=w2890, "Operation (Read)"=w2876, "APDClass in"=w2891) -> ("Error Out"=w2885:errorcluster)  [unwired: 7 in, 1 out]
        n1351 = call "APD3FGV.vi"("Error In"=w2888, "Operation (Read)"=w2876, "APDClass in"=w2889) -> ("Error Out"=w2886:errorcluster)  [unwired: 7 in, 1 out]
        n1352 = call "APD4FGV.vi"("Error In"=w2877, "Operation (Read)"=w2876, "APDClass in"=w2878) -> ("Error Out"=w2875:errorcluster)  [unwired: 7 in, 1 out]
        n1353 = Merge Errors(w2887, w2885, w2886, w2875) -> (w2884:errorcluster)
        n1354 = call <vilib>:"Add State(s) to Queue__JKI_lib_State_Machine.vi"("State(s) in (\"\")"=w2899) -> ("States Out"=w2898:string)  [unwired: 14 in]
      }
      frame "APD: UpdateCtrlVLimit" {
        w2905 = enum16{"Read", "Write"}."Read" ("Operation (Read)")
        # "Set V limit\n(You can make a copy of, or modify, this frame)"
        n1355 = call "APD1FGV.vi"("Error In"=w2906, "Operation (Read)"=w2905) -> ("Error Out"=w2921:errorcluster, "APDClass out"=w2922:refnum<class "APDClass.lvclass">)  [unwired: 8 in]
        n1356 = call "APD2FGV.vi"("Error In"=w2906, "Operation (Read)"=w2905) -> ("Error Out"=w2919:errorcluster, "APDClass out"=w2920:refnum<class "APDClass.lvclass">)  [unwired: 8 in]
        n1357 = call "APD3FGV.vi"("Error In"=w2906, "Operation (Read)"=w2905) -> ("Error Out"=w2917:errorcluster, "APDClass out"=w2918:refnum<class "APDClass.lvclass">)  [unwired: 8 in]
        n1358 = call "APD4FGV.vi"("Error In"=w2906, "Operation (Read)"=w2905) -> ("Error Out"=w2903:errorcluster, "APDClass out"=w2904:refnum<class "APDClass.lvclass">)  [unwired: 8 in]
        n1359 = call-dynamic "ReadMaxCtrlV.vi"("error in (no error)"=w2921, "APDClass in"=w2922) -> ("error out"=w2912:errorcluster, "Numeric"=w2915:dbl)  [unwired: 7 in, 1 out]
        n1360 = call-dynamic "ReadMaxCtrlV.vi"("error in (no error)"=w2919, "APDClass in"=w2920) -> ("error out"=w2910:errorcluster, "Numeric"=w2914:dbl)  [unwired: 7 in, 1 out]
        n1361 = call-dynamic "ReadMaxCtrlV.vi"("error in (no error)"=w2917, "APDClass in"=w2918) -> ("error out"=w2908:errorcluster, "Numeric"=w2913:dbl)  [unwired: 7 in, 1 out]
        n1362 = call-dynamic "ReadMaxCtrlV.vi"("error in (no error)"=w2903, "APDClass in"=w2904) -> ("error out"=w2901:errorcluster, "Numeric"=w2902:dbl)  [unwired: 7 in, 1 out]
        n1363 = property on="V 1" class="DigNum (strict)"(error in=w2912, "Maximum"=w2915) -> (error out=w2911:errorcluster)  [unwired: 1 in, 1 out]
        n1364 = property on="V 2" class="DigNum (strict)"(error in=w2910, "Maximum"=w2914) -> (error out=w2909:errorcluster)  [unwired: 1 in, 1 out]
        n1365 = property on="V 4" class="DigNum (strict)"(error in=w2901, "Maximum"=w2902) -> (error out=w2900:errorcluster)  [unwired: 1 in, 1 out]
        n1366 = property on="V 3" class="DigNum (strict)"(error in=w2908, "Maximum"=w2913) -> (error out=w2907:errorcluster)  [unwired: 1 in, 1 out]
        n1367 = Merge Errors(w2911, w2909, w2907, w2900) -> (w2916:errorcluster)
        n1368 = call <vilib>:"Add State(s) to Queue__JKI_lib_State_Machine.vi"("State(s) in (\"\")"=w2926) -> ("States Out"=w2925:string)  [unwired: 14 in]
      }
      frame "APD: GetGainLimits" {
        w2931 = enum16{"Read", "Write"}."Read" ("Operation (Read)")
        # "Template Separator\n(You can make a copy of, or modify, this frame)"
        n1369 = call "APD1FGV.vi"("Error In"=w2932, "Operation (Read)"=w2931) -> ("Error Out"=w2937:errorcluster, "APDClass out"=w2938:refnum<class "APDClass.lvclass">)  [unwired: 8 in]
        n1370 = call "APD2FGV.vi"("Error In"=w2932, "Operation (Read)"=w2931) -> ("Error Out"=w2944:errorcluster, "APDClass out"=w2945:refnum<class "APDClass.lvclass">)  [unwired: 8 in]
        n1371 = call "APD3FGV.vi"("Error In"=w2932, "Operation (Read)"=w2931) -> ("Error Out"=w2942:errorcluster, "APDClass out"=w2943:refnum<class "APDClass.lvclass">)  [unwired: 8 in]
        n1372 = call "APD4FGV.vi"("Error In"=w2932, "Operation (Read)"=w2931) -> ("Error Out"=w2929:errorcluster, "APDClass out"=w2930:refnum<class "APDClass.lvclass">)  [unwired: 8 in]
        n1373 = call-dynamic "Read Gain Limits(Log).vi"("error in (no error)"=w2937, "APDClass in"=w2938) -> ("error out"=w2936:errorcluster, "GainLimits(Log)"=w2933:cluster{"GainMax":dbl, "GainMin":dbl})  [unwired: 7 in, 1 out]
        n1374 = call-dynamic "Read Gain Limits(Log).vi"("error in (no error)"=w2944, "APDClass in"=w2945) -> ("error out"=w2940:errorcluster, "GainLimits(Log)"=w2935:cluster{"GainMax":dbl, "GainMin":dbl})  [unwired: 7 in, 1 out]
        n1375 = call-dynamic "Read Gain Limits(Log).vi"("error in (no error)"=w2942, "APDClass in"=w2943) -> ("error out"=w2939:errorcluster, "GainLimits(Log)"=w2934:cluster{"GainMax":dbl, "GainMin":dbl})  [unwired: 7 in, 1 out]
        n1376 = call-dynamic "Read Gain Limits(Log).vi"("error in (no error)"=w2929, "APDClass in"=w2930) -> ("error out"=w2927:errorcluster, "GainLimits(Log)"=w2928:cluster{"GainMax":dbl, "GainMin":dbl})  [unwired: 7 in, 1 out]
        n1377 = Merge Errors(w2936, w2940, w2939, w2927) -> (w2941:errorcluster)
        n1378 = global write "GlobalVariables.vi" "Ch1GainLim(Log)"(w2933) -> ()
        n1379 = global write "GlobalVariables.vi" "Ch2GainLim(Log)"(w2935) -> ()
        n1380 = global write "GlobalVariables.vi" "Ch3GainLim(Log)"(w2934) -> ()
        n1381 = global write "GlobalVariables.vi" "Ch4GainLim(Log)"(w2928) -> ()
        n1382 = call <vilib>:"Add State(s) to Queue__JKI_lib_State_Machine.vi"("State(s) in (\"\")"=w2949) -> ("States Out"=w2948:string)  [unwired: 14 in]
      }
      frame "---------- TCP ----------" {
        # "Template Separator\n(You can make a copy of, or modify, this frame)"
        n1383 = call <vilib>:"Add State(s) to Queue__JKI_lib_State_Machine.vi"("State(s) in (\"\")"=w2954) -> ("States Out"=w2953:string)  [unwired: 14 in]
      }
      frame "TCP: InitializeNew" {
        # "if unsuccessful and count <10, increament count \nand try again"
        # "Initialize TCP connection to aimging beam computer\n(You can make a copy of, or modify, this frame)"
        n1384 = TCP Create Listener(10:u16 2100 ("port"), 11:"RTLT" ("service name")) -> (0:w2963:errorcluster, 3:w2955:refnum<k5>)  [unwired: 3 in, 1 out]
        n1385 = while {
          tunnel: w2955 -> [w2983]
          tunnel: w2963 -> [w2982]
          tunnel: [w2973] -> w2961
          tunnel: [w2970] -> w2957
          i -> [w2979]
          stop <- w2970 stop-if-true
          n1386 = TCP Wait On Listener(8:w2982, 9:200 ("timeout ms (wait forever: -1)"), 11:w2983) -> (0:w2980:errorcluster, 4:w2977:refnum<k5>)  [unwired: 1 in, 3 out]
          n1387 = Less Or Equal?(x=50, y=w2979) -> (x <= y?=w2976:bool)
          n1388 = case shown="No Error" w2980 {
            selector: w2980 -> [w2993 w3003]
            tunnel: w2977 -> [w2994 _]
            tunnel: [errorcluster {"status"=TRUE, "code"=0, "source"=""} ("No error") w3004] -> w2972
            tunnel: [w2985 FALSE ("TCP connected?")] -> w2973
            frame No Error {
              # "connection is ready, read data"
              n1389 = TCP Read(connection ID=w2994, bytes to read=512, error in (no error)=w2993, 7:T21."CRLF" ("mode (standard)"), 9:5000 ("timeout ms (25000)")) -> (connection ID out=w2987:refnum<k5>, data out=w2989:string, error out=w2986:errorcluster)
              n1390 = Concatenate Strings("alive" ("string"), "\r\n" ("End of Line Constant")) -> (w2990:string)
              n1391 = Equal?(x=w2990, y=w2989) -> (x = y?=w2988:bool)
              n1392 = case shown="False" w2988 {
                tunnel: w2987 -> [_ w2999]
                tunnel: w2986 -> [_ _]
                tunnel: [FALSE ("TCP connected?") TRUE ("TCP connected?")] -> w2985
                frame False {
                }
                frame True {
                  n1393 = call "TcpIDFGV.vi"("action"=enum16{"write", "read"}."write", "connection ID in"=w2999) -> ()  [unwired: 8 in, 2 out]
                }
              }
            }
            frame Error {
              # "connection not ready, keep waiting"
              n1394 = Unbundle By Name(w3003) -> ("code"=w3005:i32)
              n1395 = case shown="56" w3005 {
                tunnel: w3003 -> [w3006 _]
                tunnel: [w3006 w3007] -> w3004
                frame Default {
                }
                frame 56 {
                  w3007 = errorcluster {"status"=FALSE, "code"=0, "source"=""}  # No error
                }
              }
            }
          }
          n1396 = Select(t=errorcluster {"status"=TRUE, "code"=5001, "source"=""} ("error in (no error)"), s=w2976, f=errorcluster {"status"=FALSE, "code"=0, "source"=""} ("error in (no error)")) -> (s? t:f=w2971:errorcluster)
          n1397 = Merge Errors(w2972, w2971) -> (w2970:errorcluster)
        }
        n1398 = Unbundle By Name(w2957) -> ("code"=w2960:i32)
        n1399 = Bundle By Name(cluster=w2962, "System Status.TCP/IP"=w2961, "listener ID"=w2955) -> (w2967:T23)
        n1400 = global write "GlobalVariables.vi" "TCP connected?"(w2961) -> ()
        n1401 = Equal To 0?(x=w2960) -> (x = 0?=w2959:bool)
        n1402 = Select(t=errorcluster {"status"=FALSE, "code"=0, "source"=""} ("error in (no error)"), s=w2959, f=w2957) -> (s? t:f=w2956:errorcluster)
        n1403 = call <vilib>:"Add State(s) to Queue__JKI_lib_State_Machine.vi"("State(s) in (\"\")"=w2969) -> ("States Out"=w2968:string)  [unwired: 14 in]
      }
      frame "TCP: checkSource" {
        # "Check visualization PC video source\n(send !video_source message, listen for response, then parse it to binary mask)"
        n1404 = Unbundle By Name(w3014) -> ("System Status.TCP/IP"=w3017:bool)
        n1405 = case shown="True" w3017 {
          tunnel: w3016 -> [w3022 w3045]
          tunnel: [w3022 w3029] -> w3015
          tunnel: [w3021 w3034] -> w3012
          tunnel: [w3021 w3032] -> w3011
          tunnel: [w3021 w3033] -> w3010
          tunnel: [w3021 w3031] -> w3009
          tunnel: [w3021 w3023] -> w3008
          frame False {
            w3021 = FALSE
          }
          frame True {
            n1406 = call "TcpIDFGV.vi"("Error In"=w3045, "action"=enum16{"write", "read"}."read") -> ("Error Out"=w3042:errorcluster, "connection ID out"=w3044:refnum<k5>)  [unwired: 8 in]
            n1407 = call "TCP_WriteRead.vi"("error in (no error)"=w3042, "data in"="!video_source", "connectin ID in"=w3044) -> ("error out"=w3039:errorcluster, "data out"=w3041:string)  [unwired: 4 in, 1 out]
            n1408 = Scan From String(format string="!video_source:%d", input string=w3041, error in=w3039) -> (error out=w3030:errorcluster, output 1=w3028:i32)  [unwired: 2 in, 2 out]
            n1409 = case shown="5..7, 9..11, 13..15" w3028 {
              tunnel: w3030 -> [_ _ _ _]
              tunnel: [errorcluster {"status"=TRUE, "code"=5007, "source"="Visualization PC"} ("error out") errorcluster {"status"=FALSE, "code"=0, "source"=""} ("error out") errorcluster {"status"=FALSE, "code"=0, "source"=""} ("error out") errorcluster {"status"=FALSE, "code"=0, "source"=""} ("error out")] -> w3029
              tunnel: [FALSE FALSE FALSE TRUE] -> w3023
              frame 0, Default {
                # "No video source available or default"
                n1410 = property on="Video Source" class="RadioBtnsControl (strict)"("DisabledEnum"=T11."Disabled and Grayed Out" ("Disabled")) -> ()  [unwired: 2 in, 2 out]
              }
              frame 1..3 {
                # "one or both camera available"
                n1411 = local write "Video Source"(enum32{"Camera", "FrameGrabber"}."Camera" ("Video Source")) -> ()
                n1412 = property on="Video Source" class="RadioBtnsControl (strict)"("DisabledEnum"=T11."Disabled and Grayed Out" ("Disabled")) -> ()  [unwired: 2 in, 2 out]
              }
              frame 4, 8, 12 {
                # "one or both frame grabber available"
                n1413 = local write "Video Source"(enum32{"Camera", "FrameGrabber"}."FrameGrabber" ("Video Source")) -> ()
                n1414 = property on="Video Source" class="RadioBtnsControl (strict)"("DisabledEnum"=T11."Disabled and Grayed Out" ("Disabled")) -> ()  [unwired: 2 in, 2 out]
              }
              frame 5..7, 9..11, 13..15 {
                n1415 = property on="Video Source" class="RadioBtnsControl (strict)"("DisabledEnum"=T11."Enabled" ("Disabled")) -> ()  [unwired: 2 in, 2 out]
              }
            }
            n1416 = Integer to Fixed-Point Cast(fixed-point type=fxp<+,4,4> 0.0, integer=w3028) -> (fixed-point=w3027:fxp<+,4,4>)
            n1417 = Number To Boolean Array(number=w3027) -> (Boolean array=w3025:bool[])
            n1418 = Reverse 1D Array(array=w3025) -> (reversed array=w3024:bool[])
            n1419 = Index Array(array=w3024, index=0) -> (element=w3034:bool)
            n1420 = Index Array(array=w3024, index=1) -> (element=w3032:bool)
            n1421 = Index Array(array=w3024, index=2) -> (element=w3033:bool)
            n1422 = Index Array(array=w3024, index=3) -> (element=w3031:bool)
          }
        }
        n1423 = Bundle By Name(cluster=w3014, "video source.Main Frame Grabber"=w3012, "video source.Side Frame Grabber"=w3011, "video source.Main Camera"=w3010, "video source.Side Camera"=w3009, "bothVidSourceAvail"=w3008) -> (w3013:T23)
        n1424 = call <vilib>:"Add State(s) to Queue__JKI_lib_State_Machine.vi"("State(s) in (\"\")"=w3020) -> ("States Out"=w3019:string)  [unwired: 14 in]
      }
      frame "TCP: SyncTime" {
        # "Template Separator\n(You can make a copy of, or modify, this frame)"
        n1425 = Unbundle By Name(w3062) -> ("System Status.TCP/IP"=w3061:bool)
        n1426 = case shown="True" w3061 {
          tunnel: w3063 -> [_ w3071]
          frame False {
          }
          frame True {
            n1427 = call "TcpIDFGV.vi"("Error In"=w3071, "action"=enum16{"write", "read"}."read") -> ("Error Out"=w3070:errorcluster, "connection ID out"=w3067:refnum<k5>)  [unwired: 8 in]
            n1428 = call <userlib>:"Tick Count (ms)__ogtk.vi"("error in (no error)"=w3070) -> ("error out"=w3069:errorcluster, "millisecond timer value"=w3068:u32)  [unwired: 9 in]
            n1429 = while {
              tunnel: w3069 -> [w3091]
              tunnel: w3067 -> [w3090]
              tunnel: w3068 -> [w3079]
              stop <- w3074 stop-if-true
              n1430 = Concatenate Strings("latencycheck" ("string"), "\r\n" ("End of Line Constant")) -> (w3086:string)
              n1431 = TCP Read(connection ID=w3090, bytes to read=512, error in (no error)=w3091, 7:T21."CRLF" ("mode (standard)"), 9:2000 ("timeout ms (25000)")) -> (connection ID out=w3083:refnum<k5>, data out=w3081:string, error out=w3073:errorcluster)
              n1432 = Tick Count (ms)() -> (millisecond timer value=w3080:u32)
              n1433 = Subtract(x=w3080, y=w3079) -> (x-y=w3078:u32)
              n1434 = Equal?(x=w3081, y=w3086) -> (x = y?=w3082:bool)
              n1435 = case shown="False" w3082 {
                tunnel: w3083 -> [_ w3104]
                tunnel: w3081 -> [w3096 _]
                tunnel: [w3092 FALSE] -> w3076
                tunnel: w3073 -> [_ w3098]
                frame False {
                  n1436 = Concatenate Strings("synctimer" ("string"), "\r\n" ("End of Line Constant")) -> (w3093:string)
                  n1437 = Equal?(x=w3096, y=w3093) -> (x = y?=w3092:bool)
                  "Sync Success?" <- w3092
                }
                frame True {
                  n1438 = Concatenate Strings("latencycheck:" ("string"), "\r\n" ("End of Line Constant")) -> (w3103:string)
                  n1439 = TCP Write(connection ID=w3104, data in=w3103, error in (no error)=w3098, 9:1000 ("timeout ms (25000)")) -> (error out=w3097:errorcluster)  [unwired: 2 out]
                  n1440 = call <vilib>:"Clear Errors.vi"("error in (no error)"=w3097) -> ()  [unwired: 5 in, 2 out]
                }
              }
              n1441 = Greater?(x=w3078, y=u32 10000 ("x-y")) -> (0:w3075:bool)
              n1442 = Or(x=w3076, y=w3075) -> (x .or. y?=w3074:bool)
            }
          }
        }
        n1443 = call <vilib>:"Add State(s) to Queue__JKI_lib_State_Machine.vi"("State(s) in (\"\")"=w3066) -> ("States Out"=w3065:string)  [unwired: 14 in]
      }
      frame "TCP: SendSettingMacro" {
        # "Template Separator\n(You can make a copy of, or modify, this frame)"
        n1444 = Unbundle By Name(w3108) -> ("System Status.TCP/IP"=w3107:bool)
        n1445 = case shown="True" w3107 {
          tunnel: ["" ("Empty String Constant") "TCP: sendSubjectID\nTCP: sendScaleBarSetting\nTCP: sendScaleMaxMin\nTCP: sendDeconChannel\nTCP: sendANSI\nTCP: sendRadius\nTCP: send3Dsetting\nTCP: sendFirefly\nTCP: sendPentero"] -> w3106
          frame False {
          }
          frame True {
          }
        }
        n1446 = call <vilib>:"Add State(s) to Queue__JKI_lib_State_Machine.vi"("State(s) in Front (\"\")"=w3106, "State(s) in (\"\")"=w3111) -> ("States Out"=w3110:string)  [unwired: 13 in]
      }
      frame "TCP: sendRunNum" {
        # "Send run number to AB PC\n(You can make a copy of, or modify, this frame)"
        n1447 = Unbundle By Name(w3118) -> ("System Status.TCP/IP"=w3115:bool, "IDs.RunID"=w3119:i8)
        n1448 = Increment(x=w3119) -> (x+1=w3114:i8)
        n1449 = case shown="True" w3115 {
          tunnel: w3114 -> [_ w3133]
          tunnel: [w3123 w3125] -> w3117
          tunnel: w3116 -> [w3123 w3124]
          frame False {
          }
          frame True {
            n1450 = Number To Decimal String(number=w3133, width (-)=i16 3) -> (decimal integer string=w3128:string)
            n1451 = call "TcpIDFGV.vi"("Error In"=w3124, "action"=enum16{"write", "read"}."read") -> ("Error Out"=w3126:errorcluster, "connection ID out"=w3130:refnum<k5>)  [unwired: 8 in]
            n1452 = Concatenate Strings("!run:", w3128) -> (w3127:string)
            n1453 = call "TCP_WriteRead.vi"("error in (no error)"=w3126, "data in"=w3127, "connectin ID in"=w3130) -> ("error out"=w3125:errorcluster)  [unwired: 4 in, 2 out]
          }
        }
        n1454 = call <vilib>:"Add State(s) to Queue__JKI_lib_State_Machine.vi"("State(s) in (\"\")"=w3122) -> ("States Out"=w3121:string)  [unwired: 14 in]
      }
      frame "TCP: sendVideoSource" {
        # "Send video source \n(You can make a copy of, or modify, this frame)"
        n1455 = Unbundle By Name(w3135) -> ("System Status.TCP/IP"=w3134:bool)
        n1456 = case shown="True" w3134 {
          tunnel: [w3141 w3143] -> w3137
          tunnel: w3136 -> [w3141 w3142]
          frame False {
          }
          frame True {
            n1457 = case shown="\"Camera\", Default" "Video Source" {
              tunnel: [0 1] -> w3148
              frame "Camera", Default {
              }
              frame "FrameGrabber" {
              }
            }
            n1458 = call "TcpIDFGV.vi"("Error In"=w3142, "action"=enum16{"write", "read"}."read") -> ("Error Out"=w3144:errorcluster, "connection ID out"=w3150:refnum<k5>)  [unwired: 8 in]
            n1459 = Number To Decimal String(number=w3148) -> (decimal integer string=w3146:string)  [unwired: 1 in]
            n1460 = Concatenate Strings("!invivo:" ("data in"), w3146) -> (w3145:string)
            n1461 = call "TCP_WriteRead.vi"("error in (no error)"=w3144, "data in"=w3145, "connectin ID in"=w3150) -> ("error out"=w3143:errorcluster)  [unwired: 4 in, 2 out]
          }
        }
        n1462 = call <vilib>:"Add State(s) to Queue__JKI_lib_State_Machine.vi"("State(s) in (\"\")"=w3140) -> ("States Out"=w3139:string)  [unwired: 14 in]
      }
      frame "TCP: startRun" {
        # "Template Separator\n(You can make a copy of, or modify, this frame)"
        n1463 = Unbundle By Name(w3155) -> ("System Status.TCP/IP"=w3154:bool)
        n1464 = case shown="True" w3154 {
          tunnel: [w3161 w3163] -> w3157
          tunnel: w3156 -> [w3161 w3162]
          frame False {
          }
          frame True {
            n1465 = call "TcpIDFGV.vi"("Error In"=w3162, "action"=enum16{"write", "read"}."read") -> ("Error Out"=w3164:errorcluster, "connection ID out"=w3165:refnum<k5>)  [unwired: 8 in]
            n1466 = call "TCP_WriteRead.vi"("error in (no error)"=w3164, "data in"="!acquire:1", "connectin ID in"=w3165) -> ("error out"=w3163:errorcluster)  [unwired: 4 in, 2 out]
          }
        }
        n1467 = call <vilib>:"Add State(s) to Queue__JKI_lib_State_Machine.vi"("State(s) in (\"\")"=w3160) -> ("States Out"=w3159:string)  [unwired: 14 in]
      }
      frame "TCP: stopRun" {
        # "Send stop run to AB PC\n(You can make a copy of, or modify, this frame)"
        n1468 = Unbundle By Name(w3169) -> ("System Status.TCP/IP"=w3168:bool)
        n1469 = case shown="True" w3168 {
          tunnel: [w3175 w3177] -> w3171
          tunnel: w3170 -> [w3175 w3176]
          frame False {
            # "if not connected, do nothing"
          }
          frame True {
            # "If TCP connected, send stop run"
            n1470 = call "TcpIDFGV.vi"("Error In"=w3176, "action"=enum16{"write", "read"}."read") -> ("Error Out"=w3178:errorcluster, "connection ID out"=w3180:refnum<k5>)  [unwired: 8 in]
            n1471 = call "TCP_WriteRead.vi"("error in (no error)"=w3178, "data in"="!acquire:0", "connectin ID in"=w3180) -> ("error out"=w3177:errorcluster)  [unwired: 4 in, 2 out]
          }
        }
        n1472 = call <vilib>:"Add State(s) to Queue__JKI_lib_State_Machine.vi"("State(s) in (\"\")"=w3174) -> ("States Out"=w3173:string)  [unwired: 14 in]
      }
      frame "TCP: CheckConnection" {
        # "Check TCP/IP connection statuse\n(If connection is lost, throw error)"
        n1473 = Unbundle By Name(w3183) -> ("System Status.TCP/IP"=w3182:bool)
        n1474 = case shown="False" w3182 {
          frame False {
          }
          frame True {
            # "If TCP/IP is true check, otherwise skip"
          }
        }
        n1475 = call <vilib>:"Add State(s) to Queue__JKI_lib_State_Machine.vi"("State(s) in (\"\")"=w3187) -> ("States Out"=w3186:string)  [unwired: 14 in]
      }
      frame "TCP: sendSubjectID" {
        # "Send subject ID"
        n1476 = Unbundle By Name(w3189) -> ("System Status.TCP/IP"=w3188:bool, "CaseID"=w3192:string)
        n1477 = case shown="True" w3188 {
          tunnel: w3192 -> [_ w3203]
          tunnel: [w3196 w3198] -> w3191
          tunnel: w3190 -> [w3196 w3197]
          frame False {
          }
          frame True {
            n1478 = call "TcpIDFGV.vi"("Error In"=w3197, "action"=enum16{"write", "read"}."read") -> ("Error Out"=w3199:errorcluster, "connection ID out"=w3201:refnum<k5>)  [unwired: 8 in]
            n1479 = Concatenate Strings("!subject:", w3203) -> (w3200:string)
            n1480 = call "TCP_WriteRead.vi"("error in (no error)"=w3199, "data in"=w3200, "connectin ID in"=w3201) -> ("error out"=w3198:errorcluster)  [unwired: 4 in, 2 out]
          }
        }
        n1481 = call <vilib>:"Add State(s) to Queue__JKI_lib_State_Machine.vi"("State(s) in (\"\")"=w3195) -> ("States Out"=w3194:string)  [unwired: 14 in]
      }
      frame "TCP: sendScaleBarSetting" {
        # "Template Separator\n(You can make a copy of, or modify, this frame)"
        n1482 = Unbundle By Name(w3207) -> ("System Status.TCP/IP"=w3205:bool, "VideoConfig.Scale Bar"=w3206:bool)
        n1483 = case shown="True" w3205 {
          tunnel: [w3213 w3222] -> w3209
          tunnel: w3208 -> [w3213 w3221]
          tunnel: w3206 -> [_ w3220]
          frame False {
          }
          frame True {
            n1484 = Boolean To (0,1)(Boolean=w3220) -> (0, 1=w3219:i16)
            n1485 = call "TcpIDFGV.vi"("Error In"=w3221, "action"=enum16{"write", "read"}."read") -> ("Error Out"=w3223:errorcluster, "connection ID out"=w3224:refnum<k5>)  [unwired: 8 in]
            n1486 = Number To Fractional String(number=w3219, width (-)=i16 1, precision (6)=i16 0) -> (F-format string=w3217:string)  [unwired: 1 in]
            n1487 = Concatenate Strings("!autocolor:" ("data in"), w3217) -> (w3215:string)
            n1488 = call "TCP_WriteRead.vi"("error in (no error)"=w3223, "data in"=w3215, "connectin ID in"=w3224) -> ("error out"=w3222:errorcluster)  [unwired: 4 in, 2 out]
          }
        }
        n1489 = call <vilib>:"Add State(s) to Queue__JKI_lib_State_Machine.vi"("State(s) in (\"\")"=w3212) -> ("States Out"=w3211:string)  [unwired: 14 in]
      }
      frame "TCP: sendScaleMaxMin" {
        # "Send scale bar max and min to AB PC\n(You can make a copy of, or modify, this frame)"
        n1490 = Unbundle By Name(w3229) -> ("System Status.TCP/IP"=w3226:bool, "VideoConfig.Scale Low"=w3228:dbl, "VideoConfig.Scale High"=w3227:dbl)
        n1491 = case shown="True" w3226 {
          tunnel: [w3235 w3248] -> w3231
          tunnel: w3230 -> [w3235 w3247]
          tunnel: w3228 -> [_ w3246]
          tunnel: w3227 -> [_ w3237]
          frame False {
          }
          frame True {
            n1492 = call "TcpIDFGV.vi"("Error In"=w3247, "action"=enum16{"write", "read"}."read") -> ("Error Out"=w3249:errorcluster, "connection ID out"=w3250:refnum<k5>)  [unwired: 8 in]
            n1493 = Number To Fractional String(number=w3246, width (-)=i16 4, precision (6)=i16 2) -> (F-format string=w3242:string)  [unwired: 1 in]
            n1494 = Number To Fractional String(number=w3237, width (-)=i16 4, precision (6)=i16 2) -> (F-format string=w3238:string)  [unwired: 1 in]
            n1495 = Concatenate Strings("!color:" ("string"), w3242, ";" ("string"), w3238) -> (w3236:string)
            n1496 = call "TCP_WriteRead.vi"("error in (no error)"=w3249, "data in"=w3236, "connectin ID in"=w3250) -> ("error out"=w3248:errorcluster)  [unwired: 4 in, 2 out]
          }
        }
        n1497 = call <vilib>:"Add State(s) to Queue__JKI_lib_State_Machine.vi"("State(s) in (\"\")"=w3234) -> ("States Out"=w3233:string)  [unwired: 14 in]
      }
      frame "TCP: sendDeconChannel" {
        # "Send Decon channel\n(You can make a copy of, or modify, this frame)"
        n1498 = Unbundle By Name(w3253) -> ("System Status.TCP/IP"=w3252:bool)
        n1499 = case shown="True" w3252 {
          tunnel: [w3259 w3264] -> w3255
          tunnel: w3254 -> [w3259 w3263]
          frame False {
          }
          frame True {
            n1500 = local read "Radio Buttons"() -> (w3262:T9)
            n1501 = Increment(x=w3262) -> (x+1=w3261:T9)
            n1502 = Number To Decimal String(number=w3261) -> (decimal integer string=w3260:string)  [unwired: 1 in]
            n1503 = call "TcpIDFGV.vi"("Error In"=w3263, "action"=enum16{"write", "read"}."read") -> ("Error Out"=w3265:errorcluster, "connection ID out"=w3268:refnum<k5>)  [unwired: 8 in]
            n1504 = Concatenate Strings("!channel:", w3260) -> (w3266:string)
            n1505 = call "TCP_WriteRead.vi"("error in (no error)"=w3265, "data in"=w3266, "connectin ID in"=w3268) -> ("error out"=w3264:errorcluster)  [unwired: 4 in, 2 out]
          }
        }
        n1506 = call <vilib>:"Add State(s) to Queue__JKI_lib_State_Machine.vi"("State(s) in (\"\")"=w3258) -> ("States Out"=w3257:string)  [unwired: 14 in]
      }
      frame "TCP: sendANSI" {
        # "Template Separator\n(You can make a copy of, or modify, this frame)"
        n1507 = Unbundle By Name(w3272) -> ("System Status.TCP/IP"=w3270:bool, "VideoConfig.ANSI"=w3271:dbl)
        n1508 = case shown="True" w3270 {
          tunnel: [w3278 w3284] -> w3274
          tunnel: w3273 -> [w3278 w3283]
          tunnel: w3271 -> [_ w3282]
          frame False {
          }
          frame True {
            n1509 = Number To Fractional String(number=w3282) -> (F-format string=w3280:string)  [unwired: 3 in]
            n1510 = call "TcpIDFGV.vi"("Error In"=w3283, "action"=enum16{"write", "read"}."read") -> ("Error Out"=w3285:errorcluster, "connection ID out"=w3286:refnum<k5>)  [unwired: 8 in]
            n1511 = Concatenate Strings("!ansi:" ("data in"), w3280) -> (w3279:string)
            n1512 = call "TCP_WriteRead.vi"("error in (no error)"=w3285, "data in"=w3279, "connectin ID in"=w3286) -> ("error out"=w3284:errorcluster)  [unwired: 4 in, 2 out]
          }
        }
        n1513 = call <vilib>:"Add State(s) to Queue__JKI_lib_State_Machine.vi"("State(s) in (\"\")"=w3277) -> ("States Out"=w3276:string)  [unwired: 14 in]
      }
      frame "TCP: sendRadius" {
        # "Send drawing radius to AB PC\n(You can make a copy of, or modify, this frame)"
        n1514 = Unbundle By Name(w3290) -> ("System Status.TCP/IP"=w3288:bool, "VideoConfig.Radius"=w3289:dbl)
        n1515 = case shown="True" w3288 {
          tunnel: [w3296 w3302] -> w3292
          tunnel: w3291 -> [w3296 w3301]
          tunnel: w3289 -> [_ w3300]
          frame False {
          }
          frame True {
            n1516 = Number To Fractional String(number=w3300) -> (F-format string=w3299:string)  [unwired: 3 in]
            n1517 = Concatenate Strings("!radius:" ("data in"), w3299) -> (w3297:string)
            n1518 = call "TcpIDFGV.vi"("Error In"=w3301, "action"=enum16{"write", "read"}."read") -> ("Error Out"=w3303:errorcluster, "connection ID out"=w3304:refnum<k5>)  [unwired: 8 in]
            n1519 = call "TCP_WriteRead.vi"("error in (no error)"=w3303, "data in"=w3297, "connectin ID in"=w3304) -> ("error out"=w3302:errorcluster)  [unwired: 4 in, 2 out]
          }
        }
        n1520 = call <vilib>:"Add State(s) to Queue__JKI_lib_State_Machine.vi"("State(s) in (\"\")"=w3295) -> ("States Out"=w3294:string)  [unwired: 14 in]
      }
      frame "TCP: send3Dsetting" {
        # "Send 3D setting to AB computer\n(You can make a copy of, or modify, this frame)"
        n1521 = Unbundle By Name(w3308) -> ("System Status.TCP/IP"=w3306:bool, "VideoConfig.3D?"=w3307:bool)
        n1522 = case shown="True" w3306 {
          tunnel: [w3314 w3321] -> w3310
          tunnel: w3309 -> [w3314 w3320]
          tunnel: w3307 -> [_ w3319]
          frame False {
          }
          frame True {
            n1523 = Boolean To (0,1)(Boolean=w3319) -> (0, 1=w3318:i16)
            n1524 = Number To Fractional String(number=w3318) -> (F-format string=w3317:string)  [unwired: 3 in]
            n1525 = call "TcpIDFGV.vi"("Error In"=w3320, "action"=enum16{"write", "read"}."read") -> ("Error Out"=w3322:errorcluster, "connection ID out"=w3323:refnum<k5>)  [unwired: 8 in]
            n1526 = Concatenate Strings("!3dset:" ("data in"), w3317) -> (w3315:string)
            n1527 = call "TCP_WriteRead.vi"("error in (no error)"=w3322, "data in"=w3315, "connectin ID in"=w3323) -> ("error out"=w3321:errorcluster)  [unwired: 4 in, 2 out]
          }
        }
        n1528 = call <vilib>:"Add State(s) to Queue__JKI_lib_State_Machine.vi"("State(s) in (\"\")"=w3313) -> ("States Out"=w3312:string)  [unwired: 14 in]
      }
      frame "TCP: sendFirefly" {
        # "Template Separator\n(You can make a copy of, or modify, this frame)"
        n1529 = Unbundle By Name(w3326) -> ("System Status.TCP/IP"=w3325:bool)
        n1530 = case shown="False" w3325 {
          tunnel: [w3332 w3334] -> w3328
          tunnel: w3327 -> [w3332 w3333]
          frame False {
          }
          frame True {
            n1531 = call "TcpIDFGV.vi"("Error In"=w3333, "action"=enum16{"write", "read"}."read") -> ("Error Out"=w3335:errorcluster, "connection ID out"=w3337:refnum<k5>)  [unwired: 8 in]
            n1532 = call "TCP_WriteRead.vi"("error in (no error)"=w3335, "data in"="!firefly:0", "connectin ID in"=w3337) -> ("error out"=w3334:errorcluster)  [unwired: 4 in, 2 out]
          }
        }
        n1533 = call <vilib>:"Add State(s) to Queue__JKI_lib_State_Machine.vi"("State(s) in (\"\")"=w3331) -> ("States Out"=w3330:string)  [unwired: 14 in]
      }
      frame "TCP: sendPentero" {
        # "Send Pentero setting to AB computer\n(You can make a copy of, or modify, this frame)"
        n1534 = Unbundle By Name(w3340) -> ("System Status.TCP/IP"=w3339:bool)
        n1535 = case shown="True" w3339 {
          tunnel: [w3346 w3348] -> w3342
          tunnel: w3341 -> [w3346 w3347]
          frame False {
          }
          frame True {
            n1536 = call "TcpIDFGV.vi"("Error In"=w3347, "action"=enum16{"write", "read"}."read") -> ("Error Out"=w3349:errorcluster, "connection ID out"=w3351:refnum<k5>)  [unwired: 8 in]
            n1537 = call "TCP_WriteRead.vi"("error in (no error)"=w3349, "data in"="!pentero:0", "connectin ID in"=w3351) -> ("error out"=w3348:errorcluster)  [unwired: 4 in, 2 out]
          }
        }
        n1538 = call <vilib>:"Add State(s) to Queue__JKI_lib_State_Machine.vi"("State(s) in (\"\")"=w3345) -> ("States Out"=w3344:string)  [unwired: 14 in]
      }
      frame "TCP: sendChannel" {
        # "Send DeCon Channel to AB computer\n()"
        n1539 = Unbundle By Name(w3354) -> ("System Status.TCP/IP"=w3353:bool)
        n1540 = case shown="True" w3353 {
          tunnel: [w3360 w3364] -> w3356
          tunnel: w3355 -> [w3360 w3363]
          frame False {
          }
          frame True {
            n1541 = local read "Radio Buttons"() -> (w3362:T9)
            n1542 = case shown="\"No Selection\", Default" w3362 {
              tunnel: ["" ("data in") "!channel:1" ("data in") "!channel:2" ("data in") "!channel:3" ("data in")] -> w3361
              frame "No Selection", Default {
              }
              frame "Ch1" {
              }
              frame "Ch2" {
              }
              frame "Ch3" {
              }
            }
            n1543 = call "TcpIDFGV.vi"("Error In"=w3363, "action"=enum16{"write", "read"}."read") -> ("Error Out"=w3365:errorcluster, "connection ID out"=w3366:refnum<k5>)  [unwired: 8 in]
            n1544 = call "TCP_WriteRead.vi"("error in (no error)"=w3365, "data in"=w3361, "connectin ID in"=w3366) -> ("error out"=w3364:errorcluster)  [unwired: 4 in, 2 out]
          }
        }
        n1545 = call <vilib>:"Add State(s) to Queue__JKI_lib_State_Machine.vi"("State(s) in (\"\")"=w3359) -> ("States Out"=w3358:string)  [unwired: 14 in]
      }
      frame "TCP: startCam" {
        # "Send Pentero setting to AB computer\n(You can make a copy of, or modify, this frame)"
        n1546 = Unbundle By Name(w3373) -> ("System Status.TCP/IP"=w3372:bool)
        n1547 = case shown="True" w3372 {
          tunnel: [w3379 w3381] -> w3375
          tunnel: w3374 -> [w3379 w3380]
          frame False {
          }
          frame True {
            n1548 = call "TcpIDFGV.vi"("Error In"=w3380, "action"=enum16{"write", "read"}."read") -> ("Error Out"=w3382:errorcluster, "connection ID out"=w3384:refnum<k5>)  [unwired: 8 in]
            n1549 = call "TCP_WriteRead.vi"("error in (no error)"=w3382, "data in"="!focus:1", "connectin ID in"=w3384) -> ("error out"=w3381:errorcluster)  [unwired: 4 in, 2 out]
          }
        }
        n1550 = call <vilib>:"Add State(s) to Queue__JKI_lib_State_Machine.vi"("State(s) in (\"\")"=w3378) -> ("States Out"=w3377:string)  [unwired: 14 in]
      }
      frame "TCP: stopCam" {
        # "Send Pentero setting to AB computer\n(You can make a copy of, or modify, this frame)"
        n1551 = Unbundle By Name(w3387) -> ("System Status.TCP/IP"=w3386:bool)
        n1552 = case shown="True" w3386 {
          tunnel: [w3393 w3395] -> w3389
          tunnel: w3388 -> [w3393 w3394]
          frame False {
          }
          frame True {
            n1553 = call "TcpIDFGV.vi"("Error In"=w3394, "action"=enum16{"write", "read"}."read") -> ("Error Out"=w3396:errorcluster, "connection ID out"=w3398:refnum<k5>)  [unwired: 8 in]
            n1554 = call "TCP_WriteRead.vi"("error in (no error)"=w3396, "data in"="!focus:0", "connectin ID in"=w3398) -> ("error out"=w3395:errorcluster)  [unwired: 4 in, 2 out]
          }
        }
        n1555 = call <vilib>:"Add State(s) to Queue__JKI_lib_State_Machine.vi"("State(s) in (\"\")"=w3392) -> ("States Out"=w3391:string)  [unwired: 14 in]
      }
      frame "TCP: Close" {
        # "Close TCP connection\n()"
        n1556 = Unbundle By Name(w3402) -> ("System Status.TCP/IP"=w3400:bool)
        n1557 = case shown="True" w3400 {
          tunnel: [w3408 w3410] -> w3403
          tunnel: w3401 -> [w3408 w3409]
          frame False {
          }
          frame True {
            n1558 = call "TcpIDFGV.vi"("Error In"=w3409, "action"=enum16{"write", "read"}."read") -> ("Error Out"=w3412:errorcluster, "connection ID out"=w3413:refnum<k5>)  [unwired: 8 in]
            n1559 = TCP Close Connection(connection ID=w3413, error in (no error)=w3412) -> (error out=w3410:errorcluster)  [unwired: 1 in, 1 out]
          }
        }
        n1560 = case shown="Error .." w3403 {
          tunnel: [w3416 w3417] -> w3404
          tunnel: w3402 -> [w3415 w3417]
          frame No Error {
            w3414 = FALSE ("System Status.TCP/IP")
            n1561 = Bundle By Name(cluster=w3415, "System Status.TCP/IP"=w3414) -> (w3416:T23)
            n1562 = global write "GlobalVariables.vi" "TCP connected?"(w3414) -> ()
          }
          frame Error {
          }
        }
        n1563 = call <vilib>:"Add State(s) to Queue__JKI_lib_State_Machine.vi"("State(s) in (\"\")"=w3407) -> ("States Out"=w3406:string)  [unwired: 14 in]
      }
      frame "---------- PID ----------" {
        # "Template Separator\n(You can make a copy of, or modify, this frame)"
        n1564 = call <vilib>:"Add State(s) to Queue__JKI_lib_State_Machine.vi"("State(s) in (\"\")"=w3422) -> ("States Out"=w3421:string)  [unwired: 14 in]
      }
      frame "PID: loadPID" {
        # "Template Separator\n(You can make a copy of, or modify, this frame)"
        n1565 = call "readPIDSetting.vi"("Error In"=w3426) -> ("Error Out"=w3427:errorcluster, "Ch3 PID out"=w3423:T8, "Ch2 PID out"=w3424:T8, "Ch1 PID out"=w3425:T8)  [unwired: 7 in]
        n1566 = local write "Ch1 PID gains"(w3425) -> ()
        n1567 = local write "Ch2 PID gains"(w3424) -> ()
        n1568 = local write "Ch3 PID gains"(w3423) -> ()
        n1569 = local write "Ch4 PID gains"(w3423) -> ()
        n1570 = call <vilib>:"Add State(s) to Queue__JKI_lib_State_Machine.vi"("State(s) in (\"\")"=w3431) -> ("States Out"=w3430:string)  [unwired: 14 in]
      }
      frame "---------- Classifier ----------" {
        # "Template Separator\n(You can make a copy of, or modify, this frame)"
        n1571 = call <vilib>:"Add State(s) to Queue__JKI_lib_State_Machine.vi"("State(s) in (\"\")"=w3436) -> ("States Out"=w3435:string)  [unwired: 14 in]
      }
      frame "Classifier: Init" {
        # "Initilize Python\n(You can make a copy of, or modify, this frame)"
        n1572 = call-poly <vilib>:"Open Virtual Environment Session.vi"("error in (no error)"=w3445, "Anaconda path"=path "C:/ProgramData/miniconda3", "Python version"="Python version", "Env name"="Env name") -> ("error out"=w3441:errorcluster, "session out"=w3444:refnum<k35>)  [unwired: 6 in]
        n1573 = Path To String(path="model path") -> (string=w3438:string)
        n1574 = node "Python Node"(w3444, "module path", "load_model" ("function name"), w3441, w3438) -> (→"Python session":refnum<k35>, w3440:errorcluster)  [unwired: 3 in, 2 out]
        n1575 = call <vilib>:"Add State(s) to Queue__JKI_lib_State_Machine.vi"("State(s) in (\"\")"=w3452) -> ("States Out"=w3451:string)  [unwired: 14 in]
      }
      frame "Classifier: Close" {
        # "Template Separator\n(You can make a copy of, or modify, this frame)"
        n1576 = local read "Python session"() -> (w3456:refnum<k35>)
        n1577 = Close Python Session(session in=w3456, error in=w3455) -> (11:w3454:errorcluster)
        n1578 = case shown="Error .." w3454 {
          selector: w3454 -> [w3461 _]
          tunnel: [w3461 errorcluster {"status"=FALSE, "code"=0, "source"=""} ("error IO")] -> w3453
          frame No Error {
          }
          frame Error {
          }
        }
        n1579 = call <vilib>:"Add State(s) to Queue__JKI_lib_State_Machine.vi"("State(s) in (\"\")"=w3460) -> ("States Out"=w3459:string)  [unwired: 14 in]
      }
      frame "---------- Temp ----------" {
        # "Template Separator\n(You can make a copy of, or modify, this frame)"
        n1580 = call <vilib>:"Add State(s) to Queue__JKI_lib_State_Machine.vi"("State(s) in (\"\")"=w3467) -> ("States Out"=w3466:string)  [unwired: 14 in]
      }
      frame "Temp: KeepEmpty" {
        # "Template Separator\n(You can make a copy of, or modify, this frame)"
        n1581 = call <vilib>:"Add State(s) to Queue__JKI_lib_State_Machine.vi"("State(s) in (\"\")"=w3472) -> ("States Out"=w3471:string)  [unwired: 14 in]
      }
    }
    n1582 = Not(x=w80) -> (.not. x?=w79:bool)
    n1583 = local write "ML?"(w79) -> ()
    "ML?" <- TRUE ("main loop running?")
  }
  n1584 = while {
    tunnel: w19 -> [w3506]
    tunnel: w18 -> [w3475]
    tunnel: [w3474] -> w17
    tunnel: w13 -> [w3502]
    tunnel: [w3501] -> w16
    shift-right: [w3497] -> _
    shift-left: _ -> [w3498]
    stop <- w3477 stop-if-true
    # "Read data from notifier and deconvolve it and send to Aiming Beam computer"
    n1585 = Wait on Notification(notifier=w3506, ignore previous (F)=FALSE) -> (notification=w3493:T14, error out=w3477:errorcluster)  [unwired: 2 in, 2 out]
    n1586 = local read "Data Class"() -> (w3478:enum16{"Data", "BG", "Cali"})
    n1587 = Unbundle(w3493) -> ("idx"=w3476:i32, "CH1&2"=w3505:dbl[][], "CH3&4"=w3504:dbl[][], "V cluster"=w3483:cluster{"V1":dbl, "V2":dbl, "V3":dbl, "V4":dbl})
    n1588 = call "SeperateChanData.vi"("Input (Ch1&2)"=w3504) -> ("Ch1"=w3480:dbl[][], "Ch2"=w3488:dbl[][])
    n1589 = call "SeperateChanData.vi"("Input (Ch1&2)"=w3505) -> ("Ch1"=w3482:dbl[][], "Ch2"=w3481:dbl[][])
    n1590 = case shown="\"Data\"" w3478 {
      tunnel: w3483 -> [w3518 _]
      tunnel: w3482 -> [w3517 _]
      tunnel: w3481 -> [w3516 _]
      tunnel: w3480 -> [w3515 _]
      tunnel: w3477 -> [w3514 w3626]
      tunnel: w3476 -> [w3513 _]
      tunnel: w3475 -> [w3511 w3627]
      tunnel: [w3508 w3627] -> w3474
      tunnel: [w3507 w3626] -> w3473
      frame "Data" {
        # "If acquiring data"
        n1591 = case shown="0, Default" "Overlay selection" {
          tunnel: "Radio Buttons" -> [w3522 _]
          tunnel: [w3523 w3546] -> w3509
          tunnel: w3514 -> [w3523 w3545]
          tunnel: [w3521 w3533] -> w3512
          tunnel: w3518 -> [_ w3552]
          tunnel: w3517 -> [_ w3549]
          tunnel: w3516 -> [_ w3548]
          tunnel: w3515 -> [_ w3547]
          frame 0, Default {
            # "overlay gain"
            n1592 = case shown="\"Ch4\"" w3522 {
              tunnel: [0.0 ("Gain1") w3525 w3526 w3527 w3528] -> w3521
              frame "No Selection", Default {
              }
              frame "Ch1" {
                n1593 = local read "Gain1"() -> (w3525:dbl)
              }
              frame "Ch2" {
                n1594 = local read "Gain2"() -> (w3526:dbl)
              }
              frame "Ch3" {
                n1595 = local read "Gain3"() -> (w3527:dbl)
              }
              frame "Ch4" {
                n1596 = local read "Gain4"() -> (w3528:dbl)
              }
            }
          }
          frame 1, 2 {
            # "overlay lifetime or cancer probability"
            n1597 = call "DeConAPD2FGV.vi"("Error In"=w3545) -> ("Error Out"=w3551:errorcluster, "APDClass out"=w3542:T40)  [unwired: 9 in]
            n1598 = call "DeConAPD1FGV.vi"("Error In"=w3545) -> ("Error Out"=w3553:errorcluster, "APDClass out"=w3544:T40)  [unwired: 9 in]
            n1599 = call "DeConAPD3FGV.vi"("Error In"=w3545) -> ("Error Out"=w3550:errorcluster, "APDClass out"=w3540:T40)  [unwired: 9 in]
            n1600 = Unbundle By Name(w3552) -> ("V1"=w3543:dbl, "V2"=w3541:dbl, "V3"=w3539:dbl)
            n1601 = call "getGain.vi"("CtrlV"=w3539, "APD"=w3540) -> ("gain"=w3530:dbl)  [unwired: 8 in, 1 out]
            n1602 = call "getGain.vi"("CtrlV"=w3543, "APD"=w3544) -> ("gain"=w3532:dbl)  [unwired: 8 in, 1 out]
            n1603 = call "getGain.vi"("CtrlV"=w3541, "APD"=w3542) -> ("gain"=w3531:dbl)  [unwired: 8 in, 1 out]
            n1604 = Less?(x=w3532, y="Ch1GainLim") -> (x < y?=w3537:bool)
            n1605 = Less?(x=w3531, y="Ch2&3GainLim") -> (x < y?=w3536:bool)
            n1606 = Less?(x=w3530, y="Ch2&3GainLim") -> (x < y?=w3535:bool)
            n1607 = Compound Arithmetic op=AND(w3537, w3536, w3535) -> (w3534:bool)
            n1608 = case shown="True" w3534 {
              tunnel: w3553 -> [_ w3616]
              tunnel: w3551 -> [_ w3615]
              tunnel: w3550 -> [_ w3614]
              tunnel: w3549 -> [_ w3604]
              tunnel: w3548 -> [_ w3603]
              tunnel: w3547 -> [_ w3602]
              tunnel: [w3554 w3563] -> w3546
              tunnel: w3545 -> [w3554 w3595]
              tunnel: w3544 -> [_ w3594]
              tunnel: w3543 -> [_ w3593]
              tunnel: w3542 -> [_ w3592]
              tunnel: w3541 -> [_ w3591]
              tunnel: w3540 -> [_ w3590]
              tunnel: w3539 -> [_ w3589]
              tunnel: [0.0 ("Gain4") w3556] -> w3533
              tunnel: w3532 -> [_ w3581]
              tunnel: w3531 -> [_ w3580]
              tunnel: w3530 -> [_ w3579]
              frame False {
                # "give probability of 0.5"
                # "if gain is out of acceptable range"
              }
              frame True {
                # "if gain is within range"
                n1609 = Build Array(w3581, w3580, w3579) -> (w3578:dbl[])
                n1610 = call "getIrf (SubVI).vi"("error in"=w3616, "CtrlV"=w3593, "APD"=w3594) -> ("error out"=w3608:errorcluster, "irfTNorm"=w3611:dbl[])  [unwired: 6 in, 1 out]
                n1611 = call "getIrf (SubVI).vi"("error in"=w3615, "CtrlV"=w3591, "APD"=w3592) -> ("error out"=w3607:errorcluster, "irfTNorm"=w3610:dbl[])  [unwired: 6 in, 1 out]
                n1612 = call "getIrf (SubVI).vi"("error in"=w3614, "CtrlV"=w3589, "APD"=w3590) -> ("error out"=w3606:errorcluster, "irfTNorm"=w3609:dbl[])  [unwired: 6 in, 1 out]
                n1613 = call "DotNetFGV.vi"("Error In"=w3595) -> ("Error Out"=w3599:errorcluster, "reference out"=w3600:refnum<k24>)  [unwired: 9 in]
                n1614 = local read "BGAll"() -> (w3613:dbl[][])
                n1615 = Merge Errors(w3599, w3608, w3607, w3606) -> (w3605:errorcluster)
                n1616 = Build Array(w3611, w3610, w3609) -> (w3596:dbl[][])
                n1617 = Build Array (concatenate)(w3604, w3603, w3602) -> (w3601:dbl[][])
                n1618 = local write "iRF Graph"(w3596) -> ()
                n1619 = Transpose 2D Array(2D array=w3613) -> (transposed array=w3612:dbl[][])
                n1620 = Transpose 2D Array(2D array=w3596) -> (transposed array=w3597:dbl[][])
                n1621 = Transpose 2D Array(2D array=w3601) -> (transposed array=w3598:dbl[][])
                n1622 = Reciprocal(x=w3578) -> (1/x=w3576:dbl[])
                n1623 = call "LagDeConAllCh (SubVI).vi"("new reference"=w3600, "error in (no error)"=w3605, "irf"=w3597, "BG"=w3612, "WF"=w3598) -> ("error out"=w3564:errorcluster, "LCs"=w3572:dbl[][], "INTs"=w3583:dbl[][], "LTs"=w3588:dbl[][])  [unwired: 3 in]
                n1624 = Index Array(array=w3588, index (col)=0 ("disabled index (col)")) -> (element=w3570:dbl[])  [unwired: 1 in]
                n1625 = Index Array(array=w3583, index (col)=0 ("disabled index (col)")) -> (element=w3577:dbl[])  [unwired: 1 in]
                n1626 = Multiply(x=w3577, y=w3576) -> (x*y=w3575:dbl[])
                n1627 = Index Array(array=w3572, index (col)=0 ("disabled index (col)")) -> (element=w3568:dbl[])  [unwired: 1 in]
                n1628 = Add Array Elements(numeric array=w3575) -> (sum=w3574:dbl)
                n1629 = Index Array(array=w3570, index=0) -> (element=w3560:dbl)
                "Ch1 Lifetime (ns)" <- w3560
                n1630 = Index Array(array=w3570, index=1) -> (element=w3559:dbl)
                "Ch2 Lifetime (ns)" <- w3559
                n1631 = Index Array(array=w3570, index=2) -> (element=w3558:dbl)
                "Ch3 Lifetime (ns)" <- w3558
                n1632 = Divide(x=w3575, y=w3574) -> (x/y=w3569:dbl[])
                n1633 = Bundle(w3560, w3559, w3558) -> (→"Lifetime (ns)":cluster{dbl, dbl, dbl})  [unwired: 1 in]
                n1634 = Build Array (concatenate)(w3570, w3569, w3568) -> (w3561:dbl[])
                "DeConOut" <- w3561
                n1635 = local read "module path"() -> (w3566:path)
                n1636 = local read "Python session"() -> (w3567:refnum<k35>)
                n1637 = node(w3567, w3566, "HNPredict" ("function name"), w3564, 0.0, w3561) -> (w3563:errorcluster, w3557:dbl)  [unwired: 1 in, 3 out]
                "Cancer Prob" <- w3557
                n1638 = disable-structure shown="Enabled" {
                  disable-tunnel: w3557 -> [w3619 w3624]
                  disable-tunnel: [w3618 w3620] -> w3556
                  frame Disabled {
                    n1639 = Add(x=0.01, y=w3619) -> (x+y=w3618:dbl)
                  }
                  frame Enabled {
                    n1640 = Greater?(x=w3624, y="CancerThreshold") -> (0:w3625:bool)
                    n1641 = Select(t=1.0, s=w3625, f=0.01) -> (s? t:f=w3620:dbl)
                  }
                }
              }
            }
          }
        }
        n1642 = Bundle("idx"=w3513, "f"=w3512) -> (w3510:cluster{"idx":i32, "f":dbl})  [unwired: 1 in]
        n1643 = Send Notification(notification=w3510, notifier=w3511, error in (no error)=w3509) -> (notifier out=w3508:refnum<notifier>, error out=w3507:errorcluster)
      }
      frame "BG", Default {
        # "if not acquiting data"
      }
    }
    n1644 = call "AvgArrayTimeCritical.vi"("2D array"=w3482) -> ("1D Avg"=w3489:dbl[])  [unwired: 10 in]
    n1645 = call "AvgArrayTimeCritical.vi"("2D array"=w3481) -> ("1D Avg"=w3490:dbl[])  [unwired: 10 in]
    n1646 = call "AvgArrayTimeCritical.vi"("2D array"=w3480) -> ("1D Avg"=w3491:dbl[])  [unwired: 10 in]
    n1647 = call "AvgArrayTimeCritical.vi"("2D array"=w3488) -> ("1D Avg"=w3492:dbl[])  [unwired: 10 in]
    n1648 = Build Array(w3492) -> (w3487:dbl[][])
    n1649 = Build Array(w3491) -> (w3486:dbl[][])
    n1650 = Build Array(w3490) -> (w3485:dbl[][])
    n1651 = Build Array(w3489) -> (w3484:dbl[][])
    n1652 = flat-sequence {
      tunnel: [w3628] -> w3497
      tunnel: w3477 -> [_]
      frame #0 {
        n1653 = call <vilib>:"High Resolution Relative Seconds.vi"() -> ("relative seconds"=w3628:dbl)
      }
    }
    n1654 = Subtract(x=w3497, y=w3498) -> (x-y=w3500:dbl)
    n1655 = Multiply(x=w3500, y=1000.0) -> (x*y=→"Decon Loop timing (ms)" →"DeCon Speed(ms)":dbl)
    n1656 = Bundle(w3484, w3485, w3486, w3487, "V cluster"=w3483) -> (w3503:T48)  [unwired: 1 in]
    n1657 = Send Notification(notification=w3503, notifier=w3502, error in (no error)=w3477) -> (notifier out=w3501:refnum<notifier>, error out=w3479:errorcluster)
    n1658 = Merge Errors(w3473, w3479) -> (→"decon error out":errorcluster)
  }
  n1659 = while {
    tunnel: w18 -> [w3640]
    shift-right: [w3633] -> _
    shift-left: u32 0 -> [w3634]
    stop <- w3631 stop-if-true
    # "Send data to AB computer here"
    # "if TCP ip is not open loop will run once and stop. To re-establish connection and start this loop. Reboot softwrae."
    # "Data communication loop"
    n1660 = Wait on Notification(notifier=w3640, ignore previous (F)=FALSE) -> (notification=w3638:cluster{"idx":i32, "lifetime":dbl}, error out=w3632:errorcluster)  [unwired: 2 in, 2 out]
    n1661 = Wait Until Next ms Multiple(millisecond multiple=u32 25) -> ()  [unwired: 1 out]
    n1662 = Unbundle(w3638) -> ("idx"=w3637:i32, "lifetime"=w3636:dbl)
    n1663 = Tick Count (ms)() -> (millisecond timer value=w3633:u32)
    n1664 = global read "GlobalVariables.vi" "TCP connected?"() -> (w3630:bool)
    n1665 = Subtract(x=w3633, y=w3634) -> (x-y=→"Communication loop(ms)":u32)
    n1666 = case shown="True" w3630 {
      tunnel: w3637 -> [_ w3649]
      tunnel: w3636 -> [_ w3648]
      tunnel: w3632 -> [w3641 w3645]
      tunnel: [w3641 w3642] -> w3631
      frame False {
      }
      frame True {
        n1667 = Number To Decimal String(number=w3649) -> (decimal integer string=w3657:string)  [unwired: 1 in]
        n1668 = call "TcpIDFGV.vi"("Error In"=w3645, "action"=enum16{"write", "read"}."read") -> ("Error Out"=w3644:errorcluster, "connection ID out"=w3655:refnum<k5>)  [unwired: 8 in]
        n1669 = Concatenate Strings("!idx:", w3657) -> (w3658:string)
        n1670 = call "TCP_WriteRead.vi"("error in (no error)"=w3644, "data in"=w3658, "connectin ID in"=w3655) -> ("error out"=w3643:errorcluster, "connectin ID out"=w3656:refnum<k5>)  [unwired: 4 in, 1 out]
        n1671 = Number To Fractional String(number=w3648, precision (6)=i16 2) -> (F-format string=w3647:string)  [unwired: 2 in]
        n1672 = Concatenate Strings("!lifetime:", w3647) -> (w3654:string)
        n1673 = call "TCP_WriteRead.vi"("error in (no error)"=w3643, "data in"=w3654, "connectin ID in"=w3656) -> ("error out"=w3642:errorcluster, "data out"=→"data out(communcation loop)":string)  [unwired: 4 in, 1 out]
      }
    }
  }
  n1674 = while {
    tunnel: w13 -> [w3669]
    shift-right: [w3660] -> _
    shift-left: w15 -> [w3667]
    shift-right: [w3662] -> _
    shift-left: w15 -> [w3661]
    i -> [w3663]
    stop <- w3664 stop-if-true
    # "Data display loop(30Hz)"
    n1675 = Wait on Notification(notifier=w3669, ignore previous (F)=FALSE) -> (notification=w3665:T13, error out=w3664:errorcluster)  [unwired: 2 in, 2 out]
    n1676 = Wait Until Next ms Multiple(millisecond multiple=u32 40) -> ()  [unwired: 1 out]
    n1677 = Tick Count (ms)() -> (millisecond timer value=w3660:u32)
    n1678 = Subtract(x=w3660, y=w3667) -> (x-y=→"display loop timing(ms)":u32)
    n1679 = case shown="No Error" w3664 {
      tunnel: w3665 -> [w3742 _]
      tunnel: w3661 -> [w3714 w3814]
      tunnel: [w3716 w3814] -> w3662
      tunnel: w3660 -> [w3713 _]
      frame No Error {
        w3671 = u32 1 ("Active Plot")
        w3690 = 0 ("index (row)")
        n1680 = Subtract(x=w3713, y=w3714) -> (x-y=w3715:u32)
        n1681 = Unbundle(w3742) -> ("CH1"=w3737:dbl[][], "CH2"=w3735:dbl[][], "CH3"=w3732:dbl[][], "CH4"=w3685:dbl[][], "Gain cluster"=w3691:cluster{"V1":dbl, "V2":dbl, "V3":dbl, "V4":dbl})
        n1682 = Unbundle By Name(w3691) -> ("V1"=w3709:dbl, "V2"=w3707:dbl, "V3"=w3705:dbl, "V4"=w3683:dbl)
        n1683 = Index Array(array=w3737, index (row)=w3690) -> (element=w3721:dbl[])  [unwired: 1 in]
        n1684 = Index Array(array=w3735, index (row)=w3690) -> (element=w3719:dbl[])  [unwired: 1 in]
        n1685 = Index Array(array=w3732, index (row)=w3690) -> (element=w3720:dbl[])  [unwired: 1 in]
        n1686 = Index Array(array=w3685, index (row)=w3690) -> (element=w3689:dbl[])  [unwired: 1 in]
        n1687 = call "RemoveDCBG.vi"("Channel"=enum16{"DC Only", "Ch1", "Ch2", "Ch3", "Ch4"}."Ch4", "WF in"=w3689) -> ("DC"=w3687:dbl, "WF out"=w3676:dbl[])  [unwired: 7 in, 1 out]
        n1688 = Greater?(x=w3715, y=u32 200) -> (0:w3717:bool)
        n1689 = call "CtrlVtoGain.vi"("CtrlV(V)"=w3683, "Channel"=enum16{"Ch1", "Ch2", "Ch3", "Ch4"}."Ch4") -> ("Gain"=w3675:dbl)  [unwired: 8 in, 1 out]
        n1690 = call "CtrlVtoGain.vi"("CtrlV(V)"=w3709, "Channel"=enum16{"Ch1", "Ch2", "Ch3"}."Ch1") -> ("Gain"=w3703:dbl)  [unwired: 8 in, 1 out]
        n1691 = call "RemoveDCBG.vi"("Channel"=enum16{"DC Only", "Ch1", "Ch2", "Ch3"}."Ch1", "WF in"=w3721) -> ("DC"=w3738:dbl, "WF out"=w3710:dbl[])  [unwired: 7 in, 1 out]
        n1692 = call "RemoveDCBG.vi"("Channel"=enum16{"DC Only", "Ch1", "Ch2", "Ch3"}."Ch2", "WF in"=w3719) -> ("DC"=w3734:dbl, "WF out"=w3711:dbl[])  [unwired: 7 in, 1 out]
        n1693 = call "CtrlVtoGain.vi"("CtrlV(V)"=w3707, "Channel"=enum16{"Ch1", "Ch2", "Ch3"}."Ch2") -> ("Gain"=w3698:dbl)  [unwired: 8 in, 1 out]
        n1694 = call "RemoveDCBG.vi"("Channel"=enum16{"DC Only", "Ch1", "Ch2", "Ch3"}."Ch3", "WF in"=w3720) -> ("DC"=w3731:dbl, "WF out"=w3712:dbl[])  [unwired: 7 in, 1 out]
        n1695 = call "CtrlVtoGain.vi"("CtrlV(V)"=w3705, "Channel"=enum16{"Ch1", "Ch2", "Ch3"}."Ch3") -> ("Gain"=w3694:dbl)  [unwired: 8 in, 1 out]
        n1696 = formula code="int32 out = 2;\nif (G<5){\nout = 1;\n}\nif (G>200){\nout = 3;\n}"("G"=w3675) -> ("out"=→"output variable":i32)
        n1697 = Add(x=w3676, y=w3687) -> (x+y=w3686:dbl[])
        n1698 = Less?(x=w3675, y=5.0) -> (x < y?=w3681:bool)
        n1699 = case shown="True" w3717 {
          tunnel: w3710 -> [_ w3771]
          tunnel: w3711 -> [_ w3774]
          tunnel: w3712 -> [_ w3773]
          tunnel: w3713 -> [_ w3789]
          tunnel: [w3753 w3789] -> w3716
          tunnel: w3714 -> [w3753 _]
          tunnel: w3703 -> [_ w3767]
          tunnel: w3698 -> [_ w3766]
          tunnel: w3694 -> [_ w3765]
          tunnel: w3676 -> [_ w3761]
          tunnel: w3675 -> [_ w3758]
          frame False {
          }
          frame True {
            n1700 = call "GetSNR(SubVI).vi"("Waveform"=w3771) -> ("SNR"=→"SNR1":dbl)  [unwired: 10 in]
            n1701 = Array Size(array=w3771) -> (size(s)=w3772:i32)
            n1702 = call "GetSNR(SubVI).vi"("Waveform"=w3774) -> ("SNR"=→"SNR2":dbl)  [unwired: 10 in]
            n1703 = call "GetSNR(SubVI).vi"("Waveform"=w3773) -> ("SNR"=→"SNR3":dbl)  [unwired: 10 in]
            n1704 = call "GetSNR(SubVI).vi"("Waveform"=w3761) -> ("SNR"=→"SNR4":dbl)  [unwired: 10 in]
            n1705 = global read "GlobalVariables.vi" "BG Idx2"() -> (w3760:i32)
            n1706 = Subtract(x=w3772, y=w3760) -> (x-y=w3759:i32)
            n1707 = Array Subset(array=w3771, index=w3760, length=w3759) -> (w3778:dbl[])
            n1708 = Array Subset(array=w3774, index=w3760, length=w3759) -> (w3780:dbl[])
            n1709 = Array Subset(array=w3773, index=w3760, length=w3759) -> (w3782:dbl[])
            n1710 = Array Subset(array=w3761, index=w3760, length=w3759) -> (w3762:dbl[])
            n1711 = Add Array Elements(numeric array=w3778) -> (sum=w3779:dbl)
            n1712 = Add Array Elements(numeric array=w3780) -> (sum=w3781:dbl)
            n1713 = Add Array Elements(numeric array=w3782) -> (sum=w3783:dbl)
            n1714 = Add Array Elements(numeric array=w3762) -> (sum=w3763:dbl)
            n1715 = Divide(x=w3779, y=w3767) -> (x/y=w3784:dbl)
            n1716 = Divide(x=w3781, y=w3766) -> (x/y=w3785:dbl)
            n1717 = Divide(x=w3783, y=w3765) -> (x/y=w3786:dbl)
            n1718 = Divide(x=w3763, y=w3758) -> (x/y=w3757:dbl)
            n1719 = Build Array(w3784, w3785, w3786, w3757) -> (w3787:dbl[])
            n1720 = Add Array Elements(numeric array=w3787) -> (sum=w3788:dbl)
            n1721 = Divide(x=w3787, y=w3788) -> (x/y=w3756:dbl[])
            n1722 = Index Array(array=w3756, index=2) -> (element=→"IntR3":dbl)
            n1723 = Index Array(array=w3756, index=1) -> (element=→"IntR2":dbl)
            n1724 = Index Array(array=w3756, index=0) -> (element=→"IntR1":dbl)
            n1725 = Index Array(array=w3756, index=3) -> (element=→"IntR4":dbl)
          }
        }
        n1726 = Add(x=w3710, y=w3738) -> (x+y=w3736:dbl[])
        n1727 = Add(x=w3711, y=w3734) -> (x+y=w3733:dbl[])
        n1728 = Add(x=w3712, y=w3731) -> (x+y=w3730:dbl[])
        n1729 = Less?(x=w3703, y=5.0 ("x")) -> (x < y?=w3701:bool)
        n1730 = Less?(x=w3698, y=5.0 ("x")) -> (x < y?=w3697:bool)
        n1731 = Less?(x=w3694, y=5.0 ("x")) -> (x < y?=w3693:bool)
        n1732 = case shown="False" w3693 {
          tunnel: [u32 16448250 ("Plot.Plot Color") u32 16711680 ("Plot.Plot Color")] -> w3692
          frame False {
          }
          frame True {
          }
        }
        n1733 = case shown="True" "Show BG removed?" {
          tunnel: w3737 -> [w3796 w3812]
          tunnel: w3736 -> [_ w3802]
          tunnel: [w3796 w3811] -> w3729
          tunnel: w3735 -> [w3795 w3810]
          tunnel: [w3795 w3809] -> w3673
          tunnel: w3733 -> [_ w3798]
          tunnel: w3732 -> [w3794 w3808]
          tunnel: [w3794 w3807] -> w3724
          tunnel: w3730 -> [_ w3803]
          tunnel: [w3793 w3806] -> w3680
          tunnel: w3686 -> [_ w3800]
          tunnel: w3685 -> [w3793 w3805]
          frame False {
          }
          frame True {
            n1734 = Insert Into Array(array=w3808, index (row)=1, new element=w3803) -> (w3807:dbl[][])  [unwired: 1 in]
            n1735 = Insert Into Array(array=w3812, index (row)=1, new element=w3802) -> (w3811:dbl[][])  [unwired: 1 in]
            n1736 = Insert Into Array(array=w3810, index (row)=1, new element=w3798) -> (w3809:dbl[][])  [unwired: 1 in]
            n1737 = Insert Into Array(array=w3805, index (row)=1, new element=w3800) -> (w3806:dbl[][])  [unwired: 1 in]
          }
        }
        "Channel 1" <- w3729
        "Channel 2" <- w3673
        "Channel 3" <- w3724
        "Channel 4" <- w3680
        n1738 = case shown="False" w3701 {
          tunnel: [u32 16448250 ("Plot.Plot Color") u32 16711680 ("Plot.Plot Color")] -> w3700
          frame False {
          }
          frame True {
          }
        }
        n1739 = case shown="False" w3697 {
          tunnel: [u32 16448250 ("Plot.Plot Color") u32 16711680 ("Plot.Plot Color")] -> w3696
          frame False {
          }
          frame True {
          }
        }
        n1740 = case shown="False" w3681 {
          tunnel: [u32 16448250 ("Plot.Plot Color") u32 16711680 ("Plot.Plot Color")] -> w3677
          frame False {
          }
          frame True {
          }
        }
        n1741 = case shown="False" "Show BG removed?" {
          tunnel: [u32 16744703 ("Plot.Plot Color") u32 16741120 ("Plot.Plot Color")] -> w3670
          frame False {
          }
          frame True {
          }
        }
        n1742 = property on="Channel 1" class="WFGraph (strict)"("Active Plot"=w3671, "Plot.Plot Color"=w3670, "Plot.Line Style"=u8 1, "Plot.Line Width"=u8 2, "BG Color"=w3700) -> ()  [unwired: 2 in, 2 out]
        n1743 = property on="Channel 2" class="WFGraph (strict)"("Active Plot"=w3671, "Plot.Plot Color"=w3670, "Plot.Line Style"=u8 1, "Plot.Line Width"=u8 2, "BG Color"=w3696) -> ()  [unwired: 2 in, 2 out]
        n1744 = property on="Channel 4" class="WFGraph (strict)"("Active Plot"=w3671, "Plot.Plot Color"=w3670, "Plot.Line Style"=u8 1, "Plot.Line Width"=u8 2, "BG Color"=w3677) -> ()  [unwired: 2 in, 2 out]
        n1745 = property on="Channel 3" class="WFGraph (strict)"("Active Plot"=w3671, "Plot.Plot Color"=w3670, "Plot.Line Style"=u8 1, "Plot.Line Width"=u8 2, "BG Color"=w3692) -> ()  [unwired: 2 in, 2 out]
      }
      frame Error {
        w3813 = u32 16448250 ("Plot Area:Colors:BG Color")
        n1746 = property on="Channel 1" class="WFGraph (strict)"("BG Color"=w3813) -> ()  [unwired: 2 in, 2 out]
        n1747 = property on="Channel 2" class="WFGraph (strict)"("BG Color"=w3813) -> ()  [unwired: 2 in, 2 out]
        n1748 = property on="Channel 3" class="WFGraph (strict)"("BG Color"=w3813) -> ()  [unwired: 2 in, 2 out]
      }
    }
    "DisplayLoop" <- w3663
  }
  n1749 = while {
    tunnel: w65 -> [w3827]
    tunnel: w55 -> [w3826]
    tunnel: [w3825] -> w63
    tunnel: w19 -> [w3824]
    tunnel: [w3823] -> w59
    tunnel: w39 -> [w3821]
    tunnel: w48 -> [w3820]
    tunnel: w35 -> [w3815]
    stop <- w3818 stop-if-true
    # "acquire data and send it to processing loop"
    # "Data Aquisition Loop"
    n1750 = event shown="[1] <Start digitizer>: User Event" {
      selector: w3826 -> [_ _]
      dyn-events: [_ _] -> w3825
      timeout: 30 -> [_ _]
      tunnel: w3827 -> [w3833 w3843]
      tunnel: [w3828 _] -> w3818
      tunnel: w3824 -> [w3832 w3850]
      tunnel: [w3832 w3849] -> w3823
      tunnel: w3821 -> [_ w3847]
      tunnel: w3820 -> [w3831 w3842]
      tunnel: w3815 -> [_ w3840]
      event Timeout {
        # "use queue to stop data loop\nwhen queue ref is released, error will stop this loop"
        n1751 = event-data() -> ()  [unwired: 1 in, 3 out]
        n1752 = Get Queue Status(queue=w3833) -> (error out=w3830:errorcluster)  [unwired: 2 in, 7 out]
        n1753 = Get Queue Status(queue=w3831) -> (error out=w3829:errorcluster)  [unwired: 2 in, 7 out]
        n1754 = Merge Errors(w3830, w3829) -> (w3828:errorcluster)
      }
      event User Event {
        w3848 = enum16{"Write", "Read"}."Read" ("Operation")
        n1755 = event-data() -> ("Time"=→"RunStartTime":u32)  [unwired: 1 in, 3 out]
        n1756 = call "FLImDAQ_FGV.vi"() -> ("Read data"=w3845:T5)  [unwired: 10 in, 1 out]
        n1757 = call "Digitizer1_FGV.vi"("Operation (Read)"=w3848) -> ("Read data"=w3839:refnum<k15>)  [unwired: 9 in, 1 out]
        n1758 = call "Digitizer2_FGV.vi"("Operation (Read)"=w3848) -> ("Read data"=w3846:refnum<k15>)  [unwired: 9 in, 1 out]
        n1759 = Unbundle By Name(w3845) -> ("Waveform to Avg"=w3844:i16)
        n1760 = property on="Property Node" class="niScope"(reference=w3839) -> (reference out=w3838:refnum<k15>, "Vertical Range"=w3837:dbl, "Vertical Offset"=w3836:dbl)  [unwired: 1 in, 1 out]
        n1761 = Tick Count (ms)() -> (millisecond timer value=w3835:u32)
        n1762 = while {
          tunnel: w3850 -> [w3910]
          tunnel: [w3909] -> w3849
          tunnel: w3846 -> [w3903]
          tunnel: w3838 -> [w3902]
          tunnel: w3847 -> [w3901]
          shift-right: [w3870] -> _
          shift-left: u32 0 ("millisecond timer value") -> [w3895]
          tunnel: w3844 -> [w3851]
          tunnel: w3843 -> [w3892]
          tunnel: w3842 -> [w3890]
          tunnel: w3840 -> [w3883]
          tunnel: w3837 -> [w3880]
          tunnel: w3836 -> [w3881]
          shift-right: [w3875] -> _
          shift-left: w3835 -> [w3874]
          i -> [w3852]
          stop <- w3873 stop-if-true
          w3863 = enum16{"write", "read"}."read" ("action")
          w3896 = 65536
          # "enqueue V"
          # "enqueue ch3 data"
          # "enqueue ch1&2 data"
          # "acquire ch3"
          # "acquire ch1&2"
          # "send data for processing"
          n1763 = Multiply(x=w3851, y=w3852) -> (x*y=w3860:i32)
          "Fetch Record #" <- w3860
          n1764 = property on="Property Node" class="niScope"(reference=w3902, "Fetch Record Number"=w3860) -> (reference out=w3914:refnum<k15>, error out=w3913:errorcluster, "Records Done"=w3882:i32)  [unwired: 1 in]
          n1765 = Subtract(x=w3882, y=w3860) -> (x-y=→"Record Backlog":i32)
          n1766 = call-poly <instrlib>:"niScope Fetch (poly).vi"("timeout"=1.0, "error in"=w3913, "channels"="0,1", "instrument handle"=w3914) -> ("error out"=w3857:errorcluster, "wfm"=w3858:i16[][], "wfm info"=w3879:T49)  [unwired: 4 in, 1 out]
          n1767 = property on="Property Node" class="niScope"(reference=w3903, "Fetch Record Number"=w3860) -> (reference out=w3907:refnum<k15>, error out=w3904:errorcluster, "Records Done"=w3861:i32)  [unwired: 1 in]
          n1768 = Divide(x=w3858, y=w3896) -> (x/y=w3869:dbl[][])
          n1769 = Tick Count (ms)() -> (millisecond timer value=w3870:u32)
          n1770 = Subtract(x=w3861, y=w3860) -> (x-y=→"Record Backlog 2":i32)
          n1771 = Subtract(x=w3870, y=w3895) -> (x-y=→"Aquisition loop timing(ms)":u32)
          n1772 = Subtract(x=w3870, y=w3874) -> (x-y=w3878:u32)
          n1773 = Multiply(x=w3869, y=w3880) -> (x*y=w3900:dbl[][])
          n1774 = call-poly <instrlib>:"niScope Fetch (poly).vi"("timeout"=0.25, "error in"=w3904, "channels"="0,1", "instrument handle"=w3907) -> ("error out"=w3856:errorcluster, "wfm"=w3897:i16[][])  [unwired: 4 in, 2 out]
          n1775 = Greater?(x=w3878, y=u32 1000) -> (0:w3876:bool)
          n1776 = Add(x=w3900, y=w3881) -> (x+y=w3891:dbl[][])
          n1777 = case shown="True" w3876 {
            tunnel: w3879 -> [_ w3923]
            tunnel: w3870 -> [_ w3922]
            tunnel: [w3916 w3922] -> w3875
            tunnel: w3874 -> [w3916 _]
            tunnel: [errorcluster {"status"=FALSE, "code"=0, "source"=""} ("error constant") w3919] -> w3871
            frame False {
            }
            frame True {
              # "[Covers: REQ29]"
              n1778 = call "CheckFrequency(SubVI).vi"("wfm info"=w3923) -> ("f (Hz)"=w3921:dbl)  [unwired: 10 in]
              "Laser f (Hz)" <- w3921
              n1779 = local read "Laser Rep Rate"() -> (w3918:dbl)
              n1780 = Increment(x=w3918) -> (x+1=w3917:dbl)
              n1781 = Greater?(x=w3921, y=w3917) -> (0:w3920:bool)
              n1782 = case shown="True" w3920 {
                tunnel: [errorcluster {"status"=FALSE, "code"=0, "source"=""} ("error constant") errorcluster {"status"=TRUE, "code"=0, "source"=""} ("error constant")] -> w3919
                frame False {
                }
                frame True {
                }
              }
            }
          }
          n1783 = Divide(x=w3897, y=w3896) -> (x/y=w3899:dbl[][])
          n1784 = Enqueue Element(queue=w3892, element=w3891, error in (no error)=w3857) -> (error out=w3855:errorcluster)  [unwired: 1 in, 2 out]
          n1785 = Multiply(x=w3899, y=w3880) -> (x*y=w3898:dbl[][])
          n1786 = Add(x=w3898, y=w3881) -> (x+y=w3889:dbl[][])
          n1787 = Enqueue Element(queue=w3890, element=w3889, error in (no error)=w3856) -> (error out=w3854:errorcluster)  [unwired: 1 in, 2 out]
          n1788 = Merge Errors(w3855, w3854) -> (w3853:errorcluster)
          n1789 = call "V1FGV.vi"("Error In"=w3853, "action (write)"=w3863) -> ("Error Out"=w3887:errorcluster, "V1 out"=w3885:dbl)  [unwired: 8 in]
          n1790 = call "V2FGV.vi"("Error In"=w3887, "action(write)"=w3863) -> ("Error Out"=w3886:errorcluster, "V2 out"=w3884:dbl)  [unwired: 8 in]
          n1791 = call "V3FGV.vi"("Error In"=w3886, "action(write)"=w3863) -> ("Error Out"=w3866:errorcluster, "V3 out"=w3865:dbl)  [unwired: 8 in]
          n1792 = call "V4FGV.vi"("Error In"=w3866, "action(write)"=w3863, "V3 in"=w3865) -> ("Error Out"=w3864:errorcluster, "V3 out"=w3862:dbl)  [unwired: 7 in]
          n1793 = Bundle("V1 out"=w3885, "V2 out"=w3884, "V3 out"=w3865, "V3 out"=w3862) -> (w3868:T50)  [unwired: 1 in]
          n1794 = Bundle(w3852, w3891, w3889, w3868) -> (w3893:T51)  [unwired: 1 in]
          n1795 = Enqueue Element(queue=w3883, element=w3868, error in (no error)=w3864) -> (error out=w3867:errorcluster)  [unwired: 1 in, 2 out]
          n1796 = Send Notification(notification=w3893, notifier=w3910, error in (no error)=w3867) -> (notifier out=w3909:refnum<notifier>, error out=w3872:errorcluster)
          n1797 = Merge Errors(w3871, w3872) -> (w3888:errorcluster)
          n1798 = case shown="Error .." w3888 {
            selector: w3888 -> [w3926 w3927]
            tunnel: w3901 -> [_ w3930]
            tunnel: [w3926 w3927] -> w3873
            frame No Error {
            }
            frame Error {
              # "Send user event to signal aquisition has stoped"
              n1799 = Generate User Event(priority (normal)=usereventprio."high priority", user event=w3930, event data cluster=TRUE ("event data")) -> ()  [unwired: 1 in, 2 out]
            }
          }
          "aquisition loop Error Out" <- w3873
          "Auisition Loop idx" <- w3852
        }
      }
    }
    n1800 = Unbundle By Name(w3818) -> ("status"=w3817:bool)
    n1801 = Not(x=w3817) -> (.not. x?=w3816:bool)
    n1802 = local write "Aq Loop?"(w3816) -> ()
    "Aq Loop?" <- TRUE ("Aq L?")
  }
  n1803 = disable-structure "Diagram Disable Structure" shown="Disabled" {
    frame Disabled {
      w3931 = T52 {"Horizontal"=500, "Vertical"=100}  # Top Left Corner
      n1804 = Control Help Window(0:w3931, 1:TRUE ("Show")) -> ()
      n1805 = call <vilib>:"TDMS - File Viewer.vi"() -> ()  [unwired: 6 in, 2 out]
    }
    frame Enabled {
    }
  }
  n1806 = while {
    tunnel: w19 -> [w3980]
    shift-right: [w3943] -> _
    shift-left: _ -> [w3976]
    tunnel: [w3934] -> w1 mode=indexing
    i -> [w3960]
    stop <- w3940 stop-if-true
    # "Channel 3"
    # "Channel 2"
    # "Channel 1"
    # "use FGV for gain value"
    # "stop on error"
    # "Gain adjustment and Data processing"
    n1807 = Tick Count (ms)() -> (millisecond timer value=w3943:u32)
    n1808 = Wait on Notification(notifier=w3980, ignore previous (F)=TRUE) -> (notification=w3954:T14, error out=w3933:errorcluster)  [unwired: 2 in, 2 out]
    n1809 = Subtract(x=w3943, y=w3976) -> (x-y=→"PID loop timing(ms)":u32)
    n1810 = Unbundle(w3954) -> ("CH1&2"=w3970:dbl[][], "CH3&4"=w3969:dbl[][])  [unwired: 2 out]
    n1811 = call "SeperateChanData.vi"("Input (Ch1&2)"=w3970) -> ("Ch1"=w3965:dbl[][], "Ch2"=w3963:dbl[][])
    n1812 = call "SeperateChanData.vi"("Input (Ch1&2)"=w3969) -> ("Ch1"=w3959:dbl[][], "Ch2"=w3952:dbl[][])
    n1813 = call "AvgArrayTimeCritical.vi"("2D array"=w3965) -> ("1D Avg"=w3964:dbl[])  [unwired: 10 in]
    n1814 = call "AvgArrayTimeCritical.vi"("2D array"=w3963) -> ("1D Avg"=w3974:dbl[])  [unwired: 10 in]
    n1815 = call "AvgArrayTimeCritical.vi"("2D array"=w3959) -> ("1D Avg"=w3971:dbl[])  [unwired: 10 in]
    n1816 = call "AvgArrayTimeCritical.vi"("2D array"=w3952) -> ("1D Avg"=w3951:dbl[])  [unwired: 10 in]
    n1817 = Array Max & Min(array=w3964) -> (max value=w3962:dbl)  [unwired: 3 out]
    n1818 = Array Max & Min(array=w3974) -> (max value=w3961:dbl)  [unwired: 3 out]
    n1819 = Array Max & Min(array=w3971) -> (max value=w3944:dbl)  [unwired: 3 out]
    n1820 = Array Max & Min(array=w3951) -> (max value=w3949:dbl)  [unwired: 3 out]
    n1821 = local read "Auto gain ch4"() -> (w3950:bool)
    n1822 = local read "Auto gain ch1"() -> (w3968:bool)
    n1823 = local read "Auto gain ch2"() -> (w3967:bool)
    n1824 = local read "Auto gain ch3"() -> (w3966:bool)
    n1825 = case shown="True" w3950 {
      tunnel: w3949 -> [_ w4027]
      tunnel: "V target(1.0)" -> [_ w4025]
      tunnel: [FALSE w4022] -> w3947
      tunnel: [0.0 ("CtrlV") w4017] -> w3948
      frame False {
        # "Manual control"
      }
      frame True {
        # "PID control"
        n1826 = global read "GlobalVariables.vi" "Ch4GainLim(Log)"() -> (w4028:cluster{"GainMax":dbl, "GainMin":dbl})
        n1827 = call-poly <vilib>:"PID.vi"("output range"=w4028, "PID gains"="Ch4 PID gains", "process variable"=w4027, "setpoint"=w4025) -> ("output"=w4026:dbl)  [unwired: 6 in, 1 out]
        n1828 = Power Of 10(x=w4026) -> (10^x=w4018:dbl)
        "Gain4" <- w4018
        n1829 = call "V4FGV.vi"("action(write)"=enum16{"write", "read"}."read") -> ("Error Out"=w4021:errorcluster, "V3 out"=w4023:dbl)  [unwired: 9 in]
        n1830 = call "GainToCtrlV.vi"("Gain"=w4018, "Channel"=enum16{"Ch1", "Ch2", "Ch3", "Ch4"}."Ch4") -> ("CtrlV"=w4017:dbl)  [unwired: 8 in, 1 out]
        n1831 = call "V4FGV.vi"("Error In"=w4021, "V3 in"=w4017) -> ()  [unwired: 8 in, 2 out]
        n1832 = local write "V 4"(w4017) -> ()
        n1833 = Not Equal?(x=w4017, y=w4023) -> (x != y?=w4022:bool)
      }
    }
    n1834 = case shown="True" w3968 {
      tunnel: "V target(1.0)" -> [_ w4042]
      tunnel: w3962 -> [_ w4039]
      tunnel: [0.0 ("CtrlV") w4031] -> w3941
      tunnel: [FALSE w4033] -> w3958
      frame False {
        # "Manual control"
      }
      frame True {
        # "PID control"
        n1835 = global read "GlobalVariables.vi" "Ch1GainLim(Log)"() -> (w4038:cluster{"GainMax":dbl, "GainMin":dbl})
        n1836 = call-poly <vilib>:"PID.vi"("output range"=w4038, "PID gains"="Ch1 PID gains", "process variable"=w4039, "setpoint"=w4042) -> ("output"=w4037:dbl)  [unwired: 6 in, 1 out]
        n1837 = Power Of 10(x=w4037) -> (10^x=w4036:dbl)
        "Gain1" <- w4036
        n1838 = call "V1FGV.vi"("action (write)"=enum16{"write", "read"}."read") -> ("Error Out"=w4032:errorcluster, "V1 out"=w4034:dbl)  [unwired: 9 in]
        n1839 = call "GainToCtrlV.vi"("Gain"=w4036, "Channel"=enum16{"Ch1", "Ch2", "Ch3"}."Ch1") -> ("CtrlV"=w4031:dbl)  [unwired: 8 in, 1 out]
        n1840 = local write "V 1"(w4031) -> ()
        n1841 = call "V1FGV.vi"("Error In"=w4032, "V1 in"=w4031) -> ()  [unwired: 8 in, 2 out]
        n1842 = Not Equal?(x=w4031, y=w4034) -> (x != y?=w4033:bool)
      }
    }
    n1843 = case shown="True" w3967 {
      tunnel: w3961 -> [_ w4069]
      tunnel: "V target(1.0)" -> [_ w4070]
      tunnel: [FALSE w4063] -> w3957
      tunnel: [0.0 ("CtrlV") w4059] -> w3953
      frame False {
        # "Manual control"
      }
      frame True {
        # "PID control"
        n1844 = global read "GlobalVariables.vi" "Ch2GainLim(Log)"() -> (w4067:cluster{"GainMax":dbl, "GainMin":dbl})
        n1845 = call-poly <vilib>:"PID.vi"("output range"=w4067, "PID gains"="Ch2 PID gains", "process variable"=w4069, "setpoint"=w4070) -> ("output"=w4066:dbl)  [unwired: 6 in, 1 out]
        n1846 = Power Of 10(x=w4066) -> (10^x=w4064:dbl)
        "Gain2" <- w4064
        n1847 = call "V2FGV.vi"("action(write)"=enum16{"write", "read"}."read") -> ("Error Out"=w4060:errorcluster, "V2 out"=w4061:dbl)  [unwired: 9 in]
        n1848 = call "GainToCtrlV.vi"("Gain"=w4064, "Channel"=enum16{"Ch1", "Ch2", "Ch3"}."Ch2") -> ("CtrlV"=w4059:dbl)  [unwired: 8 in, 1 out]
        n1849 = local write "V 2"(w4059) -> ()
        n1850 = call "V2FGV.vi"("Error In"=w4060, "V2 in"=w4059) -> ()  [unwired: 8 in, 2 out]
        n1851 = Not Equal?(x=w4059, y=w4061) -> (x != y?=w4063:bool)
      }
    }
    n1852 = case shown="True" w3966 {
      tunnel: w3944 -> [_ w4054]
      tunnel: "V target(1.0)" -> [_ w4051]
      tunnel: [FALSE w4047] -> w3956
      tunnel: [0.0 ("CtrlV") w4045] -> w3955
      frame False {
        # "Manual control"
      }
      frame True {
        # "PID control"
        n1853 = global read "GlobalVariables.vi" "Ch3GainLim(Log)"() -> (w4055:cluster{"GainMax":dbl, "GainMin":dbl})
        n1854 = call-poly <vilib>:"PID.vi"("output range"=w4055, "PID gains"="Ch3 PID gains", "process variable"=w4054, "setpoint"=w4051) -> ("output"=w4053:dbl)  [unwired: 6 in, 1 out]
        n1855 = Power Of 10(x=w4053) -> (10^x=w4050:dbl)
        "Gain3" <- w4050
        n1856 = call "V3FGV.vi"("action(write)"=enum16{"write", "read"}."read") -> ("Error Out"=w4046:errorcluster, "V3 out"=w4048:dbl)  [unwired: 9 in]
        n1857 = call "GainToCtrlV.vi"("Gain"=w4050, "Channel"=enum16{"Ch1", "Ch2", "Ch3"}."Ch3") -> ("CtrlV"=w4045:dbl)  [unwired: 8 in, 1 out]
        n1858 = local write "V 3"(w4045) -> ()
        n1859 = call "V3FGV.vi"("Error In"=w4046, "V3 in"=w4045) -> ()  [unwired: 8 in, 2 out]
        n1860 = Not Equal?(x=w4045, y=w4048) -> (x != y?=w4047:bool)
      }
    }
    n1861 = call "LabJack_FGV.vi"("Operation(Read)"=enum16{"Write", "Read"}."Read" ("Operation"), "error in (no error)"=w3933) -> ("error out"=w3942:errorcluster, "Read data"=w3978:i32)  [unwired: 8 in]
    n1862 = flat-sequence {
      tunnel: [w3982] -> w3939
      tunnel: w3933 -> [_]
      frame #0 {
        n1863 = Tick Count (ms)() -> (millisecond timer value=w3982:u32)
      }
    }
    n1864 = case "Channel 1" shown="True" w3958 {
      tunnel: w3942 -> [w4008 w4014]
      tunnel: w3978 -> [w4007 w4013]
      tunnel: [w4008 w4009] -> w3937
      tunnel: [w4007 w4012] -> w3973
      tunnel: w3941 -> [_ w4010]
      frame False {
        # "Do nothing"
      }
      frame True {
        # "request V\nupdate FGV"
        n1865 = global read "GlobalVariables.vi" "Ch1 LJ pin"() -> (w4011:string)
        n1866 = call "LJM_eWriteName.vi"("Handle In"=w4013, "Name"=w4011, "Value"=w4010, "error in"=w4014) -> ("Handle Out"=w4012:i32, "error out"=w4009:errorcluster)  [unwired: 10 in]
      }
    }
    n1867 = case "Channel 2" shown="True" w3957 {
      tunnel: w3937 -> [w3999 w4006]
      tunnel: [w3999 w4001] -> w3936
      tunnel: w3973 -> [w4000 w4005]
      tunnel: [w4000 w4004] -> w3972
      tunnel: w3953 -> [_ w4002]
      frame False {
        # "Do nothing"
      }
      frame True {
        # "request V\nupdate FGV"
        n1868 = global read "GlobalVariables.vi" "Ch2 LJ pin"() -> (w4003:string)
        n1869 = call "LJM_eWriteName.vi"("Handle In"=w4005, "Name"=w4003, "Value"=w4002, "error in"=w4006) -> ("Handle Out"=w4004:i32, "error out"=w4001:errorcluster)  [unwired: 10 in]
      }
    }
    n1870 = case "Channel 3" shown="True" w3956 {
      tunnel: w3936 -> [w3992 w3998]
      tunnel: [w3992 w3994] -> w3935
      tunnel: w3972 -> [w3991 w3997]
      tunnel: w3955 -> [_ w3995]
      tunnel: [w3991 w3993] -> w3946
      frame False {
        # "Do nothing"
      }
      frame True {
        # "request V\nupdate FGV"
        n1871 = global read "GlobalVariables.vi" "Ch3 LJ pin"() -> (w3996:string)
        n1872 = call "LJM_eWriteName.vi"("Handle In"=w3997, "Name"=w3996, "Value"=w3995, "error in"=w3998) -> ("Handle Out"=w3993:i32, "error out"=w3994:errorcluster)  [unwired: 10 in]
      }
    }
    n1873 = case "Channel 4" shown="True" w3947 {
      tunnel: w3935 -> [w3984 w3990]
      tunnel: w3946 -> [w3983 w3989]
      tunnel: [w3984 w3985] -> w3940
      tunnel: [w3983 w3988] -> _
      tunnel: w3948 -> [_ w3986]
      frame False {
        # "Do nothing"
      }
      frame True {
        # "request V\nupdate FGV"
        n1874 = global read "GlobalVariables.vi" "Ch4 LJ pin"() -> (w3987:string)
        n1875 = call "LJM_eWriteName.vi"("Handle In"=w3989, "Name"=w3987, "Value"=w3986, "error in"=w3990) -> ("Handle Out"=w3988:i32, "error out"=w3985:errorcluster)  [unwired: 10 in]
      }
    }
    "PID loop error out" <- w3940
    n1876 = flat-sequence {
      tunnel: [w3981] -> w3938
      tunnel: w3940 -> [_]
      frame #0 {
        n1877 = Tick Count (ms)() -> (millisecond timer value=w3981:u32)
      }
    }
    n1878 = Subtract(x=w3938, y=w3939) -> (x-y=w3934:u32)
    "LJ process (ms)" <- w3934
    "PID loop" <- w3960
  }
  "LJ time(ms)" <- w1
  n1879 = Unregister For Events(event registration refnum=w46, error in=w4) -> (error out=w52:errorcluster)
  n1880 = Destroy User Event(user event=w39, error in=w52) -> (error out=w3:errorcluster)
  n1881 = Close File(refnum=w21, error in=w3) -> ()  [unwired: 2 out]
  n1882 = Release Notifier(notifier=w16, error in (no error)=w49) -> (error out=w50:errorcluster)  [unwired: 1 in, 2 out]
  n1883 = Release Notifier(notifier=w17, error in (no error)=w38) -> (error out=w43:errorcluster)  [unwired: 1 in, 2 out]
  n1884 = call <vilib>:"Simple Error Handler.vi"("error in (no error)"=w50) -> ()  [unwired: 4 in, 5 out]
  n1885 = call <vilib>:"Simple Error Handler.vi"("error in (no error)"=w43) -> ()  [unwired: 4 in, 5 out]
  n1886 = Release Notifier(notifier=w59, error in (no error)=w58) -> (error out=w57:errorcluster)  [unwired: 1 in, 2 out]
  n1887 = Unregister For Events(event registration refnum=w63, error in=w61) -> (error out=w62:errorcluster)
  n1888 = call <vilib>:"Simple Error Handler.vi"("error in (no error)"=w57) -> ()  [unwired: 4 in, 5 out]
  n1889 = Destroy User Event(user event=w53, error in=w62) -> ()  [unwired: 1 out]
